vi "CspecN2_Part_2024.vi"(0 "Temperature [K]":dbl=293.16 format="%.4g") -> (1 "rel unc Cp0 N2":dbl=1.7168935136343725e-07 format="%.1e", 2 "Cp0/R N2":dbl=3.50261546072023 format="%.5f", 3 "Cp0 N2 [J / K mol]":dbl=29.122365250340124 format="%.5g", 4 "Cv0 N2 [J / K mol]":dbl=20.807902650340125 format="%.5g", 5 "Gamma0 N2":dbl=1.3995819636278475)   [LabVIEW 2016]
uses:
  <vilib>/Analysis/NI_AALPro.lvlib
panel:
  out "ur(Cp0) /ppm":dbl[](array[numeric]) format="%.2f"
  out "abs unc Cp0 N2 [J / K mol]":dbl=5e-06 format="%.6f"
  out "abs unc Cp0/R N2":dbl=6.013617765266032e-07 format="%.6f"
  out "u(Cp0) / J mol-1 K-1":dbl[](array[numeric]) format="%.6f"
  out "Cp0 array / J mol-1 K-1":dbl[](array[numeric]) format="%.5g"
  out "T array / K":dbl[](array[numeric]) format="%.2g"
  # "Gamache, R. R., & Orphanos, N. G. \"Thermodynamic functions for N2 from the total partition sum and its moments\" J. Phys. Chem. Ref. Data 52, 023101 (2023)"
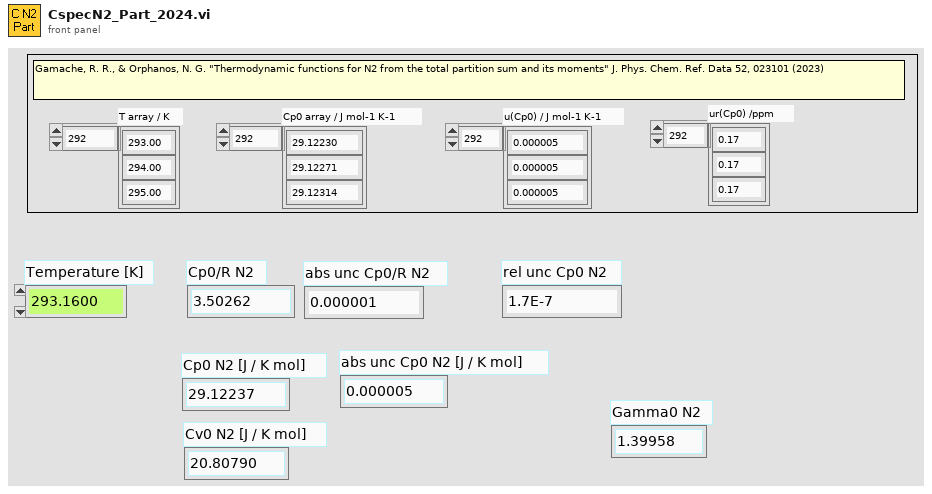
[diagram p1: front panel]
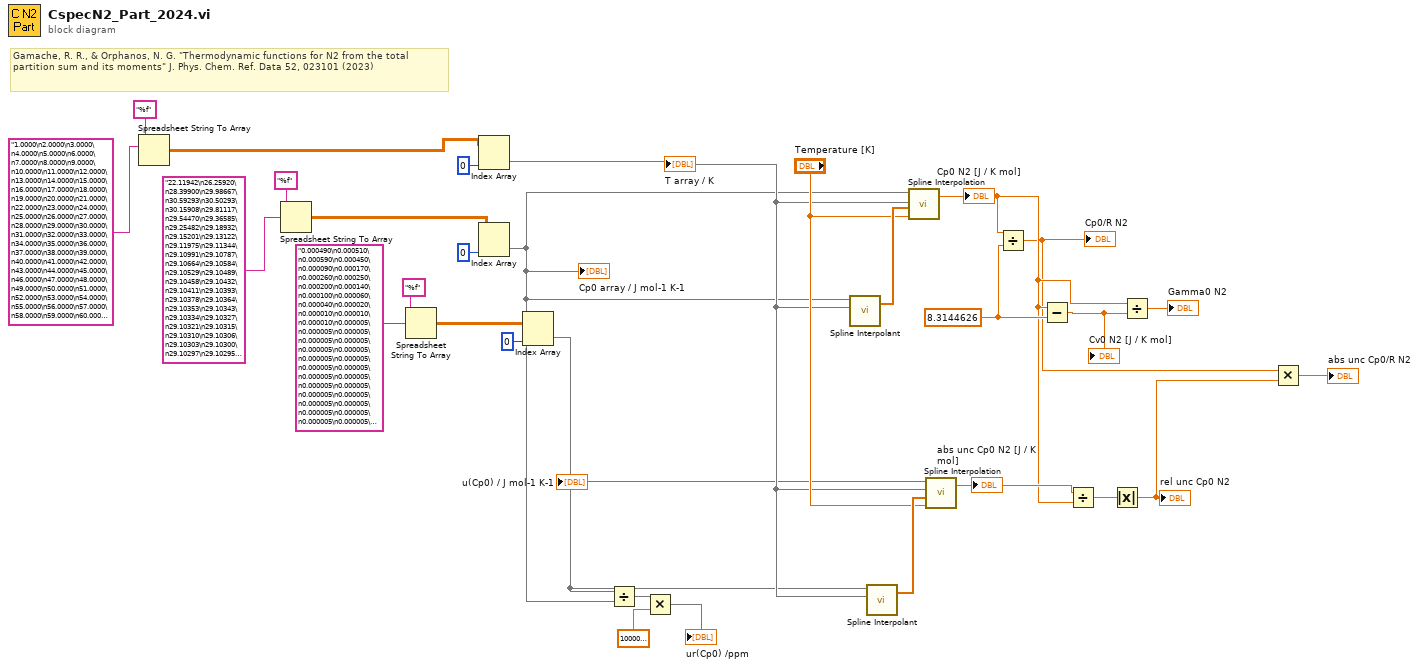
[diagram p0: block diagram]
diagram:
  w27 = 8.3144626
  # "Gamache, R. R., & Orphanos, N. G. \"Thermodynamic functions for N2 from the total partition sum and its moments\" J. Phys. Chem. Ref. Data 52, 023101 (2023)"
  n1 = Spreadsheet String To Array(format string="%f", spreadsheet string="1.0000\n2.0000\n3.0000\n4.0000\n5.0000\n6.0000\n7.0000\n8.0000\n9.0000\n10.0000\n11.0000\n12.0000\n13.0000\n14.0000\n15.0000\n16.0000\n17.0000\n18.0000\n19.0000\n20.0000\n21.0000\n22.0000\n23.0000\n24.0000\n25.0000\n26.0000\n27.0000\n28.0000\n29.0000\n30.0000\n31.0000\n32.0000\n33.0000\n34.0000\n35.0000\n36.0000\n37.0000\n38.0000\n39.0000\n40.0000\n41.0000\n42.0000\n43.0000\n44.0000\n45.0000\n46.0000\n47.0000\n48.0000\n49.0000\n50.0000\n51.0000\n52.0000\n53.0000\n54.0000\n55.0000\n56.0000\n57.0000\n58.0000\n59.0000\n60.0000\n61.0000\n62.0000\n63.0000\n64.0000\n65.0000\n66.0000\n67.0000\n68.0000\n69.0000\n70.0000\n71.0000\n72.0000\n73.0000\n74.0000\n75.0000\n76.0000\n77.0000\n78.0000\n79.0000\n80.0000\n81.0000\n82.0000\n83.0000\n84.0000\n85.0000\n86.0000\n87.0000\n88.0000\n89.0000\n90.0000\n91.0000\n92.0000\n93.0000\n94.0000\n95.0000\n96.0000\n97.0000\n98.0000\n99.0000\n100.0000\n101.0000\n102.0000\n103.0000\n104.0000\n105.0000\n106.0000\n107.0000\n108.0000\n109.0000\n110.0000\n111.0000\n112.0000\n113.0000\n114.0000\n115.0000\n116.0000\n117.0000\n118.0000\n119.0000\n120.0000\n121.0000\n122.0000\n123.0000\n124.0000\n125.0000\n126.0000\n127.0000\n128.0000\n129.0000\n130.0000\n131.0000\n132.0000\n133.0000\n134.0000\n135.0000\n136.0000\n137.0000\n138.0000\n139.0000\n140.0000\n141.0000\n142.0000\n143.0000\n144.0000\n145.0000\n146.0000\n147.0000\n148.0000\n149.0000\n150.0000\n151.0000\n152.0000\n153.0000\n154.0000\n155.0000\n156.0000\n157.0000\n158.0000\n159.0000\n160.0000\n161.0000\n162.0000\n163.0000\n164.0000\n165.0000\n166.0000\n167.0000\n168.0000\n169.0000\n170.0000\n171.0000\n172.0000\n173.0000\n174.0000\n175.0000\n176.0000\n177.0000\n178.0000\n179.0000\n180.0000\n181.0000\n182.0000\n183.0000\n184.0000\n185.0000\n186.0000\n187.0000\n188.0000\n189.0000\n190.0000\n191.0000\n192.0000\n193.0000\n194.0000\n195.0000\n196.0000\n197.0000\n198.0000\n199.0000\n200.0000\n201.0000\n202.0000\n203.0000\n204.0000\n205.0000\n206.0000\n207.0000\n208.0000\n209.0000\n210.0000\n211.0000\n212.0000\n213.0000\n214.0000\n215.0000\n216.0000\n217.0000\n218.0000\n219.0000\n220.0000\n221.0000\n222.0000\n223.0000\n224.0000\n225.0000\n226.0000\n227.0000\n228.0000\n229.0000\n230.0000\n231.0000\n232.0000\n233.0000\n234.0000\n235.0000\n236.0000\n237.0000\n238.0000\n239.0000\n240.0000\n241.0000\n242.0000\n243.0000\n244.0000\n245.0000\n246.0000\n247.0000\n248.0000\n249.0000\n250.0000\n251.0000\n252.0000\n253.0000\n254.0000\n255.0000\n256.0000\n257.0000\n258.0000\n259.0000\n260.0000\n261.0000\n262.0000\n263.0000\n264.0000\n265.0000\n266.0000\n267.0000\n268.0000\n269.0000\n270.0000\n271.0000\n272.0000\n273.0000\n274.0000\n275.0000\n276.0000\n277.0000\n278.0000\n279.0000\n280.0000\n281.0000\n282.0000\n283.0000\n284.0000\n285.0000\n286.0000\n287.0000\n288.0000\n289.0000\n290.0000\n291.0000\n292.0000\n293.0000\n294.0000\n295.0000\n296.0000\n297.0000\n298.1500\n299.0000\n300.0000\n301.0000\n302.0000\n303.0000\n304.0000\n305.0000\n306.0000\n307.0000\n308.0000\n309.0000\n310.0000\n311.0000\n312.0000\n313.0000\n314.0000\n315.0000\n316.0000\n317.0000\n318.0000\n319.0000\n320.0000\n321.0000\n322.0000\n323.0000\n324.0000\n325.0000\n326.0000\n327.0000\n328.0000\n329.0000\n330.0000\n331.0000\n332.0000\n333.0000\n334.0000\n335.0000\n336.0000\n337.0000\n338.0000\n339.0000\n340.0000\n341.0000\n342.0000\n343.0000\n344.0000\n345.0000\n346.0000\n347.0000\n348.0000\n349.0000\n350.0000\n351.0000\n352.0000\n353.0000\n354.0000\n355.0000\n356.0000\n357.0000\n358.0000\n359.0000\n360.0000\n361.0000\n362.0000\n363.0000\n364.0000\n365.0000\n366.0000\n367.0000\n368.0000\n369.0000\n370.0000\n371.0000\n372.0000\n373.0000\n374.0000\n375.0000\n376.0000\n377.0000\n378.0000\n379.0000\n380.0000\n381.0000\n382.0000\n383.0000\n384.0000\n385.0000\n386.0000\n387.0000\n388.0000\n389.0000\n390.0000\n391.0000\n392.0000\n393.0000\n394.0000\n395.0000\n396.0000\n397.0000\n398.0000\n399.0000\n400.0000\n401.0000\n402.0000\n403.0000\n404.0000\n405.0000\n406.0000\n407.0000\n408.0000\n409.0000\n410.0000\n411.0000\n412.0000\n413.0000\n414.0000\n415.0000\n416.0000\n417.0000\n418.0000\n419.0000\n420.0000\n421.0000\n422.0000\n423.0000\n424.0000\n425.0000\n426.0000\n427.0000\n428.0000\n429.0000\n430.0000\n431.0000\n432.0000\n433.0000\n434.0000\n435.0000\n436.0000\n437.0000\n438.0000\n439.0000\n440.0000\n441.0000\n442.0000\n443.0000\n444.0000\n445.0000\n446.0000\n447.0000\n448.0000\n449.0000\n450.0000\n451.0000\n452.0000\n453.0000\n454.0000\n455.0000\n456.0000\n457.0000\n458.0000\n459.0000\n460.0000\n461.0000\n462.0000\n463.0000\n464.0000\n465.0000\n466.0000\n467.0000\n468.0000\n469.0000\n470.0000\n471.0000\n472.0000\n473.0000\n474.0000\n475.0000\n476.0000\n477.0000\n478.0000\n479.0000\n480.0000\n481.0000\n482.0000\n483.0000\n484.0000\n485.0000\n486.0000\n487.0000\n488.0000\n489.0000\n490.0000\n491.0000\n492.0000\n493.0000\n494.0000\n495.0000\n496.0000\n497.0000\n498.0000\n499.0000\n500.0000\n501.0000\n502.0000\n503.0000\n504.0000\n505.0000\n506.0000\n507.0000\n508.0000\n509.0000\n510.0000\n511.0000\n512.0000\n513.0000\n514.0000\n515.0000\n516.0000\n517.0000\n518.0000\n519.0000\n520.0000\n521.0000\n522.0000\n523.0000\n524.0000\n525.0000\n526.0000\n527.0000\n528.0000\n529.0000\n530.0000\n531.0000\n532.0000\n533.0000\n534.0000\n535.0000\n536.0000\n537.0000\n538.0000\n539.0000\n540.0000\n541.0000\n542.0000\n543.0000\n544.0000\n545.0000\n546.0000\n547.0000\n548.0000\n549.0000\n550.0000\n551.0000\n552.0000\n553.0000\n554.0000\n555.0000\n556.0000\n557.0000\n558.0000\n559.0000\n560.0000\n561.0000\n562.0000\n563.0000\n564.0000\n565.0000\n566.0000\n567.0000\n568.0000\n569.0000\n570.0000\n571.0000\n572.0000\n573.0000\n574.0000\n575.0000\n576.0000\n577.0000\n578.0000\n579.0000\n580.0000\n581.0000\n582.0000\n583.0000\n584.0000\n585.0000\n586.0000\n587.0000\n588.0000\n589.0000\n590.0000\n591.0000\n592.0000\n593.0000\n594.0000\n595.0000\n596.0000\n597.0000\n598.0000\n599.0000\n600.0000\n601.0000\n602.0000\n603.0000\n604.0000\n605.0000\n606.0000\n607.0000\n608.0000\n609.0000\n610.0000\n611.0000\n612.0000\n613.0000\n614.0000\n615.0000\n616.0000\n617.0000\n618.0000\n619.0000\n620.0000\n621.0000\n622.0000\n623.0000\n624.0000\n625.0000\n626.0000\n627.0000\n628.0000\n629.0000\n630.0000\n631.0000\n632.0000\n633.0000\n634.0000\n635.0000\n636.0000\n637.0000\n638.0000\n639.0000\n640.0000\n641.0000\n642.0000\n643.0000\n644.0000\n645.0000\n646.0000\n647.0000\n648.0000\n649.0000\n650.0000\n651.0000\n652.0000\n653.0000\n654.0000\n655.0000\n656.0000\n657.0000\n658.0000\n659.0000\n660.0000\n661.0000\n662.0000\n663.0000\n664.0000\n665.0000\n666.0000\n667.0000\n668.0000\n669.0000\n670.0000\n671.0000\n672.0000\n673.0000\n674.0000\n675.0000\n676.0000\n677.0000\n678.0000\n679.0000\n680.0000\n681.0000\n682.0000\n683.0000\n684.0000\n685.0000\n686.0000\n687.0000\n688.0000\n689.0000\n690.0000\n691.0000\n692.0000\n693.0000\n694.0000\n695.0000\n696.0000\n697.0000\n698.0000\n699.0000\n700.0000\n701.0000\n702.0000\n703.0000\n704.0000\n705.0000\n706.0000\n707.0000\n708.0000\n709.0000\n710.0000\n711.0000\n712.0000\n713.0000\n714.0000\n715.0000\n716.0000\n717.0000\n718.0000\n719.0000\n720.0000\n721.0000\n722.0000\n723.0000\n724.0000\n725.0000\n726.0000\n727.0000\n728.0000\n729.0000\n730.0000\n731.0000\n732.0000\n733.0000\n734.0000\n735.0000\n736.0000\n737.0000\n738.0000\n739.0000\n740.0000\n741.0000\n742.0000\n743.0000\n744.0000\n745.0000\n746.0000\n747.0000\n748.0000\n749.0000\n750.0000\n751.0000\n752.0000\n753.0000\n754.0000\n755.0000\n756.0000\n757.0000\n758.0000\n759.0000\n760.0000\n761.0000\n762.0000\n763.0000\n764.0000\n765.0000\n766.0000\n767.0000\n768.0000\n769.0000\n770.0000\n771.0000\n772.0000\n773.0000\n774.0000\n775.0000\n776.0000\n777.0000\n778.0000\n779.0000\n780.0000\n781.0000\n782.0000\n783.0000\n784.0000\n785.0000\n786.0000\n787.0000\n788.0000\n789.0000\n790.0000\n791.0000\n792.0000\n793.0000\n794.0000\n795.0000\n796.0000\n797.0000\n798.0000\n799.0000\n800.0000\n801.0000\n802.0000\n803.0000\n804.0000\n805.0000\n806.0000\n807.0000\n808.0000\n809.0000\n810.0000\n811.0000\n812.0000\n813.0000\n814.0000\n815.0000\n816.0000\n817.0000\n818.0000\n819.0000\n820.0000\n821.0000\n822.0000\n823.0000\n824.0000\n825.0000\n826.0000\n827.0000\n828.0000\n829.0000\n830.0000\n831.0000\n832.0000\n833.0000\n834.0000\n835.0000\n836.0000\n837.0000\n838.0000\n839.0000\n840.0000\n841.0000\n842.0000\n843.0000\n844.0000\n845.0000\n846.0000\n847.0000\n848.0000\n849.0000\n850.0000\n851.0000\n852.0000\n853.0000\n854.0000\n855.0000\n856.0000\n857.0000\n858.0000\n859.0000\n860.0000\n861.0000\n862.0000\n863.0000\n864.0000\n865.0000\n866.0000\n867.0000\n868.0000\n869.0000\n870.0000\n871.0000\n872.0000\n873.0000\n874.0000\n875.0000\n876.0000\n877.0000\n878.0000\n879.0000\n880.0000\n881.0000\n882.0000\n883.0000\n884.0000\n885.0000\n886.0000\n887.0000\n888.0000\n889.0000\n890.0000\n891.0000\n892.0000\n893.0000\n894.0000\n895.0000\n896.0000\n897.0000\n898.0000\n899.0000\n900.0000\n901.0000\n902.0000\n903.0000\n904.0000\n905.0000\n906.0000\n907.0000\n908.0000\n909.0000\n910.0000\n911.0000\n912.0000\n913.0000\n914.0000\n915.0000\n916.0000\n917.0000\n918.0000\n919.0000\n920.0000\n921.0000\n922.0000\n923.0000\n924.0000\n925.0000\n926.0000\n927.0000\n928.0000\n929.0000\n930.0000\n931.0000\n932.0000\n933.0000\n934.0000\n935.0000\n936.0000\n937.0000\n938.0000\n939.0000\n940.0000\n941.0000\n942.0000\n943.0000\n944.0000\n945.0000\n946.0000\n947.0000\n948.0000\n949.0000\n950.0000\n951.0000\n952.0000\n953.0000\n954.0000\n955.0000\n956.0000\n957.0000\n958.0000\n959.0000\n960.0000\n961.0000\n962.0000\n963.0000\n964.0000\n965.0000\n966.0000\n967.0000\n968.0000\n969.0000\n970.0000\n971.0000\n972.0000\n973.0000\n974.0000\n975.0000\n976.0000\n977.0000\n978.0000\n979.0000\n980.0000\n981.0000\n982.0000\n983.0000\n984.0000\n985.0000\n986.0000\n987.0000\n988.0000\n989.0000\n990.0000\n991.0000\n992.0000\n993.0000\n994.0000\n995.0000\n996.0000\n997.0000\n998.0000\n999.0000\n1000.0000\n1001.0000\n1002.0000\n1003.0000\n1004.0000\n1005.0000\n1006.0000\n1007.0000\n1008.0000\n1009.0000\n1010.0000\n1011.0000\n1012.0000\n1013.0000\n1014.0000\n1015.0000\n1016.0000\n1017.0000\n1018.0000\n1019.0000\n1020.0000\n1021.0000\n1022.0000\n1023.0000\n1024.0000\n1025.0000\n1026.0000\n1027.0000\n1028.0000\n1029.0000\n1030.0000\n1031.0000\n1032.0000\n1033.0000\n1034.0000\n1035.0000\n1036.0000\n1037.0000\n1038.0000\n1039.0000\n1040.0000\n1041.0000\n1042.0000\n1043.0000\n1044.0000\n1045.0000\n1046.0000\n1047.0000\n1048.0000\n1049.0000\n1050.0000\n1051.0000\n1052.0000\n1053.0000\n1054.0000\n1055.0000\n1056.0000\n1057.0000\n1058.0000\n1059.0000\n1060.0000\n1061.0000\n1062.0000\n1063.0000\n1064.0000\n1065.0000\n1066.0000\n1067.0000\n1068.0000\n1069.0000\n1070.0000\n1071.0000\n1072.0000\n1073.0000\n1074.0000\n1075.0000\n1076.0000\n1077.0000\n1078.0000\n1079.0000\n1080.0000\n1081.0000\n1082.0000\n1083.0000\n1084.0000\n1085.0000\n1086.0000\n1087.0000\n1088.0000\n1089.0000\n1090.0000\n1091.0000\n1092.0000\n1093.0000\n1094.0000\n1095.0000\n1096.0000\n1097.0000\n1098.0000\n1099.0000\n1100.0000\n1101.0000\n1102.0000\n1103.0000\n1104.0000\n1105.0000\n1106.0000\n1107.0000\n1108.0000\n1109.0000\n1110.0000\n1111.0000\n1112.0000\n1113.0000\n1114.0000\n1115.0000\n1116.0000\n1117.0000\n1118.0000\n1119.0000\n1120.0000\n1121.0000\n1122.0000\n1123.0000\n1124.0000\n1125.0000\n1126.0000\n1127.0000\n1128.0000\n1129.0000\n1130.0000\n1131.0000\n1132.0000\n1133.0000\n1134.0000\n1135.0000\n1136.0000\n1137.0000\n1138.0000\n1139.0000\n1140.0000\n1141.0000\n1142.0000\n1143.0000\n1144.0000\n1145.0000\n1146.0000\n1147.0000\n1148.0000\n1149.0000\n1150.0000\n1151.0000\n1152.0000\n1153.0000\n1154.0000\n1155.0000\n1156.0000\n1157.0000\n1158.0000\n1159.0000\n1160.0000\n1161.0000\n1162.0000\n1163.0000\n1164.0000\n1165.0000\n1166.0000\n1167.0000\n1168.0000\n1169.0000\n1170.0000\n1171.0000\n1172.0000\n1173.0000\n1174.0000\n1175.0000\n1176.0000\n1177.0000\n1178.0000\n1179.0000\n1180.0000\n1181.0000\n1182.0000\n1183.0000\n1184.0000\n1185.0000\n1186.0000\n1187.0000\n1188.0000\n1189.0000\n1190.0000\n1191.0000\n1192.0000\n1193.0000\n1194.0000\n1195.0000\n1196.0000\n1197.0000\n1198.0000\n1199.0000\n1200.0000\n1201.0000\n1202.0000\n1203.0000\n1204.0000\n1205.0000\n1206.0000\n1207.0000\n1208.0000\n1209.0000\n1210.0000\n1211.0000\n1212.0000\n1213.0000\n1214.0000\n1215.0000\n1216.0000\n1217.0000\n1218.0000\n1219.0000\n1220.0000\n1221.0000\n1222.0000\n1223.0000\n1224.0000\n1225.0000\n1226.0000\n1227.0000\n1228.0000\n1229.0000\n1230.0000\n1231.0000\n1232.0000\n1233.0000\n1234.0000\n1235.0000\n1236.0000\n1237.0000\n1238.0000\n1239.0000\n1240.0000\n1241.0000\n1242.0000\n1243.0000\n1244.0000\n1245.0000\n1246.0000\n1247.0000\n1248.0000\n1249.0000\n1250.0000\n1251.0000\n1252.0000\n1253.0000\n1254.0000\n1255.0000\n1256.0000\n1257.0000\n1258.0000\n1259.0000\n1260.0000\n1261.0000\n1262.0000\n1263.0000\n1264.0000\n1265.0000\n1266.0000\n1267.0000\n1268.0000\n1269.0000\n1270.0000\n1271.0000\n1272.0000\n1273.0000\n1274.0000\n1275.0000\n1276.0000\n1277.0000\n1278.0000\n1279.0000\n1280.0000\n1281.0000\n1282.0000\n1283.0000\n1284.0000\n1285.0000\n1286.0000\n1287.0000\n1288.0000\n1289.0000\n1290.0000\n1291.0000\n1292.0000\n1293.0000\n1294.0000\n1295.0000\n1296.0000\n1297.0000\n1298.0000\n1299.0000\n1300.0000\n1301.0000\n1302.0000\n1303.0000\n1304.0000\n1305.0000\n1306.0000\n1307.0000\n1308.0000\n1309.0000\n1310.0000\n1311.0000\n1312.0000\n1313.0000\n1314.0000\n1315.0000\n1316.0000\n1317.0000\n1318.0000\n1319.0000\n1320.0000\n1321.0000\n1322.0000\n1323.0000\n1324.0000\n1325.0000\n1326.0000\n1327.0000\n1328.0000\n1329.0000\n1330.0000\n1331.0000\n1332.0000\n1333.0000\n1334.0000\n1335.0000\n1336.0000\n1337.0000\n1338.0000\n1339.0000\n1340.0000\n1341.0000\n1342.0000\n1343.0000\n1344.0000\n1345.0000\n1346.0000\n1347.0000\n1348.0000\n1349.0000\n1350.0000\n1351.0000\n1352.0000\n1353.0000\n1354.0000\n1355.0000\n1356.0000\n1357.0000\n1358.0000\n1359.0000\n1360.0000\n1361.0000\n1362.0000\n1363.0000\n1364.0000\n1365.0000\n1366.0000\n1367.0000\n1368.0000\n1369.0000\n1370.0000\n1371.0000\n1372.0000\n1373.0000\n1374.0000\n1375.0000\n1376.0000\n1377.0000\n1378.0000\n1379.0000\n1380.0000\n1381.0000\n1382.0000\n1383.0000\n1384.0000\n1385.0000\n1386.0000\n1387.0000\n1388.0000\n1389.0000\n1390.0000\n1391.0000\n1392.0000\n1393.0000\n1394.0000\n1395.0000\n1396.0000\n1397.0000\n1398.0000\n1399.0000\n1400.0000\n1401.0000\n1402.0000\n1403.0000\n1404.0000\n1405.0000\n1406.0000\n1407.0000\n1408.0000\n1409.0000\n1410.0000\n1411.0000\n1412.0000\n1413.0000\n1414.0000\n1415.0000\n1416.0000\n1417.0000\n1418.0000\n1419.0000\n1420.0000\n1421.0000\n1422.0000\n1423.0000\n1424.0000\n1425.0000\n1426.0000\n1427.0000\n1428.0000\n1429.0000\n1430.0000\n1431.0000\n1432.0000\n1433.0000\n1434.0000\n1435.0000\n1436.0000\n1437.0000\n1438.0000\n1439.0000\n1440.0000\n1441.0000\n1442.0000\n1443.0000\n1444.0000\n1445.0000\n1446.0000\n1447.0000\n1448.0000\n1449.0000\n1450.0000\n1451.0000\n1452.0000\n1453.0000\n1454.0000\n1455.0000\n1456.0000\n1457.0000\n1458.0000\n1459.0000\n1460.0000\n1461.0000\n1462.0000\n1463.0000\n1464.0000\n1465.0000\n1466.0000\n1467.0000\n1468.0000\n1469.0000\n1470.0000\n1471.0000\n1472.0000\n1473.0000\n1474.0000\n1475.0000\n1476.0000\n1477.0000\n1478.0000\n1479.0000\n1480.0000\n1481.0000\n1482.0000\n1483.0000\n1484.0000\n1485.0000\n1486.0000\n1487.0000\n1488.0000\n1489.0000\n1490.0000\n1491.0000\n1492.0000\n1493.0000\n1494.0000\n1495.0000\n1496.0000\n1497.0000\n1498.0000\n1499.0000\n1500.0000\n1501.0000\n1502.0000\n1503.0000\n1504.0000\n1505.0000\n1506.0000\n1507.0000\n1508.0000\n1509.0000\n1510.0000\n1511.0000\n1512.0000\n1513.0000\n1514.0000\n1515.0000\n1516.0000\n1517.0000\n1518.0000\n1519.0000\n1520.0000\n1521.0000\n1522.0000\n1523.0000\n1524.0000\n1525.0000\n1526.0000\n1527.0000\n1528.0000\n1529.0000\n1530.0000\n1531.0000\n1532.0000\n1533.0000\n1534.0000\n1535.0000\n1536.0000\n1537.0000\n1538.0000\n1539.0000\n1540.0000\n1541.0000\n1542.0000\n1543.0000\n1544.0000\n1545.0000\n1546.0000\n1547.0000\n1548.0000\n1549.0000\n1550.0000\n1551.0000\n1552.0000\n1553.0000\n1554.0000\n1555.0000\n1556.0000\n1557.0000\n1558.0000\n1559.0000\n1560.0000\n1561.0000\n1562.0000\n1563.0000\n1564.0000\n1565.0000\n1566.0000\n1567.0000\n1568.0000\n1569.0000\n1570.0000\n1571.0000\n1572.0000\n1573.0000\n1574.0000\n1575.0000\n1576.0000\n1577.0000\n1578.0000\n1579.0000\n1580.0000\n1581.0000\n1582.0000\n1583.0000\n1584.0000\n1585.0000\n1586.0000\n1587.0000\n1588.0000\n1589.0000\n1590.0000\n1591.0000\n1592.0000\n1593.0000\n1594.0000\n1595.0000\n1596.0000\n1597.0000\n1598.0000\n1599.0000\n1600.0000\n1601.0000\n1602.0000\n1603.0000\n1604.0000\n1605.0000\n1606.0000\n1607.0000\n1608.0000\n1609.0000\n1610.0000\n1611.0000\n1612.0000\n1613.0000\n1614.0000\n1615.0000\n1616.0000\n1617.0000\n1618.0000\n1619.0000\n1620.0000\n1621.0000\n1622.0000\n1623.0000\n1624.0000\n1625.0000\n1626.0000\n1627.0000\n1628.0000\n1629.0000\n1630.0000\n1631.0000\n1632.0000\n1633.0000\n1634.0000\n1635.0000\n1636.0000\n1637.0000\n1638.0000\n1639.0000\n1640.0000\n1641.0000\n1642.0000\n1643.0000\n1644.0000\n1645.0000\n1646.0000\n1647.0000\n1648.0000\n1649.0000\n1650.0000\n1651.0000\n1652.0000\n1653.0000\n1654.0000\n1655.0000\n1656.0000\n1657.0000\n1658.0000\n1659.0000\n1660.0000\n1661.0000\n1662.0000\n1663.0000\n1664.0000\n1665.0000\n1666.0000\n1667.0000\n1668.0000\n1669.0000\n1670.0000\n1671.0000\n1672.0000\n1673.0000\n1674.0000\n1675.0000\n1676.0000\n1677.0000\n1678.0000\n1679.0000\n1680.0000\n1681.0000\n1682.0000\n1683.0000\n1684.0000\n1685.0000\n1686.0000\n1687.0000\n1688.0000\n1689.0000\n1690.0000\n1691.0000\n1692.0000\n1693.0000\n1694.0000\n1695.0000\n1696.0000\n1697.0000\n1698.0000\n1699.0000\n1700.0000\n1701.0000\n1702.0000\n1703.0000\n1704.0000\n1705.0000\n1706.0000\n1707.0000\n1708.0000\n1709.0000\n1710.0000\n1711.0000\n1712.0000\n1713.0000\n1714.0000\n1715.0000\n1716.0000\n1717.0000\n1718.0000\n1719.0000\n1720.0000\n1721.0000\n1722.0000\n1723.0000\n1724.0000\n1725.0000\n1726.0000\n1727.0000\n1728.0000\n1729.0000\n1730.0000\n1731.0000\n1732.0000\n1733.0000\n1734.0000\n1735.0000\n1736.0000\n1737.0000\n1738.0000\n1739.0000\n1740.0000\n1741.0000\n1742.0000\n1743.0000\n1744.0000\n1745.0000\n1746.0000\n1747.0000\n1748.0000\n1749.0000\n1750.0000\n1751.0000\n1752.0000\n1753.0000\n1754.0000\n1755.0000\n1756.0000\n1757.0000\n1758.0000\n1759.0000\n1760.0000\n1761.0000\n1762.0000\n1763.0000\n1764.0000\n1765.0000\n1766.0000\n1767.0000\n1768.0000\n1769.0000\n1770.0000\n1771.0000\n1772.0000\n1773.0000\n1774.0000\n1775.0000\n1776.0000\n1777.0000\n1778.0000\n1779.0000\n1780.0000\n1781.0000\n1782.0000\n1783.0000\n1784.0000\n1785.0000\n1786.0000\n1787.0000\n1788.0000\n1789.0000\n1790.0000\n1791.0000\n1792.0000\n1793.0000\n1794.0000\n1795.0000\n1796.0000\n1797.0000\n1798.0000\n1799.0000\n1800.0000\n1801.0000\n1802.0000\n1803.0000\n1804.0000\n1805.0000\n1806.0000\n1807.0000\n1808.0000\n1809.0000\n1810.0000\n1811.0000\n1812.0000\n1813.0000\n1814.0000\n1815.0000\n1816.0000\n1817.0000\n1818.0000\n1819.0000\n1820.0000\n1821.0000\n1822.0000\n1823.0000\n1824.0000\n1825.0000\n1826.0000\n1827.0000\n1828.0000\n1829.0000\n1830.0000\n1831.0000\n1832.0000\n1833.0000\n1834.0000\n1835.0000\n1836.0000\n1837.0000\n1838.0000\n1839.0000\n1840.0000\n1841.0000\n1842.0000\n1843.0000\n1844.0000\n1845.0000\n1846.0000\n1847.0000\n1848.0000\n1849.0000\n1850.0000\n1851.0000\n1852.0000\n1853.0000\n1854.0000\n1855.0000\n1856.0000\n1857.0000\n1858.0000\n1859.0000\n1860.0000\n1861.0000\n1862.0000\n1863.0000\n1864.0000\n1865.0000\n1866.0000\n1867.0000\n1868.0000\n1869.0000\n1870.0000\n1871.0000\n1872.0000\n1873.0000\n1874.0000\n1875.0000\n1876.0000\n1877.0000\n1878.0000\n1879.0000\n1880.0000\n1881.0000\n1882.0000\n1883.0000\n1884.0000\n1885.0000\n1886.0000\n1887.0000\n1888.0000\n1889.0000\n1890.0000\n1891.0000\n1892.0000\n1893.0000\n1894.0000\n1895.0000\n1896.0000\n1897.0000\n1898.0000\n1899.0000\n1900.0000\n1901.0000\n1902.0000\n1903.0000\n1904.0000\n1905.0000\n1906.0000\n1907.0000\n1908.0000\n1909.0000\n1910.0000\n1911.0000\n1912.0000\n1913.0000\n1914.0000\n1915.0000\n1916.0000\n1917.0000\n1918.0000\n1919.0000\n1920.0000\n1921.0000\n1922.0000\n1923.0000\n1924.0000\n1925.0000\n1926.0000\n1927.0000\n1928.0000\n1929.0000\n1930.0000\n1931.0000\n1932.0000\n1933.0000\n1934.0000\n1935.0000\n1936.0000\n1937.0000\n1938.0000\n1939.0000\n1940.0000\n1941.0000\n1942.0000\n1943.0000\n1944.0000\n1945.0000\n1946.0000\n1947.0000\n1948.0000\n1949.0000\n1950.0000\n1951.0000\n1952.0000\n1953.0000\n1954.0000\n1955.0000\n1956.0000\n1957.0000\n1958.0000\n1959.0000\n1960.0000\n1961.0000\n1962.0000\n1963.0000\n1964.0000\n1965.0000\n1966.0000\n1967.0000\n1968.0000\n1969.0000\n1970.0000\n1971.0000\n1972.0000\n1973.0000\n1974.0000\n1975.0000\n1976.0000\n1977.0000\n1978.0000\n1979.0000\n1980.0000\n1981.0000\n1982.0000\n1983.0000\n1984.0000\n1985.0000\n1986.0000\n1987.0000\n1988.0000\n1989.0000\n1990.0000\n1991.0000\n1992.0000\n1993.0000\n1994.0000\n1995.0000\n1996.0000\n1997.0000\n1998.0000\n1999.0000\n2000.0000\n2001.0000\n2002.0000\n2003.0000\n2004.0000\n2005.0000\n2006.0000\n2007.0000\n2008.0000\n2009.0000\n2010.0000\n2011.0000\n2012.0000\n2013.0000\n2014.0000\n2015.0000\n2016.0000\n2017.0000\n2018.0000\n2019.0000\n2020.0000\n2021.0000\n2022.0000\n2023.0000\n2024.0000\n2025.0000\n2026.0000\n2027.0000\n2028.0000\n2029.0000\n2030.0000\n2031.0000\n2032.0000\n2033.0000\n2034.0000\n2035.0000\n2036.0000\n2037.0000\n2038.0000\n2039.0000\n2040.0000\n2041.0000\n2042.0000\n2043.0000\n2044.0000\n2045.0000\n2046.0000\n2047.0000\n2048.0000\n2049.0000\n2050.0000\n2051.0000\n2052.0000\n2053.0000\n2054.0000\n2055.0000\n2056.0000\n2057.0000\n2058.0000\n2059.0000\n2060.0000\n2061.0000\n2062.0000\n2063.0000\n2064.0000\n2065.0000\n2066.0000\n2067.0000\n2068.0000\n2069.0000\n2070.0000\n2071.0000\n2072.0000\n2073.0000\n2074.0000\n2075.0000\n2076.0000\n2077.0000\n2078.0000\n2079.0000\n2080.0000\n2081.0000\n2082.0000\n2083.0000\n2084.0000\n2085.0000\n2086.0000\n2087.0000\n2088.0000\n2089.0000\n2090.0000\n2091.0000\n2092.0000\n2093.0000\n2094.0000\n2095.0000\n2096.0000\n2097.0000\n2098.0000\n2099.0000\n2100.0000\n2101.0000\n2102.0000\n2103.0000\n2104.0000\n2105.0000\n2106.0000\n2107.0000\n2108.0000\n2109.0000\n2110.0000\n2111.0000\n2112.0000\n2113.0000\n2114.0000\n2115.0000\n2116.0000\n2117.0000\n2118.0000\n2119.0000\n2120.0000\n2121.0000\n2122.0000\n2123.0000\n2124.0000\n2125.0000\n2126.0000\n2127.0000\n2128.0000\n2129.0000\n2130.0000\n2131.0000\n2132.0000\n2133.0000\n2134.0000\n2135.0000\n2136.0000\n2137.0000\n2138.0000\n2139.0000\n2140.0000\n2141.0000\n2142.0000\n2143.0000\n2144.0000\n2145.0000\n2146.0000\n2147.0000\n2148.0000\n2149.0000\n2150.0000\n2151.0000\n2152.0000\n2153.0000\n2154.0000\n2155.0000\n2156.0000\n2157.0000\n2158.0000\n2159.0000\n2160.0000\n2161.0000\n2162.0000\n2163.0000\n2164.0000\n2165.0000\n2166.0000\n2167.0000\n2168.0000\n2169.0000\n2170.0000\n2171.0000\n2172.0000\n2173.0000\n2174.0000\n2175.0000\n2176.0000\n2177.0000\n2178.0000\n2179.0000\n2180.0000\n2181.0000\n2182.0000\n2183.0000\n2184.0000\n2185.0000\n2186.0000\n2187.0000\n2188.0000\n2189.0000\n2190.0000\n2191.0000\n2192.0000\n2193.0000\n2194.0000\n2195.0000\n2196.0000\n2197.0000\n2198.0000\n2199.0000\n2200.0000\n2201.0000\n2202.0000\n2203.0000\n2204.0000\n2205.0000\n2206.0000\n2207.0000\n2208.0000\n2209.0000\n2210.0000\n2211.0000\n2212.0000\n2213.0000\n2214.0000\n2215.0000\n2216.0000\n2217.0000\n2218.0000\n2219.0000\n2220.0000\n2221.0000\n2222.0000\n2223.0000\n2224.0000\n2225.0000\n2226.0000\n2227.0000\n2228.0000\n2229.0000\n2230.0000\n2231.0000\n2232.0000\n2233.0000\n2234.0000\n2235.0000\n2236.0000\n2237.0000\n2238.0000\n2239.0000\n2240.0000\n2241.0000\n2242.0000\n2243.0000\n2244.0000\n2245.0000\n2246.0000\n2247.0000\n2248.0000\n2249.0000\n2250.0000\n2251.0000\n2252.0000\n2253.0000\n2254.0000\n2255.0000\n2256.0000\n2257.0000\n2258.0000\n2259.0000\n2260.0000\n2261.0000\n2262.0000\n2263.0000\n2264.0000\n2265.0000\n2266.0000\n2267.0000\n2268.0000\n2269.0000\n2270.0000\n2271.0000\n2272.0000\n2273.0000\n2274.0000\n2275.0000\n2276.0000\n2277.0000\n2278.0000\n2279.0000\n2280.0000\n2281.0000\n2282.0000\n2283.0000\n2284.0000\n2285.0000\n2286.0000\n2287.0000\n2288.0000\n2289.0000\n2290.0000\n2291.0000\n2292.0000\n2293.0000\n2294.0000\n2295.0000\n2296.0000\n2297.0000\n2298.0000\n2299.0000\n2300.0000\n2301.0000\n2302.0000\n2303.0000\n2304.0000\n2305.0000\n2306.0000\n2307.0000\n2308.0000\n2309.0000\n2310.0000\n2311.0000\n2312.0000\n2313.0000\n2314.0000\n2315.0000\n2316.0000\n2317.0000\n2318.0000\n2319.0000\n2320.0000\n2321.0000\n2322.0000\n2323.0000\n2324.0000\n2325.0000\n2326.0000\n2327.0000\n2328.0000\n2329.0000\n2330.0000\n2331.0000\n2332.0000\n2333.0000\n2334.0000\n2335.0000\n2336.0000\n2337.0000\n2338.0000\n2339.0000\n2340.0000\n2341.0000\n2342.0000\n2343.0000\n2344.0000\n2345.0000\n2346.0000\n2347.0000\n2348.0000\n2349.0000\n2350.0000\n2351.0000\n2352.0000\n2353.0000\n2354.0000\n2355.0000\n2356.0000\n2357.0000\n2358.0000\n2359.0000\n2360.0000\n2361.0000\n2362.0000\n2363.0000\n2364.0000\n2365.0000\n2366.0000\n2367.0000\n2368.0000\n2369.0000\n2370.0000\n2371.0000\n2372.0000\n2373.0000\n2374.0000\n2375.0000\n2376.0000\n2377.0000\n2378.0000\n2379.0000\n2380.0000\n2381.0000\n2382.0000\n2383.0000\n2384.0000\n2385.0000\n2386.0000\n2387.0000\n2388.0000\n2389.0000\n2390.0000\n2391.0000\n2392.0000\n2393.0000\n2394.0000\n2395.0000\n2396.0000\n2397.0000\n2398.0000\n2399.0000\n2400.0000\n2401.0000\n2402.0000\n2403.0000\n2404.0000\n2405.0000\n2406.0000\n2407.0000\n2408.0000\n2409.0000\n2410.0000\n2411.0000\n2412.0000\n2413.0000\n2414.0000\n2415.0000\n2416.0000\n2417.0000\n2418.0000\n2419.0000\n2420.0000\n2421.0000\n2422.0000\n2423.0000\n2424.0000\n2425.0000\n2426.0000\n2427.0000\n2428.0000\n2429.0000\n2430.0000\n2431.0000\n2432.0000\n2433.0000\n2434.0000\n2435.0000\n2436.0000\n2437.0000\n2438.0000\n2439.0000\n2440.0000\n2441.0000\n2442.0000\n2443.0000\n2444.0000\n2445.0000\n2446.0000\n2447.0000\n2448.0000\n2449.0000\n2450.0000\n2451.0000\n2452.0000\n2453.0000\n2454.0000\n2455.0000\n2456.0000\n2457.0000\n2458.0000\n2459.0000\n2460.0000\n2461.0000\n2462.0000\n2463.0000\n2464.0000\n2465.0000\n2466.0000\n2467.0000\n2468.0000\n2469.0000\n2470.0000\n2471.0000\n2472.0000\n2473.0000\n2474.0000\n2475.0000\n2476.0000\n2477.0000\n2478.0000\n2479.0000\n2480.0000\n2481.0000\n2482.0000\n2483.0000\n2484.0000\n2485.0000\n2486.0000\n2487.0000\n2488.0000\n2489.0000\n2490.0000\n2491.0000\n2492.0000\n2493.0000\n2494.0000\n2495.0000\n2496.0000\n2497.0000\n2498.0000\n2499.0000\n2500.0000\n2501.0000\n2502.0000\n2503.0000\n2504.0000\n2505.0000\n2506.0000\n2507.0000\n2508.0000\n2509.0000\n2510.0000\n2511.0000\n2512.0000\n2513.0000\n2514.0000\n2515.0000\n2516.0000\n2517.0000\n2518.0000\n2519.0000\n2520.0000\n2521.0000\n2522.0000\n2523.0000\n2524.0000\n2525.0000\n2526.0000\n2527.0000\n2528.0000\n2529.0000\n2530.0000\n2531.0000\n2532.0000\n2533.0000\n2534.0000\n2535.0000\n2536.0000\n2537.0000\n2538.0000\n2539.0000\n2540.0000\n2541.0000\n2542.0000\n2543.0000\n2544.0000\n2545.0000\n2546.0000\n2547.0000\n2548.0000\n2549.0000\n2550.0000\n2551.0000\n2552.0000\n2553.0000\n2554.0000\n2555.0000\n2556.0000\n2557.0000\n2558.0000\n2559.0000\n2560.0000\n2561.0000\n2562.0000\n2563.0000\n2564.0000\n2565.0000\n2566.0000\n2567.0000\n2568.0000\n2569.0000\n2570.0000\n2571.0000\n2572.0000\n2573.0000\n2574.0000\n2575.0000\n2576.0000\n2577.0000\n2578.0000\n2579.0000\n2580.0000\n2581.0000\n2582.0000\n2583.0000\n2584.0000\n2585.0000\n2586.0000\n2587.0000\n2588.0000\n2589.0000\n2590.0000\n2591.0000\n2592.0000\n2593.0000\n2594.0000\n2595.0000\n2596.0000\n2597.0000\n2598.0000\n2599.0000\n2600.0000\n2601.0000\n2602.0000\n2603.0000\n2604.0000\n2605.0000\n2606.0000\n2607.0000\n2608.0000\n2609.0000\n2610.0000\n2611.0000\n2612.0000\n2613.0000\n2614.0000\n2615.0000\n2616.0000\n2617.0000\n2618.0000\n2619.0000\n2620.0000\n2621.0000\n2622.0000\n2623.0000\n2624.0000\n2625.0000\n2626.0000\n2627.0000\n2628.0000\n2629.0000\n2630.0000\n2631.0000\n2632.0000\n2633.0000\n2634.0000\n2635.0000\n2636.0000\n2637.0000\n2638.0000\n2639.0000\n2640.0000\n2641.0000\n2642.0000\n2643.0000\n2644.0000\n2645.0000\n2646.0000\n2647.0000\n2648.0000\n2649.0000\n2650.0000\n2651.0000\n2652.0000\n2653.0000\n2654.0000\n2655.0000\n2656.0000\n2657.0000\n2658.0000\n2659.0000\n2660.0000\n2661.0000\n2662.0000\n2663.0000\n2664.0000\n2665.0000\n2666.0000\n2667.0000\n2668.0000\n2669.0000\n2670.0000\n2671.0000\n2672.0000\n2673.0000\n2674.0000\n2675.0000\n2676.0000\n2677.0000\n2678.0000\n2679.0000\n2680.0000\n2681.0000\n2682.0000\n2683.0000\n2684.0000\n2685.0000\n2686.0000\n2687.0000\n2688.0000\n2689.0000\n2690.0000\n2691.0000\n2692.0000\n2693.0000\n2694.0000\n2695.0000\n2696.0000\n2697.0000\n2698.0000\n2699.0000\n2700.0000\n2701.0000\n2702.0000\n2703.0000\n2704.0000\n2705.0000\n2706.0000\n2707.0000\n2708.0000\n2709.0000\n2710.0000\n2711.0000\n2712.0000\n2713.0000\n2714.0000\n2715.0000\n2716.0000\n2717.0000\n2718.0000\n2719.0000\n2720.0000\n2721.0000\n2722.0000\n2723.0000\n2724.0000\n2725.0000\n2726.0000\n2727.0000\n2728.0000\n2729.0000\n2730.0000\n2731.0000\n2732.0000\n2733.0000\n2734.0000\n2735.0000\n2736.0000\n2737.0000\n2738.0000\n2739.0000\n2740.0000\n2741.0000\n2742.0000\n2743.0000\n2744.0000\n2745.0000\n2746.0000\n2747.0000\n2748.0000\n2749.0000\n2750.0000\n2751.0000\n2752.0000\n2753.0000\n2754.0000\n2755.0000\n2756.0000\n2757.0000\n2758.0000\n2759.0000\n2760.0000\n2761.0000\n2762.0000\n2763.0000\n2764.0000\n2765.0000\n2766.0000\n2767.0000\n2768.0000\n2769.0000\n2770.0000\n2771.0000\n2772.0000\n2773.0000\n2774.0000\n2775.0000\n2776.0000\n2777.0000\n2778.0000\n2779.0000\n2780.0000\n2781.0000\n2782.0000\n2783.0000\n2784.0000\n2785.0000\n2786.0000\n2787.0000\n2788.0000\n2789.0000\n2790.0000\n2791.0000\n2792.0000\n2793.0000\n2794.0000\n2795.0000\n2796.0000\n2797.0000\n2798.0000\n2799.0000\n2800.0000\n2801.0000\n2802.0000\n2803.0000\n2804.0000\n2805.0000\n2806.0000\n2807.0000\n2808.0000\n2809.0000\n2810.0000\n2811.0000\n2812.0000\n2813.0000\n2814.0000\n2815.0000\n2816.0000\n2817.0000\n2818.0000\n2819.0000\n2820.0000\n2821.0000\n2822.0000\n2823.0000\n2824.0000\n2825.0000\n2826.0000\n2827.0000\n2828.0000\n2829.0000\n2830.0000\n2831.0000\n2832.0000\n2833.0000\n2834.0000\n2835.0000\n2836.0000\n2837.0000\n2838.0000\n2839.0000\n2840.0000\n2841.0000\n2842.0000\n2843.0000\n2844.0000\n2845.0000\n2846.0000\n2847.0000\n2848.0000\n2849.0000\n2850.0000\n2851.0000\n2852.0000\n2853.0000\n2854.0000\n2855.0000\n2856.0000\n2857.0000\n2858.0000\n2859.0000\n2860.0000\n2861.0000\n2862.0000\n2863.0000\n2864.0000\n2865.0000\n2866.0000\n2867.0000\n2868.0000\n2869.0000\n2870.0000\n2871.0000\n2872.0000\n2873.0000\n2874.0000\n2875.0000\n2876.0000\n2877.0000\n2878.0000\n2879.0000\n2880.0000\n2881.0000\n2882.0000\n2883.0000\n2884.0000\n2885.0000\n2886.0000\n2887.0000\n2888.0000\n2889.0000\n2890.0000\n2891.0000\n2892.0000\n2893.0000\n2894.0000\n2895.0000\n2896.0000\n2897.0000\n2898.0000\n2899.0000\n2900.0000\n2901.0000\n2902.0000\n2903.0000\n2904.0000\n2905.0000\n2906.0000\n2907.0000\n2908.0000\n2909.0000\n2910.0000\n2911.0000\n2912.0000\n2913.0000\n2914.0000\n2915.0000\n2916.0000\n2917.0000\n2918.0000\n2919.0000\n2920.0000\n2921.0000\n2922.0000\n2923.0000\n2924.0000\n2925.0000\n2926.0000\n2927.0000\n2928.0000\n2929.0000\n2930.0000\n2931.0000\n2932.0000\n2933.0000\n2934.0000\n2935.0000\n2936.0000\n2937.0000\n2938.0000\n2939.0000\n2940.0000\n2941.0000\n2942.0000\n2943.0000\n2944.0000\n2945.0000\n2946.0000\n2947.0000\n2948.0000\n2949.0000\n2950.0000\n2951.0000\n2952.0000\n2953.0000\n2954.0000\n2955.0000\n2956.0000\n2957.0000\n2958.0000\n2959.0000\n2960.0000\n2961.0000\n2962.0000\n2963.0000\n2964.0000\n2965.0000\n2966.0000\n2967.0000\n2968.0000\n2969.0000\n2970.0000\n2971.0000\n2972.0000\n2973.0000\n2974.0000\n2975.0000\n2976.0000\n2977.0000\n2978.0000\n2979.0000\n2980.0000\n2981.0000\n2982.0000\n2983.0000\n2984.0000\n2985.0000\n2986.0000\n2987.0000\n2988.0000\n2989.0000\n2990.0000\n2991.0000\n2992.0000\n2993.0000\n2994.0000\n2995.0000\n2996.0000\n2997.0000\n2998.0000\n2999.0000\n3000.0000\n3001.0000\n3002.0000\n3003.0000\n3004.0000\n3005.0000\n3006.0000\n3007.0000\n3008.0000\n3009.0000\n3010.0000\n3011.0000\n3012.0000\n3013.0000\n3014.0000\n3015.0000\n3016.0000\n3017.0000\n3018.0000\n3019.0000\n3020.0000\n3021.0000\n3022.0000\n3023.0000\n3024.0000\n3025.0000\n3026.0000\n3027.0000\n3028.0000\n3029.0000\n3030.0000\n3031.0000\n3032.0000\n3033.0000\n3034.0000\n3035.0000\n3036.0000\n3037.0000\n3038.0000\n3039.0000\n3040.0000\n3041.0000\n3042.0000\n3043.0000\n3044.0000\n3045.0000\n3046.0000\n3047.0000\n3048.0000\n3049.0000\n3050.0000\n3051.0000\n3052.0000\n3053.0000\n3054.0000\n3055.0000\n3056.0000\n3057.0000\n3058.0000\n3059.0000\n3060.0000\n3061.0000\n3062.0000\n3063.0000\n3064.0000\n3065.0000\n3066.0000\n3067.0000\n3068.0000\n3069.0000\n3070.0000\n3071.0000\n3072.0000\n3073.0000\n3074.0000\n3075.0000\n3076.0000\n3077.0000\n3078.0000\n3079.0000\n3080.0000\n3081.0000\n3082.0000\n3083.0000\n3084.0000\n3085.0000\n3086.0000\n3087.0000\n3088.0000\n3089.0000\n3090.0000\n3091.0000\n3092.0000\n3093.0000\n3094.0000\n3095.0000\n3096.0000\n3097.0000\n3098.0000\n3099.0000\n3100.0000\n3101.0000\n3102.0000\n3103.0000\n3104.0000\n3105.0000\n3106.0000\n3107.0000\n3108.0000\n3109.0000\n3110.0000\n3111.0000\n3112.0000\n3113.0000\n3114.0000\n3115.0000\n3116.0000\n3117.0000\n3118.0000\n3119.0000\n3120.0000\n3121.0000\n3122.0000\n3123.0000\n3124.0000\n3125.0000\n3126.0000\n3127.0000\n3128.0000\n3129.0000\n3130.0000\n3131.0000\n3132.0000\n3133.0000\n3134.0000\n3135.0000\n3136.0000\n3137.0000\n3138.0000\n3139.0000\n3140.0000\n3141.0000\n3142.0000\n3143.0000\n3144.0000\n3145.0000\n3146.0000\n3147.0000\n3148.0000\n3149.0000\n3150.0000\n3151.0000\n3152.0000\n3153.0000\n3154.0000\n3155.0000\n3156.0000\n3157.0000\n3158.0000\n3159.0000\n3160.0000\n3161.0000\n3162.0000\n3163.0000\n3164.0000\n3165.0000\n3166.0000\n3167.0000\n3168.0000\n3169.0000\n3170.0000\n3171.0000\n3172.0000\n3173.0000\n3174.0000\n3175.0000\n3176.0000\n3177.0000\n3178.0000\n3179.0000\n3180.0000\n3181.0000\n3182.0000\n3183.0000\n3184.0000\n3185.0000\n3186.0000\n3187.0000\n3188.0000\n3189.0000\n3190.0000\n3191.0000\n3192.0000\n3193.0000\n3194.0000\n3195.0000\n3196.0000\n3197.0000\n3198.0000\n3199.0000\n3200.0000\n3201.0000\n3202.0000\n3203.0000\n3204.0000\n3205.0000\n3206.0000\n3207.0000\n3208.0000\n3209.0000\n3210.0000\n3211.0000\n3212.0000\n3213.0000\n3214.0000\n3215.0000\n3216.0000\n3217.0000\n3218.0000\n3219.0000\n3220.0000\n3221.0000\n3222.0000\n3223.0000\n3224.0000\n3225.0000\n3226.0000\n3227.0000\n3228.0000\n3229.0000\n3230.0000\n3231.0000\n3232.0000\n3233.0000\n3234.0000\n3235.0000\n3236.0000\n3237.0000\n3238.0000\n3239.0000\n3240.0000\n3241.0000\n3242.0000\n3243.0000\n3244.0000\n3245.0000\n3246.0000\n3247.0000\n3248.0000\n3249.0000\n3250.0000\n3251.0000\n3252.0000\n3253.0000\n3254.0000\n3255.0000\n3256.0000\n3257.0000\n3258.0000\n3259.0000\n3260.0000\n3261.0000\n3262.0000\n3263.0000\n3264.0000\n3265.0000\n3266.0000\n3267.0000\n3268.0000\n3269.0000\n3270.0000\n3271.0000\n3272.0000\n3273.0000\n3274.0000\n3275.0000\n3276.0000\n3277.0000\n3278.0000\n3279.0000\n3280.0000\n3281.0000\n3282.0000\n3283.0000\n3284.0000\n3285.0000\n3286.0000\n3287.0000\n3288.0000\n3289.0000\n3290.0000\n3291.0000\n3292.0000\n3293.0000\n3294.0000\n3295.0000\n3296.0000\n3297.0000\n3298.0000\n3299.0000\n3300.0000\n3301.0000\n3302.0000\n3303.0000\n3304.0000\n3305.0000\n3306.0000\n3307.0000\n3308.0000\n3309.0000\n3310.0000\n3311.0000\n3312.0000\n3313.0000\n3314.0000\n3315.0000\n3316.0000\n3317.0000\n3318.0000\n3319.0000\n3320.0000\n3321.0000\n3322.0000\n3323.0000\n3324.0000\n3325.0000\n3326.0000\n3327.0000\n3328.0000\n3329.0000\n3330.0000\n3331.0000\n3332.0000\n3333.0000\n3334.0000\n3335.0000\n3336.0000\n3337.0000\n3338.0000\n3339.0000\n3340.0000\n3341.0000\n3342.0000\n3343.0000\n3344.0000\n3345.0000\n3346.0000\n3347.0000\n3348.0000\n3349.0000\n3350.0000\n3351.0000\n3352.0000\n3353.0000\n3354.0000\n3355.0000\n3356.0000\n3357.0000\n3358.0000\n3359.0000\n3360.0000\n3361.0000\n3362.0000\n3363.0000\n3364.0000\n3365.0000\n3366.0000\n3367.0000\n3368.0000\n3369.0000\n3370.0000\n3371.0000\n3372.0000\n3373.0000\n3374.0000\n3375.0000\n3376.0000\n3377.0000\n3378.0000\n3379.0000\n3380.0000\n3381.0000\n3382.0000\n3383.0000\n3384.0000\n3385.0000\n3386.0000\n3387.0000\n3388.0000\n3389.0000\n3390.0000\n3391.0000\n3392.0000\n3393.0000\n3394.0000\n3395.0000\n3396.0000\n3397.0000\n3398.0000\n3399.0000\n3400.0000\n3401.0000\n3402.0000\n3403.0000\n3404.0000\n3405.0000\n3406.0000\n3407.0000\n3408.0000\n3409.0000\n3410.0000\n3411.0000\n3412.0000\n3413.0000\n3414.0000\n3415.0000\n3416.0000\n3417.0000\n3418.0000\n3419.0000\n3420.0000\n3421.0000\n3422.0000\n3423.0000\n3424.0000\n3425.0000\n3426.0000\n3427.0000\n3428.0000\n3429.0000\n3430.0000\n3431.0000\n3432.0000\n3433.0000\n3434.0000\n3435.0000\n3436.0000\n3437.0000\n3438.0000\n3439.0000\n3440.0000\n3441.0000\n3442.0000\n3443.0000\n3444.0000\n3445.0000\n3446.0000\n3447.0000\n3448.0000\n3449.0000\n3450.0000\n3451.0000\n3452.0000\n3453.0000\n3454.0000\n3455.0000\n3456.0000\n3457.0000\n3458.0000\n3459.0000\n3460.0000\n3461.0000\n3462.0000\n3463.0000\n3464.0000\n3465.0000\n3466.0000\n3467.0000\n3468.0000\n3469.0000\n3470.0000\n3471.0000\n3472.0000\n3473.0000\n3474.0000\n3475.0000\n3476.0000\n3477.0000\n3478.0000\n3479.0000\n3480.0000\n3481.0000\n3482.0000\n3483.0000\n3484.0000\n3485.0000\n3486.0000\n3487.0000\n3488.0000\n3489.0000\n3490.0000\n3491.0000\n3492.0000\n3493.0000\n3494.0000\n3495.0000\n3496.0000\n3497.0000\n3498.0000\n3499.0000\n3500.0000\n3501.0000\n3502.0000\n3503.0000\n3504.0000\n3505.0000\n3506.0000\n3507.0000\n3508.0000\n3509.0000\n3510.0000\n3511.0000\n3512.0000\n3513.0000\n3514.0000\n3515.0000\n3516.0000\n3517.0000\n3518.0000\n3519.0000\n3520.0000\n3521.0000\n3522.0000\n3523.0000\n3524.0000\n3525.0000\n3526.0000\n3527.0000\n3528.0000\n3529.0000\n3530.0000\n3531.0000\n3532.0000\n3533.0000\n3534.0000\n3535.0000\n3536.0000\n3537.0000\n3538.0000\n3539.0000\n3540.0000\n3541.0000\n3542.0000\n3543.0000\n3544.0000\n3545.0000\n3546.0000\n3547.0000\n3548.0000\n3549.0000\n3550.0000\n3551.0000\n3552.0000\n3553.0000\n3554.0000\n3555.0000\n3556.0000\n3557.0000\n3558.0000\n3559.0000\n3560.0000\n3561.0000\n3562.0000\n3563.0000\n3564.0000\n3565.0000\n3566.0000\n3567.0000\n3568.0000\n3569.0000\n3570.0000\n3571.0000\n3572.0000\n3573.0000\n3574.0000\n3575.0000\n3576.0000\n3577.0000\n3578.0000\n3579.0000\n3580.0000\n3581.0000\n3582.0000\n3583.0000\n3584.0000\n3585.0000\n3586.0000\n3587.0000\n3588.0000\n3589.0000\n3590.0000\n3591.0000\n3592.0000\n3593.0000\n3594.0000\n3595.0000\n3596.0000\n3597.0000\n3598.0000\n3599.0000\n3600.0000\n3601.0000\n3602.0000\n3603.0000\n3604.0000\n3605.0000\n3606.0000\n3607.0000\n3608.0000\n3609.0000\n3610.0000\n3611.0000\n3612.0000\n3613.0000\n3614.0000\n3615.0000\n3616.0000\n3617.0000\n3618.0000\n3619.0000\n3620.0000\n3621.0000\n3622.0000\n3623.0000\n3624.0000\n3625.0000\n3626.0000\n3627.0000\n3628.0000\n3629.0000\n3630.0000\n3631.0000\n3632.0000\n3633.0000\n3634.0000\n3635.0000\n3636.0000\n3637.0000\n3638.0000\n3639.0000\n3640.0000\n3641.0000\n3642.0000\n3643.0000\n3644.0000\n3645.0000\n3646.0000\n3647.0000\n3648.0000\n3649.0000\n3650.0000\n3651.0000\n3652.0000\n3653.0000\n3654.0000\n3655.0000\n3656.0000\n3657.0000\n3658.0000\n3659.0000\n3660.0000\n3661.0000\n3662.0000\n3663.0000\n3664.0000\n3665.0000\n3666.0000\n3667.0000\n3668.0000\n3669.0000\n3670.0000\n3671.0000\n3672.0000\n3673.0000\n3674.0000\n3675.0000\n3676.0000\n3677.0000\n3678.0000\n3679.0000\n3680.0000\n3681.0000\n3682.0000\n3683.0000\n3684.0000\n3685.0000\n3686.0000\n3687.0000\n3688.0000\n3689.0000\n3690.0000\n3691.0000\n3692.0000\n3693.0000\n3694.0000\n3695.0000\n3696.0000\n3697.0000\n3698.0000\n3699.0000\n3700.0000\n3701.0000\n3702.0000\n3703.0000\n3704.0000\n3705.0000\n3706.0000\n3707.0000\n3708.0000\n3709.0000\n3710.0000\n3711.0000\n3712.0000\n3713.0000\n3714.0000\n3715.0000\n3716.0000\n3717.0000\n3718.0000\n3719.0000\n3720.0000\n3721.0000\n3722.0000\n3723.0000\n3724.0000\n3725.0000\n3726.0000\n3727.0000\n3728.0000\n3729.0000\n3730.0000\n3731.0000\n3732.0000\n3733.0000\n3734.0000\n3735.0000\n3736.0000\n3737.0000\n3738.0000\n3739.0000\n3740.0000\n3741.0000\n3742.0000\n3743.0000\n3744.0000\n3745.0000\n3746.0000\n3747.0000\n3748.0000\n3749.0000\n3750.0000\n3751.0000\n3752.0000\n3753.0000\n3754.0000\n3755.0000\n3756.0000\n3757.0000\n3758.0000\n3759.0000\n3760.0000\n3761.0000\n3762.0000\n3763.0000\n3764.0000\n3765.0000\n3766.0000\n3767.0000\n3768.0000\n3769.0000\n3770.0000\n3771.0000\n3772.0000\n3773.0000\n3774.0000\n3775.0000\n3776.0000\n3777.0000\n3778.0000\n3779.0000\n3780.0000\n3781.0000\n3782.0000\n3783.0000\n3784.0000\n3785.0000\n3786.0000\n3787.0000\n3788.0000\n3789.0000\n3790.0000\n3791.0000\n3792.0000\n3793.0000\n3794.0000\n3795.0000\n3796.0000\n3797.0000\n3798.0000\n3799.0000\n3800.0000\n3801.0000\n3802.0000\n3803.0000\n3804.0000\n3805.0000\n3806.0000\n3807.0000\n3808.0000\n3809.0000\n3810.0000\n3811.0000\n3812.0000\n3813.0000\n3814.0000\n3815.0000\n3816.0000\n3817.0000\n3818.0000\n3819.0000\n3820.0000\n3821.0000\n3822.0000\n3823.0000\n3824.0000\n3825.0000\n3826.0000\n3827.0000\n3828.0000\n3829.0000\n3830.0000\n3831.0000\n3832.0000\n3833.0000\n3834.0000\n3835.0000\n3836.0000\n3837.0000\n3838.0000\n3839.0000\n3840.0000\n3841.0000\n3842.0000\n3843.0000\n3844.0000\n3845.0000\n3846.0000\n3847.0000\n3848.0000\n3849.0000\n3850.0000\n3851.0000\n3852.0000\n3853.0000\n3854.0000\n3855.0000\n3856.0000\n3857.0000\n3858.0000\n3859.0000\n3860.0000\n3861.0000\n3862.0000\n3863.0000\n3864.0000\n3865.0000\n3866.0000\n3867.0000\n3868.0000\n3869.0000\n3870.0000\n3871.0000\n3872.0000\n3873.0000\n3874.0000\n3875.0000\n3876.0000\n3877.0000\n3878.0000\n3879.0000\n3880.0000\n3881.0000\n3882.0000\n3883.0000\n3884.0000\n3885.0000\n3886.0000\n3887.0000\n3888.0000\n3889.0000\n3890.0000\n3891.0000\n3892.0000\n3893.0000\n3894.0000\n3895.0000\n3896.0000\n3897.0000\n3898.0000\n3899.0000\n3900.0000\n3901.0000\n3902.0000\n3903.0000\n3904.0000\n3905.0000\n3906.0000\n3907.0000\n3908.0000\n3909.0000\n3910.0000\n3911.0000\n3912.0000\n3913.0000\n3914.0000\n3915.0000\n3916.0000\n3917.0000\n3918.0000\n3919.0000\n3920.0000\n3921.0000\n3922.0000\n3923.0000\n3924.0000\n3925.0000\n3926.0000\n3927.0000\n3928.0000\n3929.0000\n3930.0000\n3931.0000\n3932.0000\n3933.0000\n3934.0000\n3935.0000\n3936.0000\n3937.0000\n3938.0000\n3939.0000\n3940.0000\n3941.0000\n3942.0000\n3943.0000\n3944.0000\n3945.0000\n3946.0000\n3947.0000\n3948.0000\n3949.0000\n3950.0000\n3951.0000\n3952.0000\n3953.0000\n3954.0000\n3955.0000\n3956.0000\n3957.0000\n3958.0000\n3959.0000\n3960.0000\n3961.0000\n3962.0000\n3963.0000\n3964.0000\n3965.0000\n3966.0000\n3967.0000\n3968.0000\n3969.0000\n3970.0000\n3971.0000\n3972.0000\n3973.0000\n3974.0000\n3975.0000\n3976.0000\n3977.0000\n3978.0000\n3979.0000\n3980.0000\n3981.0000\n3982.0000\n3983.0000\n3984.0000\n3985.0000\n3986.0000\n3987.0000\n3988.0000\n3989.0000\n3990.0000\n3991.0000\n3992.0000\n3993.0000\n3994.0000\n3995.0000\n3996.0000\n3997.0000\n3998.0000\n3999.0000\n4000.0000\n4001.0000\n4002.0000\n4003.0000\n4004.0000\n4005.0000\n4006.0000\n4007.0000\n4008.0000\n4009.0000\n4010.0000\n4011.0000\n4012.0000\n4013.0000\n4014.0000\n4015.0000\n4016.0000\n4017.0000\n4018.0000\n4019.0000\n4020.0000\n4021.0000\n4022.0000\n4023.0000\n4024.0000\n4025.0000\n4026.0000\n4027.0000\n4028.0000\n4029.0000\n4030.0000\n4031.0000\n4032.0000\n4033.0000\n4034.0000\n4035.0000\n4036.0000\n4037.0000\n4038.0000\n4039.0000\n4040.0000\n4041.0000\n4042.0000\n4043.0000\n4044.0000\n4045.0000\n4046.0000\n4047.0000\n4048.0000\n4049.0000\n4050.0000\n4051.0000\n4052.0000\n4053.0000\n4054.0000\n4055.0000\n4056.0000\n4057.0000\n4058.0000\n4059.0000\n4060.0000\n4061.0000\n4062.0000\n4063.0000\n4064.0000\n4065.0000\n4066.0000\n4067.0000\n4068.0000\n4069.0000\n4070.0000\n4071.0000\n4072.0000\n4073.0000\n4074.0000\n4075.0000\n4076.0000\n4077.0000\n4078.0000\n4079.0000\n4080.0000\n4081.0000\n4082.0000\n4083.0000\n4084.0000\n4085.0000\n4086.0000\n4087.0000\n4088.0000\n4089.0000\n4090.0000\n4091.0000\n4092.0000\n4093.0000\n4094.0000\n4095.0000\n4096.0000\n4097.0000\n4098.0000\n4099.0000\n4100.0000\n4101.0000\n4102.0000\n4103.0000\n4104.0000\n4105.0000\n4106.0000\n4107.0000\n4108.0000\n4109.0000\n4110.0000\n4111.0000\n4112.0000\n4113.0000\n4114.0000\n4115.0000\n4116.0000\n4117.0000\n4118.0000\n4119.0000\n4120.0000\n4121.0000\n4122.0000\n4123.0000\n4124.0000\n4125.0000\n4126.0000\n4127.0000\n4128.0000\n4129.0000\n4130.0000\n4131.0000\n4132.0000\n4133.0000\n4134.0000\n4135.0000\n4136.0000\n4137.0000\n4138.0000\n4139.0000\n4140.0000\n4141.0000\n4142.0000\n4143.0000\n4144.0000\n4145.0000\n4146.0000\n4147.0000\n4148.0000\n4149.0000\n4150.0000\n4151.0000\n4152.0000\n4153.0000\n4154.0000\n4155.0000\n4156.0000\n4157.0000\n4158.0000\n4159.0000\n4160.0000\n4161.0000\n4162.0000\n4163.0000\n4164.0000\n4165.0000\n4166.0000\n4167.0000\n4168.0000\n4169.0000\n4170.0000\n4171.0000\n4172.0000\n4173.0000\n4174.0000\n4175.0000\n4176.0000\n4177.0000\n4178.0000\n4179.0000\n4180.0000\n4181.0000\n4182.0000\n4183.0000\n4184.0000\n4185.0000\n4186.0000\n4187.0000\n4188.0000\n4189.0000\n4190.0000\n4191.0000\n4192.0000\n4193.0000\n4194.0000\n4195.0000\n4196.0000\n4197.0000\n4198.0000\n4199.0000\n4200.0000\n4201.0000\n4202.0000\n4203.0000\n4204.0000\n4205.0000\n4206.0000\n4207.0000\n4208.0000\n4209.0000\n4210.0000\n4211.0000\n4212.0000\n4213.0000\n4214.0000\n4215.0000\n4216.0000\n4217.0000\n4218.0000\n4219.0000\n4220.0000\n4221.0000\n4222.0000\n4223.0000\n4224.0000\n4225.0000\n4226.0000\n4227.0000\n4228.0000\n4229.0000\n4230.0000\n4231.0000\n4232.0000\n4233.0000\n4234.0000\n4235.0000\n4236.0000\n4237.0000\n4238.0000\n4239.0000\n4240.0000\n4241.0000\n4242.0000\n4243.0000\n4244.0000\n4245.0000\n4246.0000\n4247.0000\n4248.0000\n4249.0000\n4250.0000\n4251.0000\n4252.0000\n4253.0000\n4254.0000\n4255.0000\n4256.0000\n4257.0000\n4258.0000\n4259.0000\n4260.0000\n4261.0000\n4262.0000\n4263.0000\n4264.0000\n4265.0000\n4266.0000\n4267.0000\n4268.0000\n4269.0000\n4270.0000\n4271.0000\n4272.0000\n4273.0000\n4274.0000\n4275.0000\n4276.0000\n4277.0000\n4278.0000\n4279.0000\n4280.0000\n4281.0000\n4282.0000\n4283.0000\n4284.0000\n4285.0000\n4286.0000\n4287.0000\n4288.0000\n4289.0000\n4290.0000\n4291.0000\n4292.0000\n4293.0000\n4294.0000\n4295.0000\n4296.0000\n4297.0000\n4298.0000\n4299.0000\n4300.0000\n4301.0000\n4302.0000\n4303.0000\n4304.0000\n4305.0000\n4306.0000\n4307.0000\n4308.0000\n4309.0000\n4310.0000\n4311.0000\n4312.0000\n4313.0000\n4314.0000\n4315.0000\n4316.0000\n4317.0000\n4318.0000\n4319.0000\n4320.0000\n4321.0000\n4322.0000\n4323.0000\n4324.0000\n4325.0000\n4326.0000\n4327.0000\n4328.0000\n4329.0000\n4330.0000\n4331.0000\n4332.0000\n4333.0000\n4334.0000\n4335.0000\n4336.0000\n4337.0000\n4338.0000\n4339.0000\n4340.0000\n4341.0000\n4342.0000\n4343.0000\n4344.0000\n4345.0000\n4346.0000\n4347.0000\n4348.0000\n4349.0000\n4350.0000\n4351.0000\n4352.0000\n4353.0000\n4354.0000\n4355.0000\n4356.0000\n4357.0000\n4358.0000\n4359.0000\n4360.0000\n4361.0000\n4362.0000\n4363.0000\n4364.0000\n4365.0000\n4366.0000\n4367.0000\n4368.0000\n4369.0000\n4370.0000\n4371.0000\n4372.0000\n4373.0000\n4374.0000\n4375.0000\n4376.0000\n4377.0000\n4378.0000\n4379.0000\n4380.0000\n4381.0000\n4382.0000\n4383.0000\n4384.0000\n4385.0000\n4386.0000\n4387.0000\n4388.0000\n4389.0000\n4390.0000\n4391.0000\n4392.0000\n4393.0000\n4394.0000\n4395.0000\n4396.0000\n4397.0000\n4398.0000\n4399.0000\n4400.0000\n4401.0000\n4402.0000\n4403.0000\n4404.0000\n4405.0000\n4406.0000\n4407.0000\n4408.0000\n4409.0000\n4410.0000\n4411.0000\n4412.0000\n4413.0000\n4414.0000\n4415.0000\n4416.0000\n4417.0000\n4418.0000\n4419.0000\n4420.0000\n4421.0000\n4422.0000\n4423.0000\n4424.0000\n4425.0000\n4426.0000\n4427.0000\n4428.0000\n4429.0000\n4430.0000\n4431.0000\n4432.0000\n4433.0000\n4434.0000\n4435.0000\n4436.0000\n4437.0000\n4438.0000\n4439.0000\n4440.0000\n4441.0000\n4442.0000\n4443.0000\n4444.0000\n4445.0000\n4446.0000\n4447.0000\n4448.0000\n4449.0000\n4450.0000\n4451.0000\n4452.0000\n4453.0000\n4454.0000\n4455.0000\n4456.0000\n4457.0000\n4458.0000\n4459.0000\n4460.0000\n4461.0000\n4462.0000\n4463.0000\n4464.0000\n4465.0000\n4466.0000\n4467.0000\n4468.0000\n4469.0000\n4470.0000\n4471.0000\n4472.0000\n4473.0000\n4474.0000\n4475.0000\n4476.0000\n4477.0000\n4478.0000\n4479.0000\n4480.0000\n4481.0000\n4482.0000\n4483.0000\n4484.0000\n4485.0000\n4486.0000\n4487.0000\n4488.0000\n4489.0000\n4490.0000\n4491.0000\n4492.0000\n4493.0000\n4494.0000\n4495.0000\n4496.0000\n4497.0000\n4498.0000\n4499.0000\n4500.0000\n4501.0000\n4502.0000\n4503.0000\n4504.0000\n4505.0000\n4506.0000\n4507.0000\n4508.0000\n4509.0000\n4510.0000\n4511.0000\n4512.0000\n4513.0000\n4514.0000\n4515.0000\n4516.0000\n4517.0000\n4518.0000\n4519.0000\n4520.0000\n4521.0000\n4522.0000\n4523.0000\n4524.0000\n4525.0000\n4526.0000\n4527.0000\n4528.0000\n4529.0000\n4530.0000\n4531.0000\n4532.0000\n4533.0000\n4534.0000\n4535.0000\n4536.0000\n4537.0000\n4538.0000\n4539.0000\n4540.0000\n4541.0000\n4542.0000\n4543.0000\n4544.0000\n4545.0000\n4546.0000\n4547.0000\n4548.0000\n4549.0000\n4550.0000\n4551.0000\n4552.0000\n4553.0000\n4554.0000\n4555.0000\n4556.0000\n4557.0000\n4558.0000\n4559.0000\n4560.0000\n4561.0000\n4562.0000\n4563.0000\n4564.0000\n4565.0000\n4566.0000\n4567.0000\n4568.0000\n4569.0000\n4570.0000\n4571.0000\n4572.0000\n4573.0000\n4574.0000\n4575.0000\n4576.0000\n4577.0000\n4578.0000\n4579.0000\n4580.0000\n4581.0000\n4582.0000\n4583.0000\n4584.0000\n4585.0000\n4586.0000\n4587.0000\n4588.0000\n4589.0000\n4590.0000\n4591.0000\n4592.0000\n4593.0000\n4594.0000\n4595.0000\n4596.0000\n4597.0000\n4598.0000\n4599.0000\n4600.0000\n4601.0000\n4602.0000\n4603.0000\n4604.0000\n4605.0000\n4606.0000\n4607.0000\n4608.0000\n4609.0000\n4610.0000\n4611.0000\n4612.0000\n4613.0000\n4614.0000\n4615.0000\n4616.0000\n4617.0000\n4618.0000\n4619.0000\n4620.0000\n4621.0000\n4622.0000\n4623.0000\n4624.0000\n4625.0000\n4626.0000\n4627.0000\n4628.0000\n4629.0000\n4630.0000\n4631.0000\n4632.0000\n4633.0000\n4634.0000\n4635.0000\n4636.0000\n4637.0000\n4638.0000\n4639.0000\n4640.0000\n4641.0000\n4642.0000\n4643.0000\n4644.0000\n4645.0000\n4646.0000\n4647.0000\n4648.0000\n4649.0000\n4650.0000\n4651.0000\n4652.0000\n4653.0000\n4654.0000\n4655.0000\n4656.0000\n4657.0000\n4658.0000\n4659.0000\n4660.0000\n4661.0000\n4662.0000\n4663.0000\n4664.0000\n4665.0000\n4666.0000\n4667.0000\n4668.0000\n4669.0000\n4670.0000\n4671.0000\n4672.0000\n4673.0000\n4674.0000\n4675.0000\n4676.0000\n4677.0000\n4678.0000\n4679.0000\n4680.0000\n4681.0000\n4682.0000\n4683.0000\n4684.0000\n4685.0000\n4686.0000\n4687.0000\n4688.0000\n4689.0000\n4690.0000\n4691.0000\n4692.0000\n4693.0000\n4694.0000\n4695.0000\n4696.0000\n4697.0000\n4698.0000\n4699.0000\n4700.0000\n4701.0000\n4702.0000\n4703.0000\n4704.0000\n4705.0000\n4706.0000\n4707.0000\n4708.0000\n4709.0000\n4710.0000\n4711.0000\n4712.0000\n4713.0000\n4714.0000\n4715.0000\n4716.0000\n4717.0000\n4718.0000\n4719.0000\n4720.0000\n4721.0000\n4722.0000\n4723.0000\n4724.0000\n4725.0000\n4726.0000\n4727.0000\n4728.0000\n4729.0000\n4730.0000\n4731.0000\n4732.0000\n4733.0000\n4734.0000\n4735.0000\n4736.0000\n4737.0000\n4738.0000\n4739.0000\n4740.0000\n4741.0000\n4742.0000\n4743.0000\n4744.0000\n4745.0000\n4746.0000\n4747.0000\n4748.0000\n4749.0000\n4750.0000\n4751.0000\n4752.0000\n4753.0000\n4754.0000\n4755.0000\n4756.0000\n4757.0000\n4758.0000\n4759.0000\n4760.0000\n4761.0000\n4762.0000\n4763.0000\n4764.0000\n4765.0000\n4766.0000\n4767.0000\n4768.0000\n4769.0000\n4770.0000\n4771.0000\n4772.0000\n4773.0000\n4774.0000\n4775.0000\n4776.0000\n4777.0000\n4778.0000\n4779.0000\n4780.0000\n4781.0000\n4782.0000\n4783.0000\n4784.0000\n4785.0000\n4786.0000\n4787.0000\n4788.0000\n4789.0000\n4790.0000\n4791.0000\n4792.0000\n4793.0000\n4794.0000\n4795.0000\n4796.0000\n4797.0000\n4798.0000\n4799.0000\n4800.0000\n4801.0000\n4802.0000\n4803.0000\n4804.0000\n4805.0000\n4806.0000\n4807.0000\n4808.0000\n4809.0000\n4810.0000\n4811.0000\n4812.0000\n4813.0000\n4814.0000\n4815.0000\n4816.0000\n4817.0000\n4818.0000\n4819.0000\n4820.0000\n4821.0000\n4822.0000\n4823.0000\n4824.0000\n4825.0000\n4826.0000\n4827.0000\n4828.0000\n4829.0000\n4830.0000\n4831.0000\n4832.0000\n4833.0000\n4834.0000\n4835.0000\n4836.0000\n4837.0000\n4838.0000\n4839.0000\n4840.0000\n4841.0000\n4842.0000\n4843.0000\n4844.0000\n4845.0000\n4846.0000\n4847.0000\n4848.0000\n4849.0000\n4850.0000\n4851.0000\n4852.0000\n4853.0000\n4854.0000\n4855.0000\n4856.0000\n4857.0000\n4858.0000\n4859.0000\n4860.0000\n4861.0000\n4862.0000\n4863.0000\n4864.0000\n4865.0000\n4866.0000\n4867.0000\n4868.0000\n4869.0000\n4870.0000\n4871.0000\n4872.0000\n4873.0000\n4874.0000\n4875.0000\n4876.0000\n4877.0000\n4878.0000\n4879.0000\n4880.0000\n4881.0000\n4882.0000\n4883.0000\n4884.0000\n4885.0000\n4886.0000\n4887.0000\n4888.0000\n4889.0000\n4890.0000\n4891.0000\n4892.0000\n4893.0000\n4894.0000\n4895.0000\n4896.0000\n4897.0000\n4898.0000\n4899.0000\n4900.0000\n4901.0000\n4902.0000\n4903.0000\n4904.0000\n4905.0000\n4906.0000\n4907.0000\n4908.0000\n4909.0000\n4910.0000\n4911.0000\n4912.0000\n4913.0000\n4914.0000\n4915.0000\n4916.0000\n4917.0000\n4918.0000\n4919.0000\n4920.0000\n4921.0000\n4922.0000\n4923.0000\n4924.0000\n4925.0000\n4926.0000\n4927.0000\n4928.0000\n4929.0000\n4930.0000\n4931.0000\n4932.0000\n4933.0000\n4934.0000\n4935.0000\n4936.0000\n4937.0000\n4938.0000\n4939.0000\n4940.0000\n4941.0000\n4942.0000\n4943.0000\n4944.0000\n4945.0000\n4946.0000\n4947.0000\n4948.0000\n4949.0000\n4950.0000\n4951.0000\n4952.0000\n4953.0000\n4954.0000\n4955.0000\n4956.0000\n4957.0000\n4958.0000\n4959.0000\n4960.0000\n4961.0000\n4962.0000\n4963.0000\n4964.0000\n4965.0000\n4966.0000\n4967.0000\n4968.0000\n4969.0000\n4970.0000\n4971.0000\n4972.0000\n4973.0000\n4974.0000\n4975.0000\n4976.0000\n4977.0000\n4978.0000\n4979.0000\n4980.0000\n4981.0000\n4982.0000\n4983.0000\n4984.0000\n4985.0000\n4986.0000\n4987.0000\n4988.0000\n4989.0000\n4990.0000\n4991.0000\n4992.0000\n4993.0000\n4994.0000\n4995.0000\n4996.0000\n4997.0000\n4998.0000\n4999.0000\n5000.0000\n5001.0000\n5002.0000\n5003.0000\n5004.0000\n5005.0000\n5006.0000\n5007.0000\n5008.0000\n5009.0000\n5010.0000\n5011.0000\n5012.0000\n5013.0000\n5014.0000\n5015.0000\n5016.0000\n5017.0000\n5018.0000\n5019.0000\n5020.0000\n5021.0000\n5022.0000\n5023.0000\n5024.0000\n5025.0000\n5026.0000\n5027.0000\n5028.0000\n5029.0000\n5030.0000\n5031.0000\n5032.0000\n5033.0000\n5034.0000\n5035.0000\n5036.0000\n5037.0000\n5038.0000\n5039.0000\n5040.0000\n5041.0000\n5042.0000\n5043.0000\n5044.0000\n5045.0000\n5046.0000\n5047.0000\n5048.0000\n5049.0000\n5050.0000\n5051.0000\n5052.0000\n5053.0000\n5054.0000\n5055.0000\n5056.0000\n5057.0000\n5058.0000\n5059.0000\n5060.0000\n5061.0000\n5062.0000\n5063.0000\n5064.0000\n5065.0000\n5066.0000\n5067.0000\n5068.0000\n5069.0000\n5070.0000\n5071.0000\n5072.0000\n5073.0000\n5074.0000\n5075.0000\n5076.0000\n5077.0000\n5078.0000\n5079.0000\n5080.0000\n5081.0000\n5082.0000\n5083.0000\n5084.0000\n5085.0000\n5086.0000\n5087.0000\n5088.0000\n5089.0000\n5090.0000\n5091.0000\n5092.0000\n5093.0000\n5094.0000\n5095.0000\n5096.0000\n5097.0000\n5098.0000\n5099.0000\n5100.0000\n5101.0000\n5102.0000\n5103.0000\n5104.0000\n5105.0000\n5106.0000\n5107.0000\n5108.0000\n5109.0000\n5110.0000\n5111.0000\n5112.0000\n5113.0000\n5114.0000\n5115.0000\n5116.0000\n5117.0000\n5118.0000\n5119.0000\n5120.0000\n5121.0000\n5122.0000\n5123.0000\n5124.0000\n5125.0000\n5126.0000\n5127.0000\n5128.0000\n5129.0000\n5130.0000\n5131.0000\n5132.0000\n5133.0000\n5134.0000\n5135.0000\n5136.0000\n5137.0000\n5138.0000\n5139.0000\n5140.0000\n5141.0000\n5142.0000\n5143.0000\n5144.0000\n5145.0000\n5146.0000\n5147.0000\n5148.0000\n5149.0000\n5150.0000\n5151.0000\n5152.0000\n5153.0000\n5154.0000\n5155.0000\n5156.0000\n5157.0000\n5158.0000\n5159.0000\n5160.0000\n5161.0000\n5162.0000\n5163.0000\n5164.0000\n5165.0000\n5166.0000\n5167.0000\n5168.0000\n5169.0000\n5170.0000\n5171.0000\n5172.0000\n5173.0000\n5174.0000\n5175.0000\n5176.0000\n5177.0000\n5178.0000\n5179.0000\n5180.0000\n5181.0000\n5182.0000\n5183.0000\n5184.0000\n5185.0000\n5186.0000\n5187.0000\n5188.0000\n5189.0000\n5190.0000\n5191.0000\n5192.0000\n5193.0000\n5194.0000\n5195.0000\n5196.0000\n5197.0000\n5198.0000\n5199.0000\n5200.0000\n5201.0000\n5202.0000\n5203.0000\n5204.0000\n5205.0000\n5206.0000\n5207.0000\n5208.0000\n5209.0000\n5210.0000\n5211.0000\n5212.0000\n5213.0000\n5214.0000\n5215.0000\n5216.0000\n5217.0000\n5218.0000\n5219.0000\n5220.0000\n5221.0000\n5222.0000\n5223.0000\n5224.0000\n5225.0000\n5226.0000\n5227.0000\n5228.0000\n5229.0000\n5230.0000\n5231.0000\n5232.0000\n5233.0000\n5234.0000\n5235.0000\n5236.0000\n5237.0000\n5238.0000\n5239.0000\n5240.0000\n5241.0000\n5242.0000\n5243.0000\n5244.0000\n5245.0000\n5246.0000\n5247.0000\n5248.0000\n5249.0000\n5250.0000\n5251.0000\n5252.0000\n5253.0000\n5254.0000\n5255.0000\n5256.0000\n5257.0000\n5258.0000\n5259.0000\n5260.0000\n5261.0000\n5262.0000\n5263.0000\n5264.0000\n5265.0000\n5266.0000\n5267.0000\n5268.0000\n5269.0000\n5270.0000\n5271.0000\n5272.0000\n5273.0000\n5274.0000\n5275.0000\n5276.0000\n5277.0000\n5278.0000\n5279.0000\n5280.0000\n5281.0000\n5282.0000\n5283.0000\n5284.0000\n5285.0000\n5286.0000\n5287.0000\n5288.0000\n5289.0000\n5290.0000\n5291.0000\n5292.0000\n5293.0000\n5294.0000\n5295.0000\n5296.0000\n5297.0000\n5298.0000\n5299.0000\n5300.0000\n5301.0000\n5302.0000\n5303.0000\n5304.0000\n5305.0000\n5306.0000\n5307.0000\n5308.0000\n5309.0000\n5310.0000\n5311.0000\n5312.0000\n5313.0000\n5314.0000\n5315.0000\n5316.0000\n5317.0000\n5318.0000\n5319.0000\n5320.0000\n5321.0000\n5322.0000\n5323.0000\n5324.0000\n5325.0000\n5326.0000\n5327.0000\n5328.0000\n5329.0000\n5330.0000\n5331.0000\n5332.0000\n5333.0000\n5334.0000\n5335.0000\n5336.0000\n5337.0000\n5338.0000\n5339.0000\n5340.0000\n5341.0000\n5342.0000\n5343.0000\n5344.0000\n5345.0000\n5346.0000\n5347.0000\n5348.0000\n5349.0000\n5350.0000\n5351.0000\n5352.0000\n5353.0000\n5354.0000\n5355.0000\n5356.0000\n5357.0000\n5358.0000\n5359.0000\n5360.0000\n5361.0000\n5362.0000\n5363.0000\n5364.0000\n5365.0000\n5366.0000\n5367.0000\n5368.0000\n5369.0000\n5370.0000\n5371.0000\n5372.0000\n5373.0000\n5374.0000\n5375.0000\n5376.0000\n5377.0000\n5378.0000\n5379.0000\n5380.0000\n5381.0000\n5382.0000\n5383.0000\n5384.0000\n5385.0000\n5386.0000\n5387.0000\n5388.0000\n5389.0000\n5390.0000\n5391.0000\n5392.0000\n5393.0000\n5394.0000\n5395.0000\n5396.0000\n5397.0000\n5398.0000\n5399.0000\n5400.0000\n5401.0000\n5402.0000\n5403.0000\n5404.0000\n5405.0000\n5406.0000\n5407.0000\n5408.0000\n5409.0000\n5410.0000\n5411.0000\n5412.0000\n5413.0000\n5414.0000\n5415.0000\n5416.0000\n5417.0000\n5418.0000\n5419.0000\n5420.0000\n5421.0000\n5422.0000\n5423.0000\n5424.0000\n5425.0000\n5426.0000\n5427.0000\n5428.0000\n5429.0000\n5430.0000\n5431.0000\n5432.0000\n5433.0000\n5434.0000\n5435.0000\n5436.0000\n5437.0000\n5438.0000\n5439.0000\n5440.0000\n5441.0000\n5442.0000\n5443.0000\n5444.0000\n5445.0000\n5446.0000\n5447.0000\n5448.0000\n5449.0000\n5450.0000\n5451.0000\n5452.0000\n5453.0000\n5454.0000\n5455.0000\n5456.0000\n5457.0000\n5458.0000\n5459.0000\n5460.0000\n5461.0000\n5462.0000\n5463.0000\n5464.0000\n5465.0000\n5466.0000\n5467.0000\n5468.0000\n5469.0000\n5470.0000\n5471.0000\n5472.0000\n5473.0000\n5474.0000\n5475.0000\n5476.0000\n5477.0000\n5478.0000\n5479.0000\n5480.0000\n5481.0000\n5482.0000\n5483.0000\n5484.0000\n5485.0000\n5486.0000\n5487.0000\n5488.0000\n5489.0000\n5490.0000\n5491.0000\n5492.0000\n5493.0000\n5494.0000\n5495.0000\n5496.0000\n5497.0000\n5498.0000\n5499.0000\n5500.0000\n5501.0000\n5502.0000\n5503.0000\n5504.0000\n5505.0000\n5506.0000\n5507.0000\n5508.0000\n5509.0000\n5510.0000\n5511.0000\n5512.0000\n5513.0000\n5514.0000\n5515.0000\n5516.0000\n5517.0000\n5518.0000\n5519.0000\n5520.0000\n5521.0000\n5522.0000\n5523.0000\n5524.0000\n5525.0000\n5526.0000\n5527.0000\n5528.0000\n5529.0000\n5530.0000\n5531.0000\n5532.0000\n5533.0000\n5534.0000\n5535.0000\n5536.0000\n5537.0000\n5538.0000\n5539.0000\n5540.0000\n5541.0000\n5542.0000\n5543.0000\n5544.0000\n5545.0000\n5546.0000\n5547.0000\n5548.0000\n5549.0000\n5550.0000\n5551.0000\n5552.0000\n5553.0000\n5554.0000\n5555.0000\n5556.0000\n5557.0000\n5558.0000\n5559.0000\n5560.0000\n5561.0000\n5562.0000\n5563.0000\n5564.0000\n5565.0000\n5566.0000\n5567.0000\n5568.0000\n5569.0000\n5570.0000\n5571.0000\n5572.0000\n5573.0000\n5574.0000\n5575.0000\n5576.0000\n5577.0000\n5578.0000\n5579.0000\n5580.0000\n5581.0000\n5582.0000\n5583.0000\n5584.0000\n5585.0000\n5586.0000\n5587.0000\n5588.0000\n5589.0000\n5590.0000\n5591.0000\n5592.0000\n5593.0000\n5594.0000\n5595.0000\n5596.0000\n5597.0000\n5598.0000\n5599.0000\n5600.0000\n5601.0000\n5602.0000\n5603.0000\n5604.0000\n5605.0000\n5606.0000\n5607.0000\n5608.0000\n5609.0000\n5610.0000\n5611.0000\n5612.0000\n5613.0000\n5614.0000\n5615.0000\n5616.0000\n5617.0000\n5618.0000\n5619.0000\n5620.0000\n5621.0000\n5622.0000\n5623.0000\n5624.0000\n5625.0000\n5626.0000\n5627.0000\n5628.0000\n5629.0000\n5630.0000\n5631.0000\n5632.0000\n5633.0000\n5634.0000\n5635.0000\n5636.0000\n5637.0000\n5638.0000\n5639.0000\n5640.0000\n5641.0000\n5642.0000\n5643.0000\n5644.0000\n5645.0000\n5646.0000\n5647.0000\n5648.0000\n5649.0000\n5650.0000\n5651.0000\n5652.0000\n5653.0000\n5654.0000\n5655.0000\n5656.0000\n5657.0000\n5658.0000\n5659.0000\n5660.0000\n5661.0000\n5662.0000\n5663.0000\n5664.0000\n5665.0000\n5666.0000\n5667.0000\n5668.0000\n5669.0000\n5670.0000\n5671.0000\n5672.0000\n5673.0000\n5674.0000\n5675.0000\n5676.0000\n5677.0000\n5678.0000\n5679.0000\n5680.0000\n5681.0000\n5682.0000\n5683.0000\n5684.0000\n5685.0000\n5686.0000\n5687.0000\n5688.0000\n5689.0000\n5690.0000\n5691.0000\n5692.0000\n5693.0000\n5694.0000\n5695.0000\n5696.0000\n5697.0000\n5698.0000\n5699.0000\n5700.0000\n5701.0000\n5702.0000\n5703.0000\n5704.0000\n5705.0000\n5706.0000\n5707.0000\n5708.0000\n5709.0000\n5710.0000\n5711.0000\n5712.0000\n5713.0000\n5714.0000\n5715.0000\n5716.0000\n5717.0000\n5718.0000\n5719.0000\n5720.0000\n5721.0000\n5722.0000\n5723.0000\n5724.0000\n5725.0000\n5726.0000\n5727.0000\n5728.0000\n5729.0000\n5730.0000\n5731.0000\n5732.0000\n5733.0000\n5734.0000\n5735.0000\n5736.0000\n5737.0000\n5738.0000\n5739.0000\n5740.0000\n5741.0000\n5742.0000\n5743.0000\n5744.0000\n5745.0000\n5746.0000\n5747.0000\n5748.0000\n5749.0000\n5750.0000\n5751.0000\n5752.0000\n5753.0000\n5754.0000\n5755.0000\n5756.0000\n5757.0000\n5758.0000\n5759.0000\n5760.0000\n5761.0000\n5762.0000\n5763.0000\n5764.0000\n5765.0000\n5766.0000\n5767.0000\n5768.0000\n5769.0000\n5770.0000\n5771.0000\n5772.0000\n5773.0000\n5774.0000\n5775.0000\n5776.0000\n5777.0000\n5778.0000\n5779.0000\n5780.0000\n5781.0000\n5782.0000\n5783.0000\n5784.0000\n5785.0000\n5786.0000\n5787.0000\n5788.0000\n5789.0000\n5790.0000\n5791.0000\n5792.0000\n5793.0000\n5794.0000\n5795.0000\n5796.0000\n5797.0000\n5798.0000\n5799.0000\n5800.0000\n5801.0000\n5802.0000\n5803.0000\n5804.0000\n5805.0000\n5806.0000\n5807.0000\n5808.0000\n5809.0000\n5810.0000\n5811.0000\n5812.0000\n5813.0000\n5814.0000\n5815.0000\n5816.0000\n5817.0000\n5818.0000\n5819.0000\n5820.0000\n5821.0000\n5822.0000\n5823.0000\n5824.0000\n5825.0000\n5826.0000\n5827.0000\n5828.0000\n5829.0000\n5830.0000\n5831.0000\n5832.0000\n5833.0000\n5834.0000\n5835.0000\n5836.0000\n5837.0000\n5838.0000\n5839.0000\n5840.0000\n5841.0000\n5842.0000\n5843.0000\n5844.0000\n5845.0000\n5846.0000\n5847.0000\n5848.0000\n5849.0000\n5850.0000\n5851.0000\n5852.0000\n5853.0000\n5854.0000\n5855.0000\n5856.0000\n5857.0000\n5858.0000\n5859.0000\n5860.0000\n5861.0000\n5862.0000\n5863.0000\n5864.0000\n5865.0000\n5866.0000\n5867.0000\n5868.0000\n5869.0000\n5870.0000\n5871.0000\n5872.0000\n5873.0000\n5874.0000\n5875.0000\n5876.0000\n5877.0000\n5878.0000\n5879.0000\n5880.0000\n5881.0000\n5882.0000\n5883.0000\n5884.0000\n5885.0000\n5886.0000\n5887.0000\n5888.0000\n5889.0000\n5890.0000\n5891.0000\n5892.0000\n5893.0000\n5894.0000\n5895.0000\n5896.0000\n5897.0000\n5898.0000\n5899.0000\n5900.0000\n5901.0000\n5902.0000\n5903.0000\n5904.0000\n5905.0000\n5906.0000\n5907.0000\n5908.0000\n5909.0000\n5910.0000\n5911.0000\n5912.0000\n5913.0000\n5914.0000\n5915.0000\n5916.0000\n5917.0000\n5918.0000\n5919.0000\n5920.0000\n5921.0000\n5922.0000\n5923.0000\n5924.0000\n5925.0000\n5926.0000\n5927.0000\n5928.0000\n5929.0000\n5930.0000\n5931.0000\n5932.0000\n5933.0000\n5934.0000\n5935.0000\n5936.0000\n5937.0000\n5938.0000\n5939.0000\n5940.0000\n5941.0000\n5942.0000\n5943.0000\n5944.0000\n5945.0000\n5946.0000\n5947.0000\n5948.0000\n5949.0000\n5950.0000\n5951.0000\n5952.0000\n5953.0000\n5954.0000\n5955.0000\n5956.0000\n5957.0000\n5958.0000\n5959.0000\n5960.0000\n5961.0000\n5962.0000\n5963.0000\n5964.0000\n5965.0000\n5966.0000\n5967.0000\n5968.0000\n5969.0000\n5970.0000\n5971.0000\n5972.0000\n5973.0000\n5974.0000\n5975.0000\n5976.0000\n5977.0000\n5978.0000\n5979.0000\n5980.0000\n5981.0000\n5982.0000\n5983.0000\n5984.0000\n5985.0000\n5986.0000\n5987.0000\n5988.0000\n5989.0000\n5990.0000\n5991.0000\n5992.0000\n5993.0000\n5994.0000\n5995.0000\n5996.0000\n5997.0000\n5998.0000\n5999.0000\n6000.0000\n6001.0000\n6002.0000\n6003.0000\n6004.0000\n6005.0000\n6006.0000\n6007.0000\n6008.0000\n6009.0000\n6010.0000\n6011.0000\n6012.0000\n6013.0000\n6014.0000\n6015.0000\n6016.0000\n6017.0000\n6018.0000\n6019.0000\n6020.0000\n6021.0000\n6022.0000\n6023.0000\n6024.0000\n6025.0000\n6026.0000\n6027.0000\n6028.0000\n6029.0000\n6030.0000\n6031.0000\n6032.0000\n6033.0000\n6034.0000\n6035.0000\n6036.0000\n6037.0000\n6038.0000\n6039.0000\n6040.0000\n6041.0000\n6042.0000\n6043.0000\n6044.0000\n6045.0000\n6046.0000\n6047.0000\n6048.0000\n6049.0000\n6050.0000\n6051.0000\n6052.0000\n6053.0000\n6054.0000\n6055.0000\n6056.0000\n6057.0000\n6058.0000\n6059.0000\n6060.0000\n6061.0000\n6062.0000\n6063.0000\n6064.0000\n6065.0000\n6066.0000\n6067.0000\n6068.0000\n6069.0000\n6070.0000\n6071.0000\n6072.0000\n6073.0000\n6074.0000\n6075.0000\n6076.0000\n6077.0000\n6078.0000\n6079.0000\n6080.0000\n6081.0000\n6082.0000\n6083.0000\n6084.0000\n6085.0000\n6086.0000\n6087.0000\n6088.0000\n6089.0000\n6090.0000\n6091.0000\n6092.0000\n6093.0000\n6094.0000\n6095.0000\n6096.0000\n6097.0000\n6098.0000\n6099.0000\n6100.0000\n6101.0000\n6102.0000\n6103.0000\n6104.0000\n6105.0000\n6106.0000\n6107.0000\n6108.0000\n6109.0000\n6110.0000\n6111.0000\n6112.0000\n6113.0000\n6114.0000\n6115.0000\n6116.0000\n6117.0000\n6118.0000\n6119.0000\n6120.0000\n6121.0000\n6122.0000\n6123.0000\n6124.0000\n6125.0000\n6126.0000\n6127.0000\n6128.0000\n6129.0000\n6130.0000\n6131.0000\n6132.0000\n6133.0000\n6134.0000\n6135.0000\n6136.0000\n6137.0000\n6138.0000\n6139.0000\n6140.0000\n6141.0000\n6142.0000\n6143.0000\n6144.0000\n6145.0000\n6146.0000\n6147.0000\n6148.0000\n6149.0000\n6150.0000\n6151.0000\n6152.0000\n6153.0000\n6154.0000\n6155.0000\n6156.0000\n6157.0000\n6158.0000\n6159.0000\n6160.0000\n6161.0000\n6162.0000\n6163.0000\n6164.0000\n6165.0000\n6166.0000\n6167.0000\n6168.0000\n6169.0000\n6170.0000\n6171.0000\n6172.0000\n6173.0000\n6174.0000\n6175.0000\n6176.0000\n6177.0000\n6178.0000\n6179.0000\n6180.0000\n6181.0000\n6182.0000\n6183.0000\n6184.0000\n6185.0000\n6186.0000\n6187.0000\n6188.0000\n6189.0000\n6190.0000\n6191.0000\n6192.0000\n6193.0000\n6194.0000\n6195.0000\n6196.0000\n6197.0000\n6198.0000\n6199.0000\n6200.0000\n6201.0000\n6202.0000\n6203.0000\n6204.0000\n6205.0000\n6206.0000\n6207.0000\n6208.0000\n6209.0000\n6210.0000\n6211.0000\n6212.0000\n6213.0000\n6214.0000\n6215.0000\n6216.0000\n6217.0000\n6218.0000\n6219.0000\n6220.0000\n6221.0000\n6222.0000\n6223.0000\n6224.0000\n6225.0000\n6226.0000\n6227.0000\n6228.0000\n6229.0000\n6230.0000\n6231.0000\n6232.0000\n6233.0000\n6234.0000\n6235.0000\n6236.0000\n6237.0000\n6238.0000\n6239.0000\n6240.0000\n6241.0000\n6242.0000\n6243.0000\n6244.0000\n6245.0000\n6246.0000\n6247.0000\n6248.0000\n6249.0000\n6250.0000\n6251.0000\n6252.0000\n6253.0000\n6254.0000\n6255.0000\n6256.0000\n6257.0000\n6258.0000\n6259.0000\n6260.0000\n6261.0000\n6262.0000\n6263.0000\n6264.0000\n6265.0000\n6266.0000\n6267.0000\n6268.0000\n6269.0000\n6270.0000\n6271.0000\n6272.0000\n6273.0000\n6274.0000\n6275.0000\n6276.0000\n6277.0000\n6278.0000\n6279.0000\n6280.0000\n6281.0000\n6282.0000\n6283.0000\n6284.0000\n6285.0000\n6286.0000\n6287.0000\n6288.0000\n6289.0000\n6290.0000\n6291.0000\n6292.0000\n6293.0000\n6294.0000\n6295.0000\n6296.0000\n6297.0000\n6298.0000\n6299.0000\n6300.0000\n6301.0000\n6302.0000\n6303.0000\n6304.0000\n6305.0000\n6306.0000\n6307.0000\n6308.0000\n6309.0000\n6310.0000\n6311.0000\n6312.0000\n6313.0000\n6314.0000\n6315.0000\n6316.0000\n6317.0000\n6318.0000\n6319.0000\n6320.0000\n6321.0000\n6322.0000\n6323.0000\n6324.0000\n6325.0000\n6326.0000\n6327.0000\n6328.0000\n6329.0000\n6330.0000\n6331.0000\n6332.0000\n6333.0000\n6334.0000\n6335.0000\n6336.0000\n6337.0000\n6338.0000\n6339.0000\n6340.0000\n6341.0000\n6342.0000\n6343.0000\n6344.0000\n6345.0000\n6346.0000\n6347.0000\n6348.0000\n6349.0000\n6350.0000\n6351.0000\n6352.0000\n6353.0000\n6354.0000\n6355.0000\n6356.0000\n6357.0000\n6358.0000\n6359.0000\n6360.0000\n6361.0000\n6362.0000\n6363.0000\n6364.0000\n6365.0000\n6366.0000\n6367.0000\n6368.0000\n6369.0000\n6370.0000\n6371.0000\n6372.0000\n6373.0000\n6374.0000\n6375.0000\n6376.0000\n6377.0000\n6378.0000\n6379.0000\n6380.0000\n6381.0000\n6382.0000\n6383.0000\n6384.0000\n6385.0000\n6386.0000\n6387.0000\n6388.0000\n6389.0000\n6390.0000\n6391.0000\n6392.0000\n6393.0000\n6394.0000\n6395.0000\n6396.0000\n6397.0000\n6398.0000\n6399.0000\n6400.0000\n6401.0000\n6402.0000\n6403.0000\n6404.0000\n6405.0000\n6406.0000\n6407.0000\n6408.0000\n6409.0000\n6410.0000\n6411.0000\n6412.0000\n6413.0000\n6414.0000\n6415.0000\n6416.0000\n6417.0000\n6418.0000\n6419.0000\n6420.0000\n6421.0000\n6422.0000\n6423.0000\n6424.0000\n6425.0000\n6426.0000\n6427.0000\n6428.0000\n6429.0000\n6430.0000\n6431.0000\n6432.0000\n6433.0000\n6434.0000\n6435.0000\n6436.0000\n6437.0000\n6438.0000\n6439.0000\n6440.0000\n6441.0000\n6442.0000\n6443.0000\n6444.0000\n6445.0000\n6446.0000\n6447.0000\n6448.0000\n6449.0000\n6450.0000\n6451.0000\n6452.0000\n6453.0000\n6454.0000\n6455.0000\n6456.0000\n6457.0000\n6458.0000\n6459.0000\n6460.0000\n6461.0000\n6462.0000\n6463.0000\n6464.0000\n6465.0000\n6466.0000\n6467.0000\n6468.0000\n6469.0000\n6470.0000\n6471.0000\n6472.0000\n6473.0000\n6474.0000\n6475.0000\n6476.0000\n6477.0000\n6478.0000\n6479.0000\n6480.0000\n6481.0000\n6482.0000\n6483.0000\n6484.0000\n6485.0000\n6486.0000\n6487.0000\n6488.0000\n6489.0000\n6490.0000\n6491.0000\n6492.0000\n6493.0000\n6494.0000\n6495.0000\n6496.0000\n6497.0000\n6498.0000\n6499.0000\n6500.0000\n6501.0000\n6502.0000\n6503.0000\n6504.0000\n6505.0000\n6506.0000\n6507.0000\n6508.0000\n6509.0000\n6510.0000\n6511.0000\n6512.0000\n6513.0000\n6514.0000\n6515.0000\n6516.0000\n6517.0000\n6518.0000\n6519.0000\n6520.0000\n6521.0000\n6522.0000\n6523.0000\n6524.0000\n6525.0000\n6526.0000\n6527.0000\n6528.0000\n6529.0000\n6530.0000\n6531.0000\n6532.0000\n6533.0000\n6534.0000\n6535.0000\n6536.0000\n6537.0000\n6538.0000\n6539.0000\n6540.0000\n6541.0000\n6542.0000\n6543.0000\n6544.0000\n6545.0000\n6546.0000\n6547.0000\n6548.0000\n6549.0000\n6550.0000\n6551.0000\n6552.0000\n6553.0000\n6554.0000\n6555.0000\n6556.0000\n6557.0000\n6558.0000\n6559.0000\n6560.0000\n6561.0000\n6562.0000\n6563.0000\n6564.0000\n6565.0000\n6566.0000\n6567.0000\n6568.0000\n6569.0000\n6570.0000\n6571.0000\n6572.0000\n6573.0000\n6574.0000\n6575.0000\n6576.0000\n6577.0000\n6578.0000\n6579.0000\n6580.0000\n6581.0000\n6582.0000\n6583.0000\n6584.0000\n6585.0000\n6586.0000\n6587.0000\n6588.0000\n6589.0000\n6590.0000\n6591.0000\n6592.0000\n6593.0000\n6594.0000\n6595.0000\n6596.0000\n6597.0000\n6598.0000\n6599.0000\n6600.0000\n6601.0000\n6602.0000\n6603.0000\n6604.0000\n6605.0000\n6606.0000\n6607.0000\n6608.0000\n6609.0000\n6610.0000\n6611.0000\n6612.0000\n6613.0000\n6614.0000\n6615.0000\n6616.0000\n6617.0000\n6618.0000\n6619.0000\n6620.0000\n6621.0000\n6622.0000\n6623.0000\n6624.0000\n6625.0000\n6626.0000\n6627.0000\n6628.0000\n6629.0000\n6630.0000\n6631.0000\n6632.0000\n6633.0000\n6634.0000\n6635.0000\n6636.0000\n6637.0000\n6638.0000\n6639.0000\n6640.0000\n6641.0000\n6642.0000\n6643.0000\n6644.0000\n6645.0000\n6646.0000\n6647.0000\n6648.0000\n6649.0000\n6650.0000\n6651.0000\n6652.0000\n6653.0000\n6654.0000\n6655.0000\n6656.0000\n6657.0000\n6658.0000\n6659.0000\n6660.0000\n6661.0000\n6662.0000\n6663.0000\n6664.0000\n6665.0000\n6666.0000\n6667.0000\n6668.0000\n6669.0000\n6670.0000\n6671.0000\n6672.0000\n6673.0000\n6674.0000\n6675.0000\n6676.0000\n6677.0000\n6678.0000\n6679.0000\n6680.0000\n6681.0000\n6682.0000\n6683.0000\n6684.0000\n6685.0000\n6686.0000\n6687.0000\n6688.0000\n6689.0000\n6690.0000\n6691.0000\n6692.0000\n6693.0000\n6694.0000\n6695.0000\n6696.0000\n6697.0000\n6698.0000\n6699.0000\n6700.0000\n6701.0000\n6702.0000\n6703.0000\n6704.0000\n6705.0000\n6706.0000\n6707.0000\n6708.0000\n6709.0000\n6710.0000\n6711.0000\n6712.0000\n6713.0000\n6714.0000\n6715.0000\n6716.0000\n6717.0000\n6718.0000\n6719.0000\n6720.0000\n6721.0000\n6722.0000\n6723.0000\n6724.0000\n6725.0000\n6726.0000\n6727.0000\n6728.0000\n6729.0000\n6730.0000\n6731.0000\n6732.0000\n6733.0000\n6734.0000\n6735.0000\n6736.0000\n6737.0000\n6738.0000\n6739.0000\n6740.0000\n6741.0000\n6742.0000\n6743.0000\n6744.0000\n6745.0000\n6746.0000\n6747.0000\n6748.0000\n6749.0000\n6750.0000\n6751.0000\n6752.0000\n6753.0000\n6754.0000\n6755.0000\n6756.0000\n6757.0000\n6758.0000\n6759.0000\n6760.0000\n6761.0000\n6762.0000\n6763.0000\n6764.0000\n6765.0000\n6766.0000\n6767.0000\n6768.0000\n6769.0000\n6770.0000\n6771.0000\n6772.0000\n6773.0000\n6774.0000\n6775.0000\n6776.0000\n6777.0000\n6778.0000\n6779.0000\n6780.0000\n6781.0000\n6782.0000\n6783.0000\n6784.0000\n6785.0000\n6786.0000\n6787.0000\n6788.0000\n6789.0000\n6790.0000\n6791.0000\n6792.0000\n6793.0000\n6794.0000\n6795.0000\n6796.0000\n6797.0000\n6798.0000\n6799.0000\n6800.0000\n6801.0000\n6802.0000\n6803.0000\n6804.0000\n6805.0000\n6806.0000\n6807.0000\n6808.0000\n6809.0000\n6810.0000\n6811.0000\n6812.0000\n6813.0000\n6814.0000\n6815.0000\n6816.0000\n6817.0000\n6818.0000\n6819.0000\n6820.0000\n6821.0000\n6822.0000\n6823.0000\n6824.0000\n6825.0000\n6826.0000\n6827.0000\n6828.0000\n6829.0000\n6830.0000\n6831.0000\n6832.0000\n6833.0000\n6834.0000\n6835.0000\n6836.0000\n6837.0000\n6838.0000\n6839.0000\n6840.0000\n6841.0000\n6842.0000\n6843.0000\n6844.0000\n6845.0000\n6846.0000\n6847.0000\n6848.0000\n6849.0000\n6850.0000\n6851.0000\n6852.0000\n6853.0000\n6854.0000\n6855.0000\n6856.0000\n6857.0000\n6858.0000\n6859.0000\n6860.0000\n6861.0000\n6862.0000\n6863.0000\n6864.0000\n6865.0000\n6866.0000\n6867.0000\n6868.0000\n6869.0000\n6870.0000\n6871.0000\n6872.0000\n6873.0000\n6874.0000\n6875.0000\n6876.0000\n6877.0000\n6878.0000\n6879.0000\n6880.0000\n6881.0000\n6882.0000\n6883.0000\n6884.0000\n6885.0000\n6886.0000\n6887.0000\n6888.0000\n6889.0000\n6890.0000\n6891.0000\n6892.0000\n6893.0000\n6894.0000\n6895.0000\n6896.0000\n6897.0000\n6898.0000\n6899.0000\n6900.0000\n6901.0000\n6902.0000\n6903.0000\n6904.0000\n6905.0000\n6906.0000\n6907.0000\n6908.0000\n6909.0000\n6910.0000\n6911.0000\n6912.0000\n6913.0000\n6914.0000\n6915.0000\n6916.0000\n6917.0000\n6918.0000\n6919.0000\n6920.0000\n6921.0000\n6922.0000\n6923.0000\n6924.0000\n6925.0000\n6926.0000\n6927.0000\n6928.0000\n6929.0000\n6930.0000\n6931.0000\n6932.0000\n6933.0000\n6934.0000\n6935.0000\n6936.0000\n6937.0000\n6938.0000\n6939.0000\n6940.0000\n6941.0000\n6942.0000\n6943.0000\n6944.0000\n6945.0000\n6946.0000\n6947.0000\n6948.0000\n6949.0000\n6950.0000\n6951.0000\n6952.0000\n6953.0000\n6954.0000\n6955.0000\n6956.0000\n6957.0000\n6958.0000\n6959.0000\n6960.0000\n6961.0000\n6962.0000\n6963.0000\n6964.0000\n6965.0000\n6966.0000\n6967.0000\n6968.0000\n6969.0000\n6970.0000\n6971.0000\n6972.0000\n6973.0000\n6974.0000\n6975.0000\n6976.0000\n6977.0000\n6978.0000\n6979.0000\n6980.0000\n6981.0000\n6982.0000\n6983.0000\n6984.0000\n6985.0000\n6986.0000\n6987.0000\n6988.0000\n6989.0000\n6990.0000\n6991.0000\n6992.0000\n6993.0000\n6994.0000\n6995.0000\n6996.0000\n6997.0000\n6998.0000\n6999.0000\n7000.0000\n7001.0000\n7002.0000\n7003.0000\n7004.0000\n7005.0000\n7006.0000\n7007.0000\n7008.0000\n7009.0000\n7010.0000\n7011.0000\n7012.0000\n7013.0000\n7014.0000\n7015.0000\n7016.0000\n7017.0000\n7018.0000\n7019.0000\n7020.0000\n7021.0000\n7022.0000\n7023.0000\n7024.0000\n7025.0000\n7026.0000\n7027.0000\n7028.0000\n7029.0000\n7030.0000\n7031.0000\n7032.0000\n7033.0000\n7034.0000\n7035.0000\n7036.0000\n7037.0000\n7038.0000\n7039.0000\n7040.0000\n7041.0000\n7042.0000\n7043.0000\n7044.0000\n7045.0000\n7046.0000\n7047.0000\n7048.0000\n7049.0000\n7050.0000\n7051.0000\n7052.0000\n7053.0000\n7054.0000\n7055.0000\n7056.0000\n7057.0000\n7058.0000\n7059.0000\n7060.0000\n7061.0000\n7062.0000\n7063.0000\n7064.0000\n7065.0000\n7066.0000\n7067.0000\n7068.0000\n7069.0000\n7070.0000\n7071.0000\n7072.0000\n7073.0000\n7074.0000\n7075.0000\n7076.0000\n7077.0000\n7078.0000\n7079.0000\n7080.0000\n7081.0000\n7082.0000\n7083.0000\n7084.0000\n7085.0000\n7086.0000\n7087.0000\n7088.0000\n7089.0000\n7090.0000\n7091.0000\n7092.0000\n7093.0000\n7094.0000\n7095.0000\n7096.0000\n7097.0000\n7098.0000\n7099.0000\n7100.0000\n7101.0000\n7102.0000\n7103.0000\n7104.0000\n7105.0000\n7106.0000\n7107.0000\n7108.0000\n7109.0000\n7110.0000\n7111.0000\n7112.0000\n7113.0000\n7114.0000\n7115.0000\n7116.0000\n7117.0000\n7118.0000\n7119.0000\n7120.0000\n7121.0000\n7122.0000\n7123.0000\n7124.0000\n7125.0000\n7126.0000\n7127.0000\n7128.0000\n7129.0000\n7130.0000\n7131.0000\n7132.0000\n7133.0000\n7134.0000\n7135.0000\n7136.0000\n7137.0000\n7138.0000\n7139.0000\n7140.0000\n7141.0000\n7142.0000\n7143.0000\n7144.0000\n7145.0000\n7146.0000\n7147.0000\n7148.0000\n7149.0000\n7150.0000\n7151.0000\n7152.0000\n7153.0000\n7154.0000\n7155.0000\n7156.0000\n7157.0000\n7158.0000\n7159.0000\n7160.0000\n7161.0000\n7162.0000\n7163.0000\n7164.0000\n7165.0000\n7166.0000\n7167.0000\n7168.0000\n7169.0000\n7170.0000\n7171.0000\n7172.0000\n7173.0000\n7174.0000\n7175.0000\n7176.0000\n7177.0000\n7178.0000\n7179.0000\n7180.0000\n7181.0000\n7182.0000\n7183.0000\n7184.0000\n7185.0000\n7186.0000\n7187.0000\n7188.0000\n7189.0000\n7190.0000\n7191.0000\n7192.0000\n7193.0000\n7194.0000\n7195.0000\n7196.0000\n7197.0000\n7198.0000\n7199.0000\n7200.0000\n7201.0000\n7202.0000\n7203.0000\n7204.0000\n7205.0000\n7206.0000\n7207.0000\n7208.0000\n7209.0000\n7210.0000\n7211.0000\n7212.0000\n7213.0000\n7214.0000\n7215.0000\n7216.0000\n7217.0000\n7218.0000\n7219.0000\n7220.0000\n7221.0000\n7222.0000\n7223.0000\n7224.0000\n7225.0000\n7226.0000\n7227.0000\n7228.0000\n7229.0000\n7230.0000\n7231.0000\n7232.0000\n7233.0000\n7234.0000\n7235.0000\n7236.0000\n7237.0000\n7238.0000\n7239.0000\n7240.0000\n7241.0000\n7242.0000\n7243.0000\n7244.0000\n7245.0000\n7246.0000\n7247.0000\n7248.0000\n7249.0000\n7250.0000\n7251.0000\n7252.0000\n7253.0000\n7254.0000\n7255.0000\n7256.0000\n7257.0000\n7258.0000\n7259.0000\n7260.0000\n7261.0000\n7262.0000\n7263.0000\n7264.0000\n7265.0000\n7266.0000\n7267.0000\n7268.0000\n7269.0000\n7270.0000\n7271.0000\n7272.0000\n7273.0000\n7274.0000\n7275.0000\n7276.0000\n7277.0000\n7278.0000\n7279.0000\n7280.0000\n7281.0000\n7282.0000\n7283.0000\n7284.0000\n7285.0000\n7286.0000\n7287.0000\n7288.0000\n7289.0000\n7290.0000\n7291.0000\n7292.0000\n7293.0000\n7294.0000\n7295.0000\n7296.0000\n7297.0000\n7298.0000\n7299.0000\n7300.0000\n7301.0000\n7302.0000\n7303.0000\n7304.0000\n7305.0000\n7306.0000\n7307.0000\n7308.0000\n7309.0000\n7310.0000\n7311.0000\n7312.0000\n7313.0000\n7314.0000\n7315.0000\n7316.0000\n7317.0000\n7318.0000\n7319.0000\n7320.0000\n7321.0000\n7322.0000\n7323.0000\n7324.0000\n7325.0000\n7326.0000\n7327.0000\n7328.0000\n7329.0000\n7330.0000\n7331.0000\n7332.0000\n7333.0000\n7334.0000\n7335.0000\n7336.0000\n7337.0000\n7338.0000\n7339.0000\n7340.0000\n7341.0000\n7342.0000\n7343.0000\n7344.0000\n7345.0000\n7346.0000\n7347.0000\n7348.0000\n7349.0000\n7350.0000\n7351.0000\n7352.0000\n7353.0000\n7354.0000\n7355.0000\n7356.0000\n7357.0000\n7358.0000\n7359.0000\n7360.0000\n7361.0000\n7362.0000\n7363.0000\n7364.0000\n7365.0000\n7366.0000\n7367.0000\n7368.0000\n7369.0000\n7370.0000\n7371.0000\n7372.0000\n7373.0000\n7374.0000\n7375.0000\n7376.0000\n7377.0000\n7378.0000\n7379.0000\n7380.0000\n7381.0000\n7382.0000\n7383.0000\n7384.0000\n7385.0000\n7386.0000\n7387.0000\n7388.0000\n7389.0000\n7390.0000\n7391.0000\n7392.0000\n7393.0000\n7394.0000\n7395.0000\n7396.0000\n7397.0000\n7398.0000\n7399.0000\n7400.0000\n7401.0000\n7402.0000\n7403.0000\n7404.0000\n7405.0000\n7406.0000\n7407.0000\n7408.0000\n7409.0000\n7410.0000\n7411.0000\n7412.0000\n7413.0000\n7414.0000\n7415.0000\n7416.0000\n7417.0000\n7418.0000\n7419.0000\n7420.0000\n7421.0000\n7422.0000\n7423.0000\n7424.0000\n7425.0000\n7426.0000\n7427.0000\n7428.0000\n7429.0000\n7430.0000\n7431.0000\n7432.0000\n7433.0000\n7434.0000\n7435.0000\n7436.0000\n7437.0000\n7438.0000\n7439.0000\n7440.0000\n7441.0000\n7442.0000\n7443.0000\n7444.0000\n7445.0000\n7446.0000\n7447.0000\n7448.0000\n7449.0000\n7450.0000\n7451.0000\n7452.0000\n7453.0000\n7454.0000\n7455.0000\n7456.0000\n7457.0000\n7458.0000\n7459.0000\n7460.0000\n7461.0000\n7462.0000\n7463.0000\n7464.0000\n7465.0000\n7466.0000\n7467.0000\n7468.0000\n7469.0000\n7470.0000\n7471.0000\n7472.0000\n7473.0000\n7474.0000\n7475.0000\n7476.0000\n7477.0000\n7478.0000\n7479.0000\n7480.0000\n7481.0000\n7482.0000\n7483.0000\n7484.0000\n7485.0000\n7486.0000\n7487.0000\n7488.0000\n7489.0000\n7490.0000\n7491.0000\n7492.0000\n7493.0000\n7494.0000\n7495.0000\n7496.0000\n7497.0000\n7498.0000\n7499.0000\n7500.0000\n7501.0000\n7502.0000\n7503.0000\n7504.0000\n7505.0000\n7506.0000\n7507.0000\n7508.0000\n7509.0000\n7510.0000\n7511.0000\n7512.0000\n7513.0000\n7514.0000\n7515.0000\n7516.0000\n7517.0000\n7518.0000\n7519.0000\n7520.0000\n7521.0000\n7522.0000\n7523.0000\n7524.0000\n7525.0000\n7526.0000\n7527.0000\n7528.0000\n7529.0000\n7530.0000\n7531.0000\n7532.0000\n7533.0000\n7534.0000\n7535.0000\n7536.0000\n7537.0000\n7538.0000\n7539.0000\n7540.0000\n7541.0000\n7542.0000\n7543.0000\n7544.0000\n7545.0000\n7546.0000\n7547.0000\n7548.0000\n7549.0000\n7550.0000\n7551.0000\n7552.0000\n7553.0000\n7554.0000\n7555.0000\n7556.0000\n7557.0000\n7558.0000\n7559.0000\n7560.0000\n7561.0000\n7562.0000\n7563.0000\n7564.0000\n7565.0000\n7566.0000\n7567.0000\n7568.0000\n7569.0000\n7570.0000\n7571.0000\n7572.0000\n7573.0000\n7574.0000\n7575.0000\n7576.0000\n7577.0000\n7578.0000\n7579.0000\n7580.0000\n7581.0000\n7582.0000\n7583.0000\n7584.0000\n7585.0000\n7586.0000\n7587.0000\n7588.0000\n7589.0000\n7590.0000\n7591.0000\n7592.0000\n7593.0000\n7594.0000\n7595.0000\n7596.0000\n7597.0000\n7598.0000\n7599.0000\n7600.0000\n7601.0000\n7602.0000\n7603.0000\n7604.0000\n7605.0000\n7606.0000\n7607.0000\n7608.0000\n7609.0000\n7610.0000\n7611.0000\n7612.0000\n7613.0000\n7614.0000\n7615.0000\n7616.0000\n7617.0000\n7618.0000\n7619.0000\n7620.0000\n7621.0000\n7622.0000\n7623.0000\n7624.0000\n7625.0000\n7626.0000\n7627.0000\n7628.0000\n7629.0000\n7630.0000\n7631.0000\n7632.0000\n7633.0000\n7634.0000\n7635.0000\n7636.0000\n7637.0000\n7638.0000\n7639.0000\n7640.0000\n7641.0000\n7642.0000\n7643.0000\n7644.0000\n7645.0000\n7646.0000\n7647.0000\n7648.0000\n7649.0000\n7650.0000\n7651.0000\n7652.0000\n7653.0000\n7654.0000\n7655.0000\n7656.0000\n7657.0000\n7658.0000\n7659.0000\n7660.0000\n7661.0000\n7662.0000\n7663.0000\n7664.0000\n7665.0000\n7666.0000\n7667.0000\n7668.0000\n7669.0000\n7670.0000\n7671.0000\n7672.0000\n7673.0000\n7674.0000\n7675.0000\n7676.0000\n7677.0000\n7678.0000\n7679.0000\n7680.0000\n7681.0000\n7682.0000\n7683.0000\n7684.0000\n7685.0000\n7686.0000\n7687.0000\n7688.0000\n7689.0000\n7690.0000\n7691.0000\n7692.0000\n7693.0000\n7694.0000\n7695.0000\n7696.0000\n7697.0000\n7698.0000\n7699.0000\n7700.0000\n7701.0000\n7702.0000\n7703.0000\n7704.0000\n7705.0000\n7706.0000\n7707.0000\n7708.0000\n7709.0000\n7710.0000\n7711.0000\n7712.0000\n7713.0000\n7714.0000\n7715.0000\n7716.0000\n7717.0000\n7718.0000\n7719.0000\n7720.0000\n7721.0000\n7722.0000\n7723.0000\n7724.0000\n7725.0000\n7726.0000\n7727.0000\n7728.0000\n7729.0000\n7730.0000\n7731.0000\n7732.0000\n7733.0000\n7734.0000\n7735.0000\n7736.0000\n7737.0000\n7738.0000\n7739.0000\n7740.0000\n7741.0000\n7742.0000\n7743.0000\n7744.0000\n7745.0000\n7746.0000\n7747.0000\n7748.0000\n7749.0000\n7750.0000\n7751.0000\n7752.0000\n7753.0000\n7754.0000\n7755.0000\n7756.0000\n7757.0000\n7758.0000\n7759.0000\n7760.0000\n7761.0000\n7762.0000\n7763.0000\n7764.0000\n7765.0000\n7766.0000\n7767.0000\n7768.0000\n7769.0000\n7770.0000\n7771.0000\n7772.0000\n7773.0000\n7774.0000\n7775.0000\n7776.0000\n7777.0000\n7778.0000\n7779.0000\n7780.0000\n7781.0000\n7782.0000\n7783.0000\n7784.0000\n7785.0000\n7786.0000\n7787.0000\n7788.0000\n7789.0000\n7790.0000\n7791.0000\n7792.0000\n7793.0000\n7794.0000\n7795.0000\n7796.0000\n7797.0000\n7798.0000\n7799.0000\n7800.0000\n7801.0000\n7802.0000\n7803.0000\n7804.0000\n7805.0000\n7806.0000\n7807.0000\n7808.0000\n7809.0000\n7810.0000\n7811.0000\n7812.0000\n7813.0000\n7814.0000\n7815.0000\n7816.0000\n7817.0000\n7818.0000\n7819.0000\n7820.0000\n7821.0000\n7822.0000\n7823.0000\n7824.0000\n7825.0000\n7826.0000\n7827.0000\n7828.0000\n7829.0000\n7830.0000\n7831.0000\n7832.0000\n7833.0000\n7834.0000\n7835.0000\n7836.0000\n7837.0000\n7838.0000\n7839.0000\n7840.0000\n7841.0000\n7842.0000\n7843.0000\n7844.0000\n7845.0000\n7846.0000\n7847.0000\n7848.0000\n7849.0000\n7850.0000\n7851.0000\n7852.0000\n7853.0000\n7854.0000\n7855.0000\n7856.0000\n7857.0000\n7858.0000\n7859.0000\n7860.0000\n7861.0000\n7862.0000\n7863.0000\n7864.0000\n7865.0000\n7866.0000\n7867.0000\n7868.0000\n7869.0000\n7870.0000\n7871.0000\n7872.0000\n7873.0000\n7874.0000\n7875.0000\n7876.0000\n7877.0000\n7878.0000\n7879.0000\n7880.0000\n7881.0000\n7882.0000\n7883.0000\n7884.0000\n7885.0000\n7886.0000\n7887.0000\n7888.0000\n7889.0000\n7890.0000\n7891.0000\n7892.0000\n7893.0000\n7894.0000\n7895.0000\n7896.0000\n7897.0000\n7898.0000\n7899.0000\n7900.0000\n7901.0000\n7902.0000\n7903.0000\n7904.0000\n7905.0000\n7906.0000\n7907.0000\n7908.0000\n7909.0000\n7910.0000\n7911.0000\n7912.0000\n7913.0000\n7914.0000\n7915.0000\n7916.0000\n7917.0000\n7918.0000\n7919.0000\n7920.0000\n7921.0000\n7922.0000\n7923.0000\n7924.0000\n7925.0000\n7926.0000\n7927.0000\n7928.0000\n7929.0000\n7930.0000\n7931.0000\n7932.0000\n7933.0000\n7934.0000\n7935.0000\n7936.0000\n7937.0000\n7938.0000\n7939.0000\n7940.0000\n7941.0000\n7942.0000\n7943.0000\n7944.0000\n7945.0000\n7946.0000\n7947.0000\n7948.0000\n7949.0000\n7950.0000\n7951.0000\n7952.0000\n7953.0000\n7954.0000\n7955.0000\n7956.0000\n7957.0000\n7958.0000\n7959.0000\n7960.0000\n7961.0000\n7962.0000\n7963.0000\n7964.0000\n7965.0000\n7966.0000\n7967.0000\n7968.0000\n7969.0000\n7970.0000\n7971.0000\n7972.0000\n7973.0000\n7974.0000\n7975.0000\n7976.0000\n7977.0000\n7978.0000\n7979.0000\n7980.0000\n7981.0000\n7982.0000\n7983.0000\n7984.0000\n7985.0000\n7986.0000\n7987.0000\n7988.0000\n7989.0000\n7990.0000\n7991.0000\n7992.0000\n7993.0000\n7994.0000\n7995.0000\n7996.0000\n7997.0000\n7998.0000\n7999.0000\n8000.0000\n8001.0000\n8002.0000\n8003.0000\n8004.0000\n8005.0000\n8006.0000\n8007.0000\n8008.0000\n8009.0000\n8010.0000\n8011.0000\n8012.0000\n8013.0000\n8014.0000\n8015.0000\n8016.0000\n8017.0000\n8018.0000\n8019.0000\n8020.0000\n8021.0000\n8022.0000\n8023.0000\n8024.0000\n8025.0000\n8026.0000\n8027.0000\n8028.0000\n8029.0000\n8030.0000\n8031.0000\n8032.0000\n8033.0000\n8034.0000\n8035.0000\n8036.0000\n8037.0000\n8038.0000\n8039.0000\n8040.0000\n8041.0000\n8042.0000\n8043.0000\n8044.0000\n8045.0000\n8046.0000\n8047.0000\n8048.0000\n8049.0000\n8050.0000\n8051.0000\n8052.0000\n8053.0000\n8054.0000\n8055.0000\n8056.0000\n8057.0000\n8058.0000\n8059.0000\n8060.0000\n8061.0000\n8062.0000\n8063.0000\n8064.0000\n8065.0000\n8066.0000\n8067.0000\n8068.0000\n8069.0000\n8070.0000\n8071.0000\n8072.0000\n8073.0000\n8074.0000\n8075.0000\n8076.0000\n8077.0000\n8078.0000\n8079.0000\n8080.0000\n8081.0000\n8082.0000\n8083.0000\n8084.0000\n8085.0000\n8086.0000\n8087.0000\n8088.0000\n8089.0000\n8090.0000\n8091.0000\n8092.0000\n8093.0000\n8094.0000\n8095.0000\n8096.0000\n8097.0000\n8098.0000\n8099.0000\n8100.0000\n8101.0000\n8102.0000\n8103.0000\n8104.0000\n8105.0000\n8106.0000\n8107.0000\n8108.0000\n8109.0000\n8110.0000\n8111.0000\n8112.0000\n8113.0000\n8114.0000\n8115.0000\n8116.0000\n8117.0000\n8118.0000\n8119.0000\n8120.0000\n8121.0000\n8122.0000\n8123.0000\n8124.0000\n8125.0000\n8126.0000\n8127.0000\n8128.0000\n8129.0000\n8130.0000\n8131.0000\n8132.0000\n8133.0000\n8134.0000\n8135.0000\n8136.0000\n8137.0000\n8138.0000\n8139.0000\n8140.0000\n8141.0000\n8142.0000\n8143.0000\n8144.0000\n8145.0000\n8146.0000\n8147.0000\n8148.0000\n8149.0000\n8150.0000\n8151.0000\n8152.0000\n8153.0000\n8154.0000\n8155.0000\n8156.0000\n8157.0000\n8158.0000\n8159.0000\n8160.0000\n8161.0000\n8162.0000\n8163.0000\n8164.0000\n8165.0000\n8166.0000\n8167.0000\n8168.0000\n8169.0000\n8170.0000\n8171.0000\n8172.0000\n8173.0000\n8174.0000\n8175.0000\n8176.0000\n8177.0000\n8178.0000\n8179.0000\n8180.0000\n8181.0000\n8182.0000\n8183.0000\n8184.0000\n8185.0000\n8186.0000\n8187.0000\n8188.0000\n8189.0000\n8190.0000\n8191.0000\n8192.0000\n8193.0000\n8194.0000\n8195.0000\n8196.0000\n8197.0000\n8198.0000\n8199.0000\n8200.0000\n8201.0000\n8202.0000\n8203.0000\n8204.0000\n8205.0000\n8206.0000\n8207.0000\n8208.0000\n8209.0000\n8210.0000\n8211.0000\n8212.0000\n8213.0000\n8214.0000\n8215.0000\n8216.0000\n8217.0000\n8218.0000\n8219.0000\n8220.0000\n8221.0000\n8222.0000\n8223.0000\n8224.0000\n8225.0000\n8226.0000\n8227.0000\n8228.0000\n8229.0000\n8230.0000\n8231.0000\n8232.0000\n8233.0000\n8234.0000\n8235.0000\n8236.0000\n8237.0000\n8238.0000\n8239.0000\n8240.0000\n8241.0000\n8242.0000\n8243.0000\n8244.0000\n8245.0000\n8246.0000\n8247.0000\n8248.0000\n8249.0000\n8250.0000\n8251.0000\n8252.0000\n8253.0000\n8254.0000\n8255.0000\n8256.0000\n8257.0000\n8258.0000\n8259.0000\n8260.0000\n8261.0000\n8262.0000\n8263.0000\n8264.0000\n8265.0000\n8266.0000\n8267.0000\n8268.0000\n8269.0000\n8270.0000\n8271.0000\n8272.0000\n8273.0000\n8274.0000\n8275.0000\n8276.0000\n8277.0000\n8278.0000\n8279.0000\n8280.0000\n8281.0000\n8282.0000\n8283.0000\n8284.0000\n8285.0000\n8286.0000\n8287.0000\n8288.0000\n8289.0000\n8290.0000\n8291.0000\n8292.0000\n8293.0000\n8294.0000\n8295.0000\n8296.0000\n8297.0000\n8298.0000\n8299.0000\n8300.0000\n8301.0000\n8302.0000\n8303.0000\n8304.0000\n8305.0000\n8306.0000\n8307.0000\n8308.0000\n8309.0000\n8310.0000\n8311.0000\n8312.0000\n8313.0000\n8314.0000\n8315.0000\n8316.0000\n8317.0000\n8318.0000\n8319.0000\n8320.0000\n8321.0000\n8322.0000\n8323.0000\n8324.0000\n8325.0000\n8326.0000\n8327.0000\n8328.0000\n8329.0000\n8330.0000\n8331.0000\n8332.0000\n8333.0000\n8334.0000\n8335.0000\n8336.0000\n8337.0000\n8338.0000\n8339.0000\n8340.0000\n8341.0000\n8342.0000\n8343.0000\n8344.0000\n8345.0000\n8346.0000\n8347.0000\n8348.0000\n8349.0000\n8350.0000\n8351.0000\n8352.0000\n8353.0000\n8354.0000\n8355.0000\n8356.0000\n8357.0000\n8358.0000\n8359.0000\n8360.0000\n8361.0000\n8362.0000\n8363.0000\n8364.0000\n8365.0000\n8366.0000\n8367.0000\n8368.0000\n8369.0000\n8370.0000\n8371.0000\n8372.0000\n8373.0000\n8374.0000\n8375.0000\n8376.0000\n8377.0000\n8378.0000\n8379.0000\n8380.0000\n8381.0000\n8382.0000\n8383.0000\n8384.0000\n8385.0000\n8386.0000\n8387.0000\n8388.0000\n8389.0000\n8390.0000\n8391.0000\n8392.0000\n8393.0000\n8394.0000\n8395.0000\n8396.0000\n8397.0000\n8398.0000\n8399.0000\n8400.0000\n8401.0000\n8402.0000\n8403.0000\n8404.0000\n8405.0000\n8406.0000\n8407.0000\n8408.0000\n8409.0000\n8410.0000\n8411.0000\n8412.0000\n8413.0000\n8414.0000\n8415.0000\n8416.0000\n8417.0000\n8418.0000\n8419.0000\n8420.0000\n8421.0000\n8422.0000\n8423.0000\n8424.0000\n8425.0000\n8426.0000\n8427.0000\n8428.0000\n8429.0000\n8430.0000\n8431.0000\n8432.0000\n8433.0000\n8434.0000\n8435.0000\n8436.0000\n8437.0000\n8438.0000\n8439.0000\n8440.0000\n8441.0000\n8442.0000\n8443.0000\n8444.0000\n8445.0000\n8446.0000\n8447.0000\n8448.0000\n8449.0000\n8450.0000\n8451.0000\n8452.0000\n8453.0000\n8454.0000\n8455.0000\n8456.0000\n8457.0000\n8458.0000\n8459.0000\n8460.0000\n8461.0000\n8462.0000\n8463.0000\n8464.0000\n8465.0000\n8466.0000\n8467.0000\n8468.0000\n8469.0000\n8470.0000\n8471.0000\n8472.0000\n8473.0000\n8474.0000\n8475.0000\n8476.0000\n8477.0000\n8478.0000\n8479.0000\n8480.0000\n8481.0000\n8482.0000\n8483.0000\n8484.0000\n8485.0000\n8486.0000\n8487.0000\n8488.0000\n8489.0000\n8490.0000\n8491.0000\n8492.0000\n8493.0000\n8494.0000\n8495.0000\n8496.0000\n8497.0000\n8498.0000\n8499.0000\n8500.0000\n8501.0000\n8502.0000\n8503.0000\n8504.0000\n8505.0000\n8506.0000\n8507.0000\n8508.0000\n8509.0000\n8510.0000\n8511.0000\n8512.0000\n8513.0000\n8514.0000\n8515.0000\n8516.0000\n8517.0000\n8518.0000\n8519.0000\n8520.0000\n8521.0000\n8522.0000\n8523.0000\n8524.0000\n8525.0000\n8526.0000\n8527.0000\n8528.0000\n8529.0000\n8530.0000\n8531.0000\n8532.0000\n8533.0000\n8534.0000\n8535.0000\n8536.0000\n8537.0000\n8538.0000\n8539.0000\n8540.0000\n8541.0000\n8542.0000\n8543.0000\n8544.0000\n8545.0000\n8546.0000\n8547.0000\n8548.0000\n8549.0000\n8550.0000\n8551.0000\n8552.0000\n8553.0000\n8554.0000\n8555.0000\n8556.0000\n8557.0000\n8558.0000\n8559.0000\n8560.0000\n8561.0000\n8562.0000\n8563.0000\n8564.0000\n8565.0000\n8566.0000\n8567.0000\n8568.0000\n8569.0000\n8570.0000\n8571.0000\n8572.0000\n8573.0000\n8574.0000\n8575.0000\n8576.0000\n8577.0000\n8578.0000\n8579.0000\n8580.0000\n8581.0000\n8582.0000\n8583.0000\n8584.0000\n8585.0000\n8586.0000\n8587.0000\n8588.0000\n8589.0000\n8590.0000\n8591.0000\n8592.0000\n8593.0000\n8594.0000\n8595.0000\n8596.0000\n8597.0000\n8598.0000\n8599.0000\n8600.0000\n8601.0000\n8602.0000\n8603.0000\n8604.0000\n8605.0000\n8606.0000\n8607.0000\n8608.0000\n8609.0000\n8610.0000\n8611.0000\n8612.0000\n8613.0000\n8614.0000\n8615.0000\n8616.0000\n8617.0000\n8618.0000\n8619.0000\n8620.0000\n8621.0000\n8622.0000\n8623.0000\n8624.0000\n8625.0000\n8626.0000\n8627.0000\n8628.0000\n8629.0000\n8630.0000\n8631.0000\n8632.0000\n8633.0000\n8634.0000\n8635.0000\n8636.0000\n8637.0000\n8638.0000\n8639.0000\n8640.0000\n8641.0000\n8642.0000\n8643.0000\n8644.0000\n8645.0000\n8646.0000\n8647.0000\n8648.0000\n8649.0000\n8650.0000\n8651.0000\n8652.0000\n8653.0000\n8654.0000\n8655.0000\n8656.0000\n8657.0000\n8658.0000\n8659.0000\n8660.0000\n8661.0000\n8662.0000\n8663.0000\n8664.0000\n8665.0000\n8666.0000\n8667.0000\n8668.0000\n8669.0000\n8670.0000\n8671.0000\n8672.0000\n8673.0000\n8674.0000\n8675.0000\n8676.0000\n8677.0000\n8678.0000\n8679.0000\n8680.0000\n8681.0000\n8682.0000\n8683.0000\n8684.0000\n8685.0000\n8686.0000\n8687.0000\n8688.0000\n8689.0000\n8690.0000\n8691.0000\n8692.0000\n8693.0000\n8694.0000\n8695.0000\n8696.0000\n8697.0000\n8698.0000\n8699.0000\n8700.0000\n8701.0000\n8702.0000\n8703.0000\n8704.0000\n8705.0000\n8706.0000\n8707.0000\n8708.0000\n8709.0000\n8710.0000\n8711.0000\n8712.0000\n8713.0000\n8714.0000\n8715.0000\n8716.0000\n8717.0000\n8718.0000\n8719.0000\n8720.0000\n8721.0000\n8722.0000\n8723.0000\n8724.0000\n8725.0000\n8726.0000\n8727.0000\n8728.0000\n8729.0000\n8730.0000\n8731.0000\n8732.0000\n8733.0000\n8734.0000\n8735.0000\n8736.0000\n8737.0000\n8738.0000\n8739.0000\n8740.0000\n8741.0000\n8742.0000\n8743.0000\n8744.0000\n8745.0000\n8746.0000\n8747.0000\n8748.0000\n8749.0000\n8750.0000\n8751.0000\n8752.0000\n8753.0000\n8754.0000\n8755.0000\n8756.0000\n8757.0000\n8758.0000\n8759.0000\n8760.0000\n8761.0000\n8762.0000\n8763.0000\n8764.0000\n8765.0000\n8766.0000\n8767.0000\n8768.0000\n8769.0000\n8770.0000\n8771.0000\n8772.0000\n8773.0000\n8774.0000\n8775.0000\n8776.0000\n8777.0000\n8778.0000\n8779.0000\n8780.0000\n8781.0000\n8782.0000\n8783.0000\n8784.0000\n8785.0000\n8786.0000\n8787.0000\n8788.0000\n8789.0000\n8790.0000\n8791.0000\n8792.0000\n8793.0000\n8794.0000\n8795.0000\n8796.0000\n8797.0000\n8798.0000\n8799.0000\n8800.0000\n8801.0000\n8802.0000\n8803.0000\n8804.0000\n8805.0000\n8806.0000\n8807.0000\n8808.0000\n8809.0000\n8810.0000\n8811.0000\n8812.0000\n8813.0000\n8814.0000\n8815.0000\n8816.0000\n8817.0000\n8818.0000\n8819.0000\n8820.0000\n8821.0000\n8822.0000\n8823.0000\n8824.0000\n8825.0000\n8826.0000\n8827.0000\n8828.0000\n8829.0000\n8830.0000\n8831.0000\n8832.0000\n8833.0000\n8834.0000\n8835.0000\n8836.0000\n8837.0000\n8838.0000\n8839.0000\n8840.0000\n8841.0000\n8842.0000\n8843.0000\n8844.0000\n8845.0000\n8846.0000\n8847.0000\n8848.0000\n8849.0000\n8850.0000\n8851.0000\n8852.0000\n8853.0000\n8854.0000\n8855.0000\n8856.0000\n8857.0000\n8858.0000\n8859.0000\n8860.0000\n8861.0000\n8862.0000\n8863.0000\n8864.0000\n8865.0000\n8866.0000\n8867.0000\n8868.0000\n8869.0000\n8870.0000\n8871.0000\n8872.0000\n8873.0000\n8874.0000\n8875.0000\n8876.0000\n8877.0000\n8878.0000\n8879.0000\n8880.0000\n8881.0000\n8882.0000\n8883.0000\n8884.0000\n8885.0000\n8886.0000\n8887.0000\n8888.0000\n8889.0000\n8890.0000\n8891.0000\n8892.0000\n8893.0000\n8894.0000\n8895.0000\n8896.0000\n8897.0000\n8898.0000\n8899.0000\n8900.0000\n8901.0000\n8902.0000\n8903.0000\n8904.0000\n8905.0000\n8906.0000\n8907.0000\n8908.0000\n8909.0000\n8910.0000\n8911.0000\n8912.0000\n8913.0000\n8914.0000\n8915.0000\n8916.0000\n8917.0000\n8918.0000\n8919.0000\n8920.0000\n8921.0000\n8922.0000\n8923.0000\n8924.0000\n8925.0000\n8926.0000\n8927.0000\n8928.0000\n8929.0000\n8930.0000\n8931.0000\n8932.0000\n8933.0000\n8934.0000\n8935.0000\n8936.0000\n8937.0000\n8938.0000\n8939.0000\n8940.0000\n8941.0000\n8942.0000\n8943.0000\n8944.0000\n8945.0000\n8946.0000\n8947.0000\n8948.0000\n8949.0000\n8950.0000\n8951.0000\n8952.0000\n8953.0000\n8954.0000\n8955.0000\n8956.0000\n8957.0000\n8958.0000\n8959.0000\n8960.0000\n8961.0000\n8962.0000\n8963.0000\n8964.0000\n8965.0000\n8966.0000\n8967.0000\n8968.0000\n8969.0000\n8970.0000\n8971.0000\n8972.0000\n8973.0000\n8974.0000\n8975.0000\n8976.0000\n8977.0000\n8978.0000\n8979.0000\n8980.0000\n8981.0000\n8982.0000\n8983.0000\n8984.0000\n8985.0000\n8986.0000\n8987.0000\n8988.0000\n8989.0000\n8990.0000\n8991.0000\n8992.0000\n8993.0000\n8994.0000\n8995.0000\n8996.0000\n8997.0000\n8998.0000\n8999.0000\n9000.0000\n") -> (array=w12:dbl[][])  [unwired: 2 in]
  n2 = Spreadsheet String To Array(format string="%f", spreadsheet string="22.11942\n26.25920\n28.39900\n29.98667\n30.59293\n30.50293\n30.15908\n29.81117\n29.54470\n29.36585\n29.25482\n29.18932\n29.15201\n29.13122\n29.11975\n29.11344\n29.10991\n29.10787\n29.10664\n29.10584\n29.10529\n29.10489\n29.10458\n29.10432\n29.10411\n29.10393\n29.10378\n29.10364\n29.10353\n29.10343\n29.10334\n29.10327\n29.10321\n29.10315\n29.10310\n29.10306\n29.10303\n29.10300\n29.10297\n29.10295\n29.10294\n29.10292\n29.10292\n29.10291\n29.10291\n29.10290\n29.10291\n29.10291\n29.10291\n29.10292\n29.10293\n29.10294\n29.10295\n29.10296\n29.10298\n29.10299\n29.10301\n29.10302\n29.10304\n29.10306\n29.10308\n29.10310\n29.10312\n29.10314\n29.10316\n29.10318\n29.10321\n29.10323\n29.10325\n29.10328\n29.10330\n29.10333\n29.10335\n29.10338\n29.10340\n29.10343\n29.10346\n29.10348\n29.10351\n29.10354\n29.10357\n29.10359\n29.10362\n29.10365\n29.10368\n29.10371\n29.10374\n29.10376\n29.10379\n29.10382\n29.10385\n29.10388\n29.10391\n29.10394\n29.10397\n29.10400\n29.10403\n29.10406\n29.10409\n29.10412\n29.10415\n29.10418\n29.10421\n29.10424\n29.10428\n29.10431\n29.10434\n29.10437\n29.10440\n29.10443\n29.10446\n29.10449\n29.10453\n29.10456\n29.10459\n29.10462\n29.10465\n29.10468\n29.10472\n29.10475\n29.10478\n29.10481\n29.10484\n29.10487\n29.10491\n29.10494\n29.10497\n29.10500\n29.10504\n29.10507\n29.10510\n29.10513\n29.10516\n29.10520\n29.10523\n29.10526\n29.10529\n29.10533\n29.10536\n29.10539\n29.10542\n29.10546\n29.10549\n29.10552\n29.10555\n29.10559\n29.10562\n29.10565\n29.10569\n29.10572\n29.10575\n29.10578\n29.10582\n29.10585\n29.10588\n29.10592\n29.10595\n29.10598\n29.10602\n29.10605\n29.10608\n29.10612\n29.10615\n29.10618\n29.10622\n29.10625\n29.10628\n29.10632\n29.10635\n29.10638\n29.10642\n29.10645\n29.10649\n29.10652\n29.10656\n29.10659\n29.10663\n29.10666\n29.10670\n29.10673\n29.10677\n29.10680\n29.10684\n29.10687\n29.10691\n29.10695\n29.10698\n29.10702\n29.10706\n29.10710\n29.10713\n29.10717\n29.10721\n29.10725\n29.10729\n29.10733\n29.10737\n29.10741\n29.10745\n29.10750\n29.10754\n29.10758\n29.10763\n29.10767\n29.10772\n29.10776\n29.10781\n29.10786\n29.10790\n29.10795\n29.10800\n29.10806\n29.10811\n29.10816\n29.10822\n29.10827\n29.10833\n29.10839\n29.10845\n29.10851\n29.10857\n29.10864\n29.10870\n29.10877\n29.10884\n29.10891\n29.10898\n29.10905\n29.10913\n29.10921\n29.10929\n29.10937\n29.10945\n29.10954\n29.10963\n29.10972\n29.10982\n29.10991\n29.11001\n29.11011\n29.11022\n29.11033\n29.11044\n29.11055\n29.11067\n29.11079\n29.11091\n29.11104\n29.11117\n29.11131\n29.11145\n29.11159\n29.11174\n29.11189\n29.11204\n29.11220\n29.11237\n29.11253\n29.11271\n29.11289\n29.11307\n29.11326\n29.11345\n29.11365\n29.11385\n29.11406\n29.11428\n29.11450\n29.11472\n29.11496\n29.11520\n29.11545\n29.11570\n29.11596\n29.11623\n29.11650\n29.11678\n29.11706\n29.11736\n29.11766\n29.11796\n29.11828\n29.11860\n29.11893\n29.11927\n29.11962\n29.11998\n29.12034\n29.12071\n29.12110\n29.12149\n29.12189\n29.12230\n29.12271\n29.12314\n29.12358\n29.12403\n29.12456\n29.12495\n29.12543\n29.12593\n29.12643\n29.12694\n29.12746\n29.12799\n29.12853\n29.12909\n29.12965\n29.13023\n29.13082\n29.13142\n29.13203\n29.13266\n29.13330\n29.13395\n29.13461\n29.13528\n29.13597\n29.13668\n29.13740\n29.13813\n29.13887\n29.13963\n29.14040\n29.14118\n29.14198\n29.14279\n29.14361\n29.14446\n29.14531\n29.14618\n29.14707\n29.14797\n29.14889\n29.14983\n29.15077\n29.15174\n29.15271\n29.15371\n29.15472\n29.15575\n29.15679\n29.15785\n29.15893\n29.16002\n29.16114\n29.16227\n29.16341\n29.16457\n29.16575\n29.16695\n29.16816\n29.16940\n29.17065\n29.17191\n29.17321\n29.17451\n29.17584\n29.17718\n29.17854\n29.17992\n29.18131\n29.18273\n29.18417\n29.18562\n29.18710\n29.18860\n29.19011\n29.19164\n29.19319\n29.19476\n29.19636\n29.19797\n29.19960\n29.20126\n29.20293\n29.20462\n29.20634\n29.20807\n29.20982\n29.21160\n29.21339\n29.21521\n29.21705\n29.21891\n29.22079\n29.22269\n29.22461\n29.22655\n29.22851\n29.23051\n29.23251\n29.23454\n29.23659\n29.23866\n29.24076\n29.24287\n29.24501\n29.24717\n29.24935\n29.25156\n29.25378\n29.25603\n29.25830\n29.26059\n29.26291\n29.26524\n29.26760\n29.26998\n29.27238\n29.27481\n29.27725\n29.27973\n29.28223\n29.28474\n29.28728\n29.28984\n29.29242\n29.29503\n29.29766\n29.30031\n29.30299\n29.30568\n29.30840\n29.31114\n29.31392\n29.31671\n29.31952\n29.32235\n29.32521\n29.32808\n29.33099\n29.33392\n29.33687\n29.33984\n29.34283\n29.34585\n29.34888\n29.35196\n29.35504\n29.35815\n29.36128\n29.36443\n29.36761\n29.37082\n29.37404\n29.37728\n29.38055\n29.38384\n29.38715\n29.39050\n29.39385\n29.39723\n29.40064\n29.40406\n29.40751\n29.41099\n29.41449\n29.41800\n29.42154\n29.42510\n29.42868\n29.43230\n29.43593\n29.43958\n29.44325\n29.44695\n29.45067\n29.45441\n29.45817\n29.46196\n29.46576\n29.46959\n29.47345\n29.47732\n29.48121\n29.48513\n29.48907\n29.49302\n29.49701\n29.50102\n29.50504\n29.50908\n29.51315\n29.51724\n29.52136\n29.52549\n29.52964\n29.53381\n29.53800\n29.54223\n29.54646\n29.55072\n29.55499\n29.55929\n29.56361\n29.56796\n29.57232\n29.57670\n29.58110\n29.58552\n29.58997\n29.59443\n29.59892\n29.60342\n29.60794\n29.61248\n29.61705\n29.62163\n29.62623\n29.63085\n29.63549\n29.64016\n29.64484\n29.64954\n29.65426\n29.65900\n29.66375\n29.66854\n29.67333\n29.67814\n29.68297\n29.68782\n29.69269\n29.69759\n29.70250\n29.70742\n29.71236\n29.71732\n29.72231\n29.72731\n29.73232\n29.73735\n29.74240\n29.74747\n29.75257\n29.75767\n29.76279\n29.76793\n29.77308\n29.77825\n29.78345\n29.78866\n29.79388\n29.79912\n29.80438\n29.80966\n29.81495\n29.82025\n29.82558\n29.83091\n29.83627\n29.84165\n29.84703\n29.85244\n29.85786\n29.86329\n29.86874\n29.87421\n29.87969\n29.88519\n29.89070\n29.89622\n29.90177\n29.90733\n29.91290\n29.91849\n29.92409\n29.92970\n29.93533\n29.94098\n29.94664\n29.95231\n29.95800\n29.96370\n29.96941\n29.97515\n29.98089\n29.98665\n29.99241\n29.99820\n30.00399\n30.00981\n30.01563\n30.02146\n30.02731\n30.03317\n30.03904\n30.04494\n30.05084\n30.05675\n30.06267\n30.06861\n30.07455\n30.08052\n30.08649\n30.09248\n30.09847\n30.10448\n30.11050\n30.11653\n30.12258\n30.12863\n30.13470\n30.14077\n30.14686\n30.15295\n30.15907\n30.16519\n30.17132\n30.17746\n30.18361\n30.18977\n30.19594\n30.20213\n30.20832\n30.21452\n30.22074\n30.22696\n30.23319\n30.23943\n30.24569\n30.25195\n30.25822\n30.26449\n30.27078\n30.27708\n30.28338\n30.28971\n30.29603\n30.30236\n30.30870\n30.31505\n30.32141\n30.32778\n30.33416\n30.34054\n30.34693\n30.35333\n30.35974\n30.36615\n30.37258\n30.37902\n30.38545\n30.39190\n30.39835\n30.40481\n30.41128\n30.41775\n30.42424\n30.43073\n30.43723\n30.44373\n30.45024\n30.45675\n30.46327\n30.46980\n30.47635\n30.48289\n30.48944\n30.49599\n30.50255\n30.50912\n30.51569\n30.52226\n30.52886\n30.53545\n30.54204\n30.54864\n30.55525\n30.56186\n30.56847\n30.57509\n30.58173\n30.58836\n30.59500\n30.60164\n30.60828\n30.61494\n30.62159\n30.62825\n30.63491\n30.64159\n30.64827\n30.65494\n30.66163\n30.66831\n30.67500\n30.68169\n30.68839\n30.69509\n30.70181\n30.70852\n30.71523\n30.72195\n30.72867\n30.73539\n30.74211\n30.74884\n30.75558\n30.76232\n30.76906\n30.77580\n30.78255\n30.78929\n30.79604\n30.80280\n30.80955\n30.81631\n30.82307\n30.82984\n30.83661\n30.84338\n30.85015\n30.85692\n30.86369\n30.87047\n30.87725\n30.88403\n30.89081\n30.89759\n30.90438\n30.91117\n30.91796\n30.92475\n30.93154\n30.93833\n30.94513\n30.95192\n30.95872\n30.96552\n30.97232\n30.97912\n30.98592\n30.99273\n30.99953\n31.00633\n31.01313\n31.01994\n31.02674\n31.03355\n31.04036\n31.04716\n31.05398\n31.06079\n31.06759\n31.07440\n31.08121\n31.08802\n31.09482\n31.10163\n31.10844\n31.11525\n31.12205\n31.12886\n31.13567\n31.14249\n31.14929\n31.15610\n31.16290\n31.16971\n31.17651\n31.18331\n31.19012\n31.19692\n31.20372\n31.21052\n31.21732\n31.22412\n31.23092\n31.23772\n31.24452\n31.25131\n31.25810\n31.26490\n31.27169\n31.27848\n31.28526\n31.29205\n31.29883\n31.30562\n31.31240\n31.31918\n31.32596\n31.33273\n31.33952\n31.34629\n31.35306\n31.35983\n31.36660\n31.37337\n31.38013\n31.38689\n31.39365\n31.40041\n31.40716\n31.41392\n31.42067\n31.42742\n31.43416\n31.44091\n31.44765\n31.45439\n31.46113\n31.46787\n31.47460\n31.48133\n31.48805\n31.49477\n31.50150\n31.50821\n31.51493\n31.52164\n31.52835\n31.53506\n31.54176\n31.54846\n31.55516\n31.56185\n31.56854\n31.57523\n31.58192\n31.58860\n31.59529\n31.60196\n31.60863\n31.61530\n31.62197\n31.62863\n31.63529\n31.64194\n31.64859\n31.65524\n31.66189\n31.66853\n31.67516\n31.68180\n31.68843\n31.69505\n31.70168\n31.70829\n31.71491\n31.72152\n31.72813\n31.73473\n31.74133\n31.74793\n31.75452\n31.76110\n31.76770\n31.77428\n31.78085\n31.78742\n31.79399\n31.80055\n31.80711\n31.81367\n31.82022\n31.82676\n31.83330\n31.83984\n31.84637\n31.85290\n31.85943\n31.86595\n31.87246\n31.87897\n31.88548\n31.89198\n31.89848\n31.90497\n31.91146\n31.91794\n31.92442\n31.93089\n31.93736\n31.94383\n31.95029\n31.95674\n31.96319\n31.96964\n31.97608\n31.98252\n31.98895\n31.99537\n32.00179\n32.00822\n32.01463\n32.02104\n32.02744\n32.03384\n32.04023\n32.04662\n32.05300\n32.05937\n32.06574\n32.07211\n32.07847\n32.08483\n32.09118\n32.09752\n32.10386\n32.11020\n32.11653\n32.12285\n32.12917\n32.13549\n32.14179\n32.14810\n32.15440\n32.16069\n32.16698\n32.17326\n32.17953\n32.18581\n32.19207\n32.19833\n32.20459\n32.21083\n32.21708\n32.22332\n32.22955\n32.23578\n32.24200\n32.24821\n32.25442\n32.26063\n32.26683\n32.27302\n32.27921\n32.28539\n32.29157\n32.29774\n32.30390\n32.31006\n32.31622\n32.32237\n32.32851\n32.33465\n32.34078\n32.34690\n32.35302\n32.35913\n32.36524\n32.37134\n32.37744\n32.38353\n32.38961\n32.39569\n32.40177\n32.40783\n32.41389\n32.41995\n32.42600\n32.43204\n32.43808\n32.44411\n32.45013\n32.45615\n32.46217\n32.46817\n32.47418\n32.48017\n32.48616\n32.49214\n32.49812\n32.50409\n32.51006\n32.51602\n32.52197\n32.52792\n32.53386\n32.53979\n32.54572\n32.55165\n32.55756\n32.56347\n32.56938\n32.57528\n32.58117\n32.58705\n32.59293\n32.59881\n32.60468\n32.61054\n32.61639\n32.62224\n32.62809\n32.63392\n32.63975\n32.64558\n32.65140\n32.65721\n32.66301\n32.66881\n32.67461\n32.68039\n32.68618\n32.69195\n32.69772\n32.70348\n32.70924\n32.71499\n32.72073\n32.72647\n32.73220\n32.73792\n32.74364\n32.74935\n32.75506\n32.76076\n32.76645\n32.77214\n32.77782\n32.78350\n32.78916\n32.79483\n32.80048\n32.80613\n32.81177\n32.81741\n32.82304\n32.82867\n32.83428\n32.83989\n32.84550\n32.85110\n32.85669\n32.86228\n32.86786\n32.87343\n32.87900\n32.88456\n32.89010\n32.89565\n32.90119\n32.90673\n32.91226\n32.91778\n32.92329\n32.92880\n32.93431\n32.93981\n32.94530\n32.95078\n32.95626\n32.96173\n32.96720\n32.97265\n32.97811\n32.98355\n32.98899\n32.99443\n32.99985\n33.00528\n33.01069\n33.01610\n33.02150\n33.02690\n33.03228\n33.03767\n33.04304\n33.04841\n33.05378\n33.05913\n33.06449\n33.06983\n33.07517\n33.08050\n33.08583\n33.09114\n33.09646\n33.10176\n33.10706\n33.11236\n33.11764\n33.12293\n33.12820\n33.13347\n33.13873\n33.14399\n33.14924\n33.15448\n33.15970\n33.16493\n33.17016\n33.17538\n33.18059\n33.18579\n33.19099\n33.19618\n33.20137\n33.20655\n33.21172\n33.21689\n33.22205\n33.22720\n33.23235\n33.23749\n33.24263\n33.24776\n33.25288\n33.25800\n33.26311\n33.26821\n33.27331\n33.27840\n33.28348\n33.28856\n33.29364\n33.29870\n33.30376\n33.30882\n33.31386\n33.31890\n33.32394\n33.32897\n33.33399\n33.33900\n33.34401\n33.34902\n33.35401\n33.35900\n33.36398\n33.36896\n33.37393\n33.37890\n33.38386\n33.38881\n33.39376\n33.39870\n33.40363\n33.40856\n33.41349\n33.41840\n33.42331\n33.42822\n33.43311\n33.43801\n33.44289\n33.44777\n33.45264\n33.45751\n33.46237\n33.46723\n33.47207\n33.47692\n33.48175\n33.48658\n33.49141\n33.49622\n33.50104\n33.50584\n33.51064\n33.51542\n33.52021\n33.52499\n33.52977\n33.53453\n33.53930\n33.54405\n33.54880\n33.55355\n33.55829\n33.56302\n33.56775\n33.57247\n33.57718\n33.58189\n33.58659\n33.59129\n33.59598\n33.60066\n33.60534\n33.61001\n33.61467\n33.61933\n33.62399\n33.62864\n33.63328\n33.63791\n33.64254\n33.64717\n33.65178\n33.65640\n33.66099\n33.66559\n33.67019\n33.67477\n33.67936\n33.68393\n33.68850\n33.69307\n33.69762\n33.70218\n33.70672\n33.71126\n33.71580\n33.72033\n33.72485\n33.72937\n33.73388\n33.73838\n33.74288\n33.74738\n33.75186\n33.75635\n33.76082\n33.76529\n33.76976\n33.77422\n33.77867\n33.78311\n33.78756\n33.79198\n33.79641\n33.80083\n33.80525\n33.80966\n33.81407\n33.81847\n33.82286\n33.82725\n33.83164\n33.83601\n33.84039\n33.84475\n33.84911\n33.85347\n33.85782\n33.86216\n33.86650\n33.87083\n33.87515\n33.87947\n33.88379\n33.88810\n33.89240\n33.89670\n33.90099\n33.90528\n33.90956\n33.91382\n33.91809\n33.92235\n33.92661\n33.93087\n33.93511\n33.93935\n33.94359\n33.94782\n33.95204\n33.95626\n33.96048\n33.96468\n33.96889\n33.97308\n33.97727\n33.98146\n33.98564\n33.98981\n33.99398\n33.99815\n34.00230\n34.00646\n34.01060\n34.01475\n34.01888\n34.02301\n34.02713\n34.03125\n34.03536\n34.03947\n34.04357\n34.04767\n34.05176\n34.05585\n34.05993\n34.06401\n34.06808\n34.07214\n34.07620\n34.08026\n34.08431\n34.08835\n34.09239\n34.09642\n34.10045\n34.10447\n34.10849\n34.11250\n34.11651\n34.12051\n34.12450\n34.12850\n34.13247\n34.13645\n34.14042\n34.14439\n34.14836\n34.15232\n34.15627\n34.16022\n34.16416\n34.16810\n34.17203\n34.17596\n34.17988\n34.18380\n34.18771\n34.19162\n34.19552\n34.19941\n34.20330\n34.20719\n34.21107\n34.21494\n34.21881\n34.22268\n34.22654\n34.23039\n34.23423\n34.23808\n34.24192\n34.24575\n34.24958\n34.25340\n34.25722\n34.26104\n34.26485\n34.26865\n34.27245\n34.27624\n34.28003\n34.28381\n34.28759\n34.29137\n34.29513\n34.29890\n34.30266\n34.30641\n34.31016\n34.31390\n34.31764\n34.32137\n34.32510\n34.32883\n34.33253\n34.33625\n34.33996\n34.34366\n34.34736\n34.35105\n34.35474\n34.35843\n34.36210\n34.36578\n34.36945\n34.37311\n34.37677\n34.38043\n34.38408\n34.38772\n34.39136\n34.39500\n34.39863\n34.40225\n34.40587\n34.40949\n34.41310\n34.41671\n34.42031\n34.42390\n34.42749\n34.43107\n34.43466\n34.43823\n34.44181\n34.44538\n34.44894\n34.45250\n34.45605\n34.45960\n34.46314\n34.46668\n34.47022\n34.47375\n34.47728\n34.48080\n34.48431\n34.48782\n34.49133\n34.49483\n34.49833\n34.50182\n34.50531\n34.50880\n34.51227\n34.51574\n34.51921\n34.52267\n34.52614\n34.52959\n34.53304\n34.53649\n34.53993\n34.54337\n34.54680\n34.55023\n34.55366\n34.55707\n34.56049\n34.56390\n34.56731\n34.57071\n34.57410\n34.57750\n34.58088\n34.58427\n34.58765\n34.59102\n34.59439\n34.59776\n34.60111\n34.60446\n34.60782\n34.61116\n34.61451\n34.61785\n34.62118\n34.62451\n34.62784\n34.63116\n34.63447\n34.63779\n34.64109\n34.64440\n34.64770\n34.65099\n34.65428\n34.65757\n34.66085\n34.66413\n34.66740\n34.67067\n34.67393\n34.67719\n34.68045\n34.68370\n34.68694\n34.69018\n34.69342\n34.69666\n34.69989\n34.70311\n34.70633\n34.70955\n34.71276\n34.71597\n34.71918\n34.72238\n34.72557\n34.72877\n34.73195\n34.73514\n34.73832\n34.74149\n34.74466\n34.74783\n34.75099\n34.75415\n34.75731\n34.76046\n34.76360\n34.76675\n34.76987\n34.77301\n34.77614\n34.77926\n34.78238\n34.78550\n34.78861\n34.79172\n34.79483\n34.79793\n34.80103\n34.80412\n34.80721\n34.81029\n34.81337\n34.81645\n34.81952\n34.82259\n34.82566\n34.82872\n34.83177\n34.83483\n34.83787\n34.84092\n34.84396\n34.84700\n34.85002\n34.85305\n34.85607\n34.85909\n34.86211\n34.86512\n34.86813\n34.87114\n34.87414\n34.87713\n34.88013\n34.88312\n34.88610\n34.88908\n34.89206\n34.89503\n34.89800\n34.90097\n34.90393\n34.90689\n34.90985\n34.91280\n34.91574\n34.91869\n34.92162\n34.92456\n34.92748\n34.93041\n34.93333\n34.93625\n34.93917\n34.94208\n34.94499\n34.94789\n34.95079\n34.95369\n34.95659\n34.95948\n34.96236\n34.96524\n34.96812\n34.97100\n34.97387\n34.97674\n34.97960\n34.98246\n34.98532\n34.98817\n34.99102\n34.99386\n34.99670\n34.99954\n35.00236\n35.00520\n35.00802\n35.01085\n35.01366\n35.01648\n35.01929\n35.02210\n35.02491\n35.02771\n35.03051\n35.03330\n35.03609\n35.03888\n35.04166\n35.04444\n35.04722\n35.04999\n35.05276\n35.05552\n35.05828\n35.06104\n35.06380\n35.06655\n35.06930\n35.07204\n35.07478\n35.07751\n35.08024\n35.08297\n35.08570\n35.08842\n35.09114\n35.09386\n35.09657\n35.09928\n35.10198\n35.10469\n35.10739\n35.11008\n35.11277\n35.11546\n35.11815\n35.12083\n35.12351\n35.12618\n35.12885\n35.13152\n35.13418\n35.13684\n35.13950\n35.14216\n35.14481\n35.14745\n35.15009\n35.15273\n35.15537\n35.15800\n35.16063\n35.16326\n35.16588\n35.16850\n35.17112\n35.17373\n35.17634\n35.17895\n35.18156\n35.18416\n35.18675\n35.18935\n35.19194\n35.19453\n35.19711\n35.19969\n35.20227\n35.20484\n35.20741\n35.20998\n35.21255\n35.21511\n35.21767\n35.22022\n35.22276\n35.22531\n35.22786\n35.23040\n35.23294\n35.23547\n35.23800\n35.24053\n35.24306\n35.24558\n35.24810\n35.25062\n35.25313\n35.25564\n35.25815\n35.26065\n35.26315\n35.26565\n35.26814\n35.27064\n35.27312\n35.27561\n35.27809\n35.28057\n35.28304\n35.28552\n35.28799\n35.29045\n35.29291\n35.29537\n35.29782\n35.30028\n35.30273\n35.30518\n35.30762\n35.31006\n35.31250\n35.31494\n35.31737\n35.31980\n35.32222\n35.32465\n35.32707\n35.32949\n35.33190\n35.33431\n35.33672\n35.33912\n35.34153\n35.34393\n35.34632\n35.34872\n35.35111\n35.35349\n35.35588\n35.35826\n35.36063\n35.36300\n35.36538\n35.36775\n35.37011\n35.37248\n35.37484\n35.37719\n35.37955\n35.38190\n35.38425\n35.38660\n35.38894\n35.39128\n35.39362\n35.39595\n35.39828\n35.40061\n35.40294\n35.40526\n35.40758\n35.40990\n35.41221\n35.41453\n35.41683\n35.41914\n35.42144\n35.42374\n35.42604\n35.42834\n35.43062\n35.43291\n35.43519\n35.43748\n35.43976\n35.44203\n35.44431\n35.44658\n35.44885\n35.45112\n35.45338\n35.45564\n35.45790\n35.46016\n35.46241\n35.46466\n35.46691\n35.46915\n35.47139\n35.47363\n35.47587\n35.47810\n35.48033\n35.48256\n35.48478\n35.48701\n35.48923\n35.49144\n35.49366\n35.49587\n35.49807\n35.50028\n35.50248\n35.50468\n35.50688\n35.50907\n35.51127\n35.51346\n35.51565\n35.51783\n35.52001\n35.52219\n35.52437\n35.52654\n35.52872\n35.53088\n35.53305\n35.53522\n35.53738\n35.53954\n35.54169\n35.54384\n35.54600\n35.54814\n35.55029\n35.55243\n35.55457\n35.55671\n35.55885\n35.56098\n35.56310\n35.56523\n35.56735\n35.56947\n35.57159\n35.57371\n35.57583\n35.57794\n35.58005\n35.58216\n35.58426\n35.58636\n35.58846\n35.59056\n35.59265\n35.59475\n35.59684\n35.59892\n35.60101\n35.60309\n35.60517\n35.60725\n35.60932\n35.61139\n35.61346\n35.61553\n35.61759\n35.61966\n35.62172\n35.62377\n35.62583\n35.62788\n35.62992\n35.63197\n35.63401\n35.63606\n35.63810\n35.64013\n35.64217\n35.64420\n35.64623\n35.64826\n35.65029\n35.65231\n35.65433\n35.65635\n35.65837\n35.66038\n35.66239\n35.66440\n35.66641\n35.66841\n35.67041\n35.67241\n35.67441\n35.67640\n35.67840\n35.68039\n35.68237\n35.68436\n35.68634\n35.68832\n35.69030\n35.69228\n35.69424\n35.69621\n35.69818\n35.70015\n35.70211\n35.70408\n35.70604\n35.70799\n35.70995\n35.71190\n35.71385\n35.71580\n35.71775\n35.71969\n35.72163\n35.72357\n35.72551\n35.72744\n35.72938\n35.73131\n35.73323\n35.73516\n35.73708\n35.73900\n35.74092\n35.74284\n35.74475\n35.74667\n35.74858\n35.75048\n35.75239\n35.75429\n35.75619\n35.75808\n35.75998\n35.76188\n35.76377\n35.76566\n35.76755\n35.76943\n35.77132\n35.77320\n35.77508\n35.77695\n35.77883\n35.78070\n35.78257\n35.78444\n35.78631\n35.78817\n35.79003\n35.79189\n35.79375\n35.79560\n35.79746\n35.79931\n35.80116\n35.80301\n35.80485\n35.80669\n35.80853\n35.81037\n35.81221\n35.81404\n35.81588\n35.81771\n35.81953\n35.82135\n35.82317\n35.82499\n35.82681\n35.82863\n35.83045\n35.83226\n35.83407\n35.83588\n35.83769\n35.83949\n35.84130\n35.84310\n35.84490\n35.84669\n35.84849\n35.85028\n35.85207\n35.85386\n35.85565\n35.85743\n35.85921\n35.86099\n35.86277\n35.86455\n35.86632\n35.86810\n35.86987\n35.87164\n35.87340\n35.87517\n35.87693\n35.87869\n35.88045\n35.88220\n35.88395\n35.88570\n35.88745\n35.88920\n35.89095\n35.89269\n35.89443\n35.89618\n35.89791\n35.89965\n35.90139\n35.90312\n35.90485\n35.90658\n35.90831\n35.91003\n35.91175\n35.91348\n35.91519\n35.91691\n35.91863\n35.92034\n35.92205\n35.92376\n35.92547\n35.92718\n35.92888\n35.93058\n35.93228\n35.93398\n35.93568\n35.93737\n35.93906\n35.94075\n35.94244\n35.94413\n35.94581\n35.94749\n35.94917\n35.95085\n35.95253\n35.95420\n35.95588\n35.95755\n35.95922\n35.96089\n35.96255\n35.96422\n35.96588\n35.96754\n35.96920\n35.97086\n35.97251\n35.97417\n35.97582\n35.97747\n35.97912\n35.98076\n35.98241\n35.98405\n35.98569\n35.98733\n35.98897\n35.99060\n35.99224\n35.99387\n35.99550\n35.99713\n35.99875\n36.00038\n36.00200\n36.00362\n36.00524\n36.00685\n36.00846\n36.01008\n36.01169\n36.01330\n36.01491\n36.01652\n36.01812\n36.01973\n36.02133\n36.02293\n36.02452\n36.02612\n36.02772\n36.02931\n36.03090\n36.03249\n36.03408\n36.03566\n36.03725\n36.03883\n36.04041\n36.04199\n36.04357\n36.04514\n36.04672\n36.04829\n36.04986\n36.05143\n36.05300\n36.05456\n36.05613\n36.05769\n36.05925\n36.06081\n36.06236\n36.06392\n36.06547\n36.06703\n36.06857\n36.07011\n36.07166\n36.07321\n36.07475\n36.07629\n36.07783\n36.07937\n36.08091\n36.08244\n36.08398\n36.08551\n36.08704\n36.08857\n36.09010\n36.09162\n36.09315\n36.09467\n36.09619\n36.09771\n36.09923\n36.10074\n36.10226\n36.10377\n36.10528\n36.10679\n36.10830\n36.10980\n36.11131\n36.11281\n36.11431\n36.11581\n36.11731\n36.11881\n36.12030\n36.12179\n36.12329\n36.12478\n36.12626\n36.12775\n36.12923\n36.13071\n36.13219\n36.13367\n36.13515\n36.13663\n36.13811\n36.13958\n36.14105\n36.14253\n36.14400\n36.14546\n36.14693\n36.14840\n36.14986\n36.15132\n36.15278\n36.15424\n36.15570\n36.15715\n36.15861\n36.16006\n36.16151\n36.16296\n36.16441\n36.16586\n36.16730\n36.16875\n36.17019\n36.17163\n36.17307\n36.17451\n36.17594\n36.17738\n36.17881\n36.18024\n36.18167\n36.18310\n36.18453\n36.18596\n36.18738\n36.18880\n36.19021\n36.19163\n36.19305\n36.19447\n36.19589\n36.19730\n36.19871\n36.20012\n36.20153\n36.20294\n36.20435\n36.20575\n36.20716\n36.20856\n36.20996\n36.21136\n36.21276\n36.21415\n36.21555\n36.21694\n36.21834\n36.21973\n36.22112\n36.22250\n36.22389\n36.22527\n36.22666\n36.22804\n36.22942\n36.23080\n36.23218\n36.23356\n36.23493\n36.23630\n36.23768\n36.23905\n36.24042\n36.24179\n36.24315\n36.24452\n36.24588\n36.24724\n36.24861\n36.24996\n36.25131\n36.25267\n36.25403\n36.25538\n36.25673\n36.25809\n36.25944\n36.26078\n36.26213\n36.26348\n36.26482\n36.26617\n36.26751\n36.26885\n36.27019\n36.27152\n36.27286\n36.27420\n36.27553\n36.27686\n36.27819\n36.27952\n36.28085\n36.28218\n36.28350\n36.28483\n36.28615\n36.28747\n36.28879\n36.29011\n36.29143\n36.29275\n36.29406\n36.29538\n36.29669\n36.29800\n36.29931\n36.30062\n36.30193\n36.30323\n36.30454\n36.30584\n36.30714\n36.30844\n36.30973\n36.31103\n36.31233\n36.31362\n36.31492\n36.31621\n36.31750\n36.31879\n36.32008\n36.32137\n36.32265\n36.32394\n36.32522\n36.32651\n36.32779\n36.32907\n36.33035\n36.33162\n36.33290\n36.33418\n36.33545\n36.33672\n36.33799\n36.33926\n36.34053\n36.34180\n36.34307\n36.34433\n36.34559\n36.34686\n36.34812\n36.34938\n36.35064\n36.35190\n36.35315\n36.35441\n36.35566\n36.35691\n36.35816\n36.35941\n36.36066\n36.36191\n36.36316\n36.36440\n36.36565\n36.36689\n36.36813\n36.36936\n36.37060\n36.37184\n36.37308\n36.37431\n36.37555\n36.37678\n36.37801\n36.37924\n36.38047\n36.38170\n36.38293\n36.38415\n36.38538\n36.38660\n36.38782\n36.38904\n36.39026\n36.39148\n36.39270\n36.39392\n36.39513\n36.39635\n36.39756\n36.39877\n36.39998\n36.40119\n36.40240\n36.40361\n36.40481\n36.40602\n36.40722\n36.40842\n36.40963\n36.41083\n36.41202\n36.41322\n36.41442\n36.41561\n36.41681\n36.41800\n36.41919\n36.42039\n36.42158\n36.42276\n36.42395\n36.42514\n36.42632\n36.42750\n36.42868\n36.42986\n36.43104\n36.43222\n36.43340\n36.43458\n36.43575\n36.43693\n36.43810\n36.43928\n36.44045\n36.44162\n36.44279\n36.44396\n36.44512\n36.44629\n36.44746\n36.44862\n36.44978\n36.45094\n36.45211\n36.45327\n36.45442\n36.45558\n36.45674\n36.45789\n36.45905\n36.46020\n36.46135\n36.46250\n36.46365\n36.46480\n36.46595\n36.46710\n36.46824\n36.46939\n36.47053\n36.47167\n36.47281\n36.47395\n36.47509\n36.47623\n36.47737\n36.47850\n36.47964\n36.48077\n36.48190\n36.48304\n36.48417\n36.48530\n36.48642\n36.48754\n36.48867\n36.48979\n36.49092\n36.49204\n36.49316\n36.49428\n36.49540\n36.49652\n36.49764\n36.49876\n36.49987\n36.50099\n36.50210\n36.50322\n36.50433\n36.50544\n36.50655\n36.50766\n36.50876\n36.50987\n36.51098\n36.51208\n36.51319\n36.51429\n36.51539\n36.51649\n36.51759\n36.51869\n36.51979\n36.52088\n36.52198\n36.52307\n36.52417\n36.52526\n36.52635\n36.52744\n36.52853\n36.52962\n36.53071\n36.53179\n36.53288\n36.53396\n36.53505\n36.53613\n36.53721\n36.53829\n36.53937\n36.54045\n36.54153\n36.54260\n36.54368\n36.54475\n36.54582\n36.54689\n36.54796\n36.54903\n36.55010\n36.55117\n36.55224\n36.55331\n36.55437\n36.55544\n36.55650\n36.55756\n36.55863\n36.55969\n36.56075\n36.56181\n36.56287\n36.56392\n36.56498\n36.56603\n36.56709\n36.56814\n36.56919\n36.57025\n36.57130\n36.57235\n36.57340\n36.57444\n36.57549\n36.57654\n36.57758\n36.57863\n36.57967\n36.58071\n36.58175\n36.58279\n36.58383\n36.58487\n36.58591\n36.58695\n36.58798\n36.58902\n36.59005\n36.59108\n36.59211\n36.59315\n36.59418\n36.59521\n36.59623\n36.59726\n36.59829\n36.59931\n36.60034\n36.60136\n36.60239\n36.60341\n36.60443\n36.60544\n36.60646\n36.60748\n36.60849\n36.60951\n36.61053\n36.61154\n36.61256\n36.61357\n36.61458\n36.61559\n36.61660\n36.61761\n36.61862\n36.61963\n36.62064\n36.62164\n36.62265\n36.62365\n36.62465\n36.62566\n36.62666\n36.62766\n36.62866\n36.62966\n36.63066\n36.63165\n36.63265\n36.63364\n36.63464\n36.63563\n36.63663\n36.63762\n36.63861\n36.63960\n36.64059\n36.64158\n36.64256\n36.64355\n36.64454\n36.64552\n36.64651\n36.64749\n36.64847\n36.64945\n36.65044\n36.65142\n36.65240\n36.65337\n36.65435\n36.65533\n36.65630\n36.65728\n36.65825\n36.65923\n36.66020\n36.66117\n36.66214\n36.66311\n36.66407\n36.66504\n36.66601\n36.66697\n36.66794\n36.66890\n36.66987\n36.67083\n36.67179\n36.67276\n36.67372\n36.67468\n36.67564\n36.67659\n36.67755\n36.67851\n36.67946\n36.68042\n36.68137\n36.68233\n36.68328\n36.68423\n36.68518\n36.68613\n36.68708\n36.68803\n36.68898\n36.68993\n36.69087\n36.69182\n36.69276\n36.69371\n36.69465\n36.69559\n36.69653\n36.69747\n36.69841\n36.69935\n36.70029\n36.70123\n36.70217\n36.70310\n36.70404\n36.70497\n36.70591\n36.70684\n36.70777\n36.70870\n36.70963\n36.71056\n36.71149\n36.71242\n36.71335\n36.71427\n36.71520\n36.71612\n36.71705\n36.71797\n36.71889\n36.71982\n36.72074\n36.72166\n36.72258\n36.72349\n36.72440\n36.72532\n36.72624\n36.72715\n36.72807\n36.72898\n36.72990\n36.73081\n36.73172\n36.73263\n36.73354\n36.73445\n36.73536\n36.73627\n36.73718\n36.73809\n36.73899\n36.73990\n36.74080\n36.74171\n36.74261\n36.74351\n36.74441\n36.74531\n36.74621\n36.74711\n36.74801\n36.74891\n36.74981\n36.75070\n36.75160\n36.75249\n36.75339\n36.75428\n36.75517\n36.75607\n36.75696\n36.75785\n36.75874\n36.75963\n36.76052\n36.76140\n36.76229\n36.76318\n36.76406\n36.76495\n36.76583\n36.76671\n36.76760\n36.76848\n36.76936\n36.77024\n36.77112\n36.77200\n36.77288\n36.77376\n36.77463\n36.77551\n36.77639\n36.77726\n36.77813\n36.77901\n36.77988\n36.78075\n36.78162\n36.78248\n36.78335\n36.78422\n36.78509\n36.78596\n36.78683\n36.78769\n36.78856\n36.78942\n36.79029\n36.79115\n36.79202\n36.79288\n36.79374\n36.79460\n36.79546\n36.79632\n36.79718\n36.79804\n36.79889\n36.79975\n36.80061\n36.80146\n36.80232\n36.80317\n36.80403\n36.80488\n36.80573\n36.80658\n36.80743\n36.80828\n36.80913\n36.80998\n36.81083\n36.81168\n36.81252\n36.81337\n36.81421\n36.81506\n36.81590\n36.81675\n36.81759\n36.81843\n36.81927\n36.82011\n36.82095\n36.82179\n36.82263\n36.82347\n36.82431\n36.82514\n36.82598\n36.82682\n36.82765\n36.82848\n36.82932\n36.83015\n36.83098\n36.83181\n36.83265\n36.83348\n36.83431\n36.83513\n36.83596\n36.83679\n36.83762\n36.83844\n36.83927\n36.84009\n36.84092\n36.84174\n36.84256\n36.84338\n36.84420\n36.84502\n36.84584\n36.84666\n36.84748\n36.84830\n36.84912\n36.84994\n36.85075\n36.85157\n36.85239\n36.85320\n36.85401\n36.85483\n36.85564\n36.85645\n36.85727\n36.85808\n36.85889\n36.85970\n36.86051\n36.86132\n36.86212\n36.86293\n36.86374\n36.86454\n36.86535\n36.86616\n36.86696\n36.86776\n36.86857\n36.86937\n36.87017\n36.87097\n36.87177\n36.87257\n36.87337\n36.87417\n36.87497\n36.87577\n36.87657\n36.87736\n36.87816\n36.87895\n36.87975\n36.88054\n36.88134\n36.88213\n36.88292\n36.88371\n36.88450\n36.88529\n36.88608\n36.88687\n36.88766\n36.88845\n36.88924\n36.89003\n36.89081\n36.89160\n36.89238\n36.89317\n36.89395\n36.89473\n36.89552\n36.89630\n36.89708\n36.89786\n36.89864\n36.89942\n36.90020\n36.90098\n36.90175\n36.90253\n36.90330\n36.90408\n36.90486\n36.90563\n36.90641\n36.90718\n36.90795\n36.90873\n36.90950\n36.91027\n36.91104\n36.91181\n36.91258\n36.91335\n36.91412\n36.91489\n36.91566\n36.91643\n36.91719\n36.91796\n36.91872\n36.91949\n36.92025\n36.92102\n36.92178\n36.92254\n36.92331\n36.92407\n36.92483\n36.92559\n36.92635\n36.92711\n36.92787\n36.92863\n36.92938\n36.93014\n36.93090\n36.93165\n36.93241\n36.93317\n36.93392\n36.93467\n36.93543\n36.93618\n36.93693\n36.93768\n36.93844\n36.93919\n36.93994\n36.94069\n36.94143\n36.94218\n36.94293\n36.94368\n36.94443\n36.94517\n36.94592\n36.94666\n36.94741\n36.94815\n36.94890\n36.94964\n36.95038\n36.95112\n36.95186\n36.95261\n36.95335\n36.95409\n36.95483\n36.95556\n36.95630\n36.95704\n36.95778\n36.95851\n36.95925\n36.95999\n36.96072\n36.96146\n36.96219\n36.96291\n36.96365\n36.96438\n36.96511\n36.96584\n36.96657\n36.96730\n36.96803\n36.96876\n36.96949\n36.97022\n36.97095\n36.97168\n36.97240\n36.97313\n36.97385\n36.97458\n36.97530\n36.97603\n36.97675\n36.97748\n36.97820\n36.97892\n36.97964\n36.98036\n36.98108\n36.98180\n36.98252\n36.98324\n36.98396\n36.98468\n36.98540\n36.98612\n36.98683\n36.98755\n36.98826\n36.98898\n36.98969\n36.99041\n36.99112\n36.99183\n36.99255\n36.99326\n36.99397\n36.99468\n36.99539\n36.99610\n36.99681\n36.99752\n36.99823\n36.99894\n36.99965\n37.00035\n37.00106\n37.00177\n37.00247\n37.00318\n37.00388\n37.00459\n37.00529\n37.00599\n37.00670\n37.00740\n37.00810\n37.00880\n37.00950\n37.01020\n37.01090\n37.01160\n37.01230\n37.01300\n37.01370\n37.01440\n37.01509\n37.01579\n37.01649\n37.01718\n37.01788\n37.01857\n37.01927\n37.01996\n37.02065\n37.02135\n37.02204\n37.02273\n37.02342\n37.02410\n37.02479\n37.02548\n37.02617\n37.02686\n37.02755\n37.02824\n37.02893\n37.02961\n37.03030\n37.03099\n37.03167\n37.03236\n37.03304\n37.03373\n37.03441\n37.03509\n37.03578\n37.03646\n37.03714\n37.03782\n37.03850\n37.03918\n37.03986\n37.04054\n37.04122\n37.04190\n37.04258\n37.04326\n37.04394\n37.04461\n37.04529\n37.04597\n37.04664\n37.04732\n37.04799\n37.04867\n37.04934\n37.05001\n37.05069\n37.05136\n37.05203\n37.05270\n37.05337\n37.05404\n37.05471\n37.05538\n37.05605\n37.05672\n37.05739\n37.05806\n37.05873\n37.05939\n37.06006\n37.06073\n37.06139\n37.06206\n37.06272\n37.06339\n37.06405\n37.06472\n37.06538\n37.06604\n37.06670\n37.06737\n37.06803\n37.06869\n37.06935\n37.07001\n37.07067\n37.07133\n37.07199\n37.07265\n37.07331\n37.07396\n37.07462\n37.07528\n37.07593\n37.07659\n37.07724\n37.07790\n37.07855\n37.07921\n37.07986\n37.08052\n37.08117\n37.08182\n37.08247\n37.08312\n37.08378\n37.08443\n37.08508\n37.08572\n37.08637\n37.08702\n37.08766\n37.08831\n37.08896\n37.08961\n37.09026\n37.09090\n37.09155\n37.09219\n37.09284\n37.09348\n37.09413\n37.09477\n37.09542\n37.09606\n37.09670\n37.09735\n37.09799\n37.09863\n37.09927\n37.09991\n37.10055\n37.10119\n37.10183\n37.10247\n37.10311\n37.10375\n37.10439\n37.10502\n37.10566\n37.10630\n37.10693\n37.10757\n37.10821\n37.10884\n37.10948\n37.11011\n37.11074\n37.11138\n37.11201\n37.11264\n37.11328\n37.11391\n37.11454\n37.11517\n37.11580\n37.11643\n37.11706\n37.11769\n37.11832\n37.11895\n37.11958\n37.12021\n37.12083\n37.12146\n37.12209\n37.12271\n37.12334\n37.12397\n37.12459\n37.12522\n37.12584\n37.12646\n37.12709\n37.12771\n37.12833\n37.12896\n37.12958\n37.13020\n37.13082\n37.13144\n37.13206\n37.13268\n37.13330\n37.13392\n37.13454\n37.13516\n37.13578\n37.13640\n37.13702\n37.13763\n37.13825\n37.13887\n37.13948\n37.14010\n37.14071\n37.14133\n37.14194\n37.14256\n37.14317\n37.14378\n37.14440\n37.14501\n37.14562\n37.14623\n37.14684\n37.14746\n37.14807\n37.14867\n37.14928\n37.14989\n37.15050\n37.15111\n37.15171\n37.15232\n37.15293\n37.15354\n37.15414\n37.15475\n37.15536\n37.15596\n37.15657\n37.15717\n37.15778\n37.15838\n37.15899\n37.15959\n37.16019\n37.16080\n37.16140\n37.16200\n37.16260\n37.16321\n37.16381\n37.16441\n37.16501\n37.16561\n37.16621\n37.16681\n37.16741\n37.16801\n37.16860\n37.16920\n37.16980\n37.17040\n37.17099\n37.17159\n37.17219\n37.17278\n37.17338\n37.17397\n37.17457\n37.17516\n37.17576\n37.17635\n37.17694\n37.17754\n37.17813\n37.17872\n37.17931\n37.17990\n37.18050\n37.18109\n37.18168\n37.18227\n37.18286\n37.18345\n37.18404\n37.18462\n37.18521\n37.18580\n37.18639\n37.18698\n37.18756\n37.18815\n37.18874\n37.18932\n37.18991\n37.19049\n37.19108\n37.19166\n37.19225\n37.19283\n37.19342\n37.19400\n37.19458\n37.19516\n37.19575\n37.19633\n37.19691\n37.19749\n37.19807\n37.19865\n37.19923\n37.19981\n37.20039\n37.20097\n37.20155\n37.20213\n37.20271\n37.20329\n37.20386\n37.20444\n37.20502\n37.20559\n37.20617\n37.20675\n37.20732\n37.20790\n37.20847\n37.20905\n37.20962\n37.21019\n37.21077\n37.21134\n37.21191\n37.21249\n37.21305\n37.21362\n37.21419\n37.21476\n37.21533\n37.21590\n37.21647\n37.21704\n37.21761\n37.21818\n37.21875\n37.21932\n37.21989\n37.22046\n37.22103\n37.22159\n37.22216\n37.22273\n37.22329\n37.22386\n37.22443\n37.22499\n37.22556\n37.22612\n37.22669\n37.22725\n37.22781\n37.22838\n37.22894\n37.22950\n37.23007\n37.23063\n37.23119\n37.23175\n37.23231\n37.23287\n37.23343\n37.23399\n37.23455\n37.23511\n37.23567\n37.23623\n37.23679\n37.23735\n37.23791\n37.23847\n37.23902\n37.23958\n37.24014\n37.24069\n37.24125\n37.24181\n37.24236\n37.24292\n37.24347\n37.24403\n37.24458\n37.24514\n37.24569\n37.24624\n37.24680\n37.24735\n37.24790\n37.24846\n37.24901\n37.24956\n37.25011\n37.25066\n37.25121\n37.25176\n37.25231\n37.25286\n37.25341\n37.25396\n37.25451\n37.25506\n37.25561\n37.25616\n37.25670\n37.25725\n37.25780\n37.25835\n37.25889\n37.25944\n37.25998\n37.26053\n37.26108\n37.26162\n37.26217\n37.26271\n37.26325\n37.26380\n37.26434\n37.26489\n37.26543\n37.26597\n37.26651\n37.26706\n37.26760\n37.26814\n37.26868\n37.26922\n37.26976\n37.27030\n37.27084\n37.27138\n37.27192\n37.27246\n37.27300\n37.27354\n37.27408\n37.27462\n37.27515\n37.27569\n37.27623\n37.27676\n37.27730\n37.27784\n37.27837\n37.27891\n37.27944\n37.27997\n37.28051\n37.28104\n37.28157\n37.28211\n37.28264\n37.28318\n37.28371\n37.28424\n37.28477\n37.28531\n37.28584\n37.28637\n37.28690\n37.28743\n37.28796\n37.28850\n37.28903\n37.28956\n37.29009\n37.29062\n37.29114\n37.29167\n37.29220\n37.29273\n37.29326\n37.29379\n37.29431\n37.29484\n37.29537\n37.29590\n37.29642\n37.29695\n37.29747\n37.29800\n37.29853\n37.29905\n37.29958\n37.30010\n37.30062\n37.30115\n37.30167\n37.30220\n37.30272\n37.30324\n37.30377\n37.30429\n37.30481\n37.30533\n37.30585\n37.30637\n37.30690\n37.30742\n37.30794\n37.30846\n37.30898\n37.30950\n37.31002\n37.31054\n37.31105\n37.31157\n37.31209\n37.31261\n37.31313\n37.31365\n37.31416\n37.31468\n37.31520\n37.31571\n37.31623\n37.31675\n37.31726\n37.31778\n37.31829\n37.31881\n37.31932\n37.31984\n37.32035\n37.32086\n37.32138\n37.32189\n37.32240\n37.32292\n37.32343\n37.32394\n37.32445\n37.32497\n37.32548\n37.32599\n37.32650\n37.32701\n37.32752\n37.32803\n37.32854\n37.32905\n37.32956\n37.33007\n37.33058\n37.33109\n37.33160\n37.33211\n37.33261\n37.33312\n37.33363\n37.33414\n37.33464\n37.33515\n37.33566\n37.33616\n37.33667\n37.33717\n37.33768\n37.33819\n37.33869\n37.33919\n37.33970\n37.34020\n37.34071\n37.34121\n37.34171\n37.34222\n37.34272\n37.34322\n37.34373\n37.34423\n37.34473\n37.34523\n37.34573\n37.34623\n37.34674\n37.34723\n37.34773\n37.34823\n37.34873\n37.34923\n37.34973\n37.35023\n37.35072\n37.35122\n37.35172\n37.35222\n37.35272\n37.35322\n37.35371\n37.35421\n37.35471\n37.35521\n37.35570\n37.35620\n37.35669\n37.35719\n37.35769\n37.35818\n37.35868\n37.35917\n37.35967\n37.36016\n37.36065\n37.36115\n37.36164\n37.36214\n37.36263\n37.36312\n37.36362\n37.36411\n37.36460\n37.36509\n37.36558\n37.36608\n37.36657\n37.36706\n37.36755\n37.36804\n37.36853\n37.36902\n37.36951\n37.37000\n37.37049\n37.37098\n37.37147\n37.37196\n37.37244\n37.37293\n37.37342\n37.37391\n37.37440\n37.37488\n37.37537\n37.37586\n37.37634\n37.37683\n37.37732\n37.37780\n37.37829\n37.37877\n37.37926\n37.37975\n37.38023\n37.38071\n37.38120\n37.38168\n37.38217\n37.38265\n37.38313\n37.38362\n37.38410\n37.38458\n37.38507\n37.38555\n37.38603\n37.38651\n37.38699\n37.38748\n37.38796\n37.38844\n37.38892\n37.38940\n37.38988\n37.39036\n37.39084\n37.39132\n37.39180\n37.39228\n37.39276\n37.39324\n37.39371\n37.39419\n37.39467\n37.39515\n37.39563\n37.39610\n37.39658\n37.39706\n37.39754\n37.39801\n37.39849\n37.39896\n37.39944\n37.39992\n37.40039\n37.40087\n37.40134\n37.40182\n37.40229\n37.40277\n37.40324\n37.40371\n37.40419\n37.40466\n37.40514\n37.40561\n37.40608\n37.40655\n37.40703\n37.40750\n37.40797\n37.40844\n37.40891\n37.40939\n37.40986\n37.41033\n37.41080\n37.41127\n37.41174\n37.41221\n37.41268\n37.41315\n37.41362\n37.41409\n37.41456\n37.41503\n37.41549\n37.41596\n37.41643\n37.41690\n37.41737\n37.41783\n37.41830\n37.41876\n37.41923\n37.41969\n37.42016\n37.42063\n37.42109\n37.42156\n37.42202\n37.42249\n37.42295\n37.42342\n37.42388\n37.42435\n37.42481\n37.42528\n37.42574\n37.42621\n37.42667\n37.42713\n37.42760\n37.42806\n37.42852\n37.42899\n37.42945\n37.42991\n37.43037\n37.43083\n37.43130\n37.43176\n37.43222\n37.43268\n37.43314\n37.43360\n37.43406\n37.43452\n37.43498\n37.43544\n37.43590\n37.43636\n37.43682\n37.43728\n37.43774\n37.43820\n37.43865\n37.43911\n37.43957\n37.44003\n37.44049\n37.44094\n37.44140\n37.44186\n37.44231\n37.44277\n37.44323\n37.44368\n37.44414\n37.44460\n37.44505\n37.44551\n37.44596\n37.44642\n37.44687\n37.44733\n37.44778\n37.44824\n37.44869\n37.44914\n37.44960\n37.45005\n37.45050\n37.45096\n37.45141\n37.45186\n37.45232\n37.45277\n37.45322\n37.45367\n37.45412\n37.45458\n37.45503\n37.45548\n37.45593\n37.45638\n37.45683\n37.45728\n37.45773\n37.45818\n37.45863\n37.45908\n37.45953\n37.45998\n37.46043\n37.46088\n37.46133\n37.46178\n37.46222\n37.46267\n37.46312\n37.46357\n37.46402\n37.46446\n37.46491\n37.46536\n37.46581\n37.46625\n37.46670\n37.46715\n37.46759\n37.46804\n37.46848\n37.46893\n37.46937\n37.46982\n37.47026\n37.47071\n37.47115\n37.47160\n37.47204\n37.47249\n37.47293\n37.47337\n37.47382\n37.47426\n37.47470\n37.47515\n37.47559\n37.47603\n37.47648\n37.47692\n37.47736\n37.47780\n37.47824\n37.47869\n37.47913\n37.47957\n37.48001\n37.48045\n37.48089\n37.48133\n37.48177\n37.48221\n37.48265\n37.48309\n37.48353\n37.48397\n37.48441\n37.48485\n37.48529\n37.48573\n37.48617\n37.48660\n37.48704\n37.48748\n37.48792\n37.48836\n37.48879\n37.48923\n37.48967\n37.49011\n37.49054\n37.49098\n37.49142\n37.49185\n37.49229\n37.49272\n37.49316\n37.49360\n37.49403\n37.49446\n37.49489\n37.49533\n37.49576\n37.49620\n37.49663\n37.49706\n37.49750\n37.49793\n37.49837\n37.49880\n37.49923\n37.49967\n37.50010\n37.50053\n37.50096\n37.50140\n37.50183\n37.50226\n37.50269\n37.50313\n37.50356\n37.50399\n37.50442\n37.50485\n37.50528\n37.50571\n37.50614\n37.50657\n37.50700\n37.50743\n37.50786\n37.50829\n37.50872\n37.50915\n37.50958\n37.51001\n37.51044\n37.51087\n37.51130\n37.51173\n37.51216\n37.51258\n37.51301\n37.51344\n37.51387\n37.51429\n37.51472\n37.51515\n37.51558\n37.51600\n37.51643\n37.51686\n37.51728\n37.51771\n37.51813\n37.51856\n37.51899\n37.51941\n37.51984\n37.52026\n37.52069\n37.52111\n37.52154\n37.52196\n37.52239\n37.52281\n37.52323\n37.52366\n37.52408\n37.52451\n37.52493\n37.52535\n37.52578\n37.52620\n37.52662\n37.52704\n37.52747\n37.52789\n37.52831\n37.52873\n37.52916\n37.52958\n37.53000\n37.53042\n37.53084\n37.53126\n37.53168\n37.53210\n37.53253\n37.53295\n37.53337\n37.53379\n37.53421\n37.53463\n37.53505\n37.53547\n37.53588\n37.53630\n37.53672\n37.53714\n37.53756\n37.53798\n37.53840\n37.53882\n37.53923\n37.53965\n37.54007\n37.54049\n37.54091\n37.54132\n37.54174\n37.54216\n37.54257\n37.54299\n37.54341\n37.54382\n37.54424\n37.54466\n37.54507\n37.54549\n37.54590\n37.54632\n37.54674\n37.54715\n37.54757\n37.54798\n37.54840\n37.54881\n37.54922\n37.54964\n37.55005\n37.55047\n37.55088\n37.55130\n37.55171\n37.55212\n37.55254\n37.55295\n37.55336\n37.55378\n37.55419\n37.55460\n37.55501\n37.55543\n37.55584\n37.55625\n37.55666\n37.55707\n37.55748\n37.55790\n37.55831\n37.55872\n37.55913\n37.55954\n37.55995\n37.56036\n37.56077\n37.56118\n37.56159\n37.56200\n37.56241\n37.56282\n37.56323\n37.56364\n37.56405\n37.56446\n37.56487\n37.56528\n37.56569\n37.56609\n37.56650\n37.56691\n37.56732\n37.56773\n37.56814\n37.56854\n37.56895\n37.56936\n37.56977\n37.57017\n37.57058\n37.57099\n37.57139\n37.57180\n37.57221\n37.57261\n37.57302\n37.57342\n37.57383\n37.57424\n37.57464\n37.57505\n37.57545\n37.57586\n37.57626\n37.57667\n37.57707\n37.57748\n37.57788\n37.57829\n37.57868\n37.57908\n37.57949\n37.57989\n37.58030\n37.58070\n37.58110\n37.58151\n37.58191\n37.58231\n37.58271\n37.58312\n37.58352\n37.58392\n37.58433\n37.58473\n37.58513\n37.58553\n37.58593\n37.58633\n37.58674\n37.58714\n37.58754\n37.58794\n37.58834\n37.58874\n37.58914\n37.58954\n37.58994\n37.59034\n37.59074\n37.59114\n37.59154\n37.59194\n37.59234\n37.59274\n37.59314\n37.59354\n37.59394\n37.59434\n37.59474\n37.59514\n37.59554\n37.59593\n37.59633\n37.59673\n37.59713\n37.59753\n37.59792\n37.59832\n37.59872\n37.59912\n37.59951\n37.59991\n37.60031\n37.60071\n37.60110\n37.60150\n37.60190\n37.60229\n37.60269\n37.60308\n37.60348\n37.60388\n37.60427\n37.60467\n37.60506\n37.60546\n37.60585\n37.60625\n37.60664\n37.60704\n37.60743\n37.60783\n37.60822\n37.60862\n37.60901\n37.60941\n37.60980\n37.61019\n37.61059\n37.61098\n37.61137\n37.61177\n37.61216\n37.61255\n37.61295\n37.61334\n37.61373\n37.61413\n37.61452\n37.61491\n37.61530\n37.61570\n37.61609\n37.61648\n37.61687\n37.61726\n37.61765\n37.61805\n37.61844\n37.61883\n37.61922\n37.61961\n37.62000\n37.62039\n37.62078\n37.62117\n37.62156\n37.62195\n37.62234\n37.62273\n37.62312\n37.62351\n37.62390\n37.62429\n37.62468\n37.62507\n37.62546\n37.62585\n37.62624\n37.62663\n37.62701\n37.62740\n37.62779\n37.62818\n37.62857\n37.62896\n37.62934\n37.62973\n37.63012\n37.63051\n37.63089\n37.63128\n37.63167\n37.63206\n37.63244\n37.63283\n37.63322\n37.63360\n37.63399\n37.63438\n37.63476\n37.63515\n37.63554\n37.63592\n37.63631\n37.63669\n37.63708\n37.63746\n37.63785\n37.63823\n37.63862\n37.63900\n37.63939\n37.63977\n37.64016\n37.64054\n37.64093\n37.64131\n37.64170\n37.64208\n37.64246\n37.64285\n37.64323\n37.64362\n37.64400\n37.64438\n37.64477\n37.64515\n37.64553\n37.64592\n37.64630\n37.64668\n37.64706\n37.64745\n37.64783\n37.64821\n37.64859\n37.64898\n37.64936\n37.64974\n37.65012\n37.65050\n37.65089\n37.65127\n37.65165\n37.65203\n37.65241\n37.65279\n37.65317\n37.65355\n37.65393\n37.65431\n37.65469\n37.65508\n37.65546\n37.65584\n37.65622\n37.65660\n37.65698\n37.65736\n37.65773\n37.65811\n37.65849\n37.65887\n37.65925\n37.65963\n37.66001\n37.66039\n37.66077\n37.66115\n37.66153\n37.66190\n37.66228\n37.66266\n37.66304\n37.66342\n37.66379\n37.66417\n37.66455\n37.66493\n37.66530\n37.66568\n37.66606\n37.66644\n37.66681\n37.66719\n37.66757\n37.66794\n37.66832\n37.66870\n37.66907\n37.66945\n37.66983\n37.67020\n37.67058\n37.67095\n37.67133\n37.67171\n37.67208\n37.67246\n37.67283\n37.67321\n37.67358\n37.67396\n37.67433\n37.67471\n37.67508\n37.67546\n37.67583\n37.67621\n37.67658\n37.67696\n37.67733\n37.67770\n37.67808\n37.67845\n37.67883\n37.67920\n37.67957\n37.67995\n37.68032\n37.68069\n37.68107\n37.68144\n37.68181\n37.68218\n37.68255\n37.68292\n37.68329\n37.68367\n37.68404\n37.68441\n37.68478\n37.68516\n37.68553\n37.68590\n37.68627\n37.68664\n37.68702\n37.68739\n37.68776\n37.68813\n37.68850\n37.68887\n37.68924\n37.68961\n37.68999\n37.69036\n37.69073\n37.69110\n37.69147\n37.69184\n37.69221\n37.69258\n37.69295\n37.69332\n37.69369\n37.69406\n37.69443\n37.69480\n37.69517\n37.69554\n37.69591\n37.69628\n37.69665\n37.69702\n37.69738\n37.69775\n37.69812\n37.69849\n37.69886\n37.69923\n37.69960\n37.69996\n37.70033\n37.70070\n37.70107\n37.70144\n37.70181\n37.70217\n37.70254\n37.70291\n37.70328\n37.70364\n37.70401\n37.70438\n37.70475\n37.70511\n37.70548\n37.70585\n37.70621\n37.70658\n37.70695\n37.70731\n37.70768\n37.70805\n37.70841\n37.70878\n37.70914\n37.70951\n37.70988\n37.71024\n37.71061\n37.71097\n37.71134\n37.71170\n37.71207\n37.71244\n37.71280\n37.71317\n37.71353\n37.71390\n37.71426\n37.71463\n37.71499\n37.71535\n37.71572\n37.71608\n37.71645\n37.71681\n37.71718\n37.71754\n37.71790\n37.71827\n37.71863\n37.71900\n37.71936\n37.71972\n37.72009\n37.72045\n37.72081\n37.72118\n37.72154\n37.72190\n37.72227\n37.72263\n37.72299\n37.72335\n37.72372\n37.72408\n37.72444\n37.72480\n37.72517\n37.72553\n37.72589\n37.72625\n37.72662\n37.72698\n37.72734\n37.72770\n37.72806\n37.72842\n37.72879\n37.72915\n37.72951\n37.72987\n37.73023\n37.73059\n37.73095\n37.73131\n37.73167\n37.73204\n37.73240\n37.73276\n37.73312\n37.73348\n37.73384\n37.73420\n37.73456\n37.73492\n37.73528\n37.73564\n37.73600\n37.73636\n37.73672\n37.73708\n37.73744\n37.73780\n37.73816\n37.73852\n37.73887\n37.73923\n37.73959\n37.73995\n37.74031\n37.74067\n37.74103\n37.74139\n37.74175\n37.74210\n37.74246\n37.74282\n37.74318\n37.74354\n37.74390\n37.74425\n37.74461\n37.74497\n37.74533\n37.74569\n37.74604\n37.74640\n37.74676\n37.74712\n37.74747\n37.74783\n37.74819\n37.74855\n37.74890\n37.74926\n37.74962\n37.74997\n37.75033\n37.75069\n37.75104\n37.75140\n37.75176\n37.75211\n37.75247\n37.75283\n37.75318\n37.75354\n37.75389\n37.75425\n37.75461\n37.75496\n37.75532\n37.75567\n37.75603\n37.75638\n37.75674\n37.75709\n37.75745\n37.75781\n37.75816\n37.75852\n37.75887\n37.75923\n37.75958\n37.75994\n37.76029\n37.76064\n37.76100\n37.76135\n37.76171\n37.76206\n37.76242\n37.76277\n37.76313\n37.76348\n37.76383\n37.76419\n37.76454\n37.76490\n37.76525\n37.76560\n37.76596\n37.76631\n37.76666\n37.76702\n37.76737\n37.76772\n37.76808\n37.76843\n37.76878\n37.76914\n37.76949\n37.76984\n37.77019\n37.77055\n37.77090\n37.77125\n37.77161\n37.77196\n37.77231\n37.77266\n37.77301\n37.77337\n37.77372\n37.77407\n37.77442\n37.77478\n37.77513\n37.77548\n37.77583\n37.77618\n37.77653\n37.77689\n37.77724\n37.77759\n37.77794\n37.77829\n37.77864\n37.77899\n37.77934\n37.77970\n37.78005\n37.78040\n37.78075\n37.78110\n37.78145\n37.78180\n37.78215\n37.78250\n37.78285\n37.78320\n37.78355\n37.78390\n37.78425\n37.78460\n37.78495\n37.78530\n37.78565\n37.78600\n37.78635\n37.78670\n37.78705\n37.78740\n37.78775\n37.78810\n37.78845\n37.78880\n37.78915\n37.78950\n37.78985\n37.79020\n37.79055\n37.79089\n37.79124\n37.79159\n37.79194\n37.79229\n37.79264\n37.79299\n37.79334\n37.79368\n37.79403\n37.79438\n37.79473\n37.79508\n37.79543\n37.79577\n37.79612\n37.79647\n37.79682\n37.79717\n37.79751\n37.79786\n37.79821\n37.79856\n37.79890\n37.79925\n37.79960\n37.79995\n37.80029\n37.80064\n37.80099\n37.80134\n37.80168\n37.80203\n37.80238\n37.80273\n37.80307\n37.80342\n37.80377\n37.80411\n37.80446\n37.80481\n37.80515\n37.80550\n37.80585\n37.80619\n37.80654\n37.80688\n37.80723\n37.80758\n37.80792\n37.80827\n37.80862\n37.80896\n37.80931\n37.80965\n37.81000\n37.81035\n37.81069\n37.81104\n37.81138\n37.81173\n37.81207\n37.81242\n37.81276\n37.81311\n37.81345\n37.81380\n37.81415\n37.81449\n37.81484\n37.81518\n37.81553\n37.81587\n37.81622\n37.81656\n37.81690\n37.81725\n37.81759\n37.81794\n37.81828\n37.81863\n37.81897\n37.81932\n37.81966\n37.82001\n37.82035\n37.82069\n37.82104\n37.82138\n37.82173\n37.82207\n37.82241\n37.82276\n37.82310\n37.82345\n37.82379\n37.82413\n37.82448\n37.82482\n37.82516\n37.82551\n37.82585\n37.82619\n37.82654\n37.82688\n37.82722\n37.82757\n37.82791\n37.82825\n37.82860\n37.82894\n37.82928\n37.82963\n37.82997\n37.83031\n37.83065\n37.83100\n37.83134\n37.83168\n37.83203\n37.83237\n37.83271\n37.83305\n37.83340\n37.83374\n37.83408\n37.83442\n37.83476\n37.83511\n37.83545\n37.83579\n37.83613\n37.83647\n37.83682\n37.83716\n37.83750\n37.83784\n37.83818\n37.83853\n37.83887\n37.83921\n37.83955\n37.83989\n37.84023\n37.84058\n37.84092\n37.84126\n37.84160\n37.84194\n37.84228\n37.84262\n37.84296\n37.84331\n37.84365\n37.84399\n37.84433\n37.84467\n37.84501\n37.84535\n37.84569\n37.84603\n37.84637\n37.84671\n37.84705\n37.84740\n37.84774\n37.84808\n37.84842\n37.84876\n37.84910\n37.84944\n37.84978\n37.85012\n37.85046\n37.85080\n37.85114\n37.85148\n37.85182\n37.85216\n37.85250\n37.85284\n37.85318\n37.85352\n37.85386\n37.85420\n37.85454\n37.85488\n37.85522\n37.85556\n37.85590\n37.85624\n37.85658\n37.85692\n37.85726\n37.85759\n37.85793\n37.85827\n37.85861\n37.85895\n37.85929\n37.85963\n37.85997\n37.86031\n37.86065\n37.86099\n37.86133\n37.86166\n37.86200\n37.86234\n37.86268\n37.86302\n37.86336\n37.86370\n37.86404\n37.86437\n37.86471\n37.86505\n37.86539\n37.86573\n37.86607\n37.86641\n37.86674\n37.86708\n37.86742\n37.86776\n37.86810\n37.86844\n37.86877\n37.86911\n37.86945\n37.86979\n37.87013\n37.87046\n37.87080\n37.87114\n37.87148\n37.87182\n37.87215\n37.87249\n37.87283\n37.87317\n37.87351\n37.87384\n37.87418\n37.87452\n37.87486\n37.87519\n37.87553\n37.87587\n37.87621\n37.87654\n37.87688\n37.87722\n37.87756\n37.87789\n37.87823\n37.87857\n37.87891\n37.87924\n37.87958\n37.87992\n37.88025\n37.88059\n37.88093\n37.88126\n37.88160\n37.88194\n37.88228\n37.88261\n37.88295\n37.88329\n37.88362\n37.88396\n37.88430\n37.88463\n37.88497\n37.88531\n37.88564\n37.88598\n37.88632\n37.88665\n37.88699\n37.88733\n37.88766\n37.88800\n37.88834\n37.88867\n37.88901\n37.88934\n37.88968\n37.89002\n37.89035\n37.89069\n37.89103\n37.89136\n37.89170\n37.89203\n37.89237\n37.89271\n37.89304\n37.89338\n37.89371\n37.89405\n37.89439\n37.89472\n37.89506\n37.89539\n37.89573\n37.89607\n37.89640\n37.89674\n37.89707\n37.89741\n37.89774\n37.89808\n37.89842\n37.89875\n37.89909\n37.89942\n37.89976\n37.90009\n37.90043\n37.90076\n37.90110\n37.90144\n37.90177\n37.90211\n37.90244\n37.90278\n37.90311\n37.90345\n37.90378\n37.90412\n37.90445\n37.90479\n37.90512\n37.90546\n37.90579\n37.90613\n37.90646\n37.90680\n37.90713\n37.90747\n37.90780\n37.90814\n37.90847\n37.90881\n37.90914\n37.90948\n37.90981\n37.91015\n37.91048\n37.91082\n37.91115\n37.91149\n37.91182\n37.91216\n37.91249\n37.91283\n37.91316\n37.91350\n37.91383\n37.91417\n37.91450\n37.91483\n37.91517\n37.91550\n37.91584\n37.91617\n37.91651\n37.91684\n37.91718\n37.91751\n37.91785\n37.91818\n37.91851\n37.91885\n37.91918\n37.91952\n37.91985\n37.92019\n37.92052\n37.92085\n37.92119\n37.92152\n37.92186\n37.92219\n37.92253\n37.92286\n37.92319\n37.92353\n37.92386\n37.92420\n37.92453\n37.92486\n37.92520\n37.92553\n37.92587\n37.92620\n37.92654\n37.92687\n37.92720\n37.92754\n37.92787\n37.92821\n37.92854\n37.92887\n37.92921\n37.92954\n37.92987\n37.93021\n37.93054\n37.93088\n37.93121\n37.93154\n37.93188\n37.93221\n37.93255\n37.93288\n37.93321\n37.93355\n37.93388\n37.93421\n37.93455\n37.93488\n37.93522\n37.93555\n37.93588\n37.93622\n37.93655\n37.93688\n37.93722\n37.93755\n37.93788\n37.93822\n37.93855\n37.93889\n37.93922\n37.93955\n37.93989\n37.94022\n37.94055\n37.94089\n37.94122\n37.94155\n37.94189\n37.94223\n37.94256\n37.94290\n37.94323\n37.94356\n37.94390\n37.94423\n37.94457\n37.94490\n37.94523\n37.94557\n37.94590\n37.94623\n37.94657\n37.94690\n37.94723\n37.94757\n37.94790\n37.94823\n37.94857\n37.94890\n37.94923\n37.94957\n37.94990\n37.95023\n37.95057\n37.95090\n37.95123\n37.95157\n37.95190\n37.95223\n37.95257\n37.95290\n37.95323\n37.95357\n37.95390\n37.95423\n37.95457\n37.95490\n37.95523\n37.95557\n37.95590\n37.95623\n37.95656\n37.95690\n37.95723\n37.95756\n37.95790\n37.95823\n37.95856\n37.95890\n37.95923\n37.95956\n37.95990\n37.96023\n37.96056\n37.96090\n37.96123\n37.96156\n37.96190\n37.96223\n37.96256\n37.96290\n37.96323\n37.96356\n37.96390\n37.96423\n37.96456\n37.96490\n37.96523\n37.96556\n37.96589\n37.96623\n37.96656\n37.96689\n37.96723\n37.96756\n37.96789\n37.96823\n37.96856\n37.96889\n37.96923\n37.96956\n37.96989\n37.97023\n37.97056\n37.97089\n37.97123\n37.97156\n37.97189\n37.97223\n37.97256\n37.97289\n37.97323\n37.97356\n37.97389\n37.97422\n37.97456\n37.97489\n37.97522\n37.97556\n37.97589\n37.97622\n37.97656\n37.97689\n37.97722\n37.97756\n37.97789\n37.97822\n37.97856\n37.97889\n37.97922\n37.97956\n37.97989\n37.98022\n37.98056\n37.98089\n37.98122\n37.98156\n37.98189\n37.98222\n37.98256\n37.98289\n37.98322\n37.98356\n37.98389\n37.98422\n37.98456\n37.98489\n37.98522\n37.98556\n37.98589\n37.98622\n37.98656\n37.98689\n37.98722\n37.98756\n37.98789\n37.98822\n37.98856\n37.98889\n37.98923\n37.98956\n37.98989\n37.99023\n37.99056\n37.99089\n37.99123\n37.99156\n37.99189\n37.99223\n37.99256\n37.99289\n37.99323\n37.99356\n37.99390\n37.99423\n37.99456\n37.99490\n37.99523\n37.99556\n37.99590\n37.99623\n37.99656\n37.99690\n37.99723\n37.99757\n37.99790\n37.99823\n37.99857\n37.99890\n37.99923\n37.99957\n37.99990\n38.00024\n38.00057\n38.00090\n38.00124\n38.00157\n38.00191\n38.00224\n38.00257\n38.00291\n38.00324\n38.00358\n38.00391\n38.00424\n38.00458\n38.00492\n38.00526\n38.00559\n38.00592\n38.00626\n38.00659\n38.00693\n38.00726\n38.00759\n38.00793\n38.00826\n38.00860\n38.00893\n38.00927\n38.00960\n38.00993\n38.01027\n38.01060\n38.01094\n38.01127\n38.01161\n38.01194\n38.01227\n38.01261\n38.01294\n38.01328\n38.01361\n38.01395\n38.01428\n38.01462\n38.01495\n38.01528\n38.01562\n38.01595\n38.01629\n38.01662\n38.01696\n38.01729\n38.01763\n38.01796\n38.01830\n38.01863\n38.01897\n38.01930\n38.01964\n38.01997\n38.02031\n38.02064\n38.02098\n38.02131\n38.02165\n38.02198\n38.02232\n38.02265\n38.02299\n38.02332\n38.02366\n38.02399\n38.02433\n38.02466\n38.02500\n38.02533\n38.02567\n38.02600\n38.02634\n38.02667\n38.02701\n38.02734\n38.02768\n38.02801\n38.02835\n38.02868\n38.02902\n38.02935\n38.02969\n38.03003\n38.03036\n38.03070\n38.03103\n38.03137\n38.03170\n38.03204\n38.03237\n38.03271\n38.03305\n38.03338\n38.03372\n38.03405\n38.03439\n38.03472\n38.03506\n38.03540\n38.03573\n38.03607\n38.03640\n38.03674\n38.03708\n38.03741\n38.03775\n38.03808\n38.03842\n38.03876\n38.03909\n38.03943\n38.03977\n38.04010\n38.04044\n38.04077\n38.04111\n38.04145\n38.04178\n38.04212\n38.04246\n38.04279\n38.04313\n38.04347\n38.04380\n38.04414\n38.04448\n38.04481\n38.04515\n38.04549\n38.04582\n38.04616\n38.04650\n38.04683\n38.04718\n38.04752\n38.04785\n38.04819\n38.04853\n38.04887\n38.04920\n38.04954\n38.04988\n38.05021\n38.05055\n38.05089\n38.05123\n38.05156\n38.05190\n38.05224\n38.05258\n38.05291\n38.05325\n38.05359\n38.05393\n38.05426\n38.05460\n38.05494\n38.05528\n38.05561\n38.05595\n38.05629\n38.05663\n38.05696\n38.05730\n38.05764\n38.05798\n38.05832\n38.05865\n38.05899\n38.05933\n38.05967\n38.06001\n38.06034\n38.06068\n38.06102\n38.06136\n38.06170\n38.06204\n38.06237\n38.06271\n38.06305\n38.06339\n38.06373\n38.06407\n38.06441\n38.06474\n38.06508\n38.06542\n38.06576\n38.06610\n38.06644\n38.06678\n38.06712\n38.06746\n38.06779\n38.06813\n38.06847\n38.06881\n38.06915\n38.06949\n38.06983\n38.07017\n38.07051\n38.07085\n38.07119\n38.07153\n38.07187\n38.07221\n38.07254\n38.07288\n38.07322\n38.07356\n38.07390\n38.07424\n38.07458\n38.07492\n38.07526\n38.07560\n38.07594\n38.07628\n38.07662\n38.07696\n38.07730\n38.07764\n38.07798\n38.07832\n38.07866\n38.07900\n38.07935\n38.07969\n38.08003\n38.08037\n38.08071\n38.08106\n38.08140\n38.08174\n38.08208\n38.08242\n38.08276\n38.08310\n38.08344\n38.08378\n38.08413\n38.08447\n38.08481\n38.08515\n38.08549\n38.08583\n38.08617\n38.08651\n38.08686\n38.08720\n38.08754\n38.08788\n38.08822\n38.08856\n38.08891\n38.08925\n38.08959\n38.08993\n38.09027\n38.09061\n38.09096\n38.09130\n38.09164\n38.09198\n38.09233\n38.09267\n38.09301\n38.09335\n38.09369\n38.09404\n38.09438\n38.09472\n38.09506\n38.09541\n38.09575\n38.09609\n38.09644\n38.09678\n38.09712\n38.09746\n38.09781\n38.09815\n38.09849\n38.09884\n38.09918\n38.09952\n38.09987\n38.10021\n38.10055\n38.10090\n38.10124\n38.10158\n38.10193\n38.10227\n38.10261\n38.10296\n38.10330\n38.10365\n38.10399\n38.10433\n38.10468\n38.10502\n38.10537\n38.10571\n38.10605\n38.10640\n38.10674\n38.10709\n38.10743\n38.10778\n38.10812\n38.10847\n38.10881\n38.10915\n38.10951\n38.10985\n38.11020\n38.11054\n38.11089\n38.11123\n38.11158\n38.11192\n38.11227\n38.11262\n38.11296\n38.11331\n38.11365\n38.11400\n38.11434\n38.11469\n38.11503\n38.11538\n38.11573\n38.11607\n38.11642\n38.11676\n38.11711\n38.11746\n38.11780\n38.11815\n38.11849\n38.11884\n38.11919\n38.11953\n38.11988\n38.12023\n38.12057\n38.12092\n38.12127\n38.12161\n38.12196\n38.12231\n38.12265\n38.12300\n38.12335\n38.12370\n38.12404\n38.12439\n38.12474\n38.12509\n38.12543\n38.12578\n38.12613\n38.12648\n38.12682\n38.12717\n38.12752\n38.12787\n38.12822\n38.12856\n38.12891\n38.12926\n38.12961\n38.12996\n38.13030\n38.13065\n38.13100\n38.13135\n38.13170\n38.13205\n38.13240\n38.13275\n38.13309\n38.13344\n38.13379\n38.13414\n38.13449\n38.13485\n38.13520\n38.13555\n38.13590\n38.13625\n38.13660\n38.13695\n38.13730\n38.13765\n38.13800\n38.13835\n38.13870\n38.13905\n38.13940\n38.13975\n38.14010\n38.14045\n38.14080\n38.14115\n38.14150\n38.14185\n38.14220\n38.14255\n38.14290\n38.14325\n38.14360\n38.14395\n38.14431\n38.14466\n38.14501\n38.14536\n38.14571\n38.14606\n38.14641\n38.14677\n38.14712\n38.14747\n38.14782\n38.14817\n38.14852\n38.14888\n38.14923\n38.14958\n38.14993\n38.15029\n38.15064\n38.15099\n38.15134\n38.15170\n38.15205\n38.15240\n38.15275\n38.15311\n38.15346\n38.15381\n38.15417\n38.15452\n38.15487\n38.15523\n38.15558\n38.15593\n38.15629\n38.15664\n38.15699\n38.15735\n38.15771\n38.15806\n38.15842\n38.15877\n38.15913\n38.15948\n38.15984\n38.16019\n38.16054\n38.16090\n38.16125\n38.16161\n38.16196\n38.16232\n38.16267\n38.16303\n38.16338\n38.16374\n38.16409\n38.16445\n38.16480\n38.16516\n38.16552\n38.16587\n38.16623\n38.16658\n38.16694\n38.16729\n38.16765\n38.16801\n38.16836\n38.16872\n38.16908\n38.16943\n38.16979\n38.17015\n38.17050\n38.17086\n38.17122\n38.17157\n38.17193\n38.17229\n38.17264\n38.17300\n38.17336\n38.17372\n38.17407\n38.17443\n38.17479\n38.17515\n38.17550\n38.17586\n38.17622\n38.17658\n38.17694\n38.17730\n38.17765\n38.17801\n38.17837\n38.17874\n38.17910\n38.17946\n38.17982\n38.18017\n38.18053\n38.18089\n38.18125\n38.18161\n38.18197\n38.18233\n38.18269\n38.18305\n38.18341\n38.18377\n38.18413\n38.18449\n38.18485\n38.18521\n38.18557\n38.18593\n38.18629\n38.18665\n38.18701\n38.18737\n38.18773\n38.18809\n38.18845\n38.18882\n38.18918\n38.18954\n38.18990\n38.19026\n38.19062\n38.19098\n38.19135\n38.19171\n38.19207\n38.19243\n38.19279\n38.19316\n38.19352\n38.19388\n38.19424\n38.19461\n38.19497\n38.19533\n38.19569\n38.19606\n38.19642\n38.19678\n38.19715\n38.19751\n38.19788\n38.19825\n38.19861\n38.19897\n38.19934\n38.19970\n38.20006\n38.20043\n38.20079\n38.20116\n38.20152\n38.20188\n38.20225\n38.20261\n38.20298\n38.20334\n38.20371\n38.20407\n38.20444\n38.20480\n38.20517\n38.20553\n38.20590\n38.20626\n38.20663\n38.20700\n38.20736\n38.20773\n38.20809\n38.20846\n38.20883\n38.20919\n38.20956\n38.20993\n38.21029\n38.21066\n38.21103\n38.21139\n38.21176\n38.21213\n38.21249\n38.21286\n38.21323\n38.21360\n38.21396\n38.21433\n38.21470\n38.21507\n38.21543\n38.21580\n38.21618\n38.21655\n38.21692\n38.21729\n38.21765\n38.21802\n38.21839\n38.21876\n38.21913\n38.21950\n38.21987\n38.22024\n38.22061\n38.22098\n38.22135\n38.22172\n38.22209\n38.22246\n38.22283\n38.22320\n38.22357\n38.22394\n38.22431\n38.22468\n38.22505\n38.22542\n38.22579\n38.22616\n38.22653\n38.22690\n38.22727\n38.22765\n38.22802\n38.22839\n38.22876\n38.22913\n38.22950\n38.22988\n38.23025\n38.23062\n38.23099\n38.23137\n38.23174\n38.23211\n38.23248\n38.23286\n38.23323\n38.23361\n38.23399\n38.23436\n38.23473\n38.23511\n38.23548\n38.23585\n38.23623\n38.23660\n38.23698\n38.23735\n38.23772\n38.23810\n38.23847\n38.23885\n38.23922\n38.23960\n38.23997\n38.24035\n38.24072\n38.24110\n38.24147\n38.24185\n38.24222\n38.24260\n38.24298\n38.24335\n38.24373\n38.24410\n38.24448\n38.24486\n38.24523\n38.24561\n38.24599\n38.24636\n38.24674\n38.24712\n38.24750\n38.24787\n38.24825\n38.24863\n38.24901\n38.24938\n38.24976\n38.25015\n38.25053\n38.25091\n38.25128\n38.25166\n38.25204\n38.25242\n38.25280\n38.25318\n38.25356\n38.25394\n38.25432\n38.25469\n38.25507\n38.25545\n38.25583\n38.25621\n38.25659\n38.25697\n38.25735\n38.25773\n38.25811\n38.25850\n38.25888\n38.25926\n38.25964\n38.26002\n38.26040\n38.26078\n38.26116\n38.26154\n38.26193\n38.26231\n38.26269\n38.26307\n38.26345\n38.26384\n38.26422\n38.26460\n38.26498\n38.26537\n38.26576\n38.26614\n38.26653\n38.26691\n38.26729\n38.26768\n38.26806\n38.26844\n38.26883\n38.26921\n38.26960\n38.26998\n38.27036\n38.27075\n38.27113\n38.27152\n38.27190\n38.27229\n38.27267\n38.27306\n38.27344\n38.27383\n38.27422\n38.27460\n38.27499\n38.27537\n38.27576\n38.27615\n38.27653\n38.27692\n38.27731\n38.27769\n38.27808\n38.27847\n38.27885\n38.27924\n38.27963\n38.28002\n38.28040\n38.28080\n38.28119\n38.28158\n38.28197\n38.28235\n38.28274\n38.28313\n38.28352\n38.28391\n38.28430\n38.28469\n38.28508\n38.28547\n38.28586\n38.28624\n38.28663\n38.28702\n38.28741\n38.28780\n38.28820\n38.28859\n38.28898\n38.28937\n38.28976\n38.29015\n38.29054\n38.29093\n38.29132\n38.29171\n38.29211\n38.29250\n38.29289\n38.29328\n38.29367\n38.29407\n38.29446\n38.29485\n38.29525\n38.29565\n38.29604\n38.29643\n38.29683\n38.29722\n38.29761\n38.29801\n38.29840\n38.29879\n38.29919\n38.29958\n38.29998\n38.30037\n38.30077\n38.30116\n38.30156\n38.30195\n38.30235\n38.30274\n38.30314\n38.30353\n38.30393\n38.30432\n38.30472\n38.30512\n38.30551\n38.30591\n38.30631\n38.30670\n38.30710\n38.30750\n38.30789\n38.30829\n38.30869\n38.30909\n38.30949\n38.30989\n38.31029\n38.31069\n38.31109\n38.31148\n38.31188\n38.31228\n38.31268\n38.31308\n38.31348\n38.31388\n38.31428\n38.31468\n38.31508\n38.31548\n38.31588\n38.31628\n38.31668\n38.31708\n38.31748\n38.31788\n38.31828\n38.31868\n38.31908\n38.31948\n38.31988\n38.32029\n38.32069\n38.32109\n38.32149\n38.32189\n38.32230\n38.32270\n38.32311\n38.32351\n38.32392\n38.32432\n38.32472\n38.32513\n38.32553\n38.32593\n38.32634\n38.32674\n38.32715\n38.32755\n38.32795\n38.32836\n38.32876\n38.32917\n38.32957\n38.32998\n38.33038\n38.33079\n38.33119\n38.33160\n38.33201\n38.33241\n38.33282\n38.33323\n38.33363\n38.33404\n38.33445\n38.33485\n38.33526\n38.33567\n38.33607\n38.33649\n38.33690\n38.33731\n38.33772\n38.33812\n38.33853\n38.33894\n38.33935\n38.33976\n38.34017\n38.34058\n38.34099\n38.34139\n38.34180\n38.34221\n38.34262\n38.34303\n38.34344\n38.34385\n38.34427\n38.34468\n38.34509\n38.34550\n38.34591\n38.34632\n38.34673\n38.34714\n38.34756\n38.34797\n38.34838\n38.34879\n38.34921\n38.34963\n38.35004\n38.35045\n38.35087\n38.35128\n38.35169\n38.35211\n38.35252\n38.35293\n38.35335\n38.35376\n38.35418\n38.35459\n38.35501\n38.35542\n38.35584\n38.35625\n38.35667\n38.35708\n38.35750\n38.35791\n38.35833\n38.35874\n38.35916\n38.35958\n38.35999\n38.36041\n38.36083\n38.36125\n38.36167\n38.36209\n38.36251\n38.36293\n38.36334\n38.36376\n38.36418\n38.36460\n38.36502\n38.36544\n38.36585\n38.36627\n38.36669\n38.36711\n38.36753\n38.36795\n38.36837\n38.36879\n38.36921\n38.36963\n38.37005\n38.37047\n38.37089\n38.37132\n38.37174\n38.37216\n38.37258\n38.37300\n38.37342\n38.37385\n38.37428\n38.37470\n38.37512\n38.37555\n38.37597\n38.37639\n38.37682\n38.37724\n38.37766\n38.37809\n38.37851\n38.37893\n38.37936\n38.37978\n38.38021\n38.38063\n38.38106\n38.38148\n38.38191\n38.38233\n38.38276\n38.38319\n38.38361\n38.38404\n38.38447\n38.38489\n38.38532\n38.38575\n38.38618\n38.38661\n38.38704\n38.38747\n38.38789\n38.38832\n38.38875\n38.38918\n38.38961\n38.39003\n38.39046\n38.39089\n38.39132\n38.39175\n38.39218\n38.39261\n38.39304\n38.39347\n38.39390\n38.39433\n38.39476\n38.39519\n38.39562\n38.39606\n38.39649\n38.39692\n38.39735\n38.39779\n38.39822\n38.39866\n38.39909\n38.39952\n38.39995\n38.40039\n38.40082\n38.40125\n38.40169\n38.40212\n38.40256\n38.40299\n38.40342\n38.40386\n38.40429\n38.40473\n38.40516\n38.40560\n38.40603\n38.40647\n38.40690\n38.40734\n38.40778\n38.40821\n38.40865\n38.40909\n38.40953\n38.40997\n38.41041\n38.41084\n38.41128\n38.41172\n38.41216\n38.41260\n38.41303\n38.41347\n38.41391\n38.41435\n38.41479\n38.41523\n38.41567\n38.41611\n38.41655\n38.41699\n38.41743\n38.41787\n38.41831\n38.41875\n38.41919\n38.41963\n38.42007\n38.42052\n38.42097\n38.42141\n38.42185\n38.42229\n38.42274\n38.42318\n38.42362\n38.42406\n38.42451\n38.42495\n38.42539\n38.42584\n38.42628\n38.42673\n38.42717\n38.42762\n38.42806\n38.42851\n38.42895\n38.42940\n38.42984\n38.43029\n38.43073\n38.43118\n38.43163\n38.43208\n38.43253\n38.43298\n38.43342\n38.43387\n38.43432\n38.43477\n38.43521\n38.43566\n38.43611\n38.43656\n38.43701\n38.43746\n38.43791\n38.43835\n38.43880\n38.43925\n38.43970\n38.44015\n38.44060\n38.44105\n38.44151\n38.44196\n38.44241\n38.44286\n38.44332\n38.44377\n38.44422\n38.44468\n38.44513\n38.44558\n38.44603\n38.44649\n38.44694\n38.44739\n38.44785\n38.44830\n38.44875\n38.44921\n38.44966\n38.45012\n38.45057\n38.45103\n38.45148\n38.45194\n38.45239\n38.45285\n38.45330\n38.45376\n38.45423\n38.45468\n38.45514\n38.45560\n38.45605\n38.45651\n38.45697\n38.45743\n38.45788\n38.45834\n38.45880\n38.45926\n38.45972\n38.46018\n38.46064\n38.46109\n38.46155\n38.46201\n38.46247\n38.46293\n38.46340\n38.46386\n38.46432\n38.46479\n38.46525\n38.46571\n38.46617\n38.46663\n38.46710\n38.46756\n38.46802\n38.46848\n38.46895\n38.46941\n38.46987\n38.47034\n38.47080\n38.47126\n38.47173\n38.47219\n38.47266\n38.47312\n38.47359\n38.47405\n38.47452\n38.47498\n38.47546\n38.47593\n38.47639\n38.47686\n38.47733\n38.47779\n38.47826\n38.47873\n38.47920\n38.47966\n38.48013\n38.48060\n38.48107\n38.48154\n38.48201\n38.48247\n38.48294\n38.48341\n38.48388\n38.48435\n38.48482\n38.48529\n38.48577\n38.48625\n38.48672\n38.48719\n38.48766\n38.48813\n38.48860\n38.48908\n38.48955\n38.49002\n38.49049\n38.49097\n38.49144\n38.49191\n38.49239\n38.49286\n38.49333\n38.49381\n38.49428\n38.49476\n38.49523\n38.49571\n38.49619\n38.49667\n38.49715\n38.49762\n38.49810\n38.49857\n38.49905\n38.49953\n38.50001\n38.50048\n38.50096\n38.50144\n38.50192\n38.50240\n38.50287\n38.50335\n38.50383\n38.50431\n38.50479\n38.50527\n38.50575\n38.50624\n38.50672\n38.50720\n38.50768\n38.50816\n38.50864\n38.50913\n38.50961\n38.51009\n38.51057\n38.51105\n38.51154\n38.51202\n38.51250\n38.51299\n38.51347\n38.51395\n38.51444\n38.51492\n38.51541\n38.51589\n38.51639\n38.51687\n38.51736\n38.51784\n38.51833\n38.51882\n38.51930\n38.51979\n38.52027\n38.52076\n38.52125\n38.52174\n38.52222\n38.52271\n38.52320\n38.52369\n38.52418\n38.52467\n38.52516\n38.52565\n38.52614\n38.52663\n38.52712\n38.52761\n38.52811\n38.52860\n38.52909\n38.52958\n38.53007\n38.53056\n38.53105\n38.53155\n38.53204\n38.53253\n38.53302\n38.53352\n38.53401\n38.53450\n38.53500\n38.53549\n38.53600\n38.53649\n38.53699\n38.53748\n38.53798\n38.53847\n38.53897\n38.53946\n38.53996\n38.54046\n38.54095\n38.54145\n38.54195\n38.54244\n38.54294\n38.54344\n38.54394\n38.54444\n38.54493\n38.54543\n38.54594\n38.54644\n38.54694\n38.54744\n38.54794\n38.54844\n38.54894\n38.54944\n38.54994\n38.55045\n38.55095\n38.55145\n38.55195\n38.55245\n38.55296\n38.55346\n38.55396\n38.55447\n38.55497\n38.55548\n38.55599\n38.55649\n38.55700\n38.55750\n38.55800\n38.55851\n38.55902\n38.55952\n38.56003\n38.56053\n38.56104\n38.56155\n38.56205\n38.56256\n38.56307\n38.56358\n38.56408\n38.56459\n38.56511\n38.56562\n38.56613\n38.56664\n38.56715\n38.56766\n38.56817\n38.56868\n38.56919\n38.56970\n38.57021\n38.57072\n38.57123\n38.57174\n38.57226\n38.57277\n38.57328\n38.57379\n38.57431\n38.57483\n38.57534\n38.57586\n38.57637\n38.57688\n38.57740\n38.57791\n38.57843\n38.57894\n38.57946\n38.57998\n38.58049\n38.58101\n38.58152\n38.58204\n38.58256\n38.58308\n38.58359\n38.58412\n38.58464\n38.58516\n38.58568\n38.58620\n38.58671\n38.58723\n38.58775\n38.58827\n38.58879\n38.58931\n38.58983\n38.59036\n38.59088\n38.59140\n38.59192\n38.59244\n38.59296\n38.59350\n38.59402\n38.59454\n38.59507\n38.59559\n38.59611\n38.59664\n38.59716\n38.59769\n38.59821\n38.59874\n38.59926\n38.59979\n38.60031\n38.60084\n38.60137\n38.60189\n38.60242\n38.60296\n38.60348\n38.60401\n38.60454\n38.60507\n38.60560\n38.60613\n38.60665\n38.60718\n38.60771\n38.60824\n38.60877\n38.60930\n38.60984\n38.61037\n38.61090\n38.61143\n38.61197\n38.61250\n38.61303\n38.61357\n38.61410\n38.61463\n38.61517\n38.61570\n38.61623\n38.61677\n38.61730\n38.61784\n38.61837\n38.61891\n38.61944\n38.61998\n38.62052\n38.62106\n38.62160\n38.62214\n38.62267\n38.62321\n38.62375\n38.62429\n38.62482\n38.62536\n38.62590\n38.62644\n38.62698\n38.62752\n38.62806\n38.62860\n38.62914\n38.62968\n38.63023\n38.63077\n38.63131\n38.63186\n38.63240\n38.63294\n38.63348\n38.63403\n38.63457\n38.63511\n38.63566\n38.63620\n38.63675\n38.63729\n38.63783\n38.63838\n38.63893\n38.63948\n38.64003\n38.64057\n38.64112\n38.64167\n38.64221\n38.64276\n38.64331\n38.64386\n38.64440\n38.64495\n38.64550\n38.64605\n38.64660\n38.64715\n38.64770\n38.64826\n38.64881\n38.64936\n38.64991\n38.65046\n38.65102\n38.65157\n38.65212\n38.65267\n38.65322\n38.65378\n38.65433\n38.65488\n38.65544\n38.65599\n38.65655\n38.65711\n38.65767\n38.65822\n38.65878\n38.65933\n38.65989\n38.66045\n38.66100\n38.66156\n38.66212\n38.66267\n38.66323\n38.66379\n38.66435\n38.66491\n38.66547\n38.66604\n38.66660\n38.66716\n38.66772\n38.66828\n38.66884\n38.66940\n38.66996\n38.67052\n38.67108\n38.67165\n38.67221\n38.67277\n38.67333\n38.67390\n38.67446\n38.67504\n38.67560\n38.67616\n38.67673\n38.67729\n38.67786\n38.67843\n38.67899\n38.67956\n38.68012\n38.68069\n38.68126\n38.68183\n38.68239\n38.68296\n38.68354\n38.68411\n38.68468\n38.68525\n38.68582\n38.68639\n38.68696\n38.68753\n38.68810\n38.68867\n38.68924\n38.68981\n38.69038\n38.69096\n38.69153\n38.69210\n38.69268\n38.69326\n38.69383\n38.69441\n38.69498\n38.69555\n38.69613\n38.69670\n38.69728\n38.69786\n38.69843\n38.69901\n38.69959\n38.70016\n38.70074\n38.70133\n38.70191\n38.70248\n38.70306\n38.70364\n38.70422\n38.70480\n38.70538\n38.70596\n38.70654\n38.70712\n38.70770\n38.70828\n38.70886\n38.70945\n38.71004\n38.71062\n38.71120\n38.71179\n38.71237\n38.71295\n38.71354\n38.71412\n38.71471\n38.71529\n38.71588\n38.71646\n38.71705\n38.71763\n38.71823\n38.71882\n38.71940\n38.71999\n38.72058\n38.72117\n38.72176\n38.72234\n38.72293\n38.72352\n38.72411\n38.72470\n38.72529\n38.72588\n38.72647\n38.72707\n38.72767\n38.72826\n38.72885\n38.72944\n38.73003\n38.73063\n38.73122\n38.73181\n38.73241\n38.73300\n38.73360\n38.73419\n38.73479\n38.73539\n38.73599\n38.73658\n38.73718\n38.73778\n38.73837\n38.73897\n38.73957\n38.74017\n38.74077\n38.74136\n38.74196\n38.74256\n38.74316\n38.74377\n38.74437\n38.74497\n38.74557\n38.74618\n38.74678\n38.74738\n38.74798\n38.74858\n38.74919\n38.74979\n38.75039\n38.75100\n38.75160\n38.75220\n38.75282\n38.75342\n38.75403\n38.75464\n38.75524\n38.75585\n38.75645\n38.75706\n38.75767\n38.75828\n38.75888\n38.75949\n38.76010\n38.76072\n38.76133\n38.76194\n38.76255\n38.76316\n38.76377\n38.76438\n38.76499\n38.76560\n38.76621\n38.76683\n38.76744\n38.76805\n38.76866\n38.76929\n38.76990\n38.77052\n38.77113\n38.77174\n38.77236\n38.77297\n38.77359\n38.77421\n38.77482\n38.77544\n38.77606\n38.77667\n38.77729\n38.77792\n38.77854\n38.77916\n38.77978\n38.78039\n38.78101\n38.78163\n38.78225\n38.78287\n38.78350\n38.78412\n38.78474\n38.78536\n38.78599\n38.78662\n38.78724\n38.78786\n38.78849\n38.78911\n38.78973\n38.79036\n38.79098\n38.79161\n38.79223\n38.79286\n38.79349\n38.79412\n38.79475\n38.79538\n38.79600\n38.79663\n38.79726\n38.79789\n38.79852\n38.79915\n38.79978\n38.80041\n38.80104\n38.80167\n38.80230\n38.80294\n38.80357\n38.80420\n38.80484\n38.80547\n38.80610\n38.80674\n38.80737\n38.80800\n38.80864\n38.80927\n38.80991\n38.81054\n38.81119\n38.81182\n38.81246\n38.81310\n38.81373\n38.81437\n38.81501\n38.81565\n38.81629\n38.81692\n38.81756\n38.81820\n38.81885\n38.81949\n38.82013\n38.82077\n38.82142\n38.82206\n38.82270\n38.82334\n38.82398\n38.82463\n38.82527\n38.82591\n38.82656\n38.82721\n38.82786\n38.82850\n38.82915\n38.82979\n38.83044\n38.83108\n38.83173\n38.83238\n38.83303\n38.83367\n38.83432\n38.83497\n38.83563\n38.83628\n38.83693\n38.83758\n38.83823\n38.83888\n38.83953\n38.84018\n38.84083\n38.84148\n38.84214\n38.84279\n38.84345\n38.84411\n38.84476\n38.84541\n38.84607\n38.84672\n38.84738\n38.84803\n38.84869\n38.84934\n38.85000\n38.85066\n38.85131\n38.85198\n38.85264\n38.85330\n38.85396\n38.85462\n38.85528\n38.85594\n38.85660\n38.85726\n38.85792\n38.85858\n38.85924\n38.85991\n38.86057\n38.86124\n38.86190\n38.86256\n38.86323\n38.86389\n38.86455\n38.86522\n38.86588\n38.86655\n38.86721\n38.86789\n38.86856\n38.86922\n38.86989\n38.87056\n38.87123\n38.87189\n38.87256\n38.87323\n38.87390\n38.87457\n38.87524\n38.87592\n38.87659\n38.87726\n38.87794\n38.87861\n38.87928\n38.87995\n38.88063\n38.88130\n38.88197\n38.88265\n38.88332\n38.88401\n38.88468\n38.88536\n38.88603\n38.88671\n38.88738\n38.88806\n38.88874\n38.88942\n38.89009\n38.89077\n38.89145\n38.89214\n38.89282\n38.89350\n38.89418\n38.89486\n38.89554\n38.89622\n38.89691\n38.89759\n38.89827\n38.89895\n38.89964\n38.90033\n38.90101\n38.90170\n38.90238\n38.90307\n38.90375\n38.90444\n38.90513\n38.90581\n38.90650\n38.90719\n38.90788\n38.90857\n38.90926\n38.90995\n38.91064\n38.91133\n38.91202\n38.91271\n38.91340\n38.91409\n38.91478\n38.91547\n38.91617\n38.91687\n38.91756\n38.91825\n38.91895\n38.91964\n38.92034\n38.92103\n38.92172\n38.92242\n38.92312\n38.92381\n38.92452\n38.92522\n38.92591\n38.92661\n38.92731\n38.92801\n38.92871\n38.92941\n38.93011\n38.93081\n38.93151\n38.93222\n38.93292\n38.93362\n38.93432\n38.93502\n38.93573\n38.93643\n38.93713\n38.93784\n38.93854\n38.93925\n38.93996\n38.94067\n38.94137\n38.94208\n38.94278\n38.94349\n38.94420\n38.94491\n38.94561\n38.94632\n38.94703\n38.94775\n38.94846\n38.94917\n38.94988\n38.95059\n38.95130\n38.95201\n38.95273\n38.95344\n38.95415\n38.95486\n38.95559\n38.95630\n38.95701\n38.95773\n38.95844\n38.95916\n38.95988\n38.96059\n38.96131\n38.96202\n38.96274\n38.96347\n38.96419\n38.96491\n38.96562\n38.96634\n38.96706\n38.96778\n38.96850\n38.96922\n38.96995\n38.97067\n38.97140\n38.97212\n38.97284\n38.97357\n38.97429\n38.97502\n38.97574\n38.97646\n38.97719\n38.97791\n38.97864\n38.97938\n38.98010\n38.98083\n38.98156\n38.98229\n38.98301\n38.98374\n38.98447\n38.98520\n38.98593\n38.98666\n38.98740\n38.98813\n38.98886\n38.98960\n38.99033\n38.99106\n38.99179\n38.99253\n38.99326\n38.99399\n38.99473\n38.99547\n38.99621\n38.99695\n38.99768\n38.99842\n38.99916\n38.99989\n39.00063\n39.00137\n39.00211\n39.00286\n39.00360\n39.00433\n39.00507\n39.00582\n39.00656\n39.00730\n39.00804\n39.00878\n39.00952\n39.01027\n39.01102\n39.01176\n39.01251\n39.01325\n39.01400\n39.01474\n39.01549\n39.01624\n39.01698\n39.01773\n39.01849\n39.01923\n39.01998\n39.02073\n39.02148\n39.02223\n39.02298\n39.02373\n39.02448\n39.02523\n39.02599\n39.02674\n39.02750\n39.02825\n39.02900\n39.02976\n39.03051\n39.03126\n39.03202\n39.03277\n39.03353\n39.03430\n39.03505\n39.03581\n39.03657\n39.03732\n39.03808\n39.03884\n39.03960\n39.04036\n39.04112\n39.04189\n39.04265\n39.04341\n39.04417\n39.04493\n39.04569\n39.04646\n39.04722\n39.04798\n39.04875\n39.04952\n39.05028\n39.05105\n39.05181\n39.05258\n39.05335\n39.05411\n39.05488\n39.05565\n39.05642\n39.05719\n39.05796\n39.05873\n39.05950\n39.06027\n39.06104\n39.06181\n39.06258\n39.06336\n39.06413\n39.06491\n39.06568\n39.06646\n39.06723\n39.06800\n39.06878\n39.06955\n39.07033\n39.07110\n39.07188\n39.07267\n39.07344\n39.07422\n39.07500\n39.07578\n39.07656\n39.07734\n39.07812\n39.07890\n39.07968\n39.08047\n39.08125\n39.08203\n39.08281\n39.08359\n39.08438\n39.08516\n39.08594\n39.08673\n39.08751\n39.08831\n39.08909\n39.08988\n39.09067\n39.09145\n39.09224\n39.09303\n39.09382\n39.09460\n39.09539\n39.09619\n39.09698\n39.09777\n39.09856\n39.09935\n39.10015\n39.10094\n39.10173\n39.10252\n39.10333\n39.10412\n39.10491\n39.10571\n39.10650\n39.10730\n39.10809\n39.10889\n39.10969\n39.11048\n39.11129\n39.11209\n39.11289\n39.11369\n39.11448\n39.11528\n39.11608\n39.11689\n39.11769\n39.11850\n39.11930\n39.12010\n39.12090\n39.12171\n39.12251\n39.12331\n39.12412\n39.12492\n39.12573\n39.12654\n39.12735\n39.12816\n39.12896\n39.12977\n39.13058\n39.13139\n39.13220\n39.13301\n39.13382\n39.13463\n39.13545\n39.13626\n39.13707\n39.13788\n39.13869\n39.13950\n39.14032\n39.14113\n39.14195\n39.14277\n39.14358\n39.14440\n39.14521\n39.14603\n39.14685\n39.14766\n39.14848\n39.14931\n39.15013\n39.15095\n39.15177\n39.15259\n39.15341\n39.15423\n39.15505\n39.15587\n39.15670\n39.15752\n39.15835\n39.15917\n39.15999\n39.16082\n39.16164\n39.16247\n39.16329\n39.16412\n39.16495\n39.16578\n39.16661\n39.16743\n39.16826\n39.16909\n39.16992\n39.17075\n39.17158\n39.17242\n39.17325\n39.17408\n39.17491\n39.17575\n39.17658\n39.17741\n39.17824\n39.17908\n39.17992\n39.18076\n39.18159\n39.18243\n39.18326\n39.18410\n39.18494\n39.18578\n39.18661\n39.18746\n39.18830\n39.18914\n39.18998\n39.19082\n39.19166\n39.19250\n39.19334\n39.19418\n39.19504\n39.19588\n39.19672\n39.19757\n39.19841\n39.19926\n39.20010\n39.20095\n39.20179\n39.20265\n39.20350\n39.20434\n39.20519\n39.20604\n39.20689\n39.20774\n39.20859\n39.20944\n39.21030\n39.21115\n39.21200\n39.21285\n39.21370\n39.21456\n39.21541\n39.21626\n39.21712\n39.21798\n39.21884\n39.21969\n39.22055\n39.22141\n39.22226\n39.22312\n39.22398\n39.22484\n39.22570\n39.22656\n39.22742\n39.22828\n39.22914\n39.23001\n39.23087\n39.23173\n39.23260\n39.23346\n39.23433\n39.23519\n39.23606\n39.23692\n39.23779\n39.23865\n39.23952\n39.24039\n39.24126\n39.24213\n39.24300\n39.24387\n39.24473\n39.24560\n39.24647\n39.24734\n39.24822\n39.24910\n39.24997\n39.25084\n39.25171\n39.25259\n39.25346\n39.25433\n39.25521\n39.25609\n39.25697\n39.25784\n39.25872\n39.25960\n39.26047\n39.26135\n39.26223\n39.26312\n39.26400\n39.26488\n39.26576\n39.26664\n39.26752\n39.26840\n39.26928\n39.27017\n39.27106\n39.27194\n39.27283\n39.27371\n39.27459\n39.27548\n39.27637\n39.27725\n39.27815\n39.27904\n39.27992\n39.28081\n39.28170\n39.28259\n39.28348\n39.28437\n39.28526\n39.28616\n39.28705\n39.28794\n39.28884\n39.28973\n39.29062\n39.29152\n39.29241\n39.29331\n39.29421\n39.29511\n39.29600\n39.29690\n39.29779\n39.29869\n39.29959\n39.30050\n39.30140\n39.30230\n39.30320\n39.30410\n39.30500\n39.30590\n39.30680\n39.30770\n39.30862\n39.30952\n39.31042\n39.31133\n39.31223\n39.31314\n39.31404\n39.31495\n39.31587\n39.31677\n39.31768\n39.31859\n39.31950\n39.32041\n39.32132\n39.32223\n39.32315\n39.32406\n39.32497\n39.32588\n39.32679\n39.32771\n39.32862\n39.32953\n39.33045\n39.33137\n39.33229\n39.33320\n39.33412\n39.33504\n39.33595\n39.33687\n39.33779\n39.33872\n39.33964\n39.34056\n39.34148\n39.34240\n39.34332\n39.34424\n39.34516\n39.34610\n39.34702\n39.34794\n39.34887\n39.34979\n39.35072\n39.35164\n39.35257\n39.35350\n39.35443\n39.35536\n39.35629\n39.35722\n39.35814\n39.35907\n39.36000\n39.36094\n39.36188\n39.36281\n39.36374\n39.36467\n39.36560\n39.36654\n39.36747\n39.36842\n39.36935\n39.37029\n39.37122\n39.37216\n39.37309\n39.37403\n39.37497\n39.37592\n39.37686\n39.37780\n39.37874\n39.37968\n39.38062\n39.38156\n39.38250\n39.38345\n39.38439\n39.38534\n39.38628\n39.38722\n39.38817\n39.38911\n39.39006\n39.39102\n39.39196\n39.39291\n39.39386\n39.39481\n39.39575\n39.39670\n39.39765\n39.39861\n39.39956\n39.40052\n39.40147\n39.40242\n39.40337\n39.40433\n39.40528\n39.40624\n39.40720\n39.40815\n39.40911\n39.41006\n39.41102\n39.41198\n39.41295\n39.41390\n39.41486\n39.41582\n39.41678\n39.41774\n39.41870\n39.41966\n39.42064\n39.42160\n39.42256\n39.42352\n39.42449\n39.42545\n39.42642\n39.42738\n39.42836\n39.42932\n39.43029\n39.43126\n39.43222\n39.43319\n39.43416\n39.43513\n39.43611\n39.43708\n39.43805\n39.43902\n39.43999\n39.44097\n39.44194\n39.44292\n39.44390\n39.44487\n39.44584\n39.44682\n39.44780\n39.44877\n39.44975\n39.45074\n39.45171\n39.45269\n39.45367\n39.45465\n39.45563\n39.45661\n39.45759\n39.45858\n39.45957\n39.46055\n39.46153\n39.46251\n39.46350\n39.46448\n39.46548\n39.46646\n39.46745\n39.46844\n39.46942\n39.47041\n39.47140\n39.47239\n39.47339\n39.47437\n39.47536\n39.47636\n39.47735\n39.47834\n39.47933\n39.48033\n39.48133\n39.48232\n39.48331\n39.48431\n39.48530\n39.48630\n39.48730\n39.48830\n39.48930\n39.49030\n39.49130\n39.49230\n39.49329\n39.49429\n39.49530\n39.49631\n39.49731\n39.49831\n39.49931\n39.50031\n39.50132\n39.50232\n39.50334\n39.50434\n39.50535\n39.50635\n39.50736\n39.50837\n39.50937\n39.51039\n39.51140\n39.51241\n39.51342\n39.51443\n39.51544\n39.51645\n39.51747\n39.51849\n39.51950\n39.52051\n39.52153\n39.52254\n39.52356\n39.52457\n39.52560\n39.52661\n39.52763\n39.52865\n39.52967\n39.53069\n39.53170\n39.53273\n39.53375\n39.53478\n39.53580\n39.53682\n39.53784\n39.53886\n39.53990\n39.54092\n39.54195\n39.54297\n39.54400\n39.54502\n39.54605\n39.54708\n39.54811\n39.54914\n39.55017\n39.55120\n39.55223\n39.55326\n39.55429\n39.55533\n39.55636\n39.55739\n39.55843\n39.55946\n39.56049\n39.56153\n39.56257\n39.56361\n39.56465\n39.56568\n39.56672\n39.56776\n39.56879\n39.56984\n39.57088\n39.57192\n39.57296\n39.57400\n39.57504\n39.57609\n39.57714\n39.57818\n39.57923\n39.58027\n39.58131\n39.58236\n39.58340\n39.58446\n39.58551\n39.58655\n39.58760\n39.58865\n39.58970\n39.59075\n39.59181\n39.59286\n39.59391\n39.59496\n39.59601\n39.59707\n39.59812\n39.59917\n39.60024\n39.60129\n39.60235\n39.60340\n39.60446\n39.60552\n39.60657\n39.60764\n39.60870\n39.60976\n39.61082\n39.61188\n39.61294\n39.61400\n39.61507\n39.61613\n39.61720\n39.61826\n39.61932\n39.62039\n39.62145\n39.62253\n39.62359\n39.62466\n39.62573\n39.62680\n39.62786\n39.62893\n39.63001\n39.63108\n39.63215\n39.63322\n39.63429\n39.63537\n39.63645\n39.63752\n39.63859\n39.63967\n39.64074\n39.64182\n39.64289\n39.64398\n39.64506\n39.64614\n39.64721\n39.64829\n39.64937\n39.65045\n39.65154\n39.65262\n39.65370\n39.65478\n39.65587\n39.65695\n39.65803\n39.65913\n39.66021\n39.66130\n39.66238\n39.66347\n39.66455\n39.66564\n39.66674\n39.66783\n39.66892\n39.67001\n39.67110\n39.67219\n39.67328\n39.67438\n39.67547\n39.67656\n39.67766\n39.67875\n39.67985\n39.68094\n39.68205\n39.68314\n39.68424\n39.68534\n39.68643\n39.68753\n39.68864\n39.68974\n39.69084\n39.69194\n39.69304\n39.69414\n39.69525\n39.69636\n39.69746\n39.69857\n39.69967\n39.70077\n39.70188\n39.70299\n39.70410\n39.70521\n39.70632\n39.70743\n39.70853\n39.70964\n39.71075\n39.71187\n39.71298\n39.71410\n39.71521\n39.71632\n39.71743\n39.71856\n39.71967\n39.72079\n39.72190\n39.72302\n39.72413\n39.72525\n39.72638\n39.72750\n39.72862\n39.72974\n39.73086\n39.73198\n39.73310\n39.73423\n39.73535\n39.73647\n39.73760\n39.73872\n39.73985\n39.74098\n39.74211\n39.74323\n39.74436\n39.74549\n39.74661\n39.74774\n39.74888\n39.75001\n39.75114\n39.75227\n39.75340\n39.75453\n39.75568\n39.75681\n39.75794\n39.75908\n39.76021\n39.76135\n39.76248\n39.76363\n39.76476\n39.76590\n39.76704\n39.76818\n39.76932\n39.77046\n39.77161\n39.77275\n39.77389\n39.77503\n39.77617\n39.77732\n39.77847\n39.77961\n39.78076\n39.78190\n39.78305\n39.78419\n39.78534\n39.78650\n39.78765\n39.78880\n39.78995\n39.79110\n39.79225\n39.79341\n39.79456\n39.79571\n39.79686\n39.79802\n39.79917\n39.80033\n39.80149\n39.80264\n39.80380\n39.80496\n39.80611\n39.80727\n39.80844\n39.80960\n39.81076\n39.81192\n39.81308\n39.81424\n39.81541\n39.81657\n39.81774\n39.81890\n39.82006\n39.82123\n39.82239\n39.82357\n39.82474\n39.82590\n39.82707\n39.82824\n39.82941\n39.83059\n39.83176\n39.83293\n39.83410\n39.83527\n39.83644\n39.83762\n39.83880\n39.83997\n39.84115\n39.84232\n39.84350\n39.84467\n39.84586\n39.84704\n39.84821\n39.84939\n39.85057\n39.85175\n39.85294\n39.85412\n39.85530\n39.85648\n39.85767\n39.85885\n39.86004\n39.86123\n39.86241\n39.86360\n39.86478\n39.86597\n39.86716\n39.86836\n39.86954\n39.87073\n39.87192\n39.87311\n39.87430\n39.87550\n39.87670\n39.87789\n39.87908\n39.88027\n39.88147\n39.88267\n39.88387\n39.88506\n39.88626\n39.88746\n39.88865\n39.88985\n39.89106\n39.89226\n39.89346\n39.89466\n39.89586\n39.89706\n39.89828\n39.89948\n39.90068\n39.90189\n39.90309\n39.90430\n39.90551\n39.90672\n39.90792\n39.90913\n39.91034\n39.91155\n39.91277\n39.91398\n39.91519\n39.91640\n39.91761\n39.91882\n39.92005\n39.92126\n39.92247\n39.92369\n39.92490\n39.92612\n39.92734\n39.92856\n39.92978\n39.93100\n39.93222\n39.93343\n39.93465\n39.93588\n39.93711\n39.93833\n39.93955\n39.94077\n39.94200\n39.94323\n39.94445\n39.94568\n39.94690\n39.94813\n39.94936\n39.95060\n39.95182\n39.95305\n39.95428\n39.95551\n39.95674\n39.95798\n39.95921\n39.96045\n39.96168\n39.96291\n39.96415\n39.96539\n39.96663\n39.96786\n39.96910\n39.97034\n39.97157\n39.97282\n39.97406\n39.97530\n39.97654\n39.97778\n39.97902\n39.98027\n39.98151\n39.98276\n39.98400\n39.98525\n39.98649\n39.98775\n39.98899\n39.99024\n39.99148\n39.99273\n39.99398\n39.99524\n39.99649\n39.99774\n39.99899\n40.00024\n40.00149\n40.00276\n40.00401\n40.00526\n40.00652\n40.00777\n40.00903\n40.01029\n40.01155\n40.01281\n40.01406\n40.01532\n40.01658\n40.01785\n40.01911\n40.02037\n40.02163\n40.02290\n40.02416\n40.02543\n40.02670\n40.02796\n40.02922\n40.03049\n40.03176\n40.03303\n40.03430\n40.03557\n40.03684\n40.03811\n40.03938\n40.04066\n40.04193\n40.04320\n40.04447\n40.04575\n40.04702\n40.04830\n40.04958\n40.05085\n40.05213\n40.05340\n40.05469\n40.05597\n40.05725\n40.05853\n40.05981\n40.06109\n40.06238\n40.06366\n40.06494\n40.06622\n40.06751\n40.06879\n40.07008\n40.07137\n40.07265\n40.07394\n40.07523\n40.07652\n40.07781\n40.07910\n40.08039\n40.08168\n40.08297\n40.08426\n40.08556\n40.08686\n40.08815\n40.08944\n40.09074\n40.09203\n40.09334\n40.09463\n40.09593\n40.09723\n40.09852\n40.09983\n40.10113\n40.10243\n40.10373\n40.10503\n40.10633\n40.10765\n40.10895\n40.11025\n40.11156\n40.11286\n40.11416\n40.11548\n40.11679\n40.11809\n40.11940\n40.12071\n40.12202\n40.12334\n40.12465\n40.12596\n40.12727\n40.12858\n40.12990\n40.13122\n40.13253\n40.13384\n40.13516\n40.13647\n40.13780\n40.13912\n40.14043\n40.14175\n40.14307\n40.14439\n40.14572\n40.14704\n40.14836\n40.14968\n40.15101\n40.15233\n40.15366\n40.15499\n40.15631\n40.15764\n40.15896\n40.16030\n40.16163\n40.16295\n40.16428\n40.16561\n40.16694\n40.16828\n40.16961\n40.17094\n40.17228\n40.17361\n40.17494\n40.17629\n40.17762\n40.17896\n40.18029\n40.18163\n40.18297\n40.18431\n40.18565\n40.18699\n40.18833\n40.18967\n40.19102\n40.19236\n40.19370\n40.19505\n40.19639\n40.19774\n40.19909\n40.20043\n40.20178\n40.20313\n40.20447\n40.20583\n40.20718\n40.20853\n40.20988\n40.21123\n40.21258\n40.21394\n40.21529\n40.21664\n40.21800\n40.21935\n40.22071\n40.22207\n40.22343\n40.22478\n40.22614\n40.22750\n40.22886\n40.23022\n40.23158\n40.23294\n40.23430\n40.23568\n40.23704\n40.23840\n40.23976\n40.24113\n40.24249\n40.24387\n40.24523\n40.24660\n40.24797\n40.24933\n40.25071\n40.25208\n40.25345\n40.25482\n40.25619\n40.25756\n40.25894\n40.26032\n40.26169\n40.26306\n40.26444\n40.26582\n40.26720\n40.26858\n40.26995\n40.27133\n40.27271\n40.27410\n40.27548\n40.27686\n40.27824\n40.27962\n40.28101\n40.28239\n40.28378\n40.28516\n40.28655\n40.28793\n40.28933\n40.29071\n40.29210\n40.29349\n40.29488\n40.29628\n40.29767\n40.29906\n40.30045\n40.30184\n40.30323\n40.30463\n40.30603\n40.30742\n40.30881\n40.31021\n40.31162\n40.31301\n40.31441\n40.31581\n40.31721\n40.31861\n40.32002\n40.32142\n40.32282\n40.32422\n40.32562\n40.32703\n40.32844\n40.32984\n40.33125\n40.33265\n40.33407\n40.33547\n40.33688\n40.33829\n40.33970\n40.34111\n40.34253\n40.34394\n40.34535\n40.34676\n40.34817\n40.34960\n40.35101\n40.35242\n40.35384\n40.35526\n40.35667\n40.35810\n40.35952\n40.36093\n40.36235\n40.36377\n40.36520\n40.36662\n40.36804\n40.36947\n40.37089\n40.37232\n40.37375\n40.37517\n40.37660\n40.37802\n40.37945\n40.38089\n40.38231\n40.38374\n40.38517\n40.38660\n40.38804\n40.38947\n40.39090\n40.39234\n40.39377\n40.39521\n40.39665\n40.39808\n40.39952\n40.40095\n40.40239\n40.40384\n40.40527\n40.40671\n40.40815\n40.40959\n40.41104\n40.41248\n40.41393\n40.41537\n40.41681\n40.41827\n40.41971\n40.42116\n40.42260\n40.42405\n40.42550\n40.42695\n40.42840\n40.42985\n40.43130\n40.43275\n40.43421\n40.43566\n40.43711\n40.43857\n40.44002\n40.44148\n40.44294\n40.44439\n40.44585\n40.44731\n40.44877\n40.45023\n40.45169\n40.45315\n40.45461\n40.45608\n40.45754\n40.45900\n40.46047\n40.46193\n40.46339\n40.46487\n40.46633\n40.46780\n40.46926\n40.47073\n40.47221\n40.47368\n40.47515\n40.47662\n40.47809\n40.47957\n40.48104\n40.48251\n40.48398\n40.48546\n40.48694\n40.48842\n40.48989\n40.49137\n40.49284\n40.49433\n40.49581\n40.49729\n40.49877\n40.50025\n40.50173\n40.50322\n40.50470\n40.50618\n40.50767\n40.50915\n40.51065\n40.51213\n40.51362\n40.51510\n40.51659\n40.51809\n40.51958\n40.52107\n40.52256\n40.52405\n40.52555\n40.52704\n40.52853\n40.53002\n40.53152\n40.53302\n40.53452\n40.53601\n40.53751\n40.53901\n40.54051\n40.54201\n40.54351\n40.54501\n40.54651\n40.54802\n40.54952\n40.55103\n40.55253\n40.55403\n40.55554\n40.55705\n40.55856\n40.56006\n40.56157\n40.56308\n40.56459\n40.56610\n40.56761\n40.56912\n40.57063\n40.57215\n40.57367\n40.57518\n40.57669\n40.57821\n40.57973\n40.58125\n40.58276\n40.58428\n40.58580\n40.58732\n40.58884\n40.59036\n40.59188\n40.59340\n40.59493\n40.59645\n40.59798\n40.59950\n40.60102\n40.60256\n40.60408\n40.60561\n40.60714\n40.60866\n40.61020\n40.61173\n40.61326\n40.61479\n40.61632\n40.61786\n40.61939\n40.62092\n40.62246\n40.62399\n40.62553\n40.62707\n40.62861\n40.63014\n40.63168\n40.63323\n40.63476\n40.63630\n40.63784\n40.63938\n40.64093\n40.64248\n40.64402\n40.64556\n40.64711\n40.64866\n40.65020\n40.65175\n40.65330\n40.65484\n40.65640\n40.65795\n40.65950\n40.66105\n40.66260\n40.66416\n40.66571\n40.66726\n40.66882\n40.67037\n40.67193\n40.67349\n40.67504\n40.67660\n40.67816\n40.67972\n40.68128\n40.68284\n40.68440\n40.68596\n40.68753\n40.68909\n40.69065\n40.69222\n40.69378\n40.69536\n40.69692\n40.69849\n40.70005\n40.70162\n40.70320\n40.70476\n40.70633\n40.70790\n40.70947\n40.71105\n40.71263\n40.71420\n40.71577\n40.71734\n40.71893\n40.72050\n40.72208\n40.72365\n40.72523\n40.72682\n40.72840\n40.72998\n40.73155\n40.73314\n40.73473\n40.73631\n40.73789\n40.73947\n40.74107\n40.74265\n40.74423\n40.74582\n40.74741\n40.74900\n40.75059\n40.75218\n40.75377\n40.75536\n40.75696\n40.75855\n40.76014\n40.76173\n40.76332\n40.76493\n40.76652\n40.76812\n40.76971\n40.77131\n40.77292\n40.77451\n40.77611\n40.77771\n40.77931\n40.78092\n40.78252\n40.78412\n40.78573\n40.78733\n40.78894\n40.79055\n40.79215\n40.79376\n40.79537\n40.79698\n40.79859\n40.80020\n40.80180\n40.80342\n40.80503\n40.80665\n40.80826\n40.80987\n40.81149\n40.81311\n40.81472\n40.81633\n40.81795\n40.81958\n40.82119\n40.82281\n40.82443\n40.82605\n40.82768\n40.82930\n40.83092\n40.83254\n40.83416\n40.83580\n40.83742\n40.83905\n40.84067\n40.84231\n40.84393\n40.84556\n40.84719\n") -> (array=w7:dbl[][])  [unwired: 2 in]
  n3 = Spreadsheet String To Array(format string="%f", spreadsheet string="0.000490\n0.000510\n0.000590\n0.000450\n0.000090\n0.000170\n0.000260\n0.000250\n0.000200\n0.000140\n0.000100\n0.000060\n0.000040\n0.000020\n0.000010\n0.000010\n0.000010\n0.000005\n0.000005\n0.000005\n0.000005\n0.000005\n0.000005\n0.000005\n0.000005\n0.000005\n0.000005\n0.000005\n0.000005\n0.000005\n0.000005\n0.000005\n0.000005\n0.000005\n0.000005\n0.000005\n0.000005\n0.000005\n0.000005\n0.000005\n0.000005\n0.000005\n0.000005\n0.000005\n0.000005\n0.000005\n0.000005\n0.000005\n0.000005\n0.000005\n0.000005\n0.000005\n0.000005\n0.000005\n0.000005\n0.000005\n0.000005\n0.000005\n0.000005\n0.000005\n0.000005\n0.000005\n0.000005\n0.000005\n0.000005\n0.000005\n0.000005\n0.000005\n0.000005\n0.000005\n0.000005\n0.000005\n0.000005\n0.000005\n0.000005\n0.000005\n0.000005\n0.000005\n0.000005\n0.000005\n0.000005\n0.000005\n0.000005\n0.000005\n0.000005\n0.000005\n0.000005\n0.000005\n0.000005\n0.000005\n0.000005\n0.000005\n0.000005\n0.000005\n0.000005\n0.000005\n0.000005\n0.000005\n0.000005\n0.000005\n0.000005\n0.000005\n0.000005\n0.000005\n0.000005\n0.000005\n0.000005\n0.000005\n0.000005\n0.000005\n0.000005\n0.000005\n0.000005\n0.000005\n0.000005\n0.000005\n0.000005\n0.000005\n0.000005\n0.000005\n0.000005\n0.000005\n0.000005\n0.000005\n0.000005\n0.000005\n0.000005\n0.000005\n0.000005\n0.000005\n0.000005\n0.000005\n0.000005\n0.000005\n0.000005\n0.000005\n0.000005\n0.000005\n0.000005\n0.000005\n0.000005\n0.000005\n0.000005\n0.000005\n0.000005\n0.000005\n0.000005\n0.000005\n0.000005\n0.000005\n0.000005\n0.000005\n0.000005\n0.000005\n0.000005\n0.000005\n0.000005\n0.000005\n0.000005\n0.000005\n0.000005\n0.000005\n0.000005\n0.000005\n0.000005\n0.000005\n0.000005\n0.000005\n0.000005\n0.000005\n0.000005\n0.000005\n0.000005\n0.000005\n0.000005\n0.000005\n0.000005\n0.000005\n0.000005\n0.000005\n0.000005\n0.000005\n0.000005\n0.000005\n0.000005\n0.000005\n0.000005\n0.000005\n0.000005\n0.000005\n0.000005\n0.000005\n0.000005\n0.000005\n0.000005\n0.000005\n0.000005\n0.000005\n0.000005\n0.000005\n0.000005\n0.000005\n0.000005\n0.000005\n0.000005\n0.000005\n0.000005\n0.000005\n0.000005\n0.000005\n0.000005\n0.000005\n0.000005\n0.000005\n0.000005\n0.000005\n0.000005\n0.000005\n0.000005\n0.000005\n0.000005\n0.000005\n0.000005\n0.000005\n0.000005\n0.000005\n0.000005\n0.000005\n0.000005\n0.000005\n0.000005\n0.000005\n0.000005\n0.000005\n0.000005\n0.000005\n0.000005\n0.000005\n0.000005\n0.000005\n0.000005\n0.000005\n0.000005\n0.000005\n0.000005\n0.000005\n0.000005\n0.000005\n0.000005\n0.000005\n0.000005\n0.000005\n0.000005\n0.000005\n0.000005\n0.000005\n0.000005\n0.000005\n0.000005\n0.000005\n0.000005\n0.000005\n0.000005\n0.000005\n0.000005\n0.000005\n0.000005\n0.000005\n0.000005\n0.000005\n0.000005\n0.000005\n0.000005\n0.000005\n0.000005\n0.000005\n0.000005\n0.000005\n0.000005\n0.000005\n0.000005\n0.000005\n0.000005\n0.000005\n0.000005\n0.000005\n0.000005\n0.000005\n0.000005\n0.000005\n0.000005\n0.000005\n0.000005\n0.000005\n0.000005\n0.000005\n0.000005\n0.000005\n0.000005\n0.000005\n0.000005\n0.000005\n0.000005\n0.000005\n0.000005\n0.000005\n0.000005\n0.000005\n0.000005\n0.000005\n0.000005\n0.000005\n0.000005\n0.000005\n0.000005\n0.000005\n0.000005\n0.000005\n0.000005\n0.000005\n0.000005\n0.000005\n0.000005\n0.000005\n0.000005\n0.000005\n0.000005\n0.000005\n0.000005\n0.000005\n0.000005\n0.000005\n0.000005\n0.000005\n0.000005\n0.000005\n0.000005\n0.000005\n0.000005\n0.000005\n0.000005\n0.000005\n0.000005\n0.000005\n0.000005\n0.000005\n0.000005\n0.000005\n0.000005\n0.000005\n0.000005\n0.000005\n0.000005\n0.000005\n0.000005\n0.000005\n0.000005\n0.000005\n0.000005\n0.000005\n0.000005\n0.000005\n0.000005\n0.000005\n0.000005\n0.000005\n0.000005\n0.000005\n0.000005\n0.000005\n0.000005\n0.000005\n0.000005\n0.000005\n0.000005\n0.000005\n0.000005\n0.000005\n0.000005\n0.000005\n0.000005\n0.000005\n0.000005\n0.000005\n0.000005\n0.000005\n0.000005\n0.000005\n0.000005\n0.000005\n0.000005\n0.000005\n0.000005\n0.000005\n0.000005\n0.000005\n0.000005\n0.000005\n0.000005\n0.000005\n0.000005\n0.000005\n0.000005\n0.000005\n0.000005\n0.000005\n0.000005\n0.000005\n0.000005\n0.000005\n0.000005\n0.000005\n0.000005\n0.000005\n0.000005\n0.000005\n0.000005\n0.000005\n0.000005\n0.000005\n0.000005\n0.000005\n0.000005\n0.000005\n0.000005\n0.000005\n0.000005\n0.000005\n0.000005\n0.000005\n0.000005\n0.000005\n0.000005\n0.000005\n0.000005\n0.000005\n0.000005\n0.000005\n0.000005\n0.000005\n0.000005\n0.000005\n0.000005\n0.000005\n0.000005\n0.000005\n0.000005\n0.000005\n0.000005\n0.000005\n0.000005\n0.000005\n0.000005\n0.000005\n0.000005\n0.000005\n0.000005\n0.000005\n0.000005\n0.000005\n0.000005\n0.000005\n0.000005\n0.000005\n0.000005\n0.000005\n0.000005\n0.000005\n0.000005\n0.000005\n0.000005\n0.000005\n0.000005\n0.000005\n0.000005\n0.000005\n0.000005\n0.000005\n0.000005\n0.000005\n0.000005\n0.000005\n0.000005\n0.000005\n0.000005\n0.000005\n0.000005\n0.000005\n0.000005\n0.000005\n0.000005\n0.000005\n0.000005\n0.000005\n0.000005\n0.000005\n0.000005\n0.000005\n0.000005\n0.000005\n0.000005\n0.000005\n0.000005\n0.000005\n0.000005\n0.000005\n0.000005\n0.000005\n0.000005\n0.000005\n0.000005\n0.000005\n0.000005\n0.000005\n0.000005\n0.000005\n0.000005\n0.000005\n0.000005\n0.000005\n0.000005\n0.000005\n0.000005\n0.000005\n0.000005\n0.000005\n0.000005\n0.000005\n0.000005\n0.000005\n0.000005\n0.000005\n0.000005\n0.000005\n0.000005\n0.000005\n0.000005\n0.000005\n0.000005\n0.000005\n0.000005\n0.000005\n0.000005\n0.000005\n0.000005\n0.000005\n0.000005\n0.000005\n0.000005\n0.000005\n0.000005\n0.000005\n0.000005\n0.000005\n0.000005\n0.000005\n0.000005\n0.000005\n0.000005\n0.000005\n0.000005\n0.000005\n0.000005\n0.000005\n0.000005\n0.000005\n0.000005\n0.000005\n0.000005\n0.000005\n0.000005\n0.000005\n0.000005\n0.000005\n0.000005\n0.000005\n0.000005\n0.000005\n0.000005\n0.000005\n0.000005\n0.000005\n0.000005\n0.000005\n0.000005\n0.000005\n0.000005\n0.000005\n0.000005\n0.000005\n0.000005\n0.000005\n0.000005\n0.000005\n0.000005\n0.000005\n0.000005\n0.000005\n0.000005\n0.000005\n0.000005\n0.000005\n0.000005\n0.000005\n0.000005\n0.000005\n0.000005\n0.000005\n0.000005\n0.000005\n0.000005\n0.000005\n0.000005\n0.000005\n0.000005\n0.000005\n0.000005\n0.000005\n0.000005\n0.000005\n0.000005\n0.000005\n0.000005\n0.000005\n0.000005\n0.000005\n0.000005\n0.000005\n0.000005\n0.000005\n0.000005\n0.000005\n0.000005\n0.000005\n0.000005\n0.000005\n0.000005\n0.000005\n0.000005\n0.000005\n0.000005\n0.000005\n0.000005\n0.000005\n0.000005\n0.000005\n0.000005\n0.000005\n0.000005\n0.000005\n0.000005\n0.000005\n0.000005\n0.000005\n0.000005\n0.000005\n0.000005\n0.000005\n0.000005\n0.000005\n0.000005\n0.000005\n0.000005\n0.000005\n0.000005\n0.000005\n0.000005\n0.000005\n0.000005\n0.000005\n0.000005\n0.000005\n0.000005\n0.000005\n0.000005\n0.000005\n0.000005\n0.000005\n0.000005\n0.000005\n0.000005\n0.000005\n0.000005\n0.000005\n0.000005\n0.000005\n0.000005\n0.000005\n0.000005\n0.000005\n0.000005\n0.000005\n0.000005\n0.000005\n0.000005\n0.000005\n0.000005\n0.000005\n0.000005\n0.000005\n0.000005\n0.000005\n0.000005\n0.000005\n0.000005\n0.000005\n0.000005\n0.000005\n0.000005\n0.000005\n0.000005\n0.000005\n0.000005\n0.000005\n0.000005\n0.000005\n0.000005\n0.000005\n0.000005\n0.000005\n0.000005\n0.000005\n0.000005\n0.000005\n0.000005\n0.000005\n0.000005\n0.000005\n0.000005\n0.000005\n0.000005\n0.000005\n0.000005\n0.000005\n0.000005\n0.000005\n0.000005\n0.000005\n0.000005\n0.000005\n0.000005\n0.000005\n0.000005\n0.000005\n0.000005\n0.000005\n0.000005\n0.000005\n0.000005\n0.000005\n0.000005\n0.000005\n0.000005\n0.000005\n0.000005\n0.000005\n0.000005\n0.000005\n0.000005\n0.000005\n0.000005\n0.000005\n0.000005\n0.000005\n0.000005\n0.000005\n0.000005\n0.000005\n0.000005\n0.000005\n0.000005\n0.000005\n0.000005\n0.000005\n0.000005\n0.000005\n0.000005\n0.000005\n0.000005\n0.000005\n0.000005\n0.000005\n0.000005\n0.000005\n0.000005\n0.000005\n0.000005\n0.000005\n0.000005\n0.000005\n0.000005\n0.000005\n0.000005\n0.000005\n0.000005\n0.000005\n0.000005\n0.000005\n0.000005\n0.000005\n0.000005\n0.000005\n0.000005\n0.000005\n0.000005\n0.000005\n0.000005\n0.000005\n0.000005\n0.000005\n0.000005\n0.000005\n0.000005\n0.000005\n0.000005\n0.000005\n0.000005\n0.000005\n0.000005\n0.000005\n0.000005\n0.000005\n0.000005\n0.000005\n0.000005\n0.000005\n0.000005\n0.000005\n0.000005\n0.000005\n0.000005\n0.000005\n0.000005\n0.000005\n0.000005\n0.000005\n0.000005\n0.000005\n0.000005\n0.000005\n0.000005\n0.000005\n0.000005\n0.000005\n0.000005\n0.000005\n0.000005\n0.000005\n0.000005\n0.000005\n0.000005\n0.000005\n0.000005\n0.000005\n0.000005\n0.000005\n0.000005\n0.000005\n0.000005\n0.000005\n0.000005\n0.000005\n0.000005\n0.000005\n0.000005\n0.000005\n0.000005\n0.000005\n0.000005\n0.000005\n0.000005\n0.000005\n0.000005\n0.000005\n0.000005\n0.000005\n0.000005\n0.000005\n0.000005\n0.000005\n0.000005\n0.000005\n0.000005\n0.000005\n0.000005\n0.000005\n0.000005\n0.000005\n0.000005\n0.000005\n0.000005\n0.000005\n0.000005\n0.000005\n0.000005\n0.000005\n0.000005\n0.000005\n0.000005\n0.000005\n0.000005\n0.000005\n0.000005\n0.000005\n0.000005\n0.000005\n0.000005\n0.000005\n0.000005\n0.000005\n0.000005\n0.000005\n0.000005\n0.000005\n0.000005\n0.000005\n0.000005\n0.000005\n0.000005\n0.000005\n0.000005\n0.000005\n0.000005\n0.000005\n0.000005\n0.000005\n0.000005\n0.000005\n0.000005\n0.000005\n0.000005\n0.000005\n0.000005\n0.000005\n0.000005\n0.000005\n0.000005\n0.000005\n0.000005\n0.000005\n0.000005\n0.000005\n0.000005\n0.000005\n0.000005\n0.000005\n0.000005\n0.000005\n0.000005\n0.000005\n0.000005\n0.000005\n0.000005\n0.000005\n0.000005\n0.000005\n0.000005\n0.000005\n0.000005\n0.000005\n0.000005\n0.000005\n0.000005\n0.000005\n0.000005\n0.000005\n0.000005\n0.000005\n0.000005\n0.000005\n0.000005\n0.000005\n0.000005\n0.000005\n0.000005\n0.000005\n0.000005\n0.000005\n0.000005\n0.000005\n0.000005\n0.000005\n0.000005\n0.000005\n0.000005\n0.000005\n0.000005\n0.000005\n0.000005\n0.000005\n0.000005\n0.000005\n0.000005\n0.000005\n0.000005\n0.000005\n0.000005\n0.000005\n0.000005\n0.000005\n0.000005\n0.000005\n0.000005\n0.000005\n0.000005\n0.000005\n0.000005\n0.000005\n0.000005\n0.000005\n0.000005\n0.000005\n0.000005\n0.000005\n0.000005\n0.000005\n0.000005\n0.000005\n0.000005\n0.000005\n0.000005\n0.000005\n0.000005\n0.000005\n0.000005\n0.000005\n0.000005\n0.000005\n0.000005\n0.000005\n0.000005\n0.000005\n0.000005\n0.000005\n0.000005\n0.000005\n0.000005\n0.000005\n0.000005\n0.000005\n0.000005\n0.000005\n0.000005\n0.000005\n0.000005\n0.000005\n0.000005\n0.000005\n0.000005\n0.000005\n0.000005\n0.000005\n0.000005\n0.000005\n0.000005\n0.000005\n0.000005\n0.000005\n0.000005\n0.000005\n0.000005\n0.000005\n0.000005\n0.000005\n0.000005\n0.000005\n0.000005\n0.000005\n0.000005\n0.000005\n0.000005\n0.000005\n0.000005\n0.000005\n0.000005\n0.000005\n0.000005\n0.000005\n0.000005\n0.000005\n0.000005\n0.000005\n0.000005\n0.000005\n0.000005\n0.000005\n0.000005\n0.000005\n0.000005\n0.000005\n0.000005\n0.000005\n0.000005\n0.000005\n0.000005\n0.000005\n0.000005\n0.000005\n0.000005\n0.000005\n0.000005\n0.000005\n0.000005\n0.000005\n0.000005\n0.000005\n0.000005\n0.000005\n0.000005\n0.000005\n0.000005\n0.000005\n0.000005\n0.000005\n0.000005\n0.000005\n0.000005\n0.000005\n0.000005\n0.000005\n0.000005\n0.000005\n0.000005\n0.000005\n0.000005\n0.000005\n0.000005\n0.000005\n0.000005\n0.000005\n0.000005\n0.000005\n0.000005\n0.000005\n0.000005\n0.000005\n0.000005\n0.000005\n0.000005\n0.000005\n0.000005\n0.000005\n0.000005\n0.000005\n0.000005\n0.000005\n0.000005\n0.000005\n0.000005\n0.000005\n0.000005\n0.000005\n0.000005\n0.000005\n0.000005\n0.000005\n0.000005\n0.000005\n0.000005\n0.000005\n0.000005\n0.000005\n0.000005\n0.000005\n0.000005\n0.000005\n0.000005\n0.000005\n0.000010\n0.000005\n0.000005\n0.000010\n0.000005\n0.000005\n0.000005\n0.000005\n0.000005\n0.000005\n0.000005\n0.000005\n0.000005\n0.000005\n0.000005\n0.000005\n0.000010\n0.000005\n0.000005\n0.000005\n0.000005\n0.000005\n0.000010\n0.000010\n0.000005\n0.000005\n0.000005\n0.000005\n0.000010\n0.000005\n0.000005\n0.000005\n0.000005\n0.000005\n0.000005\n0.000005\n0.000005\n0.000010\n0.000005\n0.000005\n0.000005\n0.000005\n0.000005\n0.000005\n0.000010\n0.000005\n0.000005\n0.000010\n0.000005\n0.000005\n0.000005\n0.000005\n0.000005\n0.000010\n0.000005\n0.000005\n0.000010\n0.000010\n0.000005\n0.000005\n0.000010\n0.000010\n0.000005\n0.000005\n0.000005\n0.000005\n0.000005\n0.000005\n0.000005\n0.000005\n0.000005\n0.000010\n0.000005\n0.000005\n0.000005\n0.000005\n0.000005\n0.000005\n0.000005\n0.000005\n0.000005\n0.000005\n0.000005\n0.000005\n0.000010\n0.000005\n0.000005\n0.000005\n0.000005\n0.000010\n0.000005\n0.000010\n0.000005\n0.000005\n0.000005\n0.000005\n0.000005\n0.000005\n0.000010\n0.000005\n0.000010\n0.000005\n0.000005\n0.000005\n0.000005\n0.000005\n0.000005\n0.000005\n0.000005\n0.000005\n0.000005\n0.000005\n0.000005\n0.000005\n0.000005\n0.000005\n0.000005\n0.000005\n0.000005\n0.000005\n0.000010\n0.000010\n0.000005\n0.000010\n0.000005\n0.000005\n0.000005\n0.000010\n0.000005\n0.000005\n0.000005\n0.000005\n0.000005\n0.000010\n0.000010\n0.000005\n0.000005\n0.000005\n0.000005\n0.000005\n0.000010\n0.000005\n0.000005\n0.000005\n0.000005\n0.000005\n0.000010\n0.000005\n0.000005\n0.000005\n0.000005\n0.000005\n0.000005\n0.000005\n0.000005\n0.000005\n0.000005\n0.000005\n0.000010\n0.000010\n0.000005\n0.000005\n0.000005\n0.000005\n0.000005\n0.000005\n0.000005\n0.000010\n0.000005\n0.000005\n0.000005\n0.000010\n0.000005\n0.000005\n0.000005\n0.000005\n0.000005\n0.000005\n0.000010\n0.000005\n0.000005\n0.000005\n0.000005\n0.000010\n0.000005\n0.000005\n0.000010\n0.000005\n0.000005\n0.000005\n0.000010\n0.000005\n0.000005\n0.000005\n0.000005\n0.000010\n0.000010\n0.000005\n0.000010\n0.000005\n0.000010\n0.000005\n0.000010\n0.000005\n0.000010\n0.000005\n0.000010\n0.000005\n0.000010\n0.000005\n0.000010\n0.000010\n0.000010\n0.000005\n0.000010\n0.000010\n0.000010\n0.000005\n0.000005\n0.000005\n0.000005\n0.000005\n0.000005\n0.000010\n0.000010\n0.000010\n0.000005\n0.000010\n0.000005\n0.000005\n0.000005\n0.000005\n0.000010\n0.000005\n0.000005\n0.000010\n0.000005\n0.000010\n0.000005\n0.000010\n0.000010\n0.000005\n0.000010\n0.000010\n0.000010\n0.000010\n0.000005\n0.000010\n0.000005\n0.000005\n0.000005\n0.000005\n0.000005\n0.000005\n0.000005\n0.000005\n0.000005\n0.000010\n0.000005\n0.000010\n0.000005\n0.000005\n0.000005\n0.000010\n0.000005\n0.000005\n0.000005\n0.000005\n0.000005\n0.000005\n0.000005\n0.000010\n0.000005\n0.000005\n0.000010\n0.000010\n0.000010\n0.000005\n0.000005\n0.000005\n0.000005\n0.000005\n0.000005\n0.000005\n0.000005\n0.000005\n0.000010\n0.000005\n0.000010\n0.000005\n0.000005\n0.000005\n0.000005\n0.000005\n0.000005\n0.000010\n0.000005\n0.000010\n0.000005\n0.000005\n0.000010\n0.000010\n0.000010\n0.000010\n0.000005\n0.000005\n0.000010\n0.000005\n0.000010\n0.000005\n0.000010\n0.000010\n0.000005\n0.000005\n0.000005\n0.000005\n0.000005\n0.000005\n0.000010\n0.000005\n0.000005\n0.000010\n0.000005\n0.000010\n0.000005\n0.000005\n0.000010\n0.000005\n0.000005\n0.000005\n0.000005\n0.000005\n0.000005\n0.000005\n0.000005\n0.000005\n0.000005\n0.000005\n0.000010\n0.000010\n0.000005\n0.000005\n0.000010\n0.000005\n0.000005\n0.000010\n0.000005\n0.000010\n0.000005\n0.000010\n0.000005\n0.000010\n0.000005\n0.000010\n0.000005\n0.000010\n0.000005\n0.000010\n0.000005\n0.000005\n0.000010\n0.000005\n0.000010\n0.000005\n0.000010\n0.000005\n0.000010\n0.000005\n0.000010\n0.000005\n0.000010\n0.000005\n0.000010\n0.000005\n0.000005\n0.000010\n0.000005\n0.000010\n0.000010\n0.000005\n0.000005\n0.000010\n0.000010\n0.000010\n0.000010\n0.000005\n0.000005\n0.000005\n0.000010\n0.000010\n0.000010\n0.000005\n0.000005\n0.000010\n0.000010\n0.000005\n0.000010\n0.000005\n0.000010\n0.000005\n0.000005\n0.000010\n0.000010\n0.000010\n0.000005\n0.000005\n0.000010\n0.000010\n0.000010\n0.000005\n0.000010\n0.000010\n0.000005\n0.000005\n0.000010\n0.000005\n0.000005\n0.000005\n0.000005\n0.000005\n0.000010\n0.000010\n0.000005\n0.000010\n0.000005\n0.000010\n0.000010\n0.000005\n0.000005\n0.000005\n0.000005\n0.000010\n0.000005\n0.000010\n0.000005\n0.000010\n0.000010\n0.000005\n0.000005\n0.000010\n0.000010\n0.000005\n0.000010\n0.000005\n0.000010\n0.000010\n0.000010\n0.000010\n0.000005\n0.000005\n0.000010\n0.000010\n0.000005\n0.000005\n0.000005\n0.000005\n0.000010\n0.000005\n0.000010\n0.000005\n0.000005\n0.000005\n0.000005\n0.000010\n0.000005\n0.000010\n0.000005\n0.000005\n0.000005\n0.000010\n0.000010\n0.000005\n0.000005\n0.000010\n0.000010\n0.000005\n0.000005\n0.000010\n0.000010\n0.000005\n0.000005\n0.000010\n0.000010\n0.000005\n0.000005\n0.000010\n0.000010\n0.000005\n0.000010\n0.000005\n0.000010\n0.000010\n0.000005\n0.000005\n0.000010\n0.000010\n0.000010\n0.000010\n0.000010\n0.000005\n0.000010\n0.000010\n0.000010\n0.000005\n0.000010\n0.000005\n0.000005\n0.000005\n0.000005\n0.000010\n0.000010\n0.000010\n0.000010\n0.000010\n0.000010\n0.000005\n0.000005\n0.000005\n0.000010\n0.000005\n0.000005\n0.000005\n0.000010\n0.000010\n0.000010\n0.000010\n0.000010\n0.000005\n0.000010\n0.000010\n0.000010\n0.000005\n0.000010\n0.000010\n0.000010\n0.000010\n0.000005\n0.000005\n0.000005\n0.000010\n0.000010\n0.000010\n0.000010\n0.000010\n0.000005\n0.000005\n0.000005\n0.000005\n0.000010\n0.000010\n0.000010\n0.000010\n0.000005\n0.000005\n0.000005\n0.000005\n0.000010\n0.000010\n0.000010\n0.000005\n0.000010\n0.000010\n0.000010\n0.000005\n0.000010\n0.000010\n0.000005\n0.000010\n0.000010\n0.000010\n0.000010\n0.000010\n0.000010\n0.000010\n0.000005\n0.000005\n0.000005\n0.000010\n0.000005\n0.000010\n0.000005\n0.000010\n0.000010\n0.000010\n0.000010\n0.000010\n0.000010\n0.000010\n0.000010\n0.000010\n0.000010\n0.000005\n0.000010\n0.000010\n0.000005\n0.000005\n0.000005\n0.000010\n0.000010\n0.000010\n0.000005\n0.000010\n0.000010\n0.000010\n0.000005\n0.000005\n0.000005\n0.000010\n0.000010\n0.000010\n0.000005\n0.000010\n0.000010\n0.000010\n0.000005\n0.000005\n0.000010\n0.000005\n0.000005\n0.000010\n0.000010\n0.000010\n0.000010\n0.000010\n0.000010\n0.000005\n0.000010\n0.000010\n0.000005\n0.000005\n0.000005\n0.000010\n0.000010\n0.000010\n0.000005\n0.000010\n0.000005\n0.000010\n0.000010\n0.000010\n0.000010\n0.000010\n0.000010\n0.000010\n0.000010\n0.000010\n0.000010\n0.000010\n0.000005\n0.000010\n0.000005\n0.000010\n0.000010\n0.000010\n0.000010\n0.000010\n0.000005\n0.000010\n0.000005\n0.000010\n0.000010\n0.000010\n0.000010\n0.000010\n0.000010\n0.000010\n0.000010\n0.000010\n0.000005\n0.000010\n0.000005\n0.000010\n0.000010\n0.000010\n0.000010\n0.000010\n0.000010\n0.000010\n0.000010\n0.000010\n0.000010\n0.000010\n0.000010\n0.000010\n0.000010\n0.000005\n0.000005\n0.000010\n0.000010\n0.000010\n0.000010\n0.000010\n0.000010\n0.000005\n0.000010\n0.000010\n0.000010\n0.000010\n0.000005\n0.000010\n0.000010\n0.000010\n0.000010\n0.000010\n0.000010\n0.000010\n0.000010\n0.000005\n0.000010\n0.000010\n0.000005\n0.000010\n0.000005\n0.000005\n0.000010\n0.000010\n0.000010\n0.000010\n0.000010\n0.000010\n0.000010\n0.000005\n0.000005\n0.000010\n0.000005\n0.000010\n0.000005\n0.000005\n0.000010\n0.000010\n0.000005\n0.000010\n0.000010\n0.000010\n0.000005\n0.000010\n0.000010\n0.000010\n0.000010\n0.000010\n0.000010\n0.000010\n0.000010\n0.000010\n0.000010\n0.000010\n0.000010\n0.000010\n0.000010\n0.000010\n0.000010\n0.000010\n0.000010\n0.000010\n0.000010\n0.000010\n0.000010\n0.000005\n0.000005\n0.000010\n0.000010\n0.000005\n0.000010\n0.000010\n0.000005\n0.000010\n0.000010\n0.000010\n0.000010\n0.000010\n0.000010\n0.000005\n0.000010\n0.000010\n0.000010\n0.000010\n0.000010\n0.000010\n0.000010\n0.000010\n0.000010\n0.000010\n0.000010\n0.000010\n0.000010\n0.000010\n0.000010\n0.000010\n0.000010\n0.000010\n0.000010\n0.000010\n0.000010\n0.000010\n0.000010\n0.000010\n0.000010\n0.000005\n0.000010\n0.000010\n0.000010\n0.000010\n0.000005\n0.000010\n0.000010\n0.000010\n0.000010\n0.000010\n0.000010\n0.000010\n0.000010\n0.000010\n0.000010\n0.000010\n0.000010\n0.000010\n0.000010\n0.000010\n0.000010\n0.000010\n0.000010\n0.000010\n0.000010\n0.000010\n0.000010\n0.000010\n0.000010\n0.000010\n0.000010\n0.000010\n0.000010\n0.000010\n0.000010\n0.000010\n0.000010\n0.000010\n0.000010\n0.000010\n0.000010\n0.000010\n0.000010\n0.000010\n0.000010\n0.000010\n0.000010\n0.000010\n0.000010\n0.000010\n0.000010\n0.000010\n0.000010\n0.000010\n0.000010\n0.000010\n0.000010\n0.000010\n0.000010\n0.000010\n0.000010\n0.000010\n0.000010\n0.000010\n0.000010\n0.000010\n0.000010\n0.000010\n0.000010\n0.000010\n0.000010\n0.000010\n0.000010\n0.000010\n0.000010\n0.000010\n0.000010\n0.000010\n0.000010\n0.000010\n0.000010\n0.000010\n0.000010\n0.000010\n0.000010\n0.000010\n0.000010\n0.000010\n0.000010\n0.000010\n0.000010\n0.000010\n0.000010\n0.000010\n0.000010\n0.000010\n0.000010\n0.000010\n0.000010\n0.000010\n0.000010\n0.000010\n0.000010\n0.000010\n0.000010\n0.000010\n0.000010\n0.000010\n0.000010\n0.000010\n0.000010\n0.000010\n0.000010\n0.000010\n0.000010\n0.000010\n0.000010\n0.000010\n0.000010\n0.000010\n0.000010\n0.000010\n0.000010\n0.000010\n0.000010\n0.000010\n0.000010\n0.000010\n0.000010\n0.000010\n0.000010\n0.000010\n0.000010\n0.000010\n0.000010\n0.000010\n0.000010\n0.000010\n0.000010\n0.000010\n0.000010\n0.000010\n0.000010\n0.000010\n0.000010\n0.000010\n0.000010\n0.000010\n0.000010\n0.000010\n0.000010\n0.000010\n0.000010\n0.000010\n0.000010\n0.000010\n0.000010\n0.000010\n0.000010\n0.000010\n0.000010\n0.000010\n0.000010\n0.000010\n0.000010\n0.000010\n0.000010\n0.000010\n0.000010\n0.000010\n0.000010\n0.000010\n0.000010\n0.000010\n0.000010\n0.000010\n0.000010\n0.000010\n0.000010\n0.000010\n0.000010\n0.000010\n0.000010\n0.000010\n0.000010\n0.000010\n0.000010\n0.000010\n0.000010\n0.000010\n0.000010\n0.000010\n0.000010\n0.000010\n0.000010\n0.000010\n0.000010\n0.000010\n0.000010\n0.000010\n0.000010\n0.000010\n0.000010\n0.000010\n0.000010\n0.000010\n0.000010\n0.000010\n0.000010\n0.000010\n0.000010\n0.000010\n0.000010\n0.000010\n0.000010\n0.000010\n0.000010\n0.000010\n0.000010\n0.000010\n0.000010\n0.000010\n0.000010\n0.000010\n0.000010\n0.000010\n0.000010\n0.000010\n0.000010\n0.000010\n0.000010\n0.000010\n0.000010\n0.000010\n0.000010\n0.000010\n0.000010\n0.000010\n0.000010\n0.000010\n0.000010\n0.000010\n0.000010\n0.000010\n0.000010\n0.000010\n0.000010\n0.000010\n0.000010\n0.000010\n0.000010\n0.000010\n0.000010\n0.000010\n0.000010\n0.000010\n0.000010\n0.000010\n0.000010\n0.000010\n0.000010\n0.000010\n0.000010\n0.000010\n0.000010\n0.000010\n0.000010\n0.000010\n0.000010\n0.000010\n0.000010\n0.000010\n0.000010\n0.000010\n0.000010\n0.000010\n0.000010\n0.000010\n0.000010\n0.000010\n0.000010\n0.000010\n0.000010\n0.000010\n0.000010\n0.000010\n0.000010\n0.000010\n0.000010\n0.000010\n0.000010\n0.000010\n0.000010\n0.000010\n0.000010\n0.000010\n0.000010\n0.000010\n0.000010\n0.000010\n0.000010\n0.000010\n0.000010\n0.000010\n0.000010\n0.000010\n0.000010\n0.000010\n0.000010\n0.000010\n0.000010\n0.000010\n0.000010\n0.000010\n0.000010\n0.000010\n0.000010\n0.000010\n0.000010\n0.000010\n0.000010\n0.000010\n0.000010\n0.000010\n0.000010\n0.000010\n0.000010\n0.000010\n0.000010\n0.000010\n0.000010\n0.000010\n0.000010\n0.000010\n0.000010\n0.000010\n0.000010\n0.000010\n0.000010\n0.000010\n0.000010\n0.000010\n0.000010\n0.000010\n0.000010\n0.000010\n0.000010\n0.000010\n0.000010\n0.000010\n0.000010\n0.000010\n0.000010\n0.000010\n0.000010\n0.000010\n0.000010\n0.000010\n0.000010\n0.000010\n0.000010\n0.000010\n0.000010\n0.000010\n0.000010\n0.000010\n0.000010\n0.000010\n0.000010\n0.000010\n0.000010\n0.000010\n0.000010\n0.000010\n0.000010\n0.000010\n0.000010\n0.000010\n0.000010\n0.000010\n0.000010\n0.000010\n0.000010\n0.000010\n0.000010\n0.000010\n0.000010\n0.000010\n0.000010\n0.000010\n0.000010\n0.000010\n0.000010\n0.000010\n0.000010\n0.000010\n0.000010\n0.000010\n0.000010\n0.000010\n0.000010\n0.000010\n0.000010\n0.000010\n0.000020\n0.000010\n0.000010\n0.000010\n0.000020\n0.000010\n0.000010\n0.000010\n0.000010\n0.000010\n0.000010\n0.000020\n0.000010\n0.000010\n0.000010\n0.000010\n0.000010\n0.000010\n0.000010\n0.000010\n0.000010\n0.000010\n0.000010\n0.000010\n0.000010\n0.000010\n0.000020\n0.000010\n0.000010\n0.000010\n0.000010\n0.000010\n0.000020\n0.000010\n0.000020\n0.000020\n0.000010\n0.000010\n0.000010\n0.000020\n0.000010\n0.000010\n0.000010\n0.000020\n0.000010\n0.000010\n0.000010\n0.000020\n0.000020\n0.000010\n0.000020\n0.000010\n0.000020\n0.000020\n0.000010\n0.000020\n0.000010\n0.000010\n0.000020\n0.000010\n0.000010\n0.000010\n0.000010\n0.000020\n0.000020\n0.000020\n0.000010\n0.000020\n0.000020\n0.000020\n0.000020\n0.000020\n0.000010\n0.000010\n0.000020\n0.000010\n0.000010\n0.000010\n0.000020\n0.000010\n0.000020\n0.000010\n0.000010\n0.000020\n0.000020\n0.000020\n0.000010\n0.000020\n0.000020\n0.000020\n0.000020\n0.000010\n0.000010\n0.000010\n0.000020\n0.000020\n0.000020\n0.000020\n0.000020\n0.000020\n0.000010\n0.000010\n0.000010\n0.000020\n0.000020\n0.000020\n0.000020\n0.000020\n0.000020\n0.000020\n0.000020\n0.000020\n0.000020\n0.000020\n0.000020\n0.000020\n0.000020\n0.000010\n0.000010\n0.000020\n0.000020\n0.000020\n0.000020\n0.000020\n0.000020\n0.000020\n0.000020\n0.000020\n0.000020\n0.000020\n0.000020\n0.000020\n0.000020\n0.000020\n0.000020\n0.000020\n0.000020\n0.000020\n0.000020\n0.000020\n0.000020\n0.000020\n0.000020\n0.000020\n0.000020\n0.000020\n0.000020\n0.000020\n0.000020\n0.000020\n0.000020\n0.000020\n0.000020\n0.000020\n0.000020\n0.000020\n0.000020\n0.000020\n0.000020\n0.000020\n0.000020\n0.000020\n0.000020\n0.000020\n0.000020\n0.000020\n0.000020\n0.000020\n0.000020\n0.000020\n0.000020\n0.000020\n0.000020\n0.000020\n0.000020\n0.000020\n0.000020\n0.000020\n0.000020\n0.000020\n0.000020\n0.000020\n0.000020\n0.000020\n0.000020\n0.000020\n0.000020\n0.000020\n0.000020\n0.000020\n0.000020\n0.000020\n0.000020\n0.000020\n0.000020\n0.000020\n0.000020\n0.000020\n0.000020\n0.000020\n0.000020\n0.000020\n0.000020\n0.000020\n0.000020\n0.000020\n0.000020\n0.000020\n0.000020\n0.000020\n0.000020\n0.000020\n0.000020\n0.000020\n0.000020\n0.000020\n0.000020\n0.000020\n0.000020\n0.000020\n0.000020\n0.000020\n0.000020\n0.000020\n0.000020\n0.000020\n0.000020\n0.000020\n0.000020\n0.000020\n0.000020\n0.000020\n0.000020\n0.000020\n0.000020\n0.000020\n0.000020\n0.000020\n0.000020\n0.000020\n0.000020\n0.000020\n0.000020\n0.000020\n0.000020\n0.000020\n0.000020\n0.000020\n0.000020\n0.000020\n0.000020\n0.000020\n0.000020\n0.000020\n0.000020\n0.000020\n0.000020\n0.000020\n0.000020\n0.000020\n0.000020\n0.000020\n0.000020\n0.000020\n0.000020\n0.000020\n0.000020\n0.000020\n0.000020\n0.000020\n0.000020\n0.000020\n0.000020\n0.000020\n0.000020\n0.000020\n0.000020\n0.000020\n0.000020\n0.000020\n0.000020\n0.000020\n0.000020\n0.000020\n0.000020\n0.000020\n0.000020\n0.000020\n0.000020\n0.000020\n0.000020\n0.000020\n0.000020\n0.000020\n0.000020\n0.000020\n0.000020\n0.000020\n0.000020\n0.000020\n0.000020\n0.000020\n0.000020\n0.000020\n0.000020\n0.000020\n0.000020\n0.000020\n0.000020\n0.000020\n0.000020\n0.000020\n0.000020\n0.000020\n0.000020\n0.000020\n0.000020\n0.000020\n0.000020\n0.000020\n0.000020\n0.000020\n0.000020\n0.000020\n0.000020\n0.000030\n0.000020\n0.000020\n0.000020\n0.000020\n0.000020\n0.000020\n0.000030\n0.000030\n0.000020\n0.000020\n0.000030\n0.000020\n0.000020\n0.000020\n0.000030\n0.000020\n0.000020\n0.000020\n0.000020\n0.000020\n0.000030\n0.000020\n0.000030\n0.000020\n0.000020\n0.000030\n0.000030\n0.000020\n0.000030\n0.000030\n0.000030\n0.000030\n0.000020\n0.000030\n0.000030\n0.000020\n0.000020\n0.000030\n0.000030\n0.000030\n0.000020\n0.000030\n0.000030\n0.000020\n0.000030\n0.000020\n0.000030\n0.000030\n0.000030\n0.000030\n0.000030\n0.000030\n0.000030\n0.000030\n0.000030\n0.000030\n0.000030\n0.000030\n0.000030\n0.000030\n0.000020\n0.000030\n0.000030\n0.000030\n0.000030\n0.000030\n0.000030\n0.000030\n0.000030\n0.000030\n0.000030\n0.000030\n0.000030\n0.000030\n0.000030\n0.000030\n0.000030\n0.000030\n0.000030\n0.000030\n0.000030\n0.000030\n0.000030\n0.000030\n0.000030\n0.000030\n0.000030\n0.000030\n0.000030\n0.000030\n0.000030\n0.000030\n0.000030\n0.000030\n0.000030\n0.000030\n0.000030\n0.000030\n0.000030\n0.000030\n0.000030\n0.000030\n0.000030\n0.000030\n0.000030\n0.000030\n0.000030\n0.000030\n0.000030\n0.000030\n0.000030\n0.000030\n0.000030\n0.000030\n0.000030\n0.000030\n0.000030\n0.000030\n0.000030\n0.000030\n0.000030\n0.000030\n0.000030\n0.000030\n0.000030\n0.000030\n0.000030\n0.000030\n0.000030\n0.000030\n0.000030\n0.000030\n0.000030\n0.000030\n0.000030\n0.000030\n0.000030\n0.000030\n0.000030\n0.000030\n0.000030\n0.000030\n0.000030\n0.000030\n0.000030\n0.000030\n0.000030\n0.000030\n0.000030\n0.000030\n0.000030\n0.000030\n0.000030\n0.000030\n0.000030\n0.000030\n0.000030\n0.000030\n0.000030\n0.000030\n0.000030\n0.000030\n0.000030\n0.000030\n0.000030\n0.000030\n0.000030\n0.000030\n0.000030\n0.000030\n0.000030\n0.000030\n0.000030\n0.000030\n0.000030\n0.000040\n0.000030\n0.000030\n0.000030\n0.000040\n0.000030\n0.000040\n0.000030\n0.000030\n0.000030\n0.000030\n0.000030\n0.000040\n0.000030\n0.000040\n0.000040\n0.000030\n0.000040\n0.000040\n0.000040\n0.000040\n0.000030\n0.000040\n0.000040\n0.000040\n0.000040\n0.000030\n0.000040\n0.000030\n0.000040\n0.000040\n0.000040\n0.000040\n0.000040\n0.000040\n0.000040\n0.000040\n0.000040\n0.000040\n0.000040\n0.000040\n0.000040\n0.000040\n0.000040\n0.000040\n0.000040\n0.000040\n0.000040\n0.000040\n0.000040\n0.000040\n0.000040\n0.000040\n0.000040\n0.000040\n0.000040\n0.000040\n0.000040\n0.000040\n0.000040\n0.000040\n0.000040\n0.000040\n0.000040\n0.000040\n0.000040\n0.000040\n0.000040\n0.000040\n0.000040\n0.000040\n0.000040\n0.000040\n0.000040\n0.000040\n0.000040\n0.000040\n0.000040\n0.000040\n0.000050\n0.000040\n0.000050\n0.000040\n0.000040\n0.000040\n0.000040\n0.000050\n0.000040\n0.000050\n0.000040\n0.000040\n0.000040\n0.000040\n0.000040\n0.000040\n0.000050\n0.000040\n0.000040\n0.000050\n0.000050\n0.000050\n0.000050\n0.000040\n0.000050\n0.000040\n0.000050\n0.000050\n0.000050\n0.000050\n0.000050\n0.000050\n0.000050\n0.000050\n0.000050\n0.000050\n0.000050\n0.000050\n0.000050\n0.000050\n0.000050\n0.000050\n0.000050\n0.000050\n0.000050\n0.000050\n0.000050\n0.000050\n0.000050\n0.000050\n0.000050\n0.000050\n0.000050\n0.000050\n0.000050\n0.000050\n0.000050\n0.000050\n0.000050\n0.000050\n0.000050\n0.000050\n0.000050\n0.000050\n0.000050\n0.000050\n0.000050\n0.000050\n0.000050\n0.000050\n0.000050\n0.000050\n0.000050\n0.000050\n0.000050\n0.000050\n0.000050\n0.000050\n0.000050\n0.000050\n0.000050\n0.000050\n0.000050\n0.000050\n0.000050\n0.000050\n0.000050\n0.000050\n0.000050\n0.000050\n0.000050\n0.000050\n0.000050\n0.000050\n0.000050\n0.000050\n0.000050\n0.000050\n0.000050\n0.000050\n0.000050\n0.000050\n0.000050\n0.000050\n0.000050\n0.000050\n0.000050\n0.000050\n0.000050\n0.000050\n0.000050\n0.000060\n0.000060\n0.000060\n0.000060\n0.000060\n0.000050\n0.000060\n0.000050\n0.000060\n0.000060\n0.000050\n0.000050\n0.000050\n0.000060\n0.000060\n0.000050\n0.000060\n0.000060\n0.000060\n0.000060\n0.000060\n0.000060\n0.000060\n0.000060\n0.000060\n0.000060\n0.000060\n0.000060\n0.000060\n0.000060\n0.000060\n0.000060\n0.000060\n0.000060\n0.000060\n0.000060\n0.000060\n0.000060\n0.000060\n0.000060\n0.000060\n0.000060\n0.000060\n0.000060\n0.000060\n0.000060\n0.000060\n0.000060\n0.000060\n0.000060\n0.000060\n0.000060\n0.000060\n0.000060\n0.000060\n0.000060\n0.000060\n0.000060\n0.000060\n0.000060\n0.000060\n0.000060\n0.000060\n0.000060\n0.000060\n0.000060\n0.000060\n0.000060\n0.000060\n0.000060\n0.000060\n0.000060\n0.000060\n0.000060\n0.000060\n0.000060\n0.000060\n0.000060\n0.000060\n0.000060\n0.000060\n0.000060\n0.000070\n0.000060\n0.000060\n0.000060\n0.000070\n0.000070\n0.000060\n0.000060\n0.000070\n0.000070\n0.000070\n0.000060\n0.000070\n0.000070\n0.000070\n0.000070\n0.000070\n0.000070\n0.000070\n0.000070\n0.000070\n0.000070\n0.000070\n0.000070\n0.000070\n0.000070\n0.000070\n0.000070\n0.000070\n0.000070\n0.000070\n0.000070\n0.000070\n0.000070\n0.000070\n0.000070\n0.000070\n0.000070\n0.000070\n0.000070\n0.000070\n0.000070\n0.000070\n0.000070\n0.000070\n0.000070\n0.000070\n0.000070\n0.000070\n0.000070\n0.000070\n0.000070\n0.000070\n0.000080\n0.000080\n0.000080\n0.000080\n0.000080\n0.000070\n0.000080\n0.000080\n0.000070\n0.000080\n0.000080\n0.000080\n0.000080\n0.000080\n0.000080\n0.000080\n0.000080\n0.000080\n0.000080\n0.000080\n0.000080\n0.000080\n0.000080\n0.000080\n0.000080\n0.000080\n0.000080\n0.000080\n0.000080\n0.000080\n0.000080\n0.000080\n0.000080\n0.000080\n0.000080\n0.000080\n0.000080\n0.000080\n0.000080\n0.000080\n0.000080\n0.000080\n0.000080\n0.000080\n0.000080\n0.000080\n0.000080\n0.000080\n0.000080\n0.000080\n0.000080\n0.000080\n0.000080\n0.000080\n0.000080\n0.000080\n0.000080\n0.000080\n0.000080\n0.000080\n0.000080\n0.000080\n0.000080\n0.000080\n0.000080\n0.000080\n0.000080\n0.000080\n0.000080\n0.000080\n0.000080\n0.000090\n0.000090\n0.000080\n0.000090\n0.000090\n0.000080\n0.000090\n0.000090\n0.000090\n0.000090\n0.000090\n0.000090\n0.000090\n0.000090\n0.000090\n0.000090\n0.000090\n0.000090\n0.000090\n0.000090\n0.000090\n0.000090\n0.000090\n0.000090\n0.000090\n0.000090\n0.000090\n0.000090\n0.000090\n0.000090\n0.000090\n0.000090\n0.000090\n0.000090\n0.000090\n0.000100\n0.000090\n0.000090\n0.000090\n0.000100\n0.000090\n0.000090\n0.000090\n0.000090\n0.000090\n0.000090\n0.000100\n0.000100\n0.000090\n0.000100\n0.000100\n0.000100\n0.000100\n0.000100\n0.000100\n0.000100\n0.000100\n0.000100\n0.000100\n0.000100\n0.000100\n0.000100\n0.000100\n0.000100\n0.000100\n0.000100\n0.000100\n0.000100\n0.000100\n0.000100\n0.000100\n0.000100\n0.000100\n0.000100\n0.000100\n0.000100\n0.000100\n0.000100\n0.000100\n0.000100\n0.000100\n0.000100\n0.000100\n0.000100\n0.000100\n0.000100\n0.000100\n0.000100\n0.000100\n0.000100\n0.000100\n0.000100\n0.000100\n0.000100\n0.000100\n0.000110\n0.000100\n0.000100\n0.000110\n0.000100\n0.000110\n0.000110\n0.000100\n0.000110\n0.000110\n0.000110\n0.000110\n0.000110\n0.000110\n0.000110\n0.000110\n0.000110\n0.000110\n0.000110\n0.000110\n0.000110\n0.000110\n0.000110\n0.000110\n0.000110\n0.000110\n0.000110\n0.000110\n0.000110\n0.000110\n0.000110\n0.000110\n0.000110\n0.000110\n0.000110\n0.000110\n0.000110\n0.000110\n0.000110\n0.000110\n0.000110\n0.000110\n0.000110\n0.000110\n0.000110\n0.000110\n0.000110\n0.000110\n0.000110\n0.000110\n0.000110\n0.000110\n0.000110\n0.000120\n0.000110\n0.000110\n0.000110\n0.000120\n0.000110\n0.000120\n0.000120\n0.000120\n0.000110\n0.000110\n0.000120\n0.000120\n0.000120\n0.000120\n0.000120\n0.000120\n0.000120\n0.000120\n0.000120\n0.000120\n0.000120\n0.000120\n0.000120\n0.000120\n0.000120\n0.000120\n0.000120\n0.000120\n0.000120\n0.000120\n0.000120\n0.000120\n0.000120\n0.000130\n0.000120\n0.000120\n0.000120\n0.000120\n0.000120\n0.000130\n0.000130\n0.000130\n0.000120\n0.000130\n0.000120\n0.000130\n0.000130\n0.000130\n0.000130\n0.000130\n0.000130\n0.000130\n0.000130\n0.000130\n0.000130\n0.000130\n0.000130\n0.000130\n0.000130\n0.000130\n0.000130\n0.000130\n0.000130\n0.000130\n0.000130\n0.000130\n0.000130\n0.000130\n0.000130\n0.000130\n0.000130\n0.000130\n0.000130\n0.000130\n0.000130\n0.000130\n0.000130\n0.000130\n0.000130\n0.000130\n0.000130\n0.000130\n0.000130\n0.000130\n0.000140\n0.000130\n0.000130\n0.000140\n0.000130\n0.000140\n0.000140\n0.000140\n0.000130\n0.000140\n0.000140\n0.000140\n0.000140\n0.000140\n0.000140\n0.000140\n0.000140\n0.000140\n0.000140\n0.000140\n0.000140\n0.000140\n0.000140\n0.000140\n0.000140\n0.000140\n0.000140\n0.000140\n0.000140\n0.000140\n0.000140\n0.000140\n0.000140\n0.000140\n0.000140\n0.000140\n0.000140\n0.000140\n0.000140\n0.000140\n0.000140\n0.000140\n0.000140\n0.000140\n0.000140\n0.000140\n0.000150\n0.000140\n0.000140\n0.000150\n0.000140\n0.000150\n0.000150\n0.000140\n0.000140\n0.000150\n0.000150\n0.000150\n0.000150\n0.000150\n0.000150\n0.000150\n0.000150\n0.000150\n0.000150\n0.000150\n0.000150\n0.000150\n0.000150\n0.000150\n0.000150\n0.000150\n0.000150\n0.000150\n0.000150\n0.000150\n0.000150\n0.000160\n0.000160\n0.000150\n0.000160\n0.000150\n0.000160\n0.000150\n0.000160\n0.000160\n0.000160\n0.000160\n0.000160\n0.000160\n0.000160\n0.000160\n0.000160\n0.000160\n0.000160\n0.000160\n0.000160\n0.000160\n0.000160\n0.000160\n0.000160\n0.000160\n0.000160\n0.000160\n0.000160\n0.000160\n0.000160\n0.000160\n0.000160\n0.000160\n0.000160\n0.000160\n0.000160\n0.000160\n0.000160\n0.000160\n0.000160\n0.000160\n0.000170\n0.000160\n0.000160\n0.000160\n0.000160\n0.000160\n0.000160\n0.000160\n0.000170\n0.000170\n0.000170\n0.000170\n0.000170\n0.000170\n0.000170\n0.000170\n0.000170\n0.000170\n0.000170\n0.000170\n0.000170\n0.000170\n0.000170\n0.000170\n0.000170\n0.000170\n0.000170\n0.000180\n0.000170\n0.000170\n0.000170\n0.000170\n0.000170\n0.000180\n0.000170\n0.000180\n0.000180\n0.000180\n0.000180\n0.000180\n0.000180\n0.000180\n0.000180\n0.000180\n0.000180\n0.000180\n0.000180\n0.000180\n0.000180\n0.000180\n0.000180\n0.000180\n0.000180\n0.000180\n0.000180\n0.000180\n0.000180\n0.000180\n0.000180\n0.000180\n0.000180\n0.000180\n0.000180\n0.000180\n0.000180\n0.000180\n0.000180\n0.000180\n0.000180\n0.000180\n0.000180\n0.000180\n0.000190\n0.000190\n0.000190\n0.000190\n0.000190\n0.000190\n0.000190\n0.000190\n0.000190\n0.000190\n0.000190\n0.000190\n0.000190\n0.000190\n0.000190\n0.000190\n0.000190\n0.000190\n0.000190\n0.000190\n0.000190\n0.000190\n0.000190\n0.000190\n0.000190\n0.000190\n0.000190\n0.000190\n0.000190\n0.000190\n0.000190\n0.000190\n0.000190\n0.000190\n0.000190\n0.000190\n0.000190\n0.000190\n0.000200\n0.000200\n0.000200\n0.000200\n0.000200\n0.000200\n0.000200\n0.000200\n0.000200\n0.000200\n0.000200\n0.000200\n0.000200\n0.000200\n0.000200\n0.000200\n0.000200\n0.000200\n0.000200\n0.000200\n0.000200\n0.000210\n0.000210\n0.000210\n0.000210\n0.000210\n0.000200\n0.000200\n0.000200\n0.000210\n0.000210\n0.000210\n0.000210\n0.000210\n0.000210\n0.000210\n0.000210\n0.000210\n0.000210\n0.000210\n0.000210\n0.000210\n0.000210\n0.000210\n0.000210\n0.000210\n0.000210\n0.000210\n0.000210\n0.000210\n0.000210\n0.000210\n0.000210\n0.000210\n0.000210\n0.000210\n0.000210\n0.000210\n0.000210\n0.000210\n0.000210\n0.000210\n0.000210\n0.000210\n0.000210\n0.000210\n0.000210\n0.000220\n0.000220\n0.000220\n0.000210\n0.000220\n0.000220\n0.000220\n0.000220\n0.000220\n0.000220\n0.000220\n0.000220\n0.000220\n0.000220\n0.000220\n0.000220\n0.000220\n0.000230\n0.000230\n0.000220\n0.000220\n0.000220\n0.000220\n0.000230\n0.000230\n0.000230\n0.000230\n0.000230\n0.000230\n0.000230\n0.000230\n0.000230\n0.000230\n0.000230\n0.000230\n0.000230\n0.000230\n0.000230\n0.000230\n0.000230\n0.000230\n0.000230\n0.000230\n0.000230\n0.000230\n0.000230\n0.000230\n0.000230\n0.000230\n0.000230\n0.000230\n0.000230\n0.000230\n0.000230\n0.000230\n0.000240\n0.000230\n0.000230\n0.000230\n0.000230\n0.000230\n0.000230\n0.000230\n0.000240\n0.000240\n0.000240\n0.000240\n0.000240\n0.000240\n0.000240\n0.000240\n0.000240\n0.000240\n0.000240\n0.000240\n0.000240\n0.000240\n0.000240\n0.000240\n0.000240\n0.000240\n0.000240\n0.000240\n0.000240\n0.000240\n0.000240\n0.000240\n0.000240\n0.000240\n0.000250\n0.000240\n0.000240\n0.000250\n0.000240\n0.000250\n0.000240\n0.000250\n0.000250\n0.000250\n0.000250\n0.000250\n0.000250\n0.000250\n0.000250\n0.000250\n0.000250\n0.000250\n0.000250\n0.000250\n0.000250\n0.000250\n0.000260\n0.000250\n0.000250\n0.000260\n0.000250\n0.000260\n0.000260\n0.000260\n0.000260\n0.000260\n0.000260\n0.000260\n0.000260\n0.000260\n0.000260\n0.000260\n0.000260\n0.000260\n0.000260\n0.000260\n0.000260\n0.000260\n0.000260\n0.000260\n0.000260\n0.000260\n0.000260\n0.000260\n0.000260\n0.000260\n0.000260\n0.000260\n0.000260\n0.000260\n0.000260\n0.000270\n0.000260\n0.000260\n0.000260\n0.000270\n0.000270\n0.000270\n0.000270\n0.000270\n0.000270\n0.000270\n0.000270\n0.000270\n0.000270\n0.000270\n0.000270\n0.000270\n0.000270\n0.000270\n0.000270\n0.000270\n0.000270\n0.000270\n0.000270\n0.000270\n0.000270\n0.000270\n0.000270\n0.000270\n0.000270\n0.000270\n0.000270\n0.000270\n0.000270\n0.000270\n0.000270\n0.000270\n0.000270\n0.000280\n0.000280\n0.000270\n0.000280\n0.000280\n0.000280\n0.000280\n0.000280\n0.000280\n0.000280\n0.000280\n0.000280\n0.000280\n0.000280\n0.000280\n0.000280\n0.000280\n0.000280\n0.000280\n0.000280\n0.000280\n0.000280\n0.000280\n0.000290\n0.000290\n0.000290\n0.000290\n0.000290\n0.000290\n0.000290\n0.000290\n0.000290\n0.000290\n0.000290\n0.000290\n0.000290\n0.000290\n0.000290\n0.000290\n0.000290\n0.000290\n0.000290\n0.000290\n0.000290\n0.000290\n0.000290\n0.000290\n0.000290\n0.000290\n0.000290\n0.000290\n0.000290\n0.000300\n0.000300\n0.000290\n0.000300\n0.000300\n0.000290\n0.000300\n0.000300\n0.000300\n0.000300\n0.000300\n0.000300\n0.000300\n0.000300\n0.000300\n0.000300\n0.000300\n0.000300\n0.000300\n0.000300\n0.000300\n0.000300\n0.000300\n0.000300\n0.000310\n0.000310\n0.000310\n0.000310\n0.000300\n0.000310\n0.000310\n0.000310\n0.000310\n0.000310\n0.000310\n0.000310\n0.000310\n0.000310\n0.000310\n0.000310\n0.000310\n0.000310\n0.000310\n0.000310\n0.000310\n0.000310\n0.000310\n0.000310\n0.000310\n0.000310\n0.000310\n0.000310\n0.000320\n0.000310\n0.000310\n0.000310\n0.000310\n0.000320\n0.000320\n0.000310\n0.000320\n0.000320\n0.000320\n0.000320\n0.000320\n0.000320\n0.000320\n0.000320\n0.000320\n0.000320\n0.000320\n0.000320\n0.000320\n0.000320\n0.000320\n0.000320\n0.000320\n0.000320\n0.000320\n0.000320\n0.000320\n0.000320\n0.000320\n0.000320\n0.000330\n0.000320\n0.000320\n0.000320\n0.000330\n0.000330\n0.000330\n0.000330\n0.000320\n0.000330\n0.000330\n0.000330\n0.000330\n0.000330\n0.000330\n0.000330\n0.000330\n0.000330\n0.000330\n0.000330\n0.000330\n0.000330\n0.000340\n0.000340\n0.000340\n0.000340\n0.000340\n0.000340\n0.000340\n0.000340\n0.000340\n0.000340\n0.000340\n0.000340\n0.000340\n0.000340\n0.000340\n0.000340\n0.000340\n0.000340\n0.000340\n0.000340\n0.000340\n0.000340\n0.000340\n0.000340\n0.000340\n0.000340\n0.000340\n0.000340\n0.000340\n0.000340\n0.000340\n0.000340\n0.000350\n0.000350\n0.000350\n0.000350\n0.000350\n0.000350\n0.000350\n0.000350\n0.000350\n0.000350\n0.000350\n0.000350\n0.000350\n0.000350\n0.000350\n0.000350\n0.000350\n0.000350\n0.000350\n0.000350\n0.000350\n0.000350\n0.000350\n0.000350\n0.000350\n0.000350\n0.000350\n0.000350\n0.000350\n0.000350\n0.000350\n0.000350\n0.000350\n0.000360\n0.000360\n0.000360\n0.000360\n0.000360\n0.000360\n0.000360\n0.000360\n0.000360\n0.000360\n0.000360\n0.000360\n0.000360\n0.000360\n0.000360\n0.000360\n0.000360\n0.000360\n0.000370\n0.000360\n0.000370\n0.000370\n0.000370\n0.000370\n0.000360\n0.000370\n0.000370\n0.000370\n0.000370\n0.000370\n0.000370\n0.000370\n0.000370\n0.000370\n0.000370\n0.000370\n0.000370\n0.000370\n0.000370\n0.000370\n0.000370\n0.000370\n0.000370\n0.000370\n0.000370\n0.000370\n0.000370\n0.000370\n0.000370\n0.000370\n0.000380\n0.000370\n0.000380\n0.000380\n0.000380\n0.000380\n0.000380\n0.000380\n0.000380\n0.000380\n0.000380\n0.000380\n0.000380\n0.000380\n0.000380\n0.000380\n0.000380\n0.000390\n0.000380\n0.000380\n0.000380\n0.000380\n0.000390\n0.000390\n0.000390\n0.000390\n0.000390\n0.000390\n0.000390\n0.000390\n0.000390\n0.000390\n0.000390\n0.000390\n0.000390\n0.000390\n0.000390\n0.000390\n0.000390\n0.000390\n0.000390\n0.000390\n0.000390\n0.000390\n0.000390\n0.000390\n0.000390\n0.000390\n0.000400\n0.000390\n0.000390\n0.000400\n0.000400\n0.000400\n0.000400\n0.000400\n0.000400\n0.000400\n0.000400\n0.000400\n0.000400\n0.000400\n0.000400\n0.000400\n0.000400\n0.000400\n0.000400\n0.000400\n0.000400\n0.000400\n0.000400\n0.000400\n0.000400\n0.000400\n0.000400\n0.000400\n0.000400\n0.000400\n0.000410\n0.000400\n0.000410\n0.000400\n0.000410\n0.000410\n0.000410\n0.000410\n0.000410\n0.000410\n0.000410\n0.000410\n0.000410\n0.000410\n0.000410\n0.000410\n0.000410\n0.000410\n0.000410\n0.000420\n0.000420\n0.000420\n0.000420\n0.000420\n0.000420\n0.000410\n0.000410\n0.000420\n0.000420\n0.000420\n0.000420\n0.000420\n0.000420\n0.000420\n0.000420\n0.000420\n0.000420\n0.000420\n0.000420\n0.000420\n0.000420\n0.000420\n0.000420\n0.000420\n0.000420\n0.000420\n0.000420\n0.000420\n0.000420\n0.000430\n0.000420\n0.000420\n0.000420\n0.000430\n0.000430\n0.000430\n0.000430\n0.000430\n0.000430\n0.000430\n0.000430\n0.000430\n0.000430\n0.000430\n0.000430\n0.000430\n0.000430\n0.000430\n0.000430\n0.000430\n0.000430\n0.000430\n0.000430\n0.000430\n0.000430\n0.000430\n0.000430\n0.000430\n0.000430\n0.000430\n0.000440\n0.000430\n0.000440\n0.000440\n0.000440\n0.000440\n0.000440\n0.000440\n0.000440\n0.000440\n0.000440\n0.000440\n0.000440\n0.000440\n0.000440\n0.000440\n0.000440\n0.000440\n0.000440\n0.000440\n0.000450\n0.000450\n0.000450\n0.000450\n0.000450\n0.000450\n0.000450\n0.000450\n0.000450\n0.000450\n0.000450\n0.000450\n0.000450\n0.000450\n0.000450\n0.000450\n0.000450\n0.000450\n0.000450\n0.000450\n0.000450\n0.000450\n0.000450\n0.000450\n0.000450\n0.000450\n0.000460\n0.000450\n0.000460\n0.000450\n0.000460\n0.000450\n0.000460\n0.000460\n0.000460\n0.000460\n0.000460\n0.000460\n0.000460\n0.000460\n0.000460\n0.000460\n0.000460\n0.000460\n0.000460\n0.000460\n0.000460\n0.000470\n0.000470\n0.000470\n0.000470\n0.000470\n0.000470\n0.000470\n0.000470\n0.000470\n0.000470\n0.000470\n0.000470\n0.000470\n0.000470\n0.000470\n0.000470\n0.000470\n0.000470\n0.000470\n0.000470\n0.000470\n0.000470\n0.000470\n0.000470\n0.000470\n0.000470\n0.000470\n0.000480\n0.000470\n0.000480\n0.000470\n0.000480\n0.000470\n0.000480\n0.000470\n0.000480\n0.000480\n0.000480\n0.000480\n0.000480\n0.000480\n0.000480\n0.000480\n0.000480\n0.000480\n0.000480\n0.000480\n0.000480\n0.000480\n0.000480\n0.000480\n0.000480\n0.000480\n0.000480\n0.000480\n0.000480\n0.000480\n0.000480\n0.000490\n0.000490\n0.000490\n0.000490\n0.000480\n0.000490\n0.000490\n0.000490\n0.000490\n0.000490\n0.000490\n0.000490\n0.000490\n0.000490\n0.000490\n0.000490\n0.000500\n0.000490\n0.000490\n0.000500\n0.000490\n0.000500\n0.000500\n0.000500\n0.000500\n0.000500\n0.000500\n0.000500\n0.000500\n0.000500\n0.000500\n0.000500\n0.000500\n0.000500\n0.000500\n0.000500\n0.000500\n0.000500\n0.000500\n0.000500\n0.000500\n0.000500\n0.000500\n0.000500\n0.000500\n0.000500\n0.000500\n0.000510\n0.000510\n0.000510\n0.000510\n0.000510\n0.000510\n0.000510\n0.000510\n0.000510\n0.000510\n0.000510\n0.000510\n0.000510\n0.000510\n0.000510\n0.000510\n0.000510\n0.000510\n0.000510\n0.000510\n0.000510\n0.000510\n0.000510\n0.000510\n0.000510\n0.000520\n0.000510\n0.000510\n0.000520\n0.000520\n0.000510\n0.000520\n0.000520\n0.000520\n0.000520\n0.000520\n0.000520\n0.000520\n0.000520\n0.000520\n0.000520\n0.000520\n0.000520\n0.000520\n0.000520\n0.000530\n0.000520\n0.000520\n0.000530\n0.000530\n0.000530\n0.000530\n0.000530\n0.000530\n0.000530\n0.000530\n0.000530\n0.000530\n0.000530\n0.000530\n0.000530\n0.000530\n0.000530\n0.000530\n0.000530\n0.000530\n0.000530\n0.000530\n0.000530\n0.000540\n0.000540\n0.000540\n0.000540\n0.000540\n0.000540\n0.000540\n0.000540\n0.000540\n0.000540\n0.000540\n0.000540\n0.000540\n0.000540\n0.000540\n0.000540\n0.000540\n0.000540\n0.000540\n0.000540\n0.000540\n0.000550\n0.000540\n0.000550\n0.000550\n0.000540\n0.000550\n0.000550\n0.000550\n0.000550\n0.000550\n0.000550\n0.000550\n0.000550\n0.000550\n0.000550\n0.000550\n0.000550\n0.000550\n0.000550\n0.000550\n0.000550\n0.000550\n0.000550\n0.000550\n0.000560\n0.000550\n0.000550\n0.000560\n0.000550\n0.000550\n0.000560\n0.000560\n0.000560\n0.000560\n0.000560\n0.000560\n0.000560\n0.000560\n0.000560\n0.000560\n0.000560\n0.000560\n0.000560\n0.000560\n0.000560\n0.000560\n0.000560\n0.000560\n0.000560\n0.000560\n0.000560\n0.000560\n0.000560\n0.000570\n0.000570\n0.000570\n0.000570\n0.000570\n0.000570\n0.000570\n0.000570\n0.000570\n0.000570\n0.000570\n0.000570\n0.000570\n0.000570\n0.000570\n0.000570\n0.000580\n0.000580\n0.000570\n0.000570\n0.000580\n0.000580\n0.000580\n0.000580\n0.000580\n0.000580\n0.000580\n0.000580\n0.000580\n0.000580\n0.000580\n0.000580\n0.000580\n0.000580\n0.000580\n0.000580\n0.000580\n0.000580\n0.000580\n0.000580\n0.000580\n0.000590\n0.000580\n0.000590\n0.000580\n0.000590\n0.000590\n0.000590\n0.000590\n0.000590\n0.000590\n0.000590\n0.000590\n0.000590\n0.000590\n0.000590\n0.000590\n0.000590\n0.000590\n0.000590\n0.000600\n0.000600\n0.000590\n0.000600\n0.000600\n0.000600\n0.000600\n0.000600\n0.000600\n0.000600\n0.000600\n0.000600\n0.000600\n0.000600\n0.000600\n0.000600\n0.000600\n0.000600\n0.000600\n0.000600\n0.000600\n0.000600\n0.000600\n0.000600\n0.000600\n0.000600\n0.000600\n0.000610\n0.000610\n0.000610\n0.000610\n0.000610\n0.000610\n0.000610\n0.000610\n0.000610\n0.000610\n0.000610\n0.000610\n0.000610\n0.000610\n0.000610\n0.000610\n0.000610\n0.000610\n0.000610\n0.000610\n0.000610\n0.000620\n0.000620\n0.000610\n0.000620\n0.000620\n0.000620\n0.000620\n0.000620\n0.000620\n0.000620\n0.000620\n0.000620\n0.000620\n0.000620\n0.000620\n0.000620\n0.000630\n0.000620\n0.000630\n0.000630\n0.000630\n0.000630\n0.000630\n0.000630\n0.000630\n0.000630\n0.000630\n0.000630\n0.000630\n0.000630\n0.000630\n0.000630\n0.000630\n0.000630\n0.000630\n0.000630\n0.000630\n0.000630\n0.000630\n0.000640\n0.000630\n0.000640\n0.000640\n0.000640\n0.000640\n0.000640\n0.000640\n0.000640\n0.000640\n0.000640\n0.000640\n0.000640\n0.000640\n0.000640\n0.000640\n0.000640\n0.000640\n0.000640\n0.000640\n0.000640\n0.000640\n0.000640\n0.000650\n0.000650\n0.000650\n0.000640\n0.000650\n0.000650\n0.000650\n0.000650\n0.000650\n0.000650\n0.000650\n0.000650\n0.000650\n0.000650\n0.000650\n0.000650\n0.000650\n0.000650\n0.000660\n0.000660\n0.000660\n0.000660\n0.000660\n0.000660\n0.000660\n0.000660\n0.000660\n0.000660\n0.000660\n0.000660\n0.000660\n0.000660\n0.000660\n0.000660\n0.000660\n0.000660\n0.000660\n0.000660\n0.000660\n0.000660\n0.000660\n0.000670\n0.000670\n0.000670\n0.000670\n0.000670\n0.000670\n0.000670\n0.000670\n0.000670\n0.000670\n0.000670\n0.000670\n0.000680\n0.000680\n0.000680\n0.000680\n0.000680\n0.000680\n0.000680\n0.000680\n0.000680\n0.000680\n0.000680\n0.000680\n0.000680\n0.000680\n0.000680\n0.000680\n0.000680\n0.000680\n0.000680\n0.000680\n0.000680\n0.000680\n0.000690\n0.000690\n0.000690\n0.000690\n0.000690\n0.000690\n0.000690\n0.000690\n0.000690\n0.000690\n0.000690\n0.000690\n0.000690\n0.000690\n0.000690\n0.000690\n0.000690\n0.000690\n0.000700\n0.000690\n0.000700\n0.000700\n0.000700\n0.000700\n0.000700\n0.000700\n0.000700\n0.000700\n0.000700\n0.000700\n0.000700\n0.000700\n0.000700\n0.000710\n0.000700\n0.000710\n0.000710\n0.000710\n0.000710\n0.000710\n0.000710\n0.000710\n0.000710\n0.000710\n0.000710\n0.000710\n0.000710\n0.000710\n0.000710\n0.000710\n0.000710\n0.000720\n0.000710\n0.000720\n0.000710\n0.000720\n0.000720\n0.000720\n0.000720\n0.000720\n0.000720\n0.000720\n0.000720\n0.000720\n0.000720\n0.000720\n0.000720\n0.000720\n0.000720\n0.000720\n0.000720\n0.000720\n0.000730\n0.000720\n0.000730\n0.000730\n0.000730\n0.000730\n0.000730\n0.000730\n0.000730\n0.000730\n0.000740\n0.000730\n0.000740\n0.000740\n0.000730\n0.000740\n0.000740\n0.000740\n0.000740\n0.000740\n0.000740\n0.000740\n0.000740\n0.000740\n0.000740\n0.000740\n0.000740\n0.000740\n0.000740\n0.000740\n0.000740\n0.000750\n0.000740\n0.000750\n0.000750\n0.000750\n0.000750\n0.000750\n0.000750\n0.000750\n0.000750\n0.000750\n0.000750\n0.000760\n0.000760\n0.000750\n0.000760\n0.000760\n0.000760\n0.000760\n0.000760\n0.000760\n0.000760\n0.000760\n0.000760\n0.000760\n0.000760\n0.000760\n0.000760\n0.000760\n0.000760\n0.000770\n0.000770\n0.000770\n0.000770\n0.000770\n0.000770\n0.000770\n0.000770\n0.000770\n0.000770\n0.000770\n0.000770\n0.000770\n0.000770\n0.000770\n0.000770\n0.000770\n0.000780\n0.000780\n0.000770\n0.000780\n0.000780\n0.000780\n0.000780\n0.000780\n0.000780\n0.000780\n0.000780\n0.000780\n0.000790\n0.000790\n0.000780\n0.000790\n0.000790\n0.000790\n0.000790\n0.000790\n0.000790\n0.000790\n0.000790\n0.000790\n0.000790\n0.000790\n0.000790\n0.000790\n0.000790\n0.000800\n0.000800\n0.000800\n0.000800\n0.000800\n0.000800\n0.000800\n0.000800\n0.000800\n0.000800\n0.000800\n0.000800\n0.000800\n0.000800\n0.000810\n0.000810\n0.000800\n0.000810\n0.000810\n0.000810\n0.000810\n0.000810\n0.000810\n0.000810\n0.000810\n0.000810\n0.000820\n0.000810\n0.000820\n0.000820\n0.000820\n0.000820\n0.000820\n0.000820\n0.000820\n0.000820\n0.000820\n0.000820\n0.000820\n0.000820\n0.000820\n0.000820\n0.000830\n0.000830\n0.000830\n0.000830\n0.000830\n0.000830\n0.000830\n0.000830\n0.000830\n0.000830\n0.000840\n0.000840\n0.000840\n0.000840\n0.000840\n0.000840\n0.000840\n0.000840\n0.000840\n0.000840\n0.000840\n0.000840\n0.000840\n0.000840\n0.000850\n0.000850\n0.000850\n0.000850\n0.000850\n0.000850\n0.000850\n0.000850\n0.000850\n0.000850\n0.000850\n0.000850\n0.000850\n0.000850\n0.000850\n0.000850\n0.000860\n0.000850\n0.000860\n0.000860\n0.000860\n0.000860\n0.000860\n0.000860\n0.000870\n0.000860\n0.000870\n0.000870\n0.000870\n0.000870\n0.000870\n0.000870\n0.000870\n0.000870\n0.000870\n0.000870\n0.000870\n0.000870\n0.000870\n0.000880\n0.000870\n0.000880\n0.000880\n0.000880\n0.000880\n0.000880\n0.000880\n0.000880\n0.000890\n0.000880\n0.000890\n0.000890\n0.000890\n0.000890\n0.000890\n0.000890\n0.000890\n0.000890\n0.000890\n0.000890\n0.000890\n0.000900\n0.000900\n0.000900\n0.000900\n0.000900\n0.000900\n0.000900\n0.000900\n0.000900\n0.000900\n0.000900\n0.000900\n0.000900\n0.000910\n0.000900\n0.000910\n0.000910\n0.000910\n0.000910\n0.000910\n0.000910\n0.000910\n0.000910\n0.000920\n0.000920\n0.000920\n0.000920\n0.000920\n0.000920\n0.000920\n0.000920\n0.000920\n0.000920\n0.000920\n0.000930\n0.000920\n0.000930\n0.000930\n0.000930\n0.000930\n0.000930\n0.000930\n0.000930\n0.000930\n0.000930\n0.000930\n0.000940\n0.000940\n0.000930\n0.000940\n0.000940\n0.000940\n0.000940\n0.000940\n0.000940\n0.000950\n0.000950\n0.000950\n0.000950\n0.000950\n0.000950\n0.000950\n0.000950\n0.000950\n0.000950\n0.000950\n0.000960\n0.000960\n0.000960\n0.000960\n0.000960\n0.000960\n0.000960\n0.000960\n0.000960\n0.000970\n0.000970\n0.000970\n0.000970\n0.000970\n0.000970\n0.000970\n0.000970\n0.000970\n0.000970\n0.000970\n0.000970\n0.000970\n0.000970\n0.000980\n0.000980\n0.000980\n0.000980\n0.000980\n0.000980\n0.000980\n0.000980\n0.000980\n0.000980\n0.000990\n0.000990\n0.000990\n0.000990\n0.000990\n0.000990\n0.000990\n0.001000\n0.001000\n0.001000\n0.001000\n0.001000\n0.001000\n0.001000\n0.001000\n0.001000\n0.001010\n0.001000\n0.001000\n0.001010\n0.001010\n0.001010\n0.001010\n0.001010\n0.001010\n0.001010\n0.001010\n0.001010\n0.001020\n0.001020\n0.001020\n0.001020\n0.001020\n0.001020\n0.001030\n0.001020\n0.001030\n0.001030\n0.001030\n0.001030\n0.001030\n0.001030\n0.001030\n0.001030\n0.001040\n0.001030\n0.001040\n0.001040\n0.001040\n0.001040\n0.001050\n0.001040\n0.001050\n0.001050\n0.001050\n0.001050\n0.001050\n0.001050\n0.001050\n0.001050\n0.001050\n0.001060\n0.001050\n0.001060\n0.001060\n0.001060\n0.001060\n0.001060\n0.001060\n0.001060\n0.001060\n0.001060\n0.001070\n0.001070\n0.001070\n0.001070\n0.001070\n0.001070\n0.001070\n0.001070\n0.001080\n0.001080\n0.001080\n0.001080\n0.001080\n0.001080\n0.001080\n0.001090\n0.001090\n0.001090\n0.001090\n0.001090\n0.001090\n0.001090\n0.001090\n0.001090\n0.001090\n0.001100\n0.001100\n0.001100\n0.001100\n0.001100\n0.001110\n0.001110\n0.001110\n0.001110\n0.001110\n0.001110\n0.001110\n0.001110\n0.001110\n0.001110\n0.001110\n0.001120\n0.001120\n0.001120\n0.001120\n0.001120\n0.001130\n0.001130\n0.001130\n0.001130\n0.001130\n0.001130\n0.001130\n0.001130\n0.001130\n0.001140\n0.001140\n0.001140\n0.001140\n0.001140\n0.001140\n0.001140\n0.001140\n0.001140\n0.001150\n0.001150\n0.001150\n0.001150\n0.001160\n0.001150\n0.001160\n0.001160\n0.001160\n0.001160\n0.001160\n0.001160\n0.001160\n0.001160\n0.001170\n0.001170\n0.001170\n0.001170\n0.001170\n0.001170\n0.001170\n0.001170\n0.001180\n0.001180\n0.001180\n0.001180\n0.001180\n0.001190\n0.001190\n0.001190\n0.001190\n0.001190\n0.001190\n0.001190\n0.001190\n0.001190\n0.001200\n0.001200\n0.001200\n0.001200\n0.001210\n0.001210\n0.001210\n0.001210\n0.001210\n0.001210\n0.001210\n0.001210\n0.001210\n0.001220\n0.001220\n0.001220\n0.001220\n0.001220\n0.001220\n0.001220\n0.001220\n0.001230\n0.001230\n0.001230\n0.001230\n0.001230\n0.001240\n0.001240\n0.001240\n0.001240\n0.001240\n0.001240\n0.001240\n0.001250\n0.001250\n0.001250\n0.001250\n0.001250\n0.001260\n0.001260\n0.001260\n0.001260\n0.001260\n0.001260\n0.001260\n0.001270\n0.001260\n0.001270\n0.001270\n0.001270\n0.001270\n0.001270\n0.001280\n0.001270\n0.001280\n0.001280\n0.001280\n0.001280\n0.001290\n0.001290\n0.001290\n0.001290\n0.001290\n0.001290\n0.001290\n0.001290\n0.001300\n0.001300\n0.001300\n0.001300\n0.001300\n0.001300\n0.001300\n0.001310\n0.001310\n0.001310\n0.001310\n0.001320\n0.001320\n0.001320\n0.001320\n0.001320\n0.001320\n0.001330\n0.001330\n0.001330\n0.001330\n0.001330\n0.001340\n0.001340\n0.001340\n0.001340\n0.001340\n0.001340\n0.001340\n0.001350\n0.001350\n0.001350\n0.001350\n0.001350\n0.001350\n0.001360\n0.001360\n0.001360\n0.001360\n0.001360\n0.001370\n0.001370\n0.001370\n0.001370\n0.001370\n0.001370\n0.001370\n0.001380\n0.001380\n0.001380\n0.001380\n0.001380\n0.001380\n0.001390\n0.001390\n0.001390\n0.001390\n0.001390\n0.001400\n0.001400\n0.001400\n0.001400\n0.001400\n0.001400\n0.001410\n0.001410\n0.001410\n0.001410\n0.001420\n0.001420\n0.001420\n0.001420\n0.001420\n0.001420\n0.001430\n0.001430\n0.001430\n0.001430\n0.001430\n0.001430\n0.001440\n0.001440\n0.001440\n0.001440\n0.001450\n0.001450\n0.001450\n0.001450\n0.001450\n0.001450\n0.001460\n0.001460\n0.001460\n0.001460\n0.001460\n0.001460\n0.001470\n0.001470\n0.001470\n0.001480\n0.001480\n0.001480\n0.001480\n0.001490\n0.001490\n0.001490\n0.001500\n0.001500\n0.001510\n0.001510\n0.001510\n0.001510\n0.001510\n0.001510\n0.001520\n0.001520\n0.001520\n0.001520\n0.001520\n0.001520\n0.001520\n0.001530\n0.001530\n0.001540\n0.001540\n0.001540\n0.001540\n0.001540\n0.001540\n0.001540\n0.001550\n0.001550\n0.001550\n0.001550\n0.001550\n0.001560\n0.001560\n0.001560\n0.001560\n0.001570\n0.001570\n0.001570\n0.001570\n0.001570\n0.001580\n0.001580\n0.001580\n0.001590\n0.001590\n0.001590\n0.001590\n0.001590\n0.001600\n0.001600\n0.001600\n0.001600\n0.001600\n0.001600\n0.001610\n0.001610\n0.001610\n0.001620\n0.001620\n0.001620\n0.001620\n0.001620\n0.001620\n0.001630\n0.001630\n0.001640\n0.001640\n0.001640\n0.001640\n0.001640\n0.001640\n0.001650\n0.001650\n0.001650\n0.001650\n0.001650\n0.001660\n0.001660\n0.001660\n0.001670\n0.001670\n0.001670\n0.001670\n0.001670\n0.001680\n0.001680\n0.001680\n0.001680\n0.001680\n0.001690\n0.001690\n0.001690\n0.001700\n0.001700\n0.001700\n0.001700\n0.001700\n0.001700\n0.001710\n0.001710\n0.001720\n0.001720\n0.001720\n0.001720\n0.001720\n0.001730\n0.001730\n0.001730\n0.001730\n0.001730\n0.001740\n0.001740\n0.001740\n0.001740\n0.001750\n0.001750\n0.001750\n0.001760\n0.001760\n0.001760\n0.001760\n0.001760\n0.001770\n0.001770\n0.001780\n0.001780\n0.001780\n0.001780\n0.001780\n0.001780\n0.001790\n0.001790\n0.001790\n0.001800\n0.001800\n0.001800\n0.001800\n0.001810\n0.001810\n0.001810\n0.001810\n0.001820\n0.001820\n0.001820\n0.001830\n0.001830\n0.001830\n0.001830\n0.001840\n0.001840\n0.001840\n0.001840\n0.001840\n0.001850\n0.001850\n0.001860\n0.001860\n0.001860\n0.001860\n0.001860\n0.001870\n0.001870\n0.001870\n0.001870\n0.001880\n0.001880\n0.001880\n0.001880\n0.001890\n0.001890\n0.001890\n0.001890\n0.001900\n0.001900\n0.001910\n0.001910\n0.001910\n0.001910\n0.001920\n0.001920\n0.001920\n0.001920\n0.001920\n0.001930\n0.001930\n0.001930\n0.001940\n0.001940\n0.001940\n0.001950\n0.001950\n0.001950\n0.001950\n0.001960\n0.001960\n0.001960\n0.001960\n0.001970\n0.001970\n0.001970\n0.001980\n0.001980\n0.001990\n0.001990\n0.001990\n0.001990\n0.002000\n0.002000\n0.002000\n0.002010\n0.002010\n0.002010\n0.002010\n0.002020\n0.002020\n0.002020\n0.002020\n0.002030\n0.002030\n0.002030\n0.002040\n0.002040\n0.002040\n0.002040\n0.002050\n0.002050\n0.002050\n0.002060\n0.002060\n0.002060\n0.002070\n0.002070\n0.002070\n0.002080\n0.002080\n0.002080\n0.002090\n0.002090\n0.002090\n0.002090\n0.002100\n0.002100\n0.002100\n0.002110\n0.002120\n0.002110\n0.002120\n0.002120\n0.002120\n0.002130\n0.002130\n0.002130\n0.002140\n0.002140\n0.002140\n0.002150\n0.002150\n0.002150\n0.002150\n0.002160\n0.002160\n0.002170\n0.002170\n0.002170\n0.002170\n0.002180\n0.002180\n0.002180\n0.002190\n0.002190\n0.002200\n0.002200\n0.002200\n0.002210\n0.002210\n0.002210\n0.002210\n0.002220\n0.002230\n0.002220\n0.002230\n0.002230\n0.002230\n0.002240\n0.002240\n0.002250\n0.002250\n0.002250\n0.002250\n0.002260\n0.002260\n0.002260\n0.002270\n0.002270\n0.002270\n0.002280\n0.002280\n0.002290\n0.002290\n0.002290\n0.002300\n0.002300\n0.002300\n0.002310\n0.002310\n0.002310\n0.002310\n0.002320\n0.002330\n0.002330\n0.002330\n0.002340\n0.002340\n0.002340\n0.002340\n0.002350\n0.002350\n0.002360\n0.002360\n0.002360\n0.002370\n0.002370\n0.002370\n0.002380\n0.002390\n0.002390\n0.002390\n0.002390\n0.002390\n0.002400\n0.002400\n0.002410\n0.002410\n0.002410\n0.002420\n0.002420\n0.002430\n0.002430\n0.002430\n0.002440\n0.002440\n0.002440\n0.002450\n0.002450\n0.002460\n0.002460\n0.002460\n0.002470\n0.002470\n0.002470\n0.002480\n0.002480\n0.002490\n0.002490\n0.002490\n0.002500\n0.002500\n0.002500\n0.002510\n0.002510\n0.002520\n0.002520\n0.002530\n0.002530\n0.002530\n0.002540\n0.002540\n0.002550\n0.002550\n0.002550\n0.002560\n0.002560\n0.002570\n0.002570\n0.002570\n0.002570\n0.002580\n0.002580\n0.002580\n0.002600\n0.002600\n0.002600\n0.002600\n0.002610\n0.002610\n0.002620\n0.002620\n0.002630\n0.002630\n0.002630\n0.002630\n0.002640\n0.002640\n0.002650\n0.002650\n0.002650\n0.002660\n0.002670\n0.002670\n0.002680\n0.002680\n0.002680\n0.002680\n0.002690\n0.002700\n0.002700\n0.002700\n0.002710\n0.002710\n0.002710\n0.002720\n0.002720\n0.002730\n0.002730\n0.002730\n0.002740\n0.002750\n0.002750\n0.002750\n0.002760\n0.002760\n0.002760\n0.002770\n0.002780\n0.002780\n0.002780\n0.002790\n0.002790\n0.002790\n0.002810\n0.002800\n0.002810\n0.002820\n0.002820\n0.002820\n0.002830\n0.002830\n0.002840\n0.002840\n0.002850\n0.002850\n0.002860\n0.002860\n0.002860\n0.002870\n0.002870\n0.002880\n0.002880\n0.002880\n0.002890\n0.002890\n0.002900\n0.002900\n0.002910\n0.002910\n0.002920\n0.002920\n0.002920\n0.002940\n0.002930\n0.002940\n0.002940\n0.002950\n0.002950\n0.002960\n0.002960\n0.002970\n0.002970\n0.002970\n0.002980\n0.002990\n0.002990\n0.002990\n0.003000\n0.003000\n0.003010\n0.003020\n0.003020\n0.003020\n0.003030\n0.003030\n0.003040\n0.003040\n0.003050\n0.003050\n0.003060\n0.003070\n0.003070\n0.003070\n0.003070\n0.003080\n0.003090\n0.003100\n0.003100\n0.003100\n0.003100\n0.003120\n0.003120\n0.003120\n0.003130\n0.003130\n0.003140\n0.003140\n0.003150\n0.003150\n0.003150\n0.003160\n0.003160\n0.003170\n0.003170\n0.003180\n0.003180\n0.003190\n0.003200\n0.003200\n0.003200\n0.003210\n0.003210\n0.003230\n0.003230\n0.003230\n0.003240\n0.003240\n0.003240\n0.003250\n0.003250\n0.003260\n0.003270\n0.003270\n0.003280\n0.003290\n0.003280\n0.003290\n0.003290\n0.003300\n0.003310\n0.003310\n0.003320\n0.003320\n0.003330\n0.003330\n0.003340\n0.003340\n0.003350\n0.003360\n0.003360\n0.003360\n0.003370\n0.003370\n0.003380\n0.003390\n0.003390\n0.003400\n0.003410\n0.003410\n0.003410\n0.003420\n0.003420\n0.003430\n0.003440\n0.003440\n0.003440\n0.003450\n0.003460\n0.003460\n0.003470\n0.003470\n0.003480\n0.003480\n0.003490\n0.003490\n0.003500\n0.003510\n0.003510\n0.003520\n0.003520\n0.003530\n0.003530\n0.003540\n0.003550\n0.003550\n0.003560\n0.003560\n0.003570\n0.003570\n0.003580\n0.003580\n0.003590\n0.003600\n0.003600\n0.003610\n0.003610\n0.003620\n0.003630\n0.003630\n0.003640\n0.003640\n0.003650\n0.003660\n0.003660\n0.003660\n0.003670\n0.003680\n0.003680\n0.003690\n0.003700\n0.003700\n0.003710\n0.003710\n0.003720\n0.003730\n0.003730\n0.003740\n0.003750\n0.003750\n0.003760\n0.003770\n0.003780\n0.003790\n0.003790\n0.003790\n0.003800\n0.003810\n0.003810\n0.003820\n0.003820\n0.003830\n0.003840\n0.003840\n0.003850\n0.003850\n0.003860\n0.003870\n0.003870\n0.003880\n0.003890\n0.003890\n0.003900\n0.003900\n0.003910\n0.003910\n0.003920\n0.003930\n0.003930\n0.003940\n0.003950\n0.003950\n0.003960\n0.003970\n0.003970\n0.003980\n0.003990\n0.003990\n0.003990\n0.004010\n0.004010\n0.004020\n0.004030\n0.004030\n0.004040\n0.004040\n0.004050\n0.004060\n0.004060\n0.004070\n0.004080\n0.004080\n0.004080\n0.004090\n0.004100\n0.004110\n0.004110\n0.004120\n0.004130\n0.004130\n0.004140\n0.004150\n0.004150\n0.004160\n0.004170\n0.004170\n0.004180\n0.004190\n0.004190\n0.004200\n0.004200\n0.004210\n0.004220\n0.004230\n0.004230\n0.004240\n0.004250\n0.004250\n0.004260\n0.004270\n0.004270\n0.004280\n0.004280\n0.004290\n0.004300\n0.004300\n0.004310\n0.004320\n0.004330\n0.004330\n0.004340\n0.004350\n0.004360\n0.004360\n0.004370\n0.004380\n0.004380\n0.004390\n0.004400\n0.004410\n0.004410\n0.004420\n0.004430\n0.004430\n0.004430\n0.004440\n0.004450\n0.004460\n0.004470\n0.004470\n0.004480\n0.004490\n0.004490\n0.004500\n0.004510\n0.004520\n0.004520\n0.004530\n0.004540\n0.004540\n0.004560\n0.004560\n0.004560\n0.004570\n0.004580\n0.004590\n0.004600\n0.004610\n0.004610\n0.004610\n0.004620\n0.004640\n0.004640\n0.004640\n0.004650\n0.004660\n0.004670\n0.004670\n0.004690\n0.004690\n0.004700\n0.004700\n0.004710\n0.004720\n0.004720\n0.004730\n0.004740\n0.004750\n0.004760\n0.004770\n0.004770\n0.004780\n0.004790\n0.004790\n0.004800\n0.004810\n0.004820\n0.004830\n0.004840\n0.004840\n0.004850\n0.004850\n0.004860\n0.004870\n0.004880\n0.004880\n0.004900\n0.004900\n0.004910\n0.004920\n0.004930\n0.004930\n0.004940\n0.004950\n0.004950\n0.004970\n0.004980\n0.004980\n0.004980\n0.004990\n0.005000\n0.005010\n0.005020\n0.005020\n0.005040\n0.005040\n0.005050\n0.005060\n0.005070\n0.005080\n0.005090\n0.005090\n0.005100\n0.005110\n0.005120\n0.005120\n0.005140\n0.005140\n0.005150\n0.005160\n0.005170\n0.005170\n0.005180\n0.005190\n0.005200\n0.005200\n0.005220\n0.005220\n0.005230\n0.005240\n0.005240\n0.005260\n0.005270\n0.005270\n0.005280\n0.005290\n0.005300\n0.005310\n0.005310\n0.005320\n0.005330\n0.005340\n0.005340\n0.005360\n0.005360\n0.005370\n0.005380\n0.005390\n0.005400\n0.005410\n0.005410\n0.005420\n0.005430\n0.005440\n0.005450\n0.005460\n0.005470\n0.005470\n0.005480\n0.005490\n0.005500\n0.005510\n0.005520\n0.005520\n0.005540\n0.005540\n0.005560\n0.005560\n0.005570\n0.005580\n0.005590\n0.005600\n0.005600\n0.005610\n0.005620\n0.005630\n0.005640\n0.005650\n0.005660\n0.005670\n0.005680\n0.005680\n0.005690\n0.005700\n0.005710\n0.005720\n0.005730\n0.005740\n0.005740\n0.005750\n0.005760\n0.005770\n0.005780\n0.005790\n0.005800\n0.005810\n0.005820\n0.005830\n0.005830\n0.005850\n0.005860\n0.005860\n0.005880\n0.005880\n0.005890\n0.005900\n0.005910\n0.005920\n0.005930\n0.005940\n0.005950\n0.005960\n0.005960\n0.005970\n0.005990\n0.005990\n0.006010\n0.006010\n0.006020\n0.006030\n0.006040\n0.006050\n0.006060\n0.006070\n0.006080\n0.006090\n0.006100\n0.006110\n0.006120\n0.006130\n0.006130\n0.006150\n0.006160\n0.006170\n0.006180\n0.006180\n0.006190\n0.006200\n0.006210\n0.006220\n0.006230\n0.006240\n0.006250\n0.006260\n0.006270\n0.006280\n0.006290\n0.006300\n0.006310\n0.006320\n0.006330\n0.006340\n0.006360\n0.006370\n0.006380\n0.006390\n0.006400\n0.006410\n0.006420\n0.006430\n0.006440\n0.006450\n0.006460\n0.006470\n0.006480\n0.006480\n0.006500\n0.006510\n0.006520\n0.006530\n0.006540\n0.006550\n0.006560\n0.006570\n0.006580\n0.006590\n0.006600\n0.006610\n0.006630\n0.006630\n0.006640\n0.006660\n0.006660\n0.006670\n0.006680\n0.006690\n0.006700\n0.006710\n0.006720\n0.006740\n0.006740\n0.006750\n0.006760\n0.006770\n0.006790\n0.006800\n0.006800\n0.006820\n0.006820\n0.006840\n0.006850\n0.006860\n0.006870\n0.006880\n0.006890\n0.006900\n0.006910\n0.006920\n0.006930\n0.006940\n0.006950\n0.006970\n0.006970\n0.006990\n0.007000\n0.007010\n0.007020\n0.007030\n0.007050\n0.007050\n0.007060\n0.007080\n0.007090\n0.007100\n0.007110\n0.007120\n0.007130\n0.007140\n0.007150\n0.007160\n0.007170\n0.007180\n0.007200\n0.007200\n0.007210\n0.007230\n0.007240\n0.007250\n0.007260\n0.007270\n0.007280\n0.007300\n0.007310\n0.007320\n0.007320\n0.007340\n0.007350\n0.007360\n0.007380\n0.007380\n0.007390\n0.007410\n0.007420\n0.007430\n0.007440\n0.007450\n0.007460\n0.007470\n0.007490\n0.007500\n0.007510\n0.007520\n0.007540\n0.007540\n0.007550\n0.007560\n0.007580\n0.007590\n0.007610\n0.007610\n0.007620\n0.007640\n0.007650\n0.007660\n0.007670\n0.007680\n0.007700\n0.007710\n0.007720\n0.007730\n0.007740\n0.007750\n0.007770\n0.007780\n0.007790\n0.007800\n0.007820\n0.007820\n0.007830\n0.007850\n0.007870\n0.007870\n0.007880\n0.007900\n0.007910\n0.007920\n0.007930\n0.007950\n0.007950\n0.007970\n0.007980\n0.007990\n0.008010\n0.008010\n0.008030\n0.008040\n0.008050\n0.008060\n0.008080\n0.008090\n0.008100\n0.008110\n0.008130\n0.008140\n0.008160\n0.008160\n0.008180\n0.008190\n0.008200\n0.008220\n0.008230\n0.008240\n0.008250\n0.008270\n0.008280\n0.008290\n0.008300\n0.008310\n0.008330\n0.008340\n0.008350\n0.008360\n0.008380\n0.008390\n0.008400\n0.008410\n0.008430\n0.008440\n0.008450\n0.008460\n0.008480\n0.008490\n0.008510\n0.008510\n0.008530\n0.008540\n0.008550\n0.008570\n0.008580\n0.008600\n0.008610\n0.008620\n0.008640\n0.008650\n0.008660\n0.008670\n0.008690\n0.008700\n0.008710\n0.008720\n0.008740\n0.008750\n0.008770\n0.008780\n0.008790\n0.008800\n0.008820\n0.008830\n0.008850\n0.008860\n0.008870\n0.008880\n0.008900\n0.008910\n0.008930\n0.008940\n0.008950\n0.008960\n0.008980\n0.008990\n0.009000\n0.009020\n0.009030\n0.009040\n0.009060\n0.009070\n0.009090\n0.009100\n0.009110\n0.009130\n0.009140\n0.009160\n0.009170\n0.009190\n0.009210\n0.009220\n0.009230\n0.009240\n0.009260\n0.009280\n0.009290\n0.009300\n0.009320\n0.009330\n0.009350\n0.009360\n0.009370\n0.009390\n0.009400\n0.009420\n0.009430\n0.009440\n0.009450\n0.009470\n0.009490\n0.009500\n0.009510\n0.009520\n0.009530\n0.009560\n0.009570\n0.009580\n0.009590\n0.009610\n0.009630\n0.009630\n0.009650\n0.009660\n0.009680\n0.009690\n0.009710\n0.009720\n0.009740\n0.009760\n0.009760\n0.009780\n0.009800\n0.009810\n0.009820\n0.009840\n0.009850\n0.009870\n0.009890\n0.009900\n0.009910\n0.009930\n0.009940\n0.009960\n0.009970\n0.009980\n0.010000\n0.010020\n0.010030\n0.010050\n0.010060\n0.010070\n0.010090\n0.010110\n0.010120\n0.010140\n0.010150\n0.010160\n0.010180\n0.010200\n0.010210\n0.010230\n0.010240\n0.010250\n0.010270\n0.010290\n0.010300\n0.010320\n0.010330\n0.010340\n0.010360\n0.010380\n0.010390\n0.010410\n0.010420\n0.010440\n0.010450\n0.010470\n0.010480\n0.010500\n0.010510\n0.010530\n0.010550\n0.010560\n0.010580\n0.010590\n0.010610\n0.010630\n0.010640\n0.010650\n0.010670\n0.010680\n0.010700\n0.010710\n0.010730\n0.010750\n0.010760\n0.010780\n0.010790\n0.010810\n0.010830\n0.010840\n0.010860\n0.010870\n0.010890\n0.010900\n0.010920\n0.010940\n0.010950\n0.010970\n0.010990\n0.011000\n0.011020\n0.011030\n0.011050\n0.011070\n0.011080\n0.011100\n0.011110\n0.011130\n0.011140\n0.011160\n0.011180\n0.011190\n0.011210\n0.011220\n0.011240\n0.011260\n0.011280\n0.011290\n0.011310\n0.011320\n0.011340\n0.011360\n0.011380\n0.011390\n0.011410\n0.011430\n0.011440\n0.011460\n0.011470\n0.011490\n0.011510\n0.011530\n0.011540\n0.011560\n0.011570\n0.011590\n0.011610\n0.011630\n0.011640\n0.011660\n0.011670\n0.011690\n0.011710\n0.011720\n0.011740\n0.011760\n0.011780\n0.011800\n0.011810\n0.011830\n0.011850\n0.011870\n0.011880\n0.011900\n0.011910\n0.011930\n0.011950\n0.011970\n0.011980\n0.012000\n0.012020\n0.012030\n0.012050\n0.012070\n0.012090\n0.012100\n0.012120\n0.012140\n0.012170\n0.012180\n0.012200\n0.012220\n0.012240\n0.012250\n0.012270\n0.012290\n0.012310\n0.012330\n0.012340\n0.012360\n0.012380\n0.012390\n0.012410\n0.012430\n0.012450\n0.012460\n0.012480\n0.012500\n0.012520\n0.012540\n0.012550\n0.012570\n0.012590\n0.012610\n0.012630\n0.012650\n0.012660\n0.012680\n0.012700\n0.012720\n0.012730\n0.012750\n0.012770\n0.012790\n0.012810\n0.012830\n0.012840\n0.012860\n0.012880\n0.012900\n0.012920\n0.012940\n0.012960\n0.012970\n0.012990\n0.013010\n0.013030\n0.013050\n0.013060\n0.013080\n0.013100\n0.013130\n0.013140\n0.013160\n0.013180\n0.013200\n0.013210\n0.013230\n0.013250\n0.013270\n0.013290\n0.013310\n0.013330\n0.013350\n0.013370\n0.013380\n0.013400\n0.013420\n0.013440\n0.013450\n0.013480\n0.013500\n0.013520\n0.013530\n0.013550\n0.013580\n0.013600\n0.013610\n0.013630\n0.013650\n0.013670\n0.013690\n0.013710\n0.013730\n0.013750\n0.013770\n0.013790\n0.013800\n0.013820\n0.013850\n0.013860\n0.013890\n0.013900\n0.013920\n0.013940\n0.013960\n0.013980\n0.014000\n0.014020\n0.014040\n0.014050\n0.014080\n0.014100\n0.014110\n0.014140\n0.014160\n0.014180\n0.014200\n0.014210\n0.014240\n0.014260\n0.014280\n0.014300\n0.014320\n0.014330\n0.014360\n0.014380\n0.014400\n0.014410\n0.014440\n0.014460\n0.014480\n0.014500\n0.014520\n0.014540\n0.014560\n0.014580\n0.014600\n0.014620\n0.014640\n0.014660\n0.014680\n0.014700\n0.014720\n0.014740\n0.014760\n0.014780\n0.014810\n0.014820\n0.014850\n0.014870\n0.014890\n0.014910\n0.014930\n0.014950\n0.014970\n0.014990\n0.015010\n0.015030\n0.015050\n0.015070\n0.015100\n0.015110\n0.015140\n0.015160\n0.015180\n0.015200\n0.015220\n0.015240\n0.015270\n0.015300\n0.015310\n0.015330\n0.015360\n0.015380\n0.015400\n0.015420\n0.015440\n0.015460\n0.015480\n0.015510\n0.015530\n0.015550\n0.015570\n0.015590\n0.015610\n0.015640\n0.015650\n0.015680\n0.015700\n0.015720\n0.015740\n0.015770\n0.015780\n0.015810\n0.015830\n0.015850\n0.015870\n0.015890\n0.015920\n0.015940\n0.015960\n0.015980\n0.016000\n0.016030\n0.016050\n0.016070\n0.016090\n0.016120\n0.016140\n0.016160\n0.016180\n0.016200\n0.016230\n0.016250\n0.016270\n0.016300\n0.016310\n0.016330\n0.016360\n0.016380\n0.016410\n0.016430\n0.016440\n0.016470\n0.016490\n0.016510\n0.016540\n0.016560\n0.016580\n0.016600\n0.016630\n0.016650\n0.016670\n0.016690\n0.016720\n0.016750\n0.016770\n0.016790\n0.016810\n0.016840\n0.016860\n0.016880\n0.016910\n0.016920\n0.016950\n0.016970\n0.016990\n0.017010\n0.017040\n0.017060\n0.017090\n0.017110\n0.017130\n0.017160\n0.017180\n0.017200\n0.017220\n0.017250\n0.017270\n0.017290\n0.017320\n0.017340\n0.017370\n0.017390\n0.017420\n0.017440\n0.017460\n0.017490\n0.017510\n0.017530\n0.017560\n0.017580\n0.017600\n0.017630\n0.017650\n0.017680\n0.017700\n0.017720\n0.017740\n0.017770\n0.017790\n0.017820\n0.017840\n0.017870\n0.017890\n0.017920\n0.017940\n0.017960\n0.017990\n0.018010\n0.018030\n0.018060\n0.018080\n0.018110\n0.018130\n0.018160\n0.018180\n0.018210\n0.018230\n0.018250\n0.018280\n0.018300\n0.018330\n0.018350\n0.018370\n0.018400\n0.018420\n0.018460\n0.018480\n0.018510\n0.018530\n0.018560\n0.018580\n0.018610\n0.018630\n0.018660\n0.018680\n0.018710\n0.018730\n0.018760\n0.018780\n0.018800\n0.018830\n0.018860\n0.018880\n0.018910\n0.018930\n0.018960\n0.018980\n0.019010\n0.019030\n0.019060\n0.019090\n0.019110\n0.019130\n0.019160\n0.019190\n0.019220\n0.019240\n0.019270\n0.019290\n0.019310\n0.019340\n0.019370\n0.019390\n0.019410\n0.019440\n0.019470\n0.019490\n0.019520\n0.019550\n0.019570\n0.019590\n0.019620\n0.019650\n0.019680\n0.019700\n0.019730\n0.019750\n0.019780\n0.019800\n0.019830\n0.019850\n0.019880\n0.019910\n0.019940\n0.019960\n0.019990\n0.020020\n0.020040\n0.020070\n0.020090\n0.020120\n0.020150\n0.020170\n0.020200\n0.020230\n0.020250\n0.020280\n0.020310\n0.020330\n0.020360\n0.020390\n0.020410\n0.020440\n0.020470\n0.020490\n0.020520\n0.020550\n0.020570\n0.020600\n0.020640\n0.020660\n0.020680\n0.020720\n0.020730\n0.020760\n0.020800\n0.020820\n0.020850\n0.020880\n0.020900\n0.020930\n0.020960\n0.020990\n0.021010\n0.021040\n0.021070\n0.021090\n0.021120\n0.021150\n0.021180\n0.021200\n0.021230\n0.021260\n0.021280\n0.021310\n0.021340\n0.021370\n0.021400\n0.021420\n0.021450\n0.021480\n0.021510\n0.021540\n0.021570\n0.021590\n0.021620\n0.021650\n0.021680\n0.021710\n0.021730\n0.021760\n0.021800\n0.021830\n0.021850\n0.021880\n0.021910\n0.021940\n0.021970\n0.022000\n0.022030\n0.022050\n0.022080\n0.022110\n0.022140\n0.022170\n0.022190\n0.022220\n0.022250\n0.022290\n0.022320\n0.022340\n0.022370\n0.022400\n0.022430\n0.022460\n0.022490\n0.022520\n0.022540\n0.022570\n0.022600\n0.022630\n0.022660\n0.022690\n0.022720\n0.022750\n0.022770\n0.022810\n0.022840\n0.022870\n0.022900\n0.022920\n0.022950\n0.022980\n0.023010\n0.023040\n0.023070\n0.023100\n0.023130\n0.023160\n0.023190\n0.023220\n0.023250\n0.023280\n0.023310\n0.023340\n0.023370\n0.023400\n0.023430\n0.023460\n0.023490\n0.023520\n0.023550\n0.023580\n0.023610\n0.023640\n0.023670\n0.023700\n0.023730\n0.023760\n0.023790\n0.023820\n0.023850\n0.023880\n0.023910\n0.023940\n0.023970\n0.024010\n0.024030\n0.024070\n0.024100\n0.024120\n0.024150\n0.024190\n0.024220\n0.024250\n0.024270\n0.024310\n0.024340\n0.024370\n0.024400\n0.024430\n0.024460\n0.024500\n0.024520\n0.024550\n0.024590\n0.024620\n0.024650\n0.024680\n0.024720\n0.024750\n0.024770\n0.024810\n0.024840\n0.024870\n0.024900\n0.024930\n0.024960\n0.025000\n0.025030\n0.025050\n0.025090\n0.025120\n0.025150\n0.025200\n0.025230\n0.025260\n0.025290\n0.025320\n0.025360\n0.025380\n0.025420\n0.025450\n0.025480\n0.025510\n0.025550\n0.025580\n0.025610\n0.025640\n0.025670\n0.025710\n0.025740\n0.025770\n0.025800\n0.025840\n0.025870\n0.025900\n0.025930\n0.025970\n0.026000\n0.026030\n0.026060\n0.026090\n0.026130\n0.026160\n0.026190\n0.026220\n0.026260\n0.026300\n0.026330\n0.026360\n0.026390\n0.026420\n0.026460\n0.026490\n0.026520\n0.026550\n0.026590\n0.026620\n0.026660\n0.026690\n0.026720\n0.026750\n0.026790\n0.026820\n0.026850\n0.026890\n0.026920\n0.026950\n0.026990\n0.027020\n0.027060\n0.027090\n0.027120\n0.027160\n0.027190\n0.027220\n0.027260\n0.027290\n0.027320\n0.027350\n0.027390\n0.027430\n0.027460\n0.027490\n0.027530\n0.027560\n0.027600\n0.027630\n0.027660\n0.027700\n0.027740\n0.027770\n0.027800\n0.027830\n0.027870\n0.027900\n0.027940\n0.027980\n0.028010\n0.028040\n0.028080\n0.028110\n0.028150\n0.028180\n0.028220\n0.028250\n0.028290\n0.028310\n0.028360\n0.028390\n0.028430\n0.028460\n0.028490\n0.028530\n0.028570\n0.028600\n0.028640\n0.028680\n0.028720\n0.028750\n0.028790\n0.028820\n0.028860\n0.028890\n0.028920\n0.028960\n0.029000\n0.029030\n0.029070\n0.029110\n0.029140\n0.029180\n0.029210\n0.029250\n0.029280\n0.029320\n0.029350\n0.029390\n0.029430\n0.029460\n0.029500\n0.029530\n0.029570\n0.029610\n0.029640\n0.029680\n0.029720\n0.029750\n0.029790\n0.029820\n0.029860\n0.029900\n0.029930\n0.029970\n0.030010\n0.030050\n0.030080\n0.030110\n0.030150\n0.030190\n0.030220\n0.030260\n0.030300\n0.030330\n0.030370\n0.030410\n0.030450\n0.030480\n0.030520\n0.030550\n0.030590\n0.030630\n0.030670\n0.030710\n0.030740\n0.030780\n0.030820\n0.030850\n0.030890\n0.030930\n0.030960\n0.031000\n0.031040\n0.031080\n0.031120\n0.031160\n0.031190\n0.031220\n0.031260\n0.031300\n0.031340\n0.031380\n0.031410\n0.031460\n0.031490\n0.031530\n0.031570\n0.031600\n0.031640\n0.031680\n0.031720\n0.031760\n0.031790\n0.031830\n0.031870\n0.031910\n0.031950\n0.031990\n0.032030\n0.032070\n0.032100\n0.032140\n0.032180\n0.032230\n0.032270\n0.032310\n0.032340\n0.032380\n0.032420\n0.032460\n0.032500\n0.032530\n0.032580\n0.032620\n0.032660\n0.032700\n0.032730\n0.032770\n0.032810\n0.032850\n0.032890\n0.032920\n0.032970\n0.033000\n0.033050\n0.033080\n0.033120\n0.033160\n0.033200\n0.033240\n0.033280\n0.033320\n0.033360\n0.033400\n0.033440\n0.033480\n0.033520\n0.033560\n0.033600\n0.033640\n0.033680\n0.033720\n0.033760\n0.033800\n0.033840\n0.033880\n0.033920\n0.033960\n0.034000\n0.034040\n0.034080\n0.034120\n0.034160\n0.034200\n0.034240\n0.034280\n0.034320\n0.034360\n0.034400\n0.034450\n0.034490\n0.034530\n0.034560\n0.034610\n0.034650\n0.034690\n0.034730\n0.034770\n0.034810\n0.034850\n0.034890\n0.034930\n0.034970\n0.035010\n0.035060\n0.035100\n0.035140\n0.035180\n0.035220\n0.035260\n0.035310\n0.035350\n0.035390\n0.035430\n0.035470\n0.035510\n0.035550\n0.035590\n0.035640\n0.035680\n0.035720\n0.035760\n0.035810\n0.035860\n0.035900\n0.035940\n0.035980\n0.036020\n0.036070\n0.036110\n0.036150\n0.036190\n0.036230\n0.036280\n0.036320\n0.036360\n0.036410\n0.036450\n0.036490\n0.036540\n0.036570\n0.036620\n0.036660\n0.036700\n0.036740\n0.036790\n0.036830\n0.036870\n0.036920\n0.036950\n0.037000\n0.037050\n0.037090\n0.037130\n0.037170\n0.037220\n0.037260\n0.037310\n0.037350\n0.037390\n0.037430\n0.037480\n0.037520\n0.037560\n0.037610\n0.037650\n0.037690\n0.037740\n0.037780\n0.037820\n0.037870\n0.037910\n0.037960\n0.038000\n0.038040\n0.038090\n0.038130\n0.038180\n0.038220\n0.038270\n0.038310\n0.038350\n0.038390\n0.038440\n0.038480\n0.038530\n0.038570\n0.038620\n0.038660\n0.038710\n0.038750\n0.038790\n0.038840\n0.038890\n0.038930\n0.038980\n0.039020\n0.039070\n0.039110\n0.039160\n0.039200\n0.039250\n0.039290\n0.039340\n0.039370\n0.039420\n0.039470\n0.039530\n0.039570\n0.039620\n0.039660\n0.039700\n0.039750\n0.039790\n0.039840\n0.039890\n0.039930\n0.039970\n0.040030\n0.040070\n0.040120\n0.040160\n0.040210\n0.040250\n0.040300\n0.040340\n0.040390\n0.040440\n0.040490\n0.040530\n0.040570\n0.040620\n0.040670\n0.040710\n0.040760\n0.040810\n0.040850\n0.040900\n0.040940\n0.040990\n0.041030\n0.041080\n0.041130\n0.041180\n0.041220\n0.041270\n0.041320\n0.041370\n0.041410\n0.041450\n0.041510\n0.041550\n0.041600\n0.041650\n0.041690\n0.041740\n0.041790\n0.041840\n0.041890\n0.041930\n0.041980\n0.042020\n0.042070\n0.042120\n0.042170\n0.042220\n0.042260\n0.042310\n0.042360\n0.042410\n0.042450\n0.042500\n0.042550\n0.042600\n0.042640\n0.042690\n0.042740\n0.042790\n0.042840\n0.042890\n0.042930\n0.042980\n0.043030\n0.043080\n0.043130\n0.043170\n0.043230\n0.043280\n0.043330\n0.043380\n0.043430\n0.043470\n0.043520\n0.043570\n0.043620\n0.043670\n0.043720\n0.043770\n0.043820\n0.043860\n0.043910\n0.043960\n0.044010\n0.044070\n0.044110\n0.044170\n0.044210\n0.044260\n0.044310\n0.044360\n0.044410\n0.044460\n0.044510\n0.044560\n0.044600\n0.044650\n0.044710\n0.044760\n0.044800\n0.044860\n0.044910\n0.044950\n0.045000\n0.045060\n0.045100\n0.045150\n0.045200\n0.045260\n0.045310\n0.045360\n0.045410\n0.045450\n0.045510\n0.045560\n0.045610\n0.045660\n0.045710\n0.045760\n0.045810\n0.045860\n0.045910\n0.045960\n0.046010\n0.046060\n0.046110\n0.046170\n0.046220\n0.046270\n0.046320\n0.046370\n0.046420\n0.046470\n0.046520\n0.046580\n0.046630\n0.046680\n0.046730\n0.046780\n0.046830\n0.046880\n0.046930\n0.046990\n0.047050\n0.047100\n0.047150\n0.047200\n0.047250\n0.047310\n0.047360\n0.047410\n0.047460\n0.047520\n0.047570\n0.047620\n0.047670\n0.047720\n0.047780\n0.047830\n0.047880\n0.047940\n0.047990\n0.048040\n0.048090\n0.048140\n0.048200\n0.048250\n0.048300\n0.048360\n0.048410\n0.048460\n0.048520\n0.048570\n0.048620\n0.048670\n0.048730\n0.048780\n0.048830\n0.048890\n0.048940\n0.048990\n0.049040\n0.049100\n0.049150\n0.049210\n0.049260\n0.049310\n0.049370\n0.049420\n0.049470\n0.049530\n0.049580\n0.049630\n0.049690\n0.049740\n0.049800\n0.049850\n0.049910\n0.049960\n0.050020\n0.050070\n0.050130\n0.050180\n0.050230\n0.050280\n0.050340\n0.050390\n0.050450\n0.050500\n0.050550\n0.050610\n0.050670\n0.050730\n0.050780\n0.050840\n0.050900\n0.050950\n0.051010\n0.051070\n0.051120\n0.051170\n0.051230\n0.051280\n0.051340\n0.051400\n0.051450\n0.051500\n0.051560\n0.051620\n0.051670\n0.051730\n0.051780\n0.051830\n0.051890\n0.051950\n0.052010\n0.052060\n0.052120\n0.052170\n0.052230\n0.052280\n0.052350\n0.052390\n0.052460\n0.052510\n0.052570\n0.052620\n0.052680\n0.052730\n0.052790\n0.052840\n0.052900\n0.052960\n0.053020\n0.053070\n0.053130\n0.053190\n0.053250\n0.053300\n0.053360\n0.053410\n0.053470\n0.053530\n0.053590\n0.053640\n0.053700\n0.053760\n0.053820\n0.053870\n0.053930\n0.053990\n0.054050\n0.054110\n0.054160\n0.054210\n0.054280\n0.054330\n0.054390\n0.054450\n0.054510\n0.054570\n0.054620\n0.054680\n0.054750\n0.054810\n0.054860\n0.054920\n0.054980\n0.055040\n0.055090\n0.055160\n0.055210\n0.055270\n0.055330\n0.055390\n0.055440\n0.055510\n0.055560\n0.055620\n0.055680\n0.055740\n0.055800\n0.055860\n0.055920\n0.055980\n0.056040\n0.056100\n0.056150\n0.056220\n0.056270\n0.056330\n0.056390\n0.056450\n0.056510\n0.056570\n0.056630\n0.056690\n0.056750\n0.056810\n0.056870\n0.056930\n0.056990\n0.057050\n0.057110\n0.057170\n0.057230\n0.057290\n0.057350\n0.057410\n0.057470\n0.057530\n0.057590\n0.057650\n0.057710\n0.057770\n0.057830\n0.057890\n0.057950\n0.058020\n0.058070\n0.058140\n0.058200\n0.058260\n0.058320\n0.058380\n0.058440\n0.058500\n0.058570\n0.058620\n0.058690\n0.058750\n0.058820\n0.058880\n0.058940\n0.059000\n0.059060\n0.059120\n0.059190\n0.059250\n0.059300\n0.059370\n0.059430\n0.059490\n0.059560\n0.059620\n0.059680\n0.059740\n0.059810\n0.059860\n0.059930\n0.059990\n0.060060\n0.060110\n0.060170\n0.060240\n0.060300\n0.060360\n0.060430\n0.060490\n0.060560\n0.060610\n0.060680\n0.060740\n0.060800\n0.060860\n0.060930\n0.060990\n0.061050\n0.061120\n0.061180\n0.061250\n0.061310\n0.061380\n0.061430\n0.061500\n0.061560\n0.061620\n0.061690\n0.061750\n0.061820\n0.061880\n0.061940\n0.062000\n0.062070\n0.062130\n0.062200\n0.062260\n0.062330\n0.062390\n0.062450\n0.062520\n0.062580\n0.062660\n0.062720\n0.062790\n0.062850\n0.062920\n0.062980\n0.063040\n0.063110\n0.063170\n0.063240\n0.063300\n0.063370\n0.063430\n0.063500\n0.063560\n0.063620\n0.063690\n0.063760\n0.063820\n0.063890\n0.063950\n0.064020\n0.064080\n0.064150\n0.064210\n0.064280\n0.064350\n0.064410\n0.064480\n0.064540\n0.064610\n0.064670\n0.064740\n0.064800\n0.064870\n0.064930\n0.065010\n0.065070\n0.065140\n0.065200\n0.065270\n0.065340\n0.065400\n0.065470\n0.065540\n0.065600\n0.065670\n0.065730\n0.065800\n0.065860\n0.065940\n0.066000\n0.066070\n0.066140\n0.066200\n0.066270\n0.066340\n0.066400\n0.066470\n0.066540\n0.066600\n0.066670\n0.066750\n0.066820\n0.066890\n0.066960\n0.067020\n0.067090\n0.067150\n0.067220\n0.067290\n0.067360\n0.067430\n0.067490\n0.067560\n0.067630\n0.067700\n0.067770\n0.067840\n0.067900\n0.067970\n0.068040\n0.068110\n0.068180\n0.068250\n0.068320\n0.068380\n0.068450\n0.068520\n0.068590\n0.068660\n0.068730\n0.068800\n0.068870\n0.068930\n0.069000\n0.069070\n0.069140\n0.069220\n0.069280\n0.069350\n0.069420\n0.069490\n0.069550\n0.069630\n0.069700\n0.069770\n0.069840\n0.069910\n0.069970\n0.070050\n0.070120\n0.070180\n0.070260\n0.070330\n0.070400\n0.070470\n0.070540\n0.070610\n0.070680\n0.070750\n0.070830\n0.070900\n0.070970\n0.071040\n0.071110\n0.071180\n0.071250\n0.071320\n0.071400\n0.071460\n0.071540\n0.071610\n0.071680\n0.071750\n0.071820\n0.071900\n0.071960\n0.072040\n0.072110\n0.072180\n0.072250\n0.072320\n0.072390\n0.072460\n0.072540\n0.072610\n0.072680\n0.072750\n0.072820\n0.072900\n0.072970\n0.073040\n0.073120\n0.073180\n0.073260\n0.073330\n0.073400\n0.073470\n0.073550\n0.073620\n0.073690\n0.073760\n0.073840\n0.073910\n0.073980\n0.074060\n0.074120\n0.074200\n0.074280\n0.074350\n0.074420\n0.074490\n0.074570\n0.074630\n0.074710\n0.074790\n0.074860\n0.074950\n0.075010\n0.075090\n0.075170\n0.075240\n0.075310\n0.075380\n0.075460\n0.075530\n0.075610\n0.075680\n0.075750\n0.075830\n0.075910\n0.075980\n0.076050\n0.076120\n0.076200\n0.076280\n0.076350\n0.076430\n0.076500\n0.076570\n0.076650\n0.076720\n0.076800\n0.076880\n0.076950\n0.077030\n0.077100\n0.077170\n0.077250\n0.077320\n0.077400\n0.077480\n0.077550\n0.077620\n0.077700\n0.077770\n0.077850\n0.077930\n0.078010\n0.078080\n0.078160\n0.078230\n0.078300\n0.078380\n0.078460\n0.078540\n0.078610\n0.078690\n0.078760\n0.078840\n0.078920\n0.078990\n0.079080\n0.079160\n0.079230\n0.079310\n0.079390\n0.079470\n0.079540\n0.079620\n0.079690\n0.079770\n0.079850\n0.079930\n0.080000\n0.080080\n0.080160\n0.080230\n0.080310\n0.080390\n0.080470\n0.080540\n0.080620\n0.080700\n0.080770\n0.080850\n0.080930\n0.081010\n0.081090\n0.081170\n0.081240\n0.081320\n0.081400\n0.081480\n0.081560\n0.081640\n0.081720\n0.081790\n0.081870\n0.081950\n0.082030\n0.082110\n0.082180\n0.082260\n0.082350\n0.082420\n0.082500\n0.082580\n0.082660\n0.082740\n0.082810\n0.082900\n0.082970\n0.083050\n0.083130\n0.083210\n0.083300\n0.083390\n0.083460\n0.083540\n0.083620\n0.083700\n0.083780\n0.083860\n0.083940\n0.084020\n0.084100\n0.084180\n0.084260\n0.084340\n0.084420\n0.084500\n0.084580\n0.084660\n0.084740\n0.084830\n0.084910\n0.084990\n0.085070\n0.085150\n0.085230\n0.085310\n0.085390\n0.085470\n0.085550\n0.085630\n0.085710\n0.085790\n0.085880\n0.085960\n0.086040\n0.086120\n0.086200\n0.086280\n0.086370\n0.086450\n0.086530\n0.086610\n0.086690\n0.086780\n0.086860\n0.086940\n0.087020\n0.087100\n0.087180\n0.087270\n0.087350\n0.087430\n0.087530\n0.087610\n0.087690\n0.087770\n0.087850\n0.087940\n0.088020\n0.088100\n0.088190\n0.088270\n0.088350\n0.088440\n0.088520\n0.088600\n0.088690\n0.088770\n0.088850\n0.088940\n0.089020\n0.089100\n0.089190\n0.089270\n0.089350\n0.089440\n0.089520\n0.089610\n0.089690\n0.089770\n0.089860\n0.089940\n0.090030\n0.090110\n0.090190\n0.090280\n0.090360\n0.090440\n0.090530\n0.090610\n0.090700\n0.090790\n0.090870\n0.090950\n0.091040\n0.091120\n0.091210\n0.091290\n0.091380\n0.091460\n0.091550\n0.091630\n0.091720\n0.091820\n0.091900\n0.091990\n0.092070\n0.092160\n0.092240\n0.092320\n0.092410\n0.092500\n0.092590\n0.092670\n0.092760\n0.092840\n0.092930\n0.093020\n0.093100\n0.093190\n0.093270\n0.093360\n0.093450\n0.093540\n0.093620\n0.093710\n0.093800\n0.093880\n0.093970\n0.094060\n0.094140\n0.094230\n0.094320\n0.094400\n0.094500\n0.094580\n0.094670\n0.094760\n0.094840\n0.094930\n0.095010\n0.095100\n0.095190\n0.095280\n0.095370\n0.095460\n0.095540\n0.095630\n0.095720\n0.095810\n0.095900\n0.095980\n0.096080\n0.096170\n0.096260\n0.096350\n0.096430\n0.096530\n0.096610\n0.096700\n0.096790\n0.096880\n0.096970\n0.097050\n0.097150\n0.097240\n0.097330\n0.097420\n0.097500\n0.097590\n0.097680\n0.097770\n0.097860\n0.097950\n0.098040\n0.098130\n0.098220\n0.098310\n0.098400\n0.098490\n0.098580\n0.098670\n0.098760\n0.098850\n0.098940\n0.099030\n0.099120\n0.099210\n0.099300\n0.099390\n0.099480\n0.099570\n0.099660\n0.099750\n0.099850\n0.099940\n0.100030\n0.100120\n0.100210\n0.100300\n0.100390\n0.100490\n0.100580\n0.100680\n0.100770\n0.100860\n0.100950\n0.101050\n0.101130\n0.101230\n0.101320\n0.101410\n0.101500\n0.101590\n0.101680\n0.101780\n0.101870\n0.101960\n0.102050\n0.102140\n0.102240\n0.102330\n0.102420\n0.102510\n0.102610\n0.102700\n0.102790\n0.102880\n0.102980\n0.103070\n0.103170\n0.103260\n0.103350\n0.103440\n0.103540\n0.103630\n0.103720\n0.103820\n0.103910\n0.104000\n0.104100\n0.104190\n0.104280\n0.104380\n0.104470\n0.104560\n0.104660\n0.104750\n0.104850\n0.104950\n0.105050\n0.105140\n0.105230\n0.105320\n0.105420\n0.105520\n0.105620\n0.105710\n0.105800\n0.105900\n0.105990\n0.106090\n0.106180\n0.106270\n0.106370\n0.106470\n0.106560\n0.106660\n0.106750\n0.106850\n0.106950\n0.107040\n0.107130\n0.107230\n0.107330\n0.107430\n0.107520\n0.107610\n0.107710\n0.107810\n") -> (array=w6:dbl[][])  [unwired: 2 in]
  n4 = Index Array(array=w12, index (col)=0 ("disabled index (col)")) -> (element=w10:dbl[])  [unwired: 1 in]
  "T array / K" <- w10
  n5 = Index Array(array=w7, index (col)=0 ("disabled index (col)")) -> (element=w4:dbl[])  [unwired: 1 in]
  "Cp0 array / J mol-1 K-1" <- w4
  n6 = Index Array(array=w6, index (col)=0 ("disabled index (col)")) -> (element=w5:dbl[])  [unwired: 1 in]
  "u(Cp0) / J mol-1 K-1" <- w5
  n7 = Divide(x=w5, y=w4) -> (x/y=w3:dbl[])
  n8 = Multiply(x=w3, y=1000000.0) -> (x*y=→"ur(Cp0) /ppm":dbl[])
  n9 = call <vilib>:"Spline Interpolant.vi"("X"=w10, "Y"=w4) -> ("Interpolant"=w30:dbl[])  [unwired: 2 in, 1 out]
  n10 = call <vilib>:"Spline Interpolant.vi"("X"=w10, "Y"=w5) -> ("Interpolant"=w26:dbl[])  [unwired: 2 in, 1 out]
  n11 = call <vilib>:"Spline Interpolation.vi"("x value"="Temperature [K]", "Interpolant"=w30, "X"=w10, "Y"=w4) -> ("interpolation value"=w23:dbl)  [unwired: 1 out]
  "Cp0 N2 [J / K mol]" <- w23
  n12 = call <vilib>:"Spline Interpolation.vi"("x value"="Temperature [K]", "Interpolant"=w26, "X"=w10, "Y"=w5) -> ("interpolation value"=w24:dbl)  [unwired: 1 out]
  "abs unc Cp0 N2 [J / K mol]" <- w24
  n13 = Divide(x=w23, y=w27) -> (x/y=w22:dbl)
  "Cp0/R N2" <- w22
  n14 = Subtract(x=w23, y=w27) -> (x-y=w29:dbl)
  "Cv0 N2 [J / K mol]" <- w29
  n15 = Divide(x=w24, y=w23) -> (x/y=w21:dbl)
  n16 = Absolute Value(x=w21) -> (abs(x)=w20:dbl)
  "rel unc Cp0 N2" <- w20
  n17 = Divide(x=w23, y=w29) -> (x/y=→"Gamma0 N2":dbl)
  n18 = Multiply(x=w22, y=w20) -> (x*y=→"abs unc Cp0/R N2":dbl)
